vi "UHR-Fleezers Control (host) -Leonardo 04-2018 V5_cleanup.vi"() -> ()   [LabVIEW 2013]
uses:
  <vilib>/Utility/miscctls.llb/LVPoint32TypeDef.ctl
  <vilib>/Utility/miscctls.llb/LVMinMaxIncTypeDef.ctl
  <vilib>/Platform/TimedLoop/XDataNode/timing_clust.ctl
  <vilib>/Platform/TimedLoop/XDataNode/nitl_modes.ctl
  <vilib>/Platform/TimedLoop/XDataNode/wakeup.ctl
  <vilib>/userdefined/High Color/nirio_resource_hc.ctl
  <vilib>/Analysis/baseanly.llb/Mean (DBL).vi
  FPGA VIs Alex/Alex subVIs/Downsample1D.vi
  FPGA VIs Alex/Alex subVIs/Integrate1D.vi
  <vilib>/FPGAPlugInAG/PCIe-7852R/niLvFpga_Open_PCIe-7852R.vi
  <vilib>/FPGAPlugInAG/PCIe-7852R/niLvFpga_Reset_PCIe-7852R.vi
  <vilib>/FPGAPlugInAG/PCIe-7852R/niLvFpga_Run_PCIe-7852R.vi
  <vilib>/FPGAPlugInAG/PCIe-7852R/niLvFpga_Close_PCIe-7852R.vi
  <vilib>/Utility/error.llb/Error Cluster From Error Code.vi
  <vilib>/rvi/errors/niLvFpgaAdjustHostInterfaceError.vi
  <vilib>/rvi/interface/common/niFpgaWaitOnOcc.vi
  downsample 1D array - double.vi
  <vilib>/express/express analysis/Spectral/Block/exnSpectralBlock spectral measurements PSD poly.vi
  <vilib>/express/express analysis/Spectral/Block/exnSpectralBlock spectral measurements PSD WFM.vi
  <vilib>/Waveform/WDTOps.llb/WDT Append Waveforms DBL.vi
  <vilib>/gmath/statdist.llb/Exp Random.vi
  <vilib>/gmath/statdist.llb/Gamma Random.vi
  <vilib>/FPGAPlugInAG/PCIe-7852R/niLvFpga_Abort_PCIe-7852R.vi
  openfpgaref.8.6.ctl
  <vilib>/Platform/TimedLoop/XDataNode/XDataNode.xnode
  <vilib>/rvi/interface/nirviOpenFPGA/nirviOpenFPGA.xnode
  openfpgaref.initrf.ctl
  FPGA Bitfiles/UHR-FleezersInst_FPGATarget_intitializeRF201804.lvbitx
  <vilib>/rvi/interface/nirviMethod/nirviMethod.xnode
  <vilib>/rvi/interface/nirviCloseFPGA/nirviCloseFPGA.xnode
  FPGA Bitfiles/UHR-FleezersInst_FPGATarget_UHR-FleezersCont_IqK95Pvv9lYv5.3.lvbitx
  <vilib>/rvi/interface/nirviReadWriteControl/nirviReadWriteControl.xnode
  <vilib>/express/express analysis/Spectral/XNode/ExpressSpectralMeasurementsBlockNode.xnode
  <vilib>/Analysis/NI_AALBase.lvlib
  <vilib>/Platform/TimedLoop/XDataNode/XDNodeRunTimeDep.lvlib
  <vilib>/rvi/errors/niLvFpgaMergeErrorWithErrorCode.vi
  <vilib>/gmath/NI_Gmath.lvlib
  <vilib>/FPGAPlugInAG/PCIe-7852R/niLvFpga_ConfigureFifo_PCIe-7852R.vi
  NiFpgaLv.dll
panel:
  in  "Reinit Valve?":bool=TRUE
  out "Data Period (s)":dbl=1.4999999999999999e-05 caption="Trap Data Period (s)" format="%#_6p"
  out "ideal setpoint fpga":dbl
  out "ideal setpoint avgd":dbl
  out "Step duration":dbl
  in  "Number of steps":i32
  out "Step taken":dbl
  in  "Distribution":enum16{"uniform", "Exponential", "Gamma2"}(ring)
  in  "Mean dwell time (s)":dbl=0.001 min=0.001
  in  "Backtrack probability":dbl min=0.0 max=1.0
  in  "Simulate stepping":bool
  in  "Step size (nm)":dbl min=0.0
  out "Actual setpoint":fxp<+/-,16,1> format="%.16g"
  in  "Target Force (pN)":dbl=10.5
  in  "MCL Tracking":bool
  out "Current Trap Delta":dbl=20.03845214843774
  out "Tether Extension (nm, calculated)":dbl=1280.0838354247721 format="%0.2f"
  in  "Set SP to Current Frc":bool
  out "Trap X (AI1)":T1={"Trap 1"=0.030792236328125, "Trap 2"=-0.011322021484375}
  in  "Trap Pos FB SP":fxp<+/-,16,1>=0.231353759765625 caption="Setpoint"
  in  "Trap Pos. FB ON":bool
  out "Trap Positions":waveform(dbl)[](graph)
  out "Action (%)":dbl(knob)=-100.0 scale=-100.0..100.0
  in  "Trap Pos. FB Out Scale 2^n":u8=23 caption="Action Scale"
  out "Location path":path=path "C:/Users/Fleezers/Desktop/UHR-Fleezers Instrument - Charlie/Locations.txt"
  in  "Location Matrix":string[][](array[string])=[["N.D.\r\n", "N.D.\r\n", "N.D.\r\n"], ["N.D.\r\n", "N.D.\r\n", "N.D.\r\n"], ["N.D.\r\n", "N.D.\r\n", "N.D.\r\n"], ["N.D.\r\n", "N.D.\r\n", "N.D.\r\n"]]
  in  "Tab Action Shortcuts":T2(tab)=enum."Calibration"
  in  "Negate trap 2 force":bool
  in  "Use Full Offset?":bool=TRUE
  in  "Take Stepping Data":bool
  in  "Cap 1 Flow ON":bool=TRUE
  in  "Move Cap. 1 (DNA Top)":bool
  in  "Cal/Data Acq. Spot":bool
  in  "Cap 1 T ON":bool=TRUE
  in  "Cap 1 Samp Flow ON":bool=TRUE
  in  "Offset 2 Set":dbl=2.0
  in  "Offset 1 Set":dbl=1.0
  in  "Cal @ (MHz)":dbl=20.0
  in  "W/ Offset 1":bool=TRUE
  in  "Offset 1 Start (MHz)":dbl=13.0
  in  "W/ Offset 2":bool
  in  "Offset 2 Start (MHz)":dbl=16.0
  in  "Pause at Closest Delta (s)":dbl
  in  "Move to Delta 2 (MHz)":dbl=41.0
  in  "Attempt Limit":dbl=30.0 caption="Limit"
  out "Attempts":dbl=1.0
  in  "Wait Before Save (s)":u32=1
  in  "Fish for Tether":bool
  in  "Closest Delta (MHz)":dbl=13.0 step=0.25
  in  "Stop F (pN)":dbl=10.0
  in  "Then...":string(combo)="2"
  in  "Move to Delta 1 (MHz)":dbl=15.0
  in  "Tether Alarm?":bool=TRUE
  out "Tether":bool
  in  "Raster Set Upon Tether":u32=1
  in  "Save at end (5, 6)":bool
  in  "N Steps":dbl=20.0
  in  "Step Size (nm)":dbl=0.34
  in  "Save ave factor":dbl=1.0
  in  "APD to Watch":bool
  out "Duration (s)":dbl
  in  "Action":string(combo)="Yank"
  in  "Fl. Triggered...":bool
  in  "Fl. Delta Thresh. (kHz)":dbl=0.6
  out "Waiting":bool
  out "Fl. High":bool
  in  "Yank Delay (s)":dbl=3.5
  in  "Yank to Delta Array (MHz)":dbl[](array[numeric])=[16.3, 15.85, 14.85]
  in  "N Array El":u8=3 min=1 step=1
  in  "Random Choice":bool=TRUE
  in  "Force Yank":bool
  in  "Force Reset":bool
  in  "Toggle AFish":bool
  in  "Extend Min F":dbl=1.0
  in  "Extend Min TD":dbl=8.0
  in  "Extend dTD":dbl=5.0
  out "AF Time":u32
  in  "Wiggle time":dbl
  in  "Wiggle TD":dbl=1.0
  in  "Max TD":dbl=15.0
  in  "Min TD":dbl=8.0
  out "Fish Status":u16(ring) items=["Off", "Approach", "Wiggle", "Extend", "Tether Found"]
  in  "Approach dTD":dbl=-5.0 format="%#_13g"
  out "Messages":string="5:58 PM\tUHR-Fleezers ready.\r"
  in  "Stop All":bool=TRUE
  in  "Tab Control Display":T3(tab)
  in  "APD 2 Offset":dbl
  in  "APD 1 Offset":dbl
  out "Mean":dbl=1.039039384389187 caption="Mean (pN)" format="%#_3g"
  out "Force":waveform(dbl)[](graph)
  out "APD Chart":waveform(dbl)[](graph)
  in  "Calibration":u16(ring)=2 items=["None", "Position", "Force"]
  out "T1 X":dbl=-1.511158478291593 caption="T1 X (pN)" format="%0.2f"
  out "T2 X":dbl=0.5669202904867809 caption="T2 X (pN)" format="%0.2f"
  out "Bead Separation":waveform(dbl)(graph)={"t0"=timestamp(2751.0000000002074 s since 1904-01-01), "dt"=0.15, "Y"=[13.487296816964651, 13.48037403257866], "attributes"=variant("NI_ChannelName"=variant(string "T1 X"))}
  out "Difference":dbl=0.9442381878048121 caption="Difference (pN)" format="%.2g"
  in  "Offset (nm)":dbl
  in  "Rescale on Mean":bool
  in  "Bead Sep. Int. Time (s)":dbl=5.0 caption="Int. Time (s)"
  in  "Take Detection Laser\nImage":bool
  out "APD 2":T4(plugin-control) caption="APD 2 (Cy5)"
  in  "Flip Green Filter":bool
  in  "Set X Only":bool
  in  "Set Y Only":bool
  out "APD 1":T4(plugin-control) caption="APD 1 (Cy3)"
  out "Detection Laser Y":T4(plugin-control)
  out "Pointer Y (V)":dbl=4.0025870540482815 format="%_3g"
  out "Pointer X (V)":dbl=4.635613485356835 format="%_3g"
  in  "Set Confocal Spot (X-Y)":bool
  out "Detection Laser X":T4(plugin-control)
  out "All Signals":waveform(dbl)[](graph)=[{"t0"=timestamp(2751.0000000002074 s since 1904-01-01), "dt"=0.02, "Y"=[0.0, 0.0, 0.0, 0.0, 0.0, 0.0, 0.0, 0.0, 0.0, 0.0, 0.0, 0.0, 0.0, 0.0, 0.0], "attributes"=variant("NI_ChannelName"=variant(string "APD 1"))}, {"t0"=timestamp(2751.0000000002074 s since 1904-01-01), "dt"=0.02, "Y"=[0.0, 0.0, 0.0, 0.0, 0.0, 0.0, 0.0, 0.0, 0.0, 0.0, 0.0, 0.0, 0.0, 0.0, 0.0], "attributes"=variant("NI_ChannelName"=variant(string "APD 2"))}, {"t0"=timestamp(2751.0000000002074 s since 1904-01-01), "dt"=0.15, "Y"=[-0.020049210394969354, -0.02003592505550746], "attributes"=variant("NI_ChannelName"=variant(string "T1 Y"))}, {"t0"=timestamp(2751.0000000002074 s since 1904-01-01), "dt"=0.15, "Y"=[0.03074231675925172, 0.03074526419399293], "attributes"=variant("NI_ChannelName"=variant(string "T1 X"))}, {"t0"=timestamp(2751.0000000002074 s since 1904-01-01), "dt"=0.15, "Y"=[2.9160941496017294, 2.916128360850853], "attributes"=variant("NI_ChannelName"=variant(string "T1 Sum"))}, {"t0"=timestamp(2751.0000000002074 s since 1904-01-01), "dt"=0.15, "Y"=[-0.002644972968316131, -0.002638961391604115], "attributes"=variant("NI_ChannelName"=variant(string "T2 Y"))}, {"t0"=timestamp(2751.0000000002074 s since 1904-01-01), "dt"=0.15, "Y"=[-0.011335016186436862, -0.011341032214389745], "attributes"=variant("NI_ChannelName"=variant(string "T2 X"))}, {"t0"=timestamp(2751.0000000002074 s since 1904-01-01), "dt"=0.15, "Y"=[2.746599475081634, 2.746642933439132], "attributes"=variant("NI_ChannelName"=variant(string "T2 Sum"))}, {"t0"=timestamp(2751.0000000002074 s since 1904-01-01), "dt"=0.15, "Y"=[-0.526083166086966, -0.5261552546492463], "attributes"=variant("NI_ChannelName"=variant(string "T1 FB X"))}, {"t0"=timestamp(2751.0000000002074 s since 1904-01-01), "dt"=0.15, "Y"=[3.0920304879909737, 3.0920243537705665], "attributes"=variant("NI_ChannelName"=variant(string "T2 FB Sum"))}, {"t0"=timestamp(2751.0000000002074 s since 1904-01-01), "dt"=0.15, "Y"=[-0.7128125059590501, -0.7128388598091219], "attributes"=variant("NI_ChannelName"=variant(string "T2 FB X"))}, {"t0"=timestamp(2751.0000000002074 s since 1904-01-01), "dt"=0.15, "Y"=[2.9122738731040343, 2.91227808465834], "attributes"=variant("NI_ChannelName"=variant(string "T2 FB Sum"))}, {"t0"=timestamp(2751.0000000002074 s since 1904-01-01), "dt"=0.15, "Y"=[-0.0023344523453474137, -0.002339854121524665], "attributes"=variant("NI_ChannelName"=variant(string "PSD Y"))}, {"t0"=timestamp(2751.0000000002074 s since 1904-01-01), "dt"=0.15, "Y"=[-0.0026477858821374683, -0.002642139957884409], "attributes"=variant("NI_ChannelName"=variant(string "PSD X"))}, {"t0"=timestamp(2751.0000000002074 s since 1904-01-01), "dt"=0.15, "Y"=[0.014415417950986964, 0.014429639576402777], "attributes"=variant("NI_ChannelName"=variant(string "PSD Sum"))}]
  in  "Signals to Plot":i32(listbox)=9
  out "Trap Disp. Freq. (Hz)":dbl=6.666666666666667 caption="Freq. (Hz)" format="%#_6p"
  out "Display Period (s)":dbl=0.15 caption="Period (s)" format="%#_6p"
  in  "Trap Disp. Downsample":i32=10000 caption="Downsample" max=20000
  in  "APD Disp. Scale":dbl=0.1 caption="Scale (Divide,\nfor above plot only)"
  in  "APD Disp. dSamp":i32=2 caption="Integrate" min=1 max=30 step=1
  out "APD Display Freq. (Hz)":dbl=50.0 caption="Freq. (Hz)"
  out "APD Display Period (s)":dbl=0.02 caption="Period (s)"
  out "FFT 1":cluster{"f0":dbl, "df":dbl, "magnitude":dbl[]}[](graph)=[{"f0"=0.0, "df"=16.666666666666668, "magnitude"=[-331.1367572010275, -79.05506245821404, -86.61411242440559, -88.4728176091699, -90.3181253945935, -94.12566333707997, -92.52740723119955, -94.92192587982518, -99.60936585245742, -96.87568627870715, -94.02570383337763, -83.8058550151726, -97.57441397235512, -101.59968530846606, -101.523049255742, -103.35038532190343, -101.58594091014982, -102.96098031851216, -91.39759462745924, -103.75019963279499, -104.45030075054324, -103.04245334279298, -104.0720279134107, -106.06482372394834, -103.69131867828104, -104.40395035115309, -105.96420043276396, -107.6735556337804, -106.673030006608, -107.34889066208132, -108.05626565233933, -106.25659018850432, -105.29934513380842, -105.43096056709592, -108.3728498841465, -106.0555440144992, -105.78001282181421, -107.48741857324953, -108.67624970548897, -105.39976667156175, -105.91413119232612, -109.4222808198164, -107.0898971593174, -107.91164191890915, -108.26032038855709, -107.58332347164534, -108.23559688234297, -108.01271040303237, -107.66511723652701, -106.51901583170391, -109.27249501469946, -108.55647681594805, -107.93499259231463, -107.05068166453935, -109.13641475410455, -109.29679733781423, -108.19360835527803, -109.57747591546632, -109.58364591011674, -110.47061433372711, -109.8144340420426, -108.79067462293897, -107.54887553357234, -107.99559866705923, -108.85023923652685, -109.68733225238618, -108.51101278437793, -108.51620475114115, -108.22212402200637, -104.63726950302143, -110.2989919678048, -107.61796444414897, -108.68882962798736, -104.79193983043893, -103.59504263746938, -93.64633660288543, -101.9191640501395, -105.73717393151816, -108.92572458793902, -107.43962662800902, -107.79595323081325, -107.0923101993207, -108.17603277205289, -107.87074270713183, -109.20899066381877, -108.61832060412445, -109.10072003106593, -105.76480632823524, -108.60877649218978, -109.67541158970121, -110.2286232768028, -109.84952155309578, -109.33772024076384, -109.95251642394683, -110.14777282585466, -109.13825677905699, -110.05989365698167, -109.39359990189426, -110.56255614635295, -109.66477183197163, -108.9397158528824, -110.26529907650465, -109.20049464984628, -108.20183857013548, -109.09752250184418, -108.00440442238454, -108.35465963524055, -111.16774134451799, -110.34812550238405, -108.94506763426756, -108.72845542102493, -109.41512344014713, -112.44661664432377, -110.35437330889101, -111.32939440655925, -109.42989530434981, -110.98084669076195, -111.92160561143541, -108.57755551751093, -111.40042616180912, -110.15284955891853, -112.21455132279115, -111.40787773511747, -108.82949641635288, -110.13442122547907, -111.42229298204664, -112.06314940885191, -110.6015308813694, -109.51144097251623, -111.15989713761475, -110.25535755335385, -109.65868178057926, -110.51649885452997, -109.77194745285269, -108.4234206864394, -109.50892632093968, -109.46471287444389, -107.92241289271415, -109.72283805386196, -108.63426821579918, -110.37316681536255, -111.09713996884652, -110.32903619589223, -105.32012665515045, -107.36858557554393, -108.00382215905725, -110.06430686942338, -108.81666625979916, -110.01277074453823, -110.94194741225512, -109.65934609082873, -107.80979136006962, -112.81333866824724, -111.61474300955487, -109.83998277184975, -109.45953946904639, -109.79640584952526, -108.19172301667324, -109.28894656674316, -107.61471301278785, -108.83814006090513, -109.08866847726084, -108.20250571862371, -107.96222236861584, -107.03811197900873, -108.93533000393974, -107.74482548035408, -110.79811544577694, -111.1387476496877, -107.42970105883512, -109.18442281176472, -108.73546184641192, -108.71800246690864, -108.51945944378063, -108.06825856571285, -107.27210712368412, -108.12304695877637, -107.84933283677306, -109.73682373154998, -109.32284761503395, -109.31328817453769, -106.68762108642842, -109.79203616876461, -109.9020278896408, -110.27080024357275, -108.54152101558762, -111.00464391726017, -112.42244020766577, -110.82707315747889, -111.00344011890857, -109.90461839395674, -109.42877207451863, -109.73549298167016, -111.67494793393293, -108.85799077901427, -108.5348443278263, -109.803781083881, -108.30644755543659, -108.5079527456017, -111.2055351312823, -108.53089994340155, -108.01739789012176, -108.70360662855235, -107.95873456794631, -109.58297170693093, -108.9372401694271, -110.15921663527153, -109.22399119911955, -110.89883651739237, -108.92840112258382, -110.0545300523626, -109.05961065387005, -109.45831398589371, -108.61239387653227, -110.13001256174265, -108.80060224137931, -109.46327400696283, -108.0177965824709, -109.29727944627197, -110.3237255895986, -109.03258262543821, -110.97880178489321, -109.70034895077919, -111.16405638194153, -109.17324451464711, -109.65698250854277, -108.96750235822178, -112.00534231585624, -108.69274607723942, -108.98110446396657, -108.40723795464795, -111.44459094807324, -111.74799245277113, -111.1601960491512, -108.92048232753773, -110.30506377784799, -111.33145973979093, -110.91850998672503, -110.33684985776448, -108.90206518366908, -109.28458878227542, -108.98773986023751, -110.85813863075646, -109.00041591105906, -110.84543686681204, -109.84382395806176, -109.69722434763266, -108.50915601095721, -107.80829925826895, -110.59736107582401, -109.75377770317087, -109.3992084496136, -110.51151565846742, -112.49753959826434, -109.7299632589479, -109.54070743868353, -109.90314341132164, -111.05974202976806, -109.03766862152392, -109.46667095459878, -109.52800799036197, -111.3163121356807, -110.07817134522178, -108.69251657453547, -109.40472158898045, -109.71400709815576, -110.60534468715097, -109.46937396724682, -107.70342491418788, -109.86331122597839, -108.64971387994616, -110.90117371097081, -108.34928840565928, -110.04172889660904, -111.52979926554961, -110.34759300823305, -109.62712781837159, -109.24131154553284, -110.23196152450447, -108.68509612326807, -108.0246905483419, -106.61876139289784, -101.5519630114271, -80.57695480953835, -102.03744443354402, -107.1449217193017, -110.0695213407169, -106.61597783999268, -110.79221011808191, -109.58974545931426, -109.1149802216988, -109.20993813088597, -109.63768480465863, -110.10428394219181, -109.08445084271477, -108.83472375362581, -109.69508502050168, -108.05588796178941, -110.62586360101581, -109.95315261676905, -107.52208264977473, -108.80708007514875, -110.43484881098874, -110.45942171588936, -107.83804717866751, -109.98973910294193, -109.3496496054193, -108.425252911127, -110.94579264380809, -108.54181722177951, -108.67696070083541, -108.4150202151644, -109.24973583101504, -112.0454922608961, -111.29046597340738, -110.75018248960077, -109.38326363603683, -109.2033340336957, -109.45076170874889, -109.52878049853727, -109.32340869724774, -110.98123395128233, -110.75736340635505, -109.7218385823809, -107.97422606064993, -109.77313701758703, -110.95948744392717, -110.08996774172691, -108.51011830110778, -109.78063140243836, -110.65996628628228, -109.83684298615616, -110.33329049188029, -110.13755118968292, -110.3717925645783, -108.55302219178951, -106.86811628734195, -108.6302156589162, -108.75341391045045, -108.32589578384841, -108.70061474734084, -112.30742263527534, -109.16842570592085, -109.29767035534508, -108.87829025017463, -108.2255616391397, -108.4316108616088, -108.82995906929271, -110.40135575415563, -109.51623498946435, -109.79409808792403, -107.03832759632121, -108.36534528684132, -109.72010868372905, -107.90933028179892, -106.95643597294047, -111.29929166165778, -110.23001135794706, -108.98838015381585, -109.79115357104436, -108.18627479511115, -108.14988122174307, -109.12074063466532, -109.41904850488358, -111.40409873721113, -108.83156790193294, -108.77032248953847, -108.88363158686694, -108.47515048290681, -105.94172147874599, -109.38146940214403, -109.21277078848794, -108.11309390545507, -110.70840012427504, -109.5504457849329, -109.52330684534209, -110.06776026911132, -108.21949434182314, -111.21266686269992, -108.78581501170974, -108.43115799297222, -109.63260325780062, -109.84070220619535, -109.72041980780126, -110.29615941882527, -110.60316734262464, -108.79165446414692, -110.95840439895592, -109.64926233107009, -109.16526769544322, -108.65292362430982, -109.56113898129935, -109.85693046339026, -108.92316027325207, -109.79492493553914, -109.38157962945887, -110.24545136266825, -109.30031463492487, -109.0795429936869, -111.4091719525013, -108.63499083917162, -108.43863465339358, -109.23207864880891, -111.21947487191643, -109.24525201480154, -109.56842406077318, -109.46711940800672, -111.91389548262572, -108.15655736690546, -108.71882059966947, -111.26328503478568, -110.95027143873176, -108.4853106242357, -110.36902802777546, -109.9314203579182, -108.77686164101732, -108.71871020068312, -111.04829661168574, -109.95072655339462, -109.88221342875462, -109.53241732756136, -108.2625005404823, -108.00677030040697, -110.19659317581693, -108.93858924796267, -109.46817875483995, -110.78063992017232, -111.11066570318451, -110.78774336696706, -109.19199744617812, -108.54914256407436, -109.28414960420909, -110.64143585101183, -110.5855350821307, -109.47578632252726, -108.89705360836223, -109.89214013612292, -107.93271261027171, -109.32631601340563, -108.60274611341092, -109.40110159872573, -110.889237682208, -110.01391165813328, -109.99747108785071, -108.65542819213674, -110.37211847668736, -110.44656500845738, -110.8128133834973, -108.8909299260433, -110.19551227077532, -111.37647266643523, -110.83802189730321, -109.98519377913681, -110.52378970770522, -108.16970420057817, -110.70974729773344, -110.76836765494402, -110.26884275594577, -109.22041044268806, -109.87809744746195, -107.76823252107832, -109.12119474042969, -110.28066108731146, -108.55000033509207, -110.18152097767907, -110.73030521152278, -111.49470908029893, -110.2320929919509, -110.03370979233021, -109.79181668155233, -108.6673501209991, -109.86695766650877, -107.88926518046961, -110.95525003776572, -109.18130359755742, -110.42618009658618, -107.90341931158893, -111.44736855661769, -110.72634267386593, -109.29945988519303, -107.67889101961411, -108.81148059987765, -109.13375212757057, -109.8122873383549, -109.80176697684155, -109.96342275204768, -109.90406635707086, -108.75674342748256, -110.12362902701081, -109.82151095527837, -108.62543344241836, -110.09171852771195, -110.21434637862887, -109.97254504855631, -109.27043209093468, -111.35149588204125, -110.12399876776051, -111.65983675538546, -109.28788875768564, -110.86554069990251, -111.26990906470603, -108.60956517491746, -111.49613890850938, -111.79685722966795, -109.26269485364045, -110.38555615546439, -109.40641023162068, -110.966136593156, -108.78892524584494, -110.29340727375603, -111.44032043281035, -109.95212021173755, -109.79233511584334, -112.41184021118175, -109.73687851881148, -108.65493879781806, -110.76132988919045, -108.43230346094671, -110.32968175895853, -110.29890782023821, -108.77609076424456, -110.3298662333555, -109.47734504217333, -108.2677295732245, -109.21234363352882, -107.83278941978479, -108.85136784424789, -108.43241251530755, -109.76609391460555, -108.53204373005357, -110.9660641972934, -110.3152512161094, -110.72570499399905, -109.23877906286317, -111.72407743101837, -109.20311421918561, -108.06021800233717, -109.29288625761943, -108.78395253409145, -111.85250172876302, -108.78827588901797, -109.79775055719482, -109.12089297455859, -109.49896359356035, -110.34432647103819, -107.94700097960238, -109.30489238477631, -108.89170290869342, -108.82574563272509, -110.11024077194833, -107.37946433552314, -109.60167933458756, -107.80625057819019, -110.11489057210264, -107.35436859378505, -105.69819484613895, -109.11280625683739, -109.27770293057978, -107.7053735252589, -109.75022444894368, -109.3310543596577, -107.87683693707739, -108.19931495338068, -109.26462246191564, -106.71885779297867, -100.00018022217961, -92.54434511397295, -107.20472143807373, -107.39203415155283, -110.04461177268398, -108.48860496315312, -109.0057168110333, -108.37627790492552, -108.4108380728248, -109.65509454313073, -109.64243000632982, -97.04219069306761, -109.0928856629964, -107.9760697315632, -107.52611064047497, -108.87702814778996, -109.08437599027614, -110.70097118837974, -109.00969860961283, -110.38275386163214, -110.0699155421545, -106.91498895181175, -106.22178738309017, -109.36827866896039, -107.59953130968307, -109.19516217272808, -108.31502495393616, -109.384158926223, -107.11670654202719, -108.09436312738853, -110.14559230873704, -109.84997663447679, -107.83465335309926, -108.60947100624459, -108.9932479423645, -109.17174810371898, -108.79457339828916, -109.40909327982367, -109.6328723628302, -109.51081854476179, -107.63054408568418, -109.63728404010122, -108.51163794839918, -107.55002282725216, -108.97796212764939, -107.24648164623483, -112.21470452291085, -108.74294024554423, -109.62070777514892, -108.05768666239368, -109.8224946685739, -109.34575507446003, -108.53536952609525, -109.60789300457671, -107.56681538208278, -109.22777325016398, -108.79047910308894, -110.10332477250668, -108.00206387955672, -108.45604004720035, -109.00645795765472, -109.81039564269616, -108.92785144634745, -108.3978471520567, -107.94411095685999, -110.53486519304262, -108.8773780319227, -109.03345093296107, -107.30746693745031, -108.54277704832029, -108.77629108166091, -108.91111762599647, -107.74965195880401, -109.97375370738439, -109.76326492689246, -107.91717581777407, -109.0730556927617, -107.66804873204664, -110.40438871064791, -108.05794247751498, -108.80206615156494, -107.51329354700796, -108.83687012994949, -107.57713176895379, -107.94774159581414, -109.41894615439651, -107.10869425078764, -110.51480854078629, -108.92221367099775, -109.91358786461535, -110.1744263092835, -109.30795472883494, -107.91359710691006, -109.77888185049835, -109.52060975706438, -108.66686651982212, -108.71041801553639, -110.13619546359467, -108.87957097273856, -109.72150387215271, -109.00776068810654, -109.70251113927438, -110.75769213896399, -108.53234896741436, -109.69439526582246, -110.15412541604617, -108.25183374628219, -107.97402569656481, -110.34920156998648, -108.45106995186384, -108.82031145748209, -111.38690005057539, -107.01968459818563, -110.3044500039584, -110.8755481852125, -111.08915057663255, -107.94824988655199, -110.21669144934839, -109.90539774633154, -109.58985438756767, -110.12258796623348, -109.41689951612143, -109.31128210476795, -109.00258476567323, -109.11093063041056, -108.83347064311234, -108.32685287566952, -109.44770946560935, -108.40145063144861, -109.68448193892085, -108.76525439243828, -107.62837139034596, -107.39300298848994, -109.36993934990318, -109.2465218489418, -106.66307369796812, -110.15891092764934, -109.57151745419041, -108.92425698310808, -109.8036704717834, -108.79751146756549, -109.25926431818017, -108.46260574057584, -109.1967554647261, -110.63319560262356, -109.02343067385144, -111.22073171487528, -109.4731095097105, -109.69335000085164, -109.48782989577005, -107.95204227683271, -108.19468255763758, -111.36195112053247, -109.55696116543685, -110.3130767640534, -108.9621824253354, -109.99735074896789, -109.20198058456344, -108.12100614259485, -111.27227490807289, -110.09248554008288, -109.14395535060149, -110.80882692379708, -109.22632926901655, -108.64497210802793, -111.00030482190711, -111.1317849358033, -107.43140429257826, -107.9783302193555, -109.2639893652291, -108.97008485446163, -108.66556668859064, -108.12995785876932, -109.73001061107855, -108.09691302413727, -110.68391499215569, -112.78583642012705, -108.7093037763389, -110.67868795924797, -109.0190959349128, -108.36247198231372, -109.82829353258869, -108.24916379311045, -109.84154533905823, -108.55470160833775, -109.75438989348815, -108.82865632118325, -107.63622268162582, -111.00943492886312, -110.81824358463759, -109.46028423652966, -107.52479398900992, -108.99087806823736, -109.94494831750349, -110.26788355564504, -109.8954055022304, -106.9478122391182, -108.91705388158901, -107.76095584490312, -109.28456723055147, -109.7982307261767, -108.98552661346622, -109.98937979783426, -110.57907422426224, -108.68113463944836, -108.06257240208589, -110.0707224529617, -109.19515280354733, -109.35868842818849, -110.37311467065695, -109.0404734478992, -108.16686395270187, -108.61859220485148, -109.19986437876149, -108.19707189725302, -110.06564239663074, -108.87850403465154, -110.63824157544798, -107.36918104067212, -108.7008736325543, -110.9359398265406, -111.08529123080929, -108.44209934821818, -109.79529621208783, -108.38917887958179, -108.169117639508, -109.24332926356216, -110.50584058811704, -109.63592524002665, -109.32261039377495, -109.16720880524552, -109.3084314664462, -109.5812223978583, -107.70213196487856, -108.0557884982431, -110.67058020007828, -111.68459781023608, -109.66270627185824, -110.52536245663693, -109.70208409132103, -108.78645420809342, -109.23122088059863, -109.24601474121832, -111.25604763816514, -109.50225851581177, -107.32434217163818, -109.28548556764925, -107.59972621660836, -110.46928774723048, -109.25950101547609, -110.32016453935465, -107.78482761561703, -107.89462895091089, -107.51366154391481, -108.08036891159172, -109.53371809947035, -101.2452927166745, -109.32763325689056, -107.52166868423687, -109.89648659445174, -109.11350200980485, -109.81336712738089, -110.02799517445062, -108.02767143538516, -107.97850220501483, -109.50772934896838, -109.31069875721964, -108.49991657749598, -105.60880911233095, -109.79128597340213, -106.91084537903113, -107.84880087118997, -109.63628170511824, -109.03203967193224, -110.64186113413658, -110.98027990365594, -112.33841002907062, -111.01793075565425, -108.58025797022215, -110.4259296883756, -110.38643255981424, -108.93051671115133, -110.97544177116494, -108.63883100482677, -108.37581711765226, -108.90240163126536, -107.94688047875466, -109.9482937437732, -110.09097112364414, -110.09805032265376, -111.44307114024532, -109.15483789122554, -110.9713708217832, -107.8548737634672, -111.41418477109195, -109.45699779859628, -97.03595099331734, -109.16746744169623, -109.66209204485918, -112.57048704774604, -109.73989735035725, -108.16252575067017, -110.7546980664636, -108.91536673403449, -109.20509151422344, -111.0260632167785, -109.62924582406518, -110.45466277291722, -110.2973970018937, -109.67550222925419, -108.84481022020094, -107.23686414357573, -111.79004633370906, -109.85453094194085, -109.45617270081004, -110.73920606732504, -108.90879956851099, -109.67774425528265, -109.4745715721361, -110.18080454693559, -109.26079184315502, -109.41692499885505, -109.02240975088358, -107.80833423058168, -109.32657361431549, -107.87138278655101, -110.910364670719, -109.70067156846706, -108.55301754282077, -109.4243252157005, -109.77567725161107, -107.83737232063925, -110.36509412773016, -109.6371048811367, -109.49430894422814, -108.55509251499753, -108.03996302911446, -110.4385715838736, -110.08864436068788, -109.48922484379962, -109.90865554258562, -109.7491963238264, -110.04796094537969, -107.413043439116, -108.54229076126079, -108.2522516728666, -109.75464941327974, -110.26795832300996, -109.28073673851144, -108.62990200974927, -109.89408067552287, -109.09160284731726, -109.90740624925795, -109.92534708896517, -109.79578862362752, -109.97278346890566, -107.80679350393824, -112.81728446281548, -108.09689504419987, -109.89549991422173, -108.43930976031248, -109.95153099843282, -108.18277483720716, -111.89607792605433, -109.52567003805, -109.17125106979698, -109.64300739407085, -108.21045178846524, -109.64036472149706, -109.02324448538845, -109.039163008889, -110.41006510134076, -109.50289952116489, -110.4732620447796, -110.08777181504614, -110.15589511434341, -109.55705089158471, -109.2547682932589, -110.86823885471617, -109.96330502176939, -109.85995369810554, -110.63211290903473, -112.08007783432191, -110.24725218052279, -107.62861148917592, -110.08691795849435, -108.89793794632287, -111.07702220466341, -109.46946126482341, -109.19747345337464, -110.70018609416007, -109.66366205691908, -110.78032312133551, -108.05724200456513, -108.195661625627, -110.90724508408255, -110.08307674771669, -110.76863516643007, -110.46620425061583, -109.16986788877276, -109.61921294239114, -108.51159432329543, -109.96308336765689, -107.38178944242856, -111.95930944846394, -109.3329826827624, -109.59119636368249, -108.83148571828912, -110.46194288788257, -105.87694286145472, -107.985886302892, -109.2975019660806, -111.05138725716857, -109.60005889204612, -110.92871351729086, -110.73480546964537, -108.41587420326718, -109.84275465824477, -108.8249071047676, -107.65358887817105, -108.3254150042995, -111.47362100321767, -112.7287536850025, -108.8217125660507, -109.50232320231771, -110.29587061625348, -109.30644535112089, -107.69178032077258, -110.84522325672016, -109.3735891463141, -109.12506388923123, -109.65582307934665, -111.11427272192576, -112.19827973435466, -109.11306367925813, -108.19203577968261, -107.89831568266465, -108.85805249169313, -109.51100049661844, -111.71546684086955, -109.53880495724334, -107.07739286222231, -110.66836728754211, -111.5415170557177, -110.16051267940297, -110.6107546662698, -111.36389129556191, -107.77888179117923, -110.34160392509817, -109.61287125994414, -110.23791773883013, -111.00669159903549, -110.97165069538953, -109.43965413392434, -110.6813161690388, -110.31441293654314, -111.96129906273796, -108.15998218707462, -110.08095912053633, -109.41084567452768, -109.28774416263552, -110.80159950384204, -110.41956747809755, -108.85005186267244, -107.9069227847757, -108.84249369063123, -109.92569208845894, -109.34109797584448, -109.41334788055491, -108.76462023086997, -108.22069272136177, -107.0786679601274, -108.30206755098202, -108.57613406368954, -110.83330887636482, -111.93966942736989, -109.76373713473264, -108.25782074884941, -108.16490627215555, -109.93351470267982, -110.75525684428368, -108.22814762283093, -109.73442331991602, -107.53145627482685, -108.27195221226805, -110.33032779278457, -109.48951857415828, -108.12599093700939, -107.97627415508097, -108.81426859968796, -111.21764717894752, -109.80856212352333, -110.92658779118501, -109.71551885834796, -110.38682741010847, -108.87671328341361, -109.68368600774755, -108.35359806351899, -111.7519400010676, -109.89407081573103, -108.24301180922755, -110.00646944788126, -108.6685299083706, -107.52856885980722, -111.7622363038509, -111.0025144494897, -108.64719599357296, -110.62968467177518, -108.821509935539, -107.94915453463719, -111.53070432277694, -109.87282048586256, -110.71167589371663, -109.79225006081626, -109.96203471712074, -110.29921092232489, -110.10644439440416, -111.28815007382043, -111.19165661703703, -108.46024117100558, -110.22528296512183, -110.32184972386672, -110.05120383416072, -109.78792549362107, -109.00355659956696, -108.85989369286315, -113.00899556732638, -110.91756826567867, -111.25016866167897, -111.84225040552181, -110.54451635944174, -110.72722829912917, -109.60759702177283, -110.49362602516815, -108.74419542915284, -110.3379671069179, -109.66259088220754, -110.45956400953156, -109.13956157147233, -109.27130155486806, -110.83015602667983, -109.17970724944131, -109.09662765889193, -108.0447366108107, -108.9536269357457, -110.35663108940085, -108.73418835472056, -113.42965806805827, -111.81270536656905, -110.06155590173537, -108.76582224646269, -106.7488061675813, -108.5700320158723, -111.11038264410035, -110.41435767488723, -109.12763443489911, -109.30517580756394, -111.61251165371237, -109.8116632664339, -109.36845864976851, -109.00390009629231, -110.54359197165573, -109.52629258465976, -110.75932197632896, -109.50903215359567, -107.42652056246085, -107.81146496533543, -103.22224383145215, -108.53803076819163, -109.78623360072066, -109.66306634612869, -110.80245829141279, -111.87835085452016, -102.27372781471168, -111.27763038431458, -108.45838423437681, -108.79077917058028, -109.31951755762685, -110.05415097017186, -109.5535934823387, -111.62732254641111, -110.73478247119641, -109.9468722686683, -110.39698367573979, -109.30612942398305, -109.7578384694043, -109.34817295524313, -105.56944757301993, -110.1940418750125, -109.27076023513962, -111.03491935225027, -112.2980497521063, -110.65725497955563, -109.0567530102422, -110.31700596563523, -109.64508026365678, -109.6190471404421, -110.52566833759428, -109.68595899227789, -109.7431160985074, -110.4798230300751, -109.45506977604765, -110.69504157940786, -110.63067849573177, -108.06456949500138, -107.99354148885966, -108.11349194720599, -109.15944121207349, -110.61766925164031, -110.14145801314527, -110.67420842201165, -111.91532881806512, -112.15901550030345, -109.94774413630104, -109.2819568305201, -110.94623189179737, -110.17685430287735, -110.39082916961016, -109.53953238698966, -110.76940623620611, -109.89327922318515, -109.10275695043765, -110.21445972656734, -110.58968777252528, -110.57016757660259, -109.59208496373341, -109.07946946465374, -109.10762003745964, -110.36892993974607, -109.81864495218393, -112.12972189864566, -109.26185849434863, -111.56305819991357, -111.36019621828058, -110.3397604159226, -109.58675612753163, -110.58041217474447, -106.34739062044932, -108.6722699609389, -110.03906060709869, -109.16794717548382, -109.65012481802809, -109.35377624077988, -110.51889143862303, -110.03397458059777, -110.7981307056636, -110.56653507062292, -107.61367005067231, -109.99279736988825, -111.79875182878175, -108.60382315996031, -109.71381533228038, -108.60388131505613, -107.0933685540362, -107.86037690830757, -108.40980028847238, -108.83869602763895, -110.76921375395764, -109.96766364716046, -110.8256171465781, -110.13805084291067, -108.5349140035878, -110.57158437465219, -110.8920694413417, -108.71646695477324, -108.33274238445665, -108.96152108305608, -111.03750932994224, -109.48915027983756, -110.29725207211165, -110.79527247268442, -109.47969936716117, -109.79306701834035, -110.16840035577498, -110.29840230783668, -109.15306387075587, -110.72651274964761, -109.08881658764956, -110.8349724030761, -110.64653625576447, -111.40392562616867, -109.94581588927414, -108.85136340231294, -109.77228546607624, -111.48297395390018, -109.7334001251941, -109.30537415590783, -109.63937411233408, -109.69785848648013, -109.3523781030017, -112.04667421182404, -111.56311816195343, -108.18548447362308, -110.63388993686104, -111.39768634137992, -109.87157345395542, -108.6734208287271, -109.46213300216168, -111.75774769437145, -110.10245994173216, -109.52385139033495, -110.96513097775451, -111.8709319163154, -111.54948269614047, -110.29760900080463, -108.52168175904663, -111.09033925738258, -111.14752744054172, -108.83074523709202, -109.05704141259113, -111.74377805749482, -109.57200906899736, -108.84121318623825, -110.86657990204343, -109.54363603755047, -110.89448416316372, -109.58965570570145, -110.21012263847972, -110.4063470702923, -109.5021950342969, -110.33648801598177, -110.90551031296536, -109.69205870504638, -109.8648503154861, -110.28183391384131, -109.65970942950766, -108.43615680946908, -111.11790511866548, -110.89043476451553, -113.64898442872548, -113.08004494963895, -110.81525412051718, -113.91009875719509, -110.95802128672312, -110.40944585634135, -110.33464695414992, -109.98984645778987, -110.18795067005652, -110.62364351231234, -110.44029833291248, -109.01598585569788, -110.95430216511514, -109.77987141110621, -108.54452361812068, -111.41780266439777, -110.47172771858405, -109.06084635984516, -109.30794593246578, -108.8764083815745, -108.18222749506985, -110.31330487887435, -109.04176821738014, -108.8558386035048, -109.47888284507395, -110.01459604573937, -110.48596659065309, -112.6781342298378, -109.85522803775775, -109.0569534499285, -109.08991286548698, -110.89485727880403, -109.18715778948663, -111.50381433568144, -111.3545424730884, -110.07710926239977, -111.99977850157067, -109.47444853853723, -109.81605328527645, -110.74995213151195, -112.56834665925544, -108.52052472391404, -110.89121213995557, -112.02004142355113, -108.66413739656008, -111.10053848695652, -110.41241079991636, -111.80152991764473, -110.21746151515111, -110.63265128607344, -109.483042128511, -112.78639954059729, -109.47114195846122, -109.23309637902875, -108.97133643967169, -110.08909147812822, -111.01105271457081, -111.18602432128249, -110.04633990216801, -109.53453538673071, -108.81939452082017, -111.13486114285661, -111.65877073200598, -111.63763706753498, -112.14107810664572, -113.6231865196724, -109.31743865878806, -109.18551713085722, -108.74951309653638, -109.28206426212142, -112.36687029711229, -110.10933061193728, -111.29501093502684, -108.19021080564794, -109.34497312126749, -110.37228033937312, -108.63277512903049, -110.61033993911002, -111.2975761598062, -111.49780004751436, -109.91019436685814, -109.32789992989028, -111.4482538110117, -110.1538439123475, -110.66347034043578, -110.05055133068794, -108.53002033538341, -111.7522199783972, -113.49108651193104, -108.03793940563418, -110.07108694011555, -110.83958739865201, -109.62805629409038, -112.69637731014087, -109.57996950503268, -110.104850643722, -108.83376203949506, -108.69400304840181, -110.59434352922563, -110.69121011800921, -110.18694553784364, -111.90598571547098, -110.30230802494223, -109.66810649416752, -112.6017099000434, -111.00296745333219, -110.64462650261785, -111.4775358707403, -111.98753241268494, -112.26574909791167, -112.04796822399412, -110.65853064447325, -109.6623218025264, -109.40559579075378, -110.42174451813142, -109.18991987957241, -111.02050178263048, -112.77950487440032, -110.42443751566815, -111.35440372400903, -108.5263524245987, -105.07498063939795, -107.15444425741984, -110.4508720018025, -110.25163264819463, -111.1383261104107, -109.91171620173931, -110.52200560606038, -110.5299174299573, -109.34628087255733, -110.26101817411786, -109.65071853372183, -109.66953335961068, -110.83590602054682, -110.980546313788, -109.4110066989163, -111.47223607390256, -110.00281523859483, -109.4088722967626, -109.00401922839337, -109.59655302543185, -109.7359970854586, -111.46016206343049, -110.23478747568004, -109.29441275295858, -109.82941912510167, -110.43088525283673, -108.21649744751299, -108.70220592702613, -105.2334473604296, -110.60620657984927, -107.97533820921146, -110.7664079806058, -110.56406610911355, -111.76465470250328, -108.84172809688911, -111.03661078143631, -109.85351980370237, -110.70091167176791, -109.52380717508088, -108.4356492672842, -112.25498760397127, -110.69648730540193, -110.36748838594507, -109.99090797924349, -111.2678642544111, -110.42541694325627, -111.4575545259775, -109.3211175669008, -112.7465573314208, -109.56208667784249, -111.59733497772172, -109.42295730962105, -108.55804089331346, -108.71397903286748, -110.09188290952392, -108.90810063278326, -110.31333217069538, -109.69794714542728, -109.06210020835357, -112.42465112160288, -111.74630553904855, -109.99304310093493, -108.93867687355595, -113.1669287525049, -109.09193568851137, -109.27500368450697, -108.99643325722404, -110.53962759110647, -111.2052088429852, -110.05855563908841, -110.30763723153481, -110.03411001268613, -109.6161415052669, -110.6304714466923, -110.17116005754627, -109.0753171640551, -110.92564270851628, -109.60831770517053, -110.25913363817017, -107.76644895378317, -109.2619309023068, -107.64198246311884, -107.37056168314048, -107.31978563121643, -107.68171928702894, -104.57515288104209, -104.75187637758803, -105.27246893266054, -106.96524396060869, -105.93920355631757, -103.66449995825586, -104.08476660009461, -104.53081578265315, -103.0148493379086, -106.74751670818362, -104.92309629919443, -103.98320340724693, -104.81633219413234, -105.77996356028235, -107.12559309216644, -107.28196039053535, -108.84583578337953, -109.4494696919565, -109.15525441177898, -109.7634811359225, -110.79433338587495, -108.44440079452527, -108.79597700117748, -109.98590735173822, -110.72144284267539, -109.30550753718086, -109.70072152916897, -109.65801130162137, -109.65949265997646, -109.82238573025273, -110.30669821947491, -109.83394128869384, -108.90433312205332, -110.664046708231, -110.39926453734134, -110.37725911098757, -112.12508639032839, -110.26795666332589, -108.98741993218054, -107.76168841100478, -109.82334992872889, -110.83516363498563, -112.60649745671253, -111.1960726449926, -111.03919163866381, -112.05129034965563, -108.83187987662883, -109.57240688505179, -109.32857861150738, -109.54934849013647, -108.29359879300195, -111.5179112931669, -109.52702486426027, -109.95429980789645, -110.7011078611564, -109.43204524997455, -105.56031249677113, -107.70609254346495, -108.78303653454363, -108.11457060956113, -110.44215460317537, -110.78267897406572, -110.33119812901934, -109.34449539666907, -108.82636558484161, -107.1834151347969, -108.83808254322192, -108.2542825327446, -108.80298057862501, -107.59922121598055, -108.9131916496929, -109.51519107961856, -107.7704986323755, -108.79678029009878, -111.13791068210752, -110.402746275919, -111.31702623823912, -108.49812727557243, -110.63723264798182, -109.32890666586829, -110.29721723278237, -111.66560929315017, -111.04227698307153, -111.36927505376269, -112.5203298417673, -109.93967930487354, -110.14533835678606, -110.3868348991775, -110.85413569165249, -108.44519725537315, -107.93391978795047, -109.82778679299085, -109.79311153223738, -109.25261055399044, -111.47738679135526, -111.11775495397512, -108.65898844492045, -110.26505495390529, -111.02017977446526, -110.34817965403467, -107.55161094495372, -110.21667403085983, -112.43970497917284, -110.70535338255132, -110.79438078890512, -109.81809822502822, -108.99167960596515, -106.5556893069368, -97.51736665041192, -105.29926513345109, -108.72453297392224, -108.23203912463346, -109.50324111400698, -110.9939986929772, -108.05367524487318, -108.37339392211176, -109.8553291283933, -110.46179639493138, -112.48795697163695, -111.88145079973545, -110.8678969738583, -110.62677605624849, -111.83824818603244, -109.76798658735359, -109.6654742351465, -112.58543522753767, -110.3406716250781, -109.55013159400883, -108.00481229232405, -109.90793236599207, -111.28597960985334, -110.54144527494444, -110.14704702870655, -111.2652554338908, -110.97520848958668, -108.63647576273343, -110.52472680617548, -113.16137826273847, -109.62457037485827, -109.53869420402964, -110.71399284283449, -108.55435337782664, -108.09492728294455, -112.2373886856363, -110.3693019226993, -111.65116752865308, -111.3223986412311, -109.67734725401074, -111.36420709226297, -109.14293108556625, -110.5982939020188, -110.29596476096043, -112.69847120697035, -108.39052787054206, -109.06205229490357, -110.00045399262885, -110.71775009467346, -110.69530760167493, -112.54144940754935, -109.55755373438097, -107.88943697845929, -109.98578587243783, -110.14202980613851, -110.80051915904802, -109.11327182471621, -109.50637030500913, -109.77023677605327, -109.98552825925917, -110.40235854896, -109.37603004890141, -111.36989177909379, -110.8399811877331, -109.30394670937987, -112.2769814990538, -109.10893172594731, -109.17733972841754, -108.35968166480572, -112.64492569586005, -110.13779257328873, -110.64439690778532, -108.45446935516622, -108.97325006911116, -110.54637968933774, -110.66412364132371, -111.38627695224784, -109.8942998516069, -110.36392017322382, -109.92355133054227, -109.61886697310419, -109.71969465343778, -109.85627196259388, -112.1407808286419, -111.1013489416651, -110.70428953307596, -109.3454280179969, -110.22984684615578, -109.53826801613613, -107.83673208330934, -108.72742563398342, -109.5745872123195, -108.83031823548816, -110.89059911076627, -109.87842545384129, -109.21980161063786, -109.07140273870678, -109.04628915564135, -108.79255665097845, -105.20875397856382, -110.0838008881032, -109.68293832806683, -111.24644641302518, -110.01257579497496, -110.99281477454484, -108.99296184719546, -110.96495665514604, -110.70404386182749, -108.25078498739035, -100.77667501455139, -107.61479263900088, -110.06600976399395, -110.02035637581871, -111.45524052052504, -109.975541184397, -111.07333860975358, -108.4808974233161, -109.59513524582242, -110.74711589861774, -109.50005300854993, -105.23071652566294, -111.81094849223531, -109.0168079712372, -111.89029991620679, -109.90672274216391, -109.30959446424889, -108.23718655264584, -110.10868108588909, -109.21139771899594, -110.33333323577992, -110.25792318324204, -110.67825932924109, -112.33148517950511, -108.9724848367048, -110.78371843797613, -111.40913868573313, -110.2930522718577, -111.9538408094371, -108.63639312641844, -112.4462941079034, -110.40266356498321, -108.66617580940074, -109.44306834729083, -111.08962916641603, -110.52132608161017, -110.53757698855654, -111.5587344449704, -109.77722315102946, -110.40060629757771, -109.45395807961631, -108.77558572395142, -109.0151938598724, -109.80739619986889, -108.9332873172888, -112.49933978358132, -111.28667321897437, -110.40629082858706, -109.9829216820938, -108.85102919990373, -110.84179127037925, -110.27309817549309, -109.88857884367955, -112.24517967927224, -110.23377125710859, -111.26951227953063, -110.09782138347559, -109.77508406986834, -110.55359722398646, -110.09534729906368, -109.96333904888587, -110.29372855476366, -111.36651812163072, -109.97141184588116, -110.16701683369045, -112.8562627359291, -110.66651146857079, -108.78873821095968, -108.59208174618087, -110.31784275318834, -109.43177042415276, -112.80272887161644, -111.79874205007107, -111.08216899537892, -110.73699224045636, -111.04738767291953, -110.43395896705012, -111.62106163510778, -111.32599933330843, -110.29360981749807, -109.66562228449096, -109.21316193790335, -110.06363162177448, -110.54480468587292, -109.31791670875509, -112.65386492377107, -109.91857609999171, -110.57233605624137, -110.7597333064856, -111.49767138733276, -109.36548654843229, -112.34145274183716, -110.52831153822652, -111.55802243871352, -111.81399803046556, -110.17680125962372, -111.23811621944807, -110.48042049674514, -112.43786993562033, -109.56507357271987, -110.67030752598993, -110.86377249100713, -109.06001892813467, -111.37023727930494, -109.52881096984436, -112.95107295160436, -110.49467818026214, -109.29804210589607, -109.89270706931751, -109.46354468058833, -112.10350702955014, -111.06083529077077, -110.49996587015904, -111.1617248913634, -108.84725633199014, -111.42852695852422, -110.01433866707184, -109.11616968390972, -110.76961079765468, -111.80403513904453, -109.84442686379181, -109.65447921666167, -111.3378640555306, -110.8882647652338, -112.58014202075226, -109.67128881545659, -111.73429980763389, -110.82258070774773, -110.71895931098041, -112.5117489008152, -109.16182299471309, -109.71651258790612, -109.7770618808562, -111.94294809571427, -111.1629115541574, -109.57489224865171, -109.8402445779754, -111.17931450307283, -110.09045865447595, -109.23658206733491, -112.54929616847242, -110.5150381158864, -111.32296447909377, -111.64472156295191, -111.65832771066007, -111.03359562742956, -110.85303206770837, -110.80655337650862, -109.3712696310075, -110.57313454785879, -111.18525355670417, -111.67423695430561, -112.00829831274282, -111.08915434609605, -110.3298290221436, -108.68552957386795, -112.11377370993225, -110.80288297661977, -110.33640536217185, -109.5907971201988, -107.9195263775506, -108.50223113159429, -111.91191347156142, -110.29585599512956, -109.50902788911351, -110.76819145749467, -108.86899533416589, -112.09963049260891, -110.13374376572433, -110.15881393584463, -110.87392107947531, -109.18658540731009, -109.72734703956934, -110.18732487568724, -108.76554115185057, -109.94122289815374, -110.39583285609643, -111.09540935727229, -110.6618176357367, -111.6281345666718, -109.69686483639367, -110.31633402076315, -110.61246951748903, -111.73300235294965, -111.34221378834899, -109.46708370903485, -110.70412671997354, -110.7007891485379, -110.31685483435038, -111.03016917417074, -110.94517365625376, -109.46580797053619, -111.20935248224806, -109.20661126636224, -109.50147037097533, -110.14241781654353, -109.8510950344643, -111.3794198224028, -111.28966889207122, -110.43347441663424, -109.86759980279523, -111.92101892013198, -109.31594011390644, -112.92253433794441, -110.74000829597605, -110.3690783911604, -111.9386136764295, -111.04196305034188, -110.41800427558245, -110.94287511448232, -111.66035388807579, -107.53723747644062, -110.68014818358719, -111.86628806511304, -110.12097497430523, -109.69880468221378, -111.4312783987915, -109.18240866486639, -111.45649839248873, -110.1242345454651, -113.75911576151633, -112.71747598882953, -110.9614554157337, -110.92294419716129, -110.87229098694876, -111.09943759113875, -109.48107247947176, -108.62783006742795, -110.8108025857779, -111.63342408317932, -112.0221522906341, -109.96411229549527, -111.29821085030613, -110.04566676239914, -108.41674583097112, -107.50256474992416, -108.68086611003493, -110.3738906060137, -108.86763212826641, -109.81681043446049, -111.04539822346567, -111.73290882980949, -109.75238769150758, -110.55268275367449, -110.48423701377924, -112.1116140908134, -109.53952175199518, -108.538611608547, -111.3788321484912, -110.36378736224961, -110.37712171023523, -109.82150687920334, -109.17046632238393, -105.1169578108227, -110.84067642540583, -112.91626789016587, -111.32030958133453, -108.93375913686056, -112.44450956563915, -111.1596840012794, -110.17380444915341, -109.634859036508, -110.68819277718731, -110.0648098825346, -108.87385575091399, -111.99676414571755, -111.32585405719519, -110.59892045991457, -110.32589048340424, -111.1172696292077, -109.79946399891651, -110.10030723919304, -110.71841081343656, -112.23013150012054, -108.94400401141407, -109.71044551701596, -111.77560214164039, -109.68779520039777, -110.96119601299907, -113.66477058855787, -110.17794649102234, -110.30159876509862, -110.11953836266514]}, ...(2 in all)]
  out "FFT 2":cluster{"f0":dbl, "df":dbl, "magnitude":dbl[]}[](graph)=[{"f0"=0.0, "df"=16.666666666666668, "magnitude"=[-324.19011195451765, -78.1272953812706, -85.85545438627958, -89.30587144190069, -92.90590394398903, -93.63083388385274, -91.8644929119412, -95.26924857401164, -97.0710469181336, -98.01148078956652, -99.33043660296804, -95.58776817681839, -99.9570097527269, -101.45494093095093, -101.51838334751548, -101.00386616525799, -103.01963069818913, -103.20223925731209, -103.53783076500916, -103.48065647812659, -103.97797518531912, -104.58942778240602, -104.46991277190502, -104.59813972158683, -104.56685024229951, -104.69893799348945, -105.05669000016238, -106.17061117835001, -106.43303821862656, -107.39468286383597, -106.2899368267905, -105.7863846168199, -105.17170638885071, -104.53818172761852, -106.70340956723133, -106.55444321137247, -106.67654843051936, -107.79888413750199, -107.86424326005849, -106.09722609215336, -107.71648639013972, -107.79500725395155, -106.17330953637067, -105.43663624517525, -108.04970689199158, -109.92106271611999, -106.2505251183406, -110.60221373795562, -107.11377887451098, -108.4126937286195, -108.37794745021417, -113.22457316369011, -106.38281814065472, -107.55385617652075, -108.93026538982782, -106.19334142366085, -108.90462602264525, -107.63084712174981, -109.12192537022624, -107.90627042480016, -109.44472079190832, -108.91731458372392, -105.74102972706788, -105.74407510394178, -107.5989477192235, -106.2838630137392, -107.46190542725505, -107.38881299750702, -109.08024783239452, -104.97871836903269, -106.65424712290651, -107.04966019632134, -106.16202578092883, -102.98374199247179, -99.1568704142098, -87.07383781389657, -96.41471411313154, -102.65176579899618, -107.65674867775193, -102.85397890306213, -107.58658613411464, -104.79044898833125, -106.65282019869865, -108.65027966345534, -109.46169054950127, -108.69969979291741, -110.4048706652988, -108.81020193837274, -109.42808902484134, -108.85398463561398, -108.3849716744813, -109.1844457168716, -109.32787859535676, -111.01992124870878, -106.64843449415699, -108.9926343573667, -111.59837822080355, -110.57121677672183, -111.17280164669164, -110.68901970586144, -111.69013245592781, -109.90200577018311, -109.3554172126163, -110.7515368822992, -109.2863324212524, -109.66209701262974, -108.50795548698007, -110.58126481096504, -112.36093896766921, -109.78612141282203, -108.85120530917233, -109.91424431080952, -109.84698632196245, -110.93960894966105, -109.77214706089354, -110.30762971422381, -108.77791302937449, -110.79522659679036, -108.47242514643455, -111.20629758187835, -109.05996769621125, -111.13574821570619, -107.79388178889101, -111.5768481279296, -110.52058839597171, -111.58729762739313, -108.99000864386126, -111.6585121505227, -110.50715371958135, -108.87151956974363, -110.30486244367107, -108.32392040018144, -108.1769507919999, -110.43198471512189, -109.81454097966842, -110.26717009815644, -110.82924135076777, -110.34103661156989, -110.0692667126265, -109.34555682020833, -109.1694484721415, -109.9940980324044, -110.81940616215803, -108.21162003366862, -107.97087538330561, -107.55312461506225, -110.60339321606872, -110.09004629292225, -109.05860430198882, -113.1412749514818, -109.81628200948371, -108.62343219429849, -109.48172424209761, -110.85978755785311, -109.47778611557064, -108.81728552967951, -107.47864241666747, -107.61735128422292, -109.62511618983821, -110.32417726356636, -108.24287897478176, -108.60460879530194, -110.2181558494026, -107.95550802888957, -110.80234484950323, -111.09955733353904, -109.43923052503506, -108.98949130235951, -110.05778199870154, -110.36224432927585, -108.13523430027999, -110.681114579241, -110.49106131529867, -108.73493328004297, -110.07663907252234, -109.9968931372618, -112.10715231091008, -108.80994125105168, -111.63774865669372, -111.54355694032755, -111.64024217585788, -109.34986300492378, -108.88053713185408, -111.14370830146245, -111.17327416167232, -110.36311492990576, -109.99414559884396, -112.96912007380595, -111.43191437097785, -111.71327312809349, -108.77202323682606, -110.25970374932486, -112.59574277180732, -109.77247894866957, -110.09219852365874, -111.7197662726775, -109.85454092697009, -110.06789440397942, -110.38055758638309, -111.04251386932805, -111.54279434240568, -109.74385329575985, -110.98924544863415, -111.17898077762852, -110.98364252730245, -110.75024385843372, -109.24766708578407, -109.67753987004863, -110.6537235844391, -111.84436313010086, -109.12654337292446, -109.65519521121124, -111.1845162935778, -110.5009101465602, -110.22980642268818, -110.88540043278346, -110.29249073109453, -108.80459864528464, -107.49372141121728, -108.50353962704821, -110.00730069533373, -112.012876492648, -109.01283702976382, -109.07442203290057, -108.2961442983685, -111.60962842680907, -108.84312815413224, -108.6276642979969, -108.75132871638827, -109.30004903844721, -107.20359872252604, -109.12175943862074, -110.43914247337625, -109.55954680842791, -110.37116786618797, -108.55907813251434, -110.19249995041955, -106.95269845697632, -111.07027929458712, -110.1073996792702, -110.61729280468039, -109.6419175310234, -109.47995019876329, -109.66602827275211, -110.01953864498805, -108.45989120418268, -109.79778555296474, -109.94663827736616, -109.52410616839379, -110.58014441463794, -110.09182359045897, -111.0487262011397, -110.49609187214915, -110.6114701312941, -111.17752423063314, -109.74965389041003, -108.58973724447526, -108.84292130035902, -108.90689510645983, -110.69840140049361, -111.30494362640982, -111.00224390075273, -110.50848328538423, -111.59232911931113, -109.30826761863756, -108.44510893127558, -109.63744704504391, -108.95037574307332, -111.36486409910674, -112.74508631930381, -111.03952454593811, -110.57133212903979, -110.59969855145111, -108.25570461975128, -110.44617635200193, -110.32190307214704, -110.95204704643322, -112.0595421753479, -110.45342552693265, -112.50183987758867, -110.08217804938009, -108.90353583389084, -107.02032313792242, -88.3334978919524, -107.92027625495886, -109.83148570028482, -110.30427997450572, -110.92855407802753, -109.67404674397338, -111.03606345823586, -110.58277018943096, -109.77692362669393, -109.39170901729935, -110.20711662408928, -109.41601946806779, -110.34213214925832, -111.2283900972803, -111.51682597931386, -110.47069117801351, -110.93808974285523, -111.11277478000933, -112.50698886748012, -112.12918507523611, -110.46316790252011, -109.9387334819968, -109.78723249688426, -107.13037722044297, -108.16132376075751, -109.07255491017162, -108.85068428558272, -110.28038153100799, -107.77611023481016, -110.69754506886444, -110.09495581837979, -109.21214884561816, -112.62718526248648, -109.22048725312992, -109.17793923163308, -110.87372121410577, -109.71902632604333, -112.61041177225496, -109.6374750969677, -110.74738952366951, -108.93404661877067, -109.84938675700889, -112.25316361679832, -110.30788094875312, -109.26929069321925, -111.20853536783942, -110.05212566057608, -111.72448131932816, -111.55474439772887, -111.81988954424324, -108.44452452934028, -109.21897824914645, -109.55634869894358, -111.36318572800242, -110.05777399011298, -109.64458567712875, -108.73315084760529, -108.93332091319675, -108.4816455312154, -108.80120578498936, -108.1804470361839, -109.7177707524778, -109.31977709844544, -109.33603116022124, -111.46120546572519, -111.7480378245176, -109.17907150677627, -110.47970652472505, -109.73718750984082, -109.7935026884937, -110.40458408612054, -110.91781389491092, -108.39352075861481, -108.27512197925346, -109.59155075404814, -110.40183121737397, -109.25423373270381, -108.37769008625712, -107.91335995938509, -109.5576520703013, -107.27392145737491, -110.98592762117059, -108.41809950647861, -111.48163889400448, -109.70961684769624, -109.22952568656495, -109.76504719131209, -108.86928627177666, -107.97855299877004, -109.8412204399902, -109.6690048999326, -112.28329030175193, -111.54977099314607, -109.55689540119126, -107.93716711232997, -109.84247640855929, -111.5098351445789, -109.14317615215809, -110.28319116384824, -110.57901069942578, -107.2890252845352, -109.66754569546274, -110.15708115946433, -108.83782190109405, -111.60783857760667, -111.46884385151185, -109.21985333366634, -109.63605494317056, -110.87999187262697, -112.26992029775087, -111.05491095860552, -109.22795442529183, -108.99135781712076, -110.46475190704264, -109.35746113713218, -109.29125989270668, -107.40922407684049, -109.24391685563656, -110.41554602144217, -110.68952735085914, -110.62457364102458, -110.39856310555466, -108.84256124354566, -110.01614601335088, -109.8071306678428, -110.2804500736802, -108.76205061238203, -110.3962440297242, -108.98253716257014, -109.32990745926702, -111.17276766165281, -110.41113652364085, -110.36616199963426, -112.09767002991742, -108.43599666470733, -110.91876588140981, -109.05329272502944, -107.07198690769708, -108.72934463903034, -108.6666471996132, -108.97529973794413, -109.68895260146817, -109.2658844652487, -109.75690097249196, -109.38585024123027, -110.17593039468063, -107.87223111061134, -108.15261097418302, -110.09277437980633, -110.8665497655964, -108.43061614348413, -110.3052458526819, -109.22446919161898, -110.51909692711594, -110.06620699121913, -109.53439413051383, -110.31952463872884, -111.4732125902982, -110.41443606663168, -109.9579358088152, -109.930778061577, -108.5473214465574, -109.34719220288939, -109.16964653934396, -110.04824158176345, -109.42616539603762, -108.3556027482992, -110.62331917617789, -111.3652147859356, -110.12362012120938, -110.13175448595814, -111.20110099151856, -111.50643914621541, -108.11659117128028, -111.06037600347967, -109.03822892917451, -108.25678204604324, -110.82608024151122, -109.15887945314851, -109.88255674562845, -111.18322672526185, -110.95836040044516, -107.91535345885436, -110.66285812468733, -109.61906549925033, -109.58059721670746, -109.65198009505977, -109.65950565672951, -108.95264505276342, -109.23343669003113, -110.74308548011575, -106.39170014998685, -109.61471203101753, -108.24258770956924, -109.84609566640096, -107.83834185503922, -108.93052854090027, -107.55568820082641, -109.758551082242, -110.65892780872205, -111.99907420485852, -110.71043004141137, -110.62257237494617, -109.15610413532767, -106.87403836327807, -108.19175324576331, -110.27819583792918, -110.23918003777561, -108.29703377268754, -110.07182881114713, -109.60256111108491, -111.00394752430006, -110.30750337485472, -108.78309624082331, -109.24103013025798, -108.76979253891403, -109.91618737478264, -108.83915940855513, -110.92536150834754, -109.72250903746432, -108.96533939688658, -111.08949280651164, -109.20335070860871, -109.37826578362439, -109.77953166722301, -110.1867310744785, -110.07114559821346, -110.7003631567182, -107.86455899696074, -108.94113264174617, -109.35999427135138, -109.33627364788704, -108.96588828808375, -109.08716536982254, -108.73575375369026, -109.47770132070654, -109.83726171472907, -110.73516506891792, -110.56827134787686, -107.65667508354096, -109.30200115708924, -109.28406803847896, -110.55374624323233, -111.2017766725333, -108.50851279608973, -109.79494403619485, -109.08320018013063, -110.21850624918747, -108.4652936555984, -108.74837610538873, -108.81326140648238, -108.83830180036702, -108.785270477003, -110.01845876259073, -108.76030368637825, -108.57879884880157, -110.6610608456059, -108.74669367794318, -111.55956030460833, -110.22906685783455, -110.48411613865359, -109.48060880085136, -112.77556331479562, -108.2676071206087, -108.8571136162698, -108.56944905160177, -109.16406757131058, -111.42259299295839, -108.25216316582294, -110.48487127684025, -109.69532331373831, -108.13992755196784, -109.2987762526628, -109.82536192480795, -111.28650061088359, -109.12820736404241, -109.37960655471406, -108.96014976926716, -107.97535047619023, -112.31953123574708, -109.06198330523004, -107.52722515967098, -107.31555373665437, -99.89671790804692, -107.44442600896275, -110.6549218761941, -108.02265794322076, -109.63582761762919, -110.00574746987859, -109.51565124961209, -109.3550083591902, -110.4541529175301, -107.85799722437162, -105.1197113090786, -110.25038075579738, -110.39710812865657, -109.3618876098789, -107.6131301952152, -109.21529527621463, -108.7995754403799, -108.48347353145697, -106.45678488065816, -109.60427918561142, -110.81194387812535, -109.52215044127382, -109.88751598659705, -109.30205143590227, -110.74984456751768, -109.03952092986351, -110.69170786328897, -110.39236248162467, -108.65456161733339, -107.60439764386904, -109.97367926606955, -110.2754359970249, -108.81546418006434, -106.99691398176165, -108.42047325825182, -107.24499915944605, -109.28116135603187, -108.70650358781573, -108.05516916105047, -107.20893100196241, -112.07029265690055, -109.38099990478445, -111.53461820465232, -108.11312509555277, -108.76714028655223, -109.89565008459624, -107.71879172001115, -108.08434857420214, -108.79142773619792, -107.25153085963885, -110.05595039449301, -109.31604222314259, -109.94405791565286, -109.04715370361387, -108.89278831045846, -108.84682466376424, -110.0067927716526, -107.63768959294084, -108.98109382020348, -111.4720219575084, -110.76023788797733, -108.78599647633777, -106.59726674064618, -108.66715709719243, -107.99134359630926, -110.11396713841884, -107.21091759882775, -108.08576824949941, -108.80217666857972, -111.72949572713338, -107.33126296136014, -107.33731660097102, -108.04470462977443, -109.42963925921418, -111.03517778720736, -109.55293581015796, -107.99948151285162, -106.59480934999681, -107.63777243313498, -108.96490626068824, -108.8948210299064, -108.30870516747477, -109.13612869658097, -109.59971429402015, -110.2571461001396, -108.7655464686992, -109.81144209568883, -109.80796806645141, -109.20948481699544, -108.68653880881129, -109.26329796696166, -109.22428132233863, -110.12571678351438, -109.14615461144786, -107.08261621308327, -109.11338327144382, -107.75421565039201, -107.45291780756361, -109.00477000647248, -107.41031480478154, -109.98948062864928, -107.45953654921264, -106.37522884807879, -107.7786128523167, -108.03610987358499, -108.05926797128022, -108.59400205554164, -109.89620453365603, -109.03811240487515, -109.96909236705363, -109.28212981785472, -109.6772152101994, -108.26493868190678, -110.55558039199732, -106.6252818398841, -110.19075011176416, -109.56520012524705, -109.8023423576176, -111.2697570480663, -108.26752571816566, -112.00337375484828, -109.85709226796116, -109.36922081321148, -108.8424844298318, -111.2512302139209, -110.61775974680471, -110.22501328999012, -107.76874906708105, -110.71023653476604, -109.4025656165291, -107.66667684986125, -107.59759854092948, -107.94763263251238, -107.3888591871119, -108.62692803125044, -109.18012867988286, -107.78662871481455, -108.5072814073944, -109.50348958982907, -109.95177634938378, -107.78756251182895, -108.03865042797304, -110.1814993556385, -109.34937567548833, -109.52162025123161, -109.50819015441117, -108.20953105254624, -110.52154040214435, -109.3324404469266, -109.2696617050831, -109.54675609195674, -108.5940367000989, -109.40184828664549, -108.2518305610941, -108.55972691669434, -109.03647225394408, -108.48166656251695, -107.42023429066523, -109.42453054302521, -110.09532345960083, -108.78315822119662, -109.97508586102265, -108.22687406536997, -109.17110028890058, -110.15390449992647, -107.88577458651508, -108.28851074361447, -108.52030295163331, -110.03496861709483, -109.40014319167584, -107.73048113044877, -108.17571683963915, -110.34839852994926, -108.55894048192191, -108.74107339998285, -111.17734138993401, -110.22946440841412, -109.45511941802884, -108.0657300641843, -109.33797363184166, -106.95974095511333, -107.93068343723691, -109.78867669512647, -107.2087297624043, -109.542665021243, -110.05035859052961, -110.30235238883523, -109.20586170783808, -109.2796396673401, -109.14260673746566, -108.22019460542734, -109.99011886871159, -109.89103038547285, -110.36964772493243, -108.62340319923602, -109.06779821699769, -109.21830861066148, -107.7402395759509, -107.7178850938205, -113.45665085929117, -109.24039191621704, -109.30387033426037, -107.61849760982835, -109.41430582703529, -109.11482836392241, -111.89328423764577, -111.84653367963301, -109.00674896486915, -109.84488648739638, -109.41914760797953, -108.53442910169935, -109.66883322968232, -107.68762956301386, -109.82583101109167, -107.83405397804887, -108.78052031141966, -107.37842078941692, -105.40843158543845, -108.81430898189338, -109.57374640194516, -109.41111270322058, -108.82621700188898, -110.2552502368822, -110.23903890097205, -110.52171662278697, -108.21249857906324, -109.97268479379733, -108.20088823960992, -108.85682002802234, -110.11642849164285, -109.94087886999255, -111.63180946270296, -108.20899499456195, -106.73341567332112, -109.90003508676807, -110.14688274481229, -109.62259307329889, -107.57811196819495, -106.88584597822792, -109.16132624528932, -109.78677836397806, -108.59319344451784, -108.55877448618652, -109.46883711353044, -108.47309455543844, -108.09487065732198, -109.82219079158135, -109.63780237877428, -109.28348848877269, -107.62893405379826, -109.46986737961593, -108.03089712610223, -110.3931917410696, -106.06970126043262, -109.41866550703786, -105.31710372440419, -109.20218082282653, -108.28467118008108, -108.80026326744611, -107.40729224715713, -111.07322915141532, -107.1057186510818, -107.98286374205958, -108.51298722989311, -108.69632670891366, -107.96509231988331, -108.15882223414738, -106.85862416470376, -109.70705792539056, -108.64519930633055, -106.78708421443504, -109.43552377900174, -109.4474526498122, -109.10135248755788, -111.43316642580763, -109.33457343739448, -110.23547887071898, -108.95690647379442, -109.21159903769149, -108.12969562680841, -110.82751409340537, -108.55724349027832, -109.8796329603075, -108.50369978374582, -107.43145467247209, -108.60003323209516, -108.77155705999647, -109.33806063660796, -108.37500858898439, -109.65641721611547, -109.81905873737344, -108.03483220769625, -110.48028107566635, -108.60527372219985, -109.28768201151478, -99.8804125587218, -108.8913334544964, -108.23534920737794, -111.07646463287153, -108.59029790589766, -110.3405916586831, -107.66387718565608, -108.73793152614131, -110.61440166477816, -108.76211382544581, -110.23236978486065, -109.10669297094852, -109.15247609779597, -109.00539004923506, -110.14424353412238, -110.55445060661157, -109.48721312920799, -108.17040942305823, -108.77592227268228, -108.77130256578067, -107.82494496098512, -109.57266989523707, -108.75767497229612, -108.13688624150026, -107.8280716764963, -105.676279602552, -107.6370316684844, -109.73508547021689, -109.25365178573009, -108.86767843317584, -109.70969944273735, -108.91917504090888, -109.97734866522867, -112.17308993943783, -110.28356299479682, -110.7927103729386, -110.30837645846702, -107.56364161860179, -109.50188349731121, -109.36065627483853, -109.75389877587511, -109.81713476007774, -108.14524057525358, -109.43832376796216, -110.89342891210596, -108.15657882822792, -106.84106061627887, -107.83091759905821, -108.61794662682962, -109.57142366843581, -109.85402645528154, -110.12877022469837, -109.19414429724044, -110.56168468006764, -108.74720588273881, -107.90448559921305, -108.54421401507743, -105.06700039841249, -109.17937358052484, -108.94317576365822, -107.79410219455083, -109.24955437598658, -108.23334395173994, -108.98759227946937, -107.05986359444529, -107.20956512998849, -109.00295831471958, -109.43119556916457, -108.93348410522628, -108.99932477701081, -106.6448790859128, -109.06877251308666, -107.67053918439544, -109.15052780608639, -110.16878033319385, -106.55101141640301, -108.02811045752685, -111.52173447126572, -110.16854119242062, -110.93164036911654, -111.25979320890855, -108.82629030379024, -108.52004501839738, -107.09697056562636, -108.94233383169858, -107.37962568194772, -109.1239201710643, -108.93949898577122, -110.62573772949195, -110.09592372075662, -107.56136391005947, -110.45600430869621, -108.79481000016084, -109.41462449554598, -109.30248158488335, -108.70735295493108, -109.9174743694956, -109.94232543385962, -110.71725446170196, -110.0346196158573, -110.34814317845934, -110.6651078322521, -107.55409880424479, -108.71734776861287, -109.50902203986271, -110.40207542979611, -108.7847687630861, -111.10599488129682, -109.30824728923263, -108.20134064331717, -110.55959112431609, -107.77099734327174, -110.23862843385446, -108.48520797666865, -108.54205896654946, -107.79288769037599, -109.84022250170581, -108.02758364115576, -109.35132492327935, -108.87009749667932, -109.86905123364855, -109.19826752168308, -106.835240323691, -109.37910022114056, -110.80633973102931, -109.12703823829597, -111.07432699570984, -111.8064506085314, -110.09349947650527, -108.66467295777367, -108.75119108236053, -112.63983351316729, -110.90940743670113, -110.27973159222081, -109.57141664526549, -108.61645363771719, -109.31742355616147, -109.5839599160637, -110.01188998365383, -110.01923429741011, -108.94779759137936, -108.26169431000017, -109.24553201026085, -109.95709526422822, -110.68677343596859, -108.7678734483002, -110.47090469179284, -110.31604700116512, -110.10256600741997, -109.76634647265719, -110.8830805828562, -109.94609564072982, -109.20662382740542, -108.12492970530919, -110.5274435478767, -108.02351960398035, -110.6264936805739, -107.14559226383577, -109.13821777857531, -111.05324489472586, -110.15190797512811, -107.96366234783144, -110.03950681967147, -109.17476300510336, -110.41251816187909, -111.39219865477246, -111.32530426869943, -109.97369363558423, -108.98666403063845, -109.62049358645565, -109.58130494498671, -111.72738873188874, -110.39825891106616, -108.57430325757545, -111.28625510212446, -108.77421250595326, -109.75025415031793, -109.51948456745635, -108.82129398637998, -109.81362137198361, -107.86292494316123, -107.49318292857053, -109.66948564589373, -109.54288390056654, -107.99912445612077, -110.3497559614379, -108.00549349666127, -110.01361420523357, -108.4977916421456, -109.67078387286976, -109.85678367732866, -112.01237658746248, -108.4855625950998, -110.84880875737286, -110.9178674382154, -110.44187536727453, -108.75076921971127, -110.04946286646651, -109.99780941000827, -110.14242932305507, -109.56343773672316, -109.6278993388131, -108.77419573790174, -109.10543670530926, -109.7801848627463, -110.30733124104881, -113.13440550301436, -109.32709134514755, -109.74136656933283, -110.01525283266193, -109.43924662938396, -110.25325289253, -107.75460576671303, -110.60057027395933, -110.71458404922404, -110.15788509050662, -110.69167485018224, -110.96006652476157, -111.01156633983031, -111.6058448010008, -109.51364005052672, -109.76058205940885, -108.43421621088261, -109.47973949170208, -109.25533250208288, -109.47422603921065, -111.36411644613841, -107.27566171102698, -110.45098686173688, -109.93589296291184, -109.03803734663714, -110.53118128434016, -110.2408872254969, -110.0532234862915, -109.94185495614619, -110.2662004220774, -109.51094016962288, -108.5210104215432, -108.13691752270934, -110.18460088390265, -108.32609309150783, -109.89652230508281, -109.80923900768477, -109.01917388968883, -110.01248300968739, -109.43415605440147, -108.09823485138017, -107.40637725320931, -109.40632232658412, -111.97981999127656, -111.16609811629485, -111.64500793960192, -110.99793748693381, -109.55531276386903, -110.2535662621666, -108.17429802469516, -109.09425673355422, -110.23187110421917, -110.55358397926925, -109.93461124753053, -109.55604345832225, -109.44569510408274, -109.72185151080762, -109.52963702944834, -109.2303630328152, -109.74819502244243, -109.3932530349457, -109.17096788339686, -110.46153727064616, -113.1073731246639, -109.43753070459397, -108.13332547768168, -109.42294574929969, -108.45798401969856, -110.29453435046327, -112.66249403705643, -108.78314667434937, -105.9634478773668, -109.14327524669528, -108.50645190860273, -100.81571594994128, -104.4482859840643, -110.68926237051092, -109.12362553230196, -109.45234390564677, -107.91461416156068, -110.67788819353727, -110.05744935668449, -111.78333392154664, -106.83628914455993, -110.11115457346548, -109.13434608275826, -110.80006861194663, -110.35323502651462, -112.29149906501372, -109.01656376530778, -109.30871662948859, -109.79736315392456, -109.17848983603582, -108.09752397056482, -111.6039030763455, -109.27008844877828, -110.84475733314184, -109.72393917557073, -111.31060762894991, -110.78858793807466, -107.12841545099752, -109.54510865218204, -105.2805426080281, -106.28514149354733, -109.50656759582803, -110.14700878401054, -110.49737016725709, -109.19811547071924, -109.92527399676051, -110.7961615015146, -109.7447227818197, -109.49432012009893, -108.714081576733, -110.09766801550917, -109.08448507943001, -110.36154838733857, -109.86328656267403, -109.21144237434696, -112.4145136888034, -108.57567151011159, -109.66748589540896, -109.72985837578446, -109.29989238126763, -109.85868902806475, -111.01778182304162, -111.23625326328558, -110.01270868104203, -109.27067928081415, -109.71171312410247, -109.28697459293629, -110.67868067201007, -110.91353786857455, -111.21479955051575, -109.11315965407708, -109.40418681804496, -107.80511819596003, -107.37201025889816, -111.81969609169838, -109.89875624306032, -110.29328043898657, -109.74853280072202, -111.39527865400605, -109.47746221101964, -111.75141177452517, -109.31325306583483, -109.30117448911659, -109.3997781364162, -109.45356931295724, -109.60585285774386, -111.33951689512735, -107.74187210470228, -109.62706021606415, -108.72139655505221, -109.79552836110567, -110.64354037499807, -110.96138240913136, -110.02215059889615, -110.92978442698893, -110.0620778287114, -110.85019647293322, -111.77397403227091, -109.81257196800128, -109.15643451383403, -110.72777566469594, -108.7463769025616, -109.80959395914073, -111.24500986151126, -110.48863498350322, -110.30863780110901, -109.79331354195703, -110.34087081762074, -109.45183222569266, -109.6440990067103, -111.15034876658994, -112.14912485578341, -111.8886180186196, -110.57054820211916, -111.07556239924551, -110.5872832735073, -110.28912501038172, -108.91501133754849, -111.44575118962761, -109.90799859177967, -109.74421995550023, -108.70941446115883, -110.28822893097275, -109.70039554000401, -110.33701797570251, -110.79445894683306, -109.57694314608153, -108.816904416038, -109.66517126767175, -109.39501469321644, -110.85775022889956, -109.3689402795614, -112.09107318723095, -110.67985626248422, -110.32971146814747, -112.08166943494875, -109.93955548712543, -109.31722953035252, -110.2062913031861, -108.22565380081006, -110.680898028151, -111.95386604441454, -110.83354130587097, -108.5873626748948, -111.97536144124408, -109.23944159551515, -111.57859477689586, -110.80135186615524, -110.4800953731021, -110.14040729648133, -109.25873050390551, -108.87000960474569, -110.97091597211167, -110.15787270199012, -111.62434537618091, -108.5421625277294, -110.42258666403919, -110.96896115868603, -108.98253068925274, -109.54245055160168, -110.28051096122468, -109.48060498658319, -109.77618362117276, -111.64513838754992, -111.13945484239875, -110.18094280356001, -110.43757222770748, -110.81588360154201, -110.11656805555333, -108.47936291282355, -109.16476249859961, -109.3549985917136, -110.77753190334253, -111.46065694661178, -110.40387985996301, -109.95673803226478, -111.58660981285446, -108.59894875229345, -109.37333363882607, -110.26849699991793, -109.30500469266264, -109.23789020998296, -110.82000706486865, -109.25927538839868, -111.03285659417519, -111.08899832832414, -110.69361682858042, -109.45187168573815, -109.9614018482838, -109.70209527974106, -112.11903952100165, -109.59713611623246, -110.70292028698111, -110.12743849746808, -110.63315585514292, -108.60450276298175, -109.32832664986026, -109.99753023477764, -109.46644696130294, -109.1781290160558, -111.58830180575129, -111.67229040267557, -111.3750024136205, -108.33616679452298, -109.99797067800029, -110.50892429124391, -108.66074740829372, -111.17094662568759, -109.87538933985836, -109.152526628291, -110.44623159817101, -110.21603106403009, -110.64376935639365, -109.36897426842583, -108.67303022227141, -109.89327693080823, -111.50442955563923, -111.37532237834381, -109.38132821290205, -109.73509680539144, -110.53918379735906, -111.22869870340647, -109.39977573957616, -110.3674665334106, -110.5366125953241, -109.99025356764304, -109.97300035646616, -109.87631077033762, -109.64608829594286, -113.02486102973394, -108.26250283140733, -109.62234918138763, -111.18766216512655, -110.33666026406992, -110.5808115327039, -108.2971671321189, -110.10964334161903, -110.61254021379767, -109.89852549557533, -110.16562049054073, -109.41433790018287, -111.2453823439446, -110.45554802599901, -113.11454453784393, -110.7333866145056, -110.00858191882439, -108.54745315874294, -110.08430415376903, -111.9006972727596, -110.3031506154679, -110.26331790366497, -109.36797925566673, -109.04860552478912, -111.83514212681175, -111.38960737633833, -109.01429665187288, -110.96404839103826, -108.95488871107163, -109.09652004914592, -111.884304581971, -110.57566691021339, -111.95113404442795, -110.13677174050159, -108.10078686353354, -107.69442565416006, -112.42676605669463, -109.12681161784135, -109.23120766087519, -110.57649395555585, -110.22143082743162, -108.40065951773644, -109.46923168308618, -111.39095086729745, -110.46375658526013, -111.45145283328486, -112.22610823637353, -110.61090190564383, -112.22250292674809, -111.7379343196361, -110.18530386733481, -108.93867365671692, -111.89304844956082, -109.06146134986984, -110.98405731832798, -109.76366821333497, -108.08326795663608, -109.95041147835065, -112.94140614324155, -111.79814935135965, -108.07337559063119, -109.13733403265212, -111.74906646037496, -111.12228668433455, -110.02899450462209, -110.22237716929811, -109.0224776891049, -110.18135850497721, -113.32516073881047, -111.3576490243877, -110.60510094465171, -109.6935518470342, -110.36313473154901, -111.95933240129618, -109.49625308071019, -109.18827910216122, -110.54311407822692, -108.4811035913567, -112.81280225723607, -108.86530665787413, -110.85796435061886, -110.40059714639627, -108.19250716343407, -108.96956521802292, -108.61281798886506, -109.78061525370413, -111.58885511891798, -109.06279169160345, -111.43043988466789, -111.63169336321079, -109.54702536206447, -109.62860636296405, -109.47865811135546, -108.02265793654806, -109.97461304995515, -110.72549884050886, -111.57309413919933, -110.03317891949746, -110.39570411598524, -110.27606115470397, -110.63294457306095, -110.71821689302902, -110.38076268941819, -111.51223508887897, -110.40703572670697, -112.24933273737743, -109.74954300082398, -108.46020292937696, -111.05315219575881, -110.38635148390118, -109.58268303790976, -112.34211536832117, -108.45894118755307, -108.96463982695337, -110.56040438523046, -110.67803313671729, -111.07349872375121, -110.42184162876096, -111.82081126435692, -108.85923651136297, -112.57723799596502, -113.65690874668172, -112.62314325834605, -110.70357529341362, -110.959925221544, -111.26336183001875, -108.1350700630152, -107.94545932312926, -111.17610778209841, -110.20386728310686, -108.55646511121591, -109.8400922569145, -111.73466587035968, -110.47272877573613, -108.33011124048193, -107.93042857580332, -108.60928277989103, -109.25240966798974, -108.96403833602028, -106.94222615757475, -109.37086694261907, -106.72743097285155, -109.03160193412796, -107.3549903889451, -106.8543848510082, -107.83503929060929, -106.30745467433752, -108.36915807168845, -107.13065938379303, -107.84769200880969, -106.08004345082777, -108.15244601930225, -108.37254117816573, -106.57863034819223, -108.1283698227614, -108.19776505569902, -107.58283412238643, -108.17365133196301, -108.6794309781181, -107.91552140588759, -111.60122989270022, -107.04360635941174, -111.55535949001795, -109.39870426166594, -109.55937904851662, -111.81389508925734, -109.88957041098786, -110.84764586896561, -110.59130246272693, -111.15944135223884, -110.19496154041607, -111.51861903129362, -110.74798816525838, -111.37312965175558, -110.10842817220238, -110.73198099204856, -111.36708667993291, -110.30840247819665, -110.11744489669044, -110.55237850846444, -108.2073528237766, -112.70750856801911, -110.99917956040802, -109.84949484779976, -111.3403161887679, -110.08924435263565, -110.17749213365616, -112.10849123224503, -110.94270741299202, -109.29350963424746, -110.33477486966507, -112.19620157705627, -111.45484078395934, -111.86858843505124, -110.22491147345858, -108.96177661263177, -108.67862820579893, -107.55155410582937, -108.27984439169573, -108.72682528077233, -110.64231212183269, -109.32873093119183, -112.98564364754564, -110.78933114228725, -108.50921025910479, -107.91087245586935, -112.57350030929283, -111.75871577457525, -108.42095298945462, -112.31266064114303, -110.1295657579673, -109.67444664474456, -110.33749884929306, -109.16098218724147, -109.63554874360221, -109.15892392675141, -111.90580809179818, -108.81196712336858, -111.42223552606656, -109.90571484965518, -109.99739812086352, -111.64103850263211, -111.31463957090885, -110.61247447444549, -110.20960333715526, -110.1707327818923, -109.70412636554525, -110.97278093107532, -110.24386747740314, -109.81378546061525, -110.83784085086458, -109.77357954318757, -111.22663832948885, -111.14563050139252, -110.87152231402447, -110.34246044319893, -109.97174570657546, -110.23599592972218, -111.08206161770731, -110.0073315341242, -111.11748366902188, -112.04005964728601, -109.81290191679287, -109.68543639040858, -112.01143296194752, -110.13641850530031, -108.19348942447623, -109.7534468948808, -109.36697824644176, -97.56454580435337, -104.97829040517887, -108.1539132982256, -110.048991273122, -107.46172505860011, -110.49269280640675, -109.94209901400029, -109.38576869679022, -111.43699124347364, -110.89973083498887, -111.2994445418276, -109.25144782032437, -113.25676258473536, -110.82078737428088, -109.97779571182073, -113.36294799183014, -111.38584551238931, -112.17267897274873, -108.56430946159155, -112.06841286528645, -110.36822473102735, -109.54758527532016, -110.48190506674653, -110.03535695860182, -109.3951469796576, -112.41910682256774, -111.38124138857238, -109.37850389100952, -111.65544568836181, -111.55876881606889, -109.3029209617236, -109.20030046194076, -108.82610577621037, -110.53329453526098, -109.96090595542142, -109.67834229432077, -110.62303603007352, -109.8388817181171, -109.22430039793213, -108.92749786663613, -110.05794249283548, -109.58534943218437, -110.50493887507297, -109.96373022997366, -111.0645036323456, -111.28501675364454, -109.77386932343008, -108.8952247140968, -110.09242801628717, -112.90943444063141, -110.72299296247249, -109.39094335967056, -110.95165384057718, -109.59809519359453, -110.4978602309597, -109.67109981692639, -111.2489619905986, -110.0937750887109, -109.76771021128954, -108.32976315018955, -111.3058145792439, -111.09464974601362, -110.99797900696136, -109.174315000222, -109.630351559617, -110.26289147175856, -110.22688407202517, -109.96748050100612, -112.13247633583758, -110.59994952890855, -110.93023020153811, -109.22457750926695, -110.26162558926984, -110.09713110375579, -111.73858994918328, -109.78183160058515, -109.7603471824367, -110.96016892586911, -111.23309626937036, -109.83093663960678, -114.05354944347246, -111.58202863059464, -110.42281828744524, -110.9521484732059, -112.5120328206343, -111.614891937737, -109.84428787405484, -111.61119567831453, -110.43095563229411, -111.71833448430398, -110.01132196809407, -109.37558169247951, -109.14091380022785, -110.42663661754088, -110.3598013572826, -109.78207135281417, -109.94058843992468, -109.88210328447205, -108.6217811850147, -107.17834387173707, -110.6447226986756, -111.10704778101115, -111.24396771977769, -110.47849395539598, -110.75150631628034, -109.67662689396347, -109.23145032835053, -108.83780193265358, -109.43468321661163, -102.22521103859944, -106.90009867479111, -108.91580608784525, -109.58671397003187, -110.56692028436989, -108.75103142680105, -111.00795573084157, -110.75039085328763, -109.48222099288613, -111.8621134816908, -110.26507966786443, -108.885924716389, -109.30841399453053, -112.3188631425597, -111.05677697153163, -108.8268571902449, -109.63028152237679, -114.82339015806369, -107.03435216376964, -111.34847692589166, -109.61354114874855, -112.32687758049907, -109.59816404231358, -111.64248480241805, -111.84075757907273, -110.44017657636552, -110.15181635726277, -111.93813663582833, -109.11826378836209, -109.99779889778326, -109.927119030584, -109.4389650887841, -111.52448814187727, -111.38736268499642, -110.51920914917922, -108.64230614681055, -108.90307263595304, -110.57246891832371, -109.65575340646116, -109.80359672370373, -108.83368585528197, -111.09385004343437, -108.83430005497769, -112.37784208819113, -109.50005381621696, -109.67421750136593, -111.39664088797532, -109.70867599669316, -109.52498993629875, -111.12341349673187, -110.0484037026941, -109.55138667646308, -111.06614422098669, -109.4785941493091, -110.25724082617013, -110.93950616855716, -110.53487953881397, -111.45722057988401, -110.32393446412904, -110.34361936710438, -108.6610336097813, -109.53631603696368, -108.06930707969195, -107.68056561368934, -108.73860971027449, -108.87111384617579, -108.40433837098611, -110.55999576884835, -106.83832061167207, -108.28786975902513, -109.18482905697472, -107.81071696594883, -107.91047268802457, -108.79613111673706, -111.05361322310213, -109.97897453479862, -109.12920563729425, -111.20538391490288, -109.26286135293664, -111.31400407177502, -109.92167984752287, -110.70854322826071, -108.59406515713611, -109.69371333227458, -109.36664873267313, -110.35521729513704, -110.40667924006368, -112.0181844636846, -111.01529188207431, -110.59246505728431, -109.95068312717868, -110.75807466894047, -109.58596443762707, -111.12127793384956, -109.59041634463125, -111.56255571372793, -110.43405578864342, -108.39660324329928, -111.1420710307505, -113.64788483868595, -111.67645688353934, -111.36878760365944, -109.68523694561108, -110.11608766310304, -109.25670490330123, -110.73546181099229, -111.77855039399805, -107.9662794718261, -109.67483334602832, -109.891258579519, -110.24757768183042, -109.50202895993814, -110.07763831916637, -109.96891925839451, -110.97268925927641, -109.31698133827767, -112.27933593506792, -110.36206721075725, -109.47379463718867, -110.27836850941338, -110.63738280998388, -111.3611682777485, -110.72689155959884, -111.55480904927032, -111.16689658479412, -110.35555645743601, -111.56609319131051, -110.88279459952174, -114.73607246523177, -109.95813757295693, -107.64639932425493, -111.26486783320321, -112.03946356928121, -111.8915972448334, -110.35245920812773, -110.83155104803564, -110.67437747473863, -110.9959682920065, -110.7815352345103, -111.13722283763049, -112.54797265493127, -110.06894780898469, -111.65186554925783, -111.83545188116254, -110.65894756123697, -108.48458025065264, -112.43760714427981, -114.1368408201927, -110.40065777895025, -110.1066998945526, -108.60654239598591, -110.5716060205154, -110.74257357180736, -111.1136089342442, -111.53539811075092, -113.2559601458872, -109.2003227548348, -110.42285840441025, -111.4086884998834, -111.61503050693868, -110.8194303494779, -108.9701587059964, -112.58521089509063, -110.10873915265242, -112.43440038319561, -110.03468788439882, -111.57896603236308, -110.21939233582523, -109.03614470500777, -110.11738923539659, -109.55359574898291, -110.416473622654, -109.4626868574157, -111.17164025076731, -110.3579689035081, -109.04338716157822, -112.36157114517567, -109.32125615922843, -112.71105693789394, -110.11019129547768, -108.96439402555632, -111.107663418839, -111.48306369859839, -110.9317530461794, -107.98628540532181, -111.1636972328743, -110.47837837583148, -109.04649309175733, -110.27110334963734, -111.35803630614352, -110.77259078859605, -111.46352820533895, -111.16789261049541, -109.2376344776325, -111.6795794983659, -111.74292205167644, -109.40835022991612, -111.02163652600731, -108.79482078001607, -110.6718658416566, -111.08747067599332, -112.15383726791498, -109.47049126158717, -109.061574046483, -111.23993049318979, -111.02521156588335, -109.46012868444186, -110.13918914826291, -112.08180381836377, -110.61929875223015, -111.4424805369965, -111.43420275069585, -109.71347556238717, -110.24726273025648, -109.7860268673935, -109.94126895018422, -111.41948668868926, -108.90555991781676, -110.81242861886172, -109.65007052722677, -112.12672329335953, -110.01123170946096, -111.13980448279096, -113.92013682657084, -108.6000853867411, -110.66793592761913, -110.61237681642844, -110.00839105230496, -109.38083187034974, -109.46119372195675, -110.3708067287448, -108.55518656223285, -113.33935987443276, -111.92184778392033, -111.80820718236087, -107.36852757311246, -109.51077803361602, -110.066791721019, -108.756710558672, -107.91391289865918, -110.72851430959301, -111.39074956442978, -112.928843679455, -109.87348280521556, -112.21371750380071, -110.82495902297394, -109.94006136010094, -110.58757785050143, -110.2790091349881, -111.43884888223081, -108.09540986530712, -109.63783244641691, -110.19577975613292, -110.01690033746098, -112.75938920157155, -109.27158857362184, -111.19519821680541, -110.14381902425255, -110.45955291199236, -111.55660330002316, -110.75604254261134, -111.02122553784838, -111.6490091060193, -110.93362819419399, -110.49033159684308, -110.70789549836027, -110.41991882034145, -110.0264093421208, -109.18432746063652, -110.15292268755287, -112.40733942236504, -111.32869665965416, -110.95418667871114, -111.14291568823575, -111.75555369152653, -112.98146297069803, -109.73870744292117, -111.33806139459435, -110.18838799491355, -112.60408243005732, -110.26112648646833, -110.58257045107274, -109.75155437454112]}, ...(2 in all)]
  in  "FFT 1 Choice 1":u16(ring) items=["T1 Y", "T1 X", "T1 Sum", "T2 Y", "T2 X", "T2 Sum", "T1 FB X", "T1 FB Sum", "T2 FB X", "T2 FB Sum", "PSD Y", "PSD X", "PSD Y Sum", "none"]
  in  "FFT 2 Choice 1":u16(ring)=3 items=["T1 Y", "T1 X", "T1 Sum", "T2 Y", "T2 X", "T2 Sum", "T1 FB X", "T1 FB Sum", "T2 FB X", "T2 FB Sum", "PSD Y", "PSD X", "PSD Y Sum", "none"]
  in  "FFT 1 Choice 2":u16(ring)=1 items=["T1 Y", "T1 X", "T1 Sum", "T2 Y", "T2 X", "T2 Sum", "T1 FB X", "T1 FB Sum", "T2 FB X", "T2 FB Sum", "PSD Y", "PSD X", "PSD Y Sum", "none"]
  in  "FFT 2 Choice 2":u16(ring)=4 items=["T1 Y", "T1 X", "T1 Sum", "T2 Y", "T2 X", "T2 Sum", "T1 FB X", "T1 FB Sum", "T2 FB X", "T2 FB Sum", "PSD Y", "PSD X", "PSD Y Sum", "none"]
  in  "Reset FFT":bool
  in  "# Spectra to Ave.":dbl=25.0
  out "Ave. Time (s)":dbl=1.5
  out "1 Channel":waveform(dbl)(graph)={"t0"=timestamp(0 s since 1904-01-01), "dt"=1.4999999999999999e-05, "Y"=array[20000 elements], "attributes"=variant("NI_ChannelName"=variant(string "T1 Y"))}
  out "Slow mean":dbl=-0.021350993491001932 format="%0.2f"
  in  "Slow mean N ave.":dbl=1.0 min=1.0 step=1.0
  out "Mean Intensity":dbl=-0.021350993491001957
  out "Sigma":dbl=0.006231607115497778
  out "Sigma/Mean":dbl=-0.2918649719098079
  in  "Subtract mean":bool
  in  "High Res. Display":u16(ring) items=["T1 Y", "T1 X", "T1 Sum", "T2 Y", "T2 X", "T2 Sum", "T1 FB X", "T1 FB Sum", "T2 FB X", "T2 FB Sum", "PSD Y", "PSD X", "PSD Y Sum"]
  in  "Tab Green FB":T5(tab)=enum."Trap Control (RF)"
  in  "Scale factor":dbl=0.5
  in  "Scale intensities":bool
  out "Feedback overload":bool
  in  "T2 for asymmetric\n(MHz)":dbl=85.0
  in  "Middle freq for \nsymmetric (MHz)":dbl=78.0
  in  "Symmetric manual \ntrap motion":bool
  out "Stage Moving":bool
  in  "Read Cal":bool
  in  "Confocal Linescan":bool
  in  "Speed (nm/s)":dbl=100.0
  in  "Furthest Withdraw (MHz)":dbl=15.0
  in  "Confocal Image":bool
  in  "Round T1 X":bool caption="Round"
  in  "T1 offset_x (mV)":dbl=44.132512662199076 format="%#_2g"
  in  "T1 kappa_x (pN/nm)":dbl=0.1608167093260824 min=0.0 step=0.001 format="%#_2g"
  out "Time (s)":dbl=40.5
  out "Total Time (s)":dbl=60.0
  in  "Start Saving":bool
  in  "Cal sets to save":u32=50 min=1 step=1
  in  "Comment":string="testing confocal setup"
  out "Calibrating Trap...":bool
  in  "Trap 2 (ON/OFF)":bool=TRUE
  in  "Trap 1 (ON/OFF)":bool=TRUE
  in  "Save Calibration":bool
  in  "N sets to save":u32=200 caption="N Sets"
  in  "Save N Sets":bool
  out "Save file name":path=path "I:/Data/160525/160525_043.dat"
  in  "Save ave N":i32=500 caption="Averaging Factor"
  out "Saving...":bool
  in  "Stop Saving":bool
  out "Progress":u16(slide) scale=0.0..100.0
  out "Manipulating Trap":bool
  out "Buffer Status":dbl(slide) scale=0.0..1.0
  out "Overflow (data lost)":bool
  in  "Reset":bool
  out "Data Rate (Hz)":dbl=66666.66666666667 caption="Trap Data Rate (Hz)" format="%#_3p"
  out "Save Data Rate (Hz)":dbl=133.33333333333334 caption="Rate (Hz)" format="%#_3p"
  out "Save Data Period (s)":dbl=0.0075 caption="Period (s)" format="%#_6p"
  in  "T1 alpha_x (nm/V)":dbl=701.8425766517444 step=10.0 format="%#_3g"
  in  "T2 alpha_x (nm/V)":dbl=806.869454518421 step=10.0 format="%#_3g"
  in  "T2 kappa_x (pN/nm)":dbl=0.13871102209446912 min=0.0 step=0.001 format="%#_2g"
  in  "T2 offset_x (mV)":dbl=-16.403354316809207 format="%#_2g"
  in  "BD 1 Frq 2 (MHz)":dbl=90.0 caption="T2 X (MHz)" min=60.0 max=90.0 step=1.0 format="%#_6p"
  in  "Round T2 X":bool caption="Round"
  in  "MCL Y":dbl(slide)=4.669617603076266 caption="Confocal Y (V)" min=0.0 max=10.0 step=0.01 scale=0.0..10.0 scale format="%_1f"
  in  "MCL X":dbl(slide)=3.742542191839351 caption="Confocal X (V)" min=0.0 max=10.0 step=0.01 scale=0.0..10.0 scale format="%_1f"
  in  "Trap Raster Scan":bool
  out "Raster Scanning...":bool
  in  "Trap Delta (MHz)":dbl=20.0 step=1.0 format="%05.2g"
  in  "Trap Intensity\nSetpoints (V)":cluster{"Set 1":dbl, "Set 2":dbl}={"Set 1"=5.0, "Set 2"=5.0}
  in  "Index":dbl=43.0 caption="Save File Index" min=1.0 step=1.0
  in  "BD 1 Frq 1 (MHz)":dbl=70.0 caption="T1 X (MHz)" min=60.0 max=90.0 step=1.0 format="%#_6p"
  in  "Goto Top (F6)":bool
  in  "Save":bool
  in  "Capture":bool
  in  "?":cluster{"x":string, "y":string, "z":string}={"x"="N.D.\r\n", "y"="N.D.\r\n", "z"="N.D.\r\n"}
  in  "Capture Locations":i32(listbox)=2
  out "X Pos":string="-0.85624\r\n"
  out "Y Pos":string="0.27735\r\n"
  out "Z Pos Pos":string="0.05734\r\n"
  out "X Motion":string="1\r\n"
  out "Y Motion":string="1\r\n"
  out "Z motion":string="1\r\n"
  in  "Goto Bottom (F7)":bool
  in  "Goto Exp (F8)":bool
  in  "Main:":bool caption="Inject Pump 3"
  in  "Inject Top:":bool caption="Inject Pump 1"
  in  "Shunt:":bool
  in  "Inject Bottom":bool
  in  "Scan Range (nm)":dbl=1683.3000000000002
  in  "Symmetric Raster/Feedback?":bool
  in  "VISA Clear":bool
  in  "Green Laser ON/Interlacing":bool
  in  "Current When FB OFF (%)":dbl=10.0 min=0.0 max=100.0 step=1.0
  in  "Green laser mode":enum32{"Laser ON", "Laser OFF", "Interlace"}(radio)
  in  "Ch 1 Inject Rate (ul/h)":dbl=50.0
  in  "Pump write delay (ms)":dbl=300.0
  in  "All Pump Parameters":T6={"Pump 1"={"Diameter (mm)"=4.61, "Units"=4.0, "Volume"=100.0, "Rate"=50.0}, "Pump 2"={"Diameter (mm)"=4.61, "Units"=3.0, "Volume"=0.0, "Rate"=0.0}, "Pump 3"={"Diameter (mm)"=4.61, "Units"=4.0, "Volume"=100.0, "Rate"=250.0}}
  in  "Ch 2 Inject Volume (uL)":dbl=100.0
  in  "Pump pause delay (ms)":u32
  in  "Ch 3 Inject Volume (uL)":dbl=100.0
  in  "Ch 3 Inject Rate (ul/h)":dbl=250.0
  in  "Flush Center Ch Volume (uL)":dbl=15.0
  in  "Flush Center Ch Rate (ul/m)":dbl=100.0
  in  "Inject Valve B":bool caption="Inject Pump 2\n(Flush Center)"
  in  "Total Volume\nFlushed (uL)":dbl
  in  "Tab IR Control":T7(tab)=enum."Feedback on Trap Position"
  in  "RF phase reset before cycles":bool
  in  "Phase increment trap 2":fxp<+/-,64,32>
  in  "Phase increment trap 1":fxp<+/-,64,32>
  in  "Phase offset method":u8=3
  in  "Next trap write delay (ticks)":u16
  out "FPGA error out":errorcluster
  out "Total Counts (ticks)":u32=600
  in  "Trap ON/OFF X or Y Amp?":bool=TRUE
  in  "Oscillate Set 2":bool
  in  "Trap 1 ON":bool=TRUE
  in  "Number Interlace Sets":u8=3 min=1 max=3
  in  "DIO count 3 (ticks)":u32=200
  in  "DIO count 2 (ticks)":u32=200
  in  "DIO count 1 (ticks)":u32=200
  in  "BD 2 Amp 3 (%)":dbl min=0.0 max=75.0 step=1.0
  in  "BD 2 Amp 2 (%)":dbl min=0.0 max=75.0 step=1.0
  in  "BD 2 Amp 1 (%)":dbl min=0.0 max=75.0 step=1.0
  in  "BD 1 Amp 3 (%)":dbl min=0.0 max=75.0 step=1.0
  in  "BD 1 Amp 2 (%)":dbl=42.0 min=0.0 max=75.0 step=1.0
  in  "BD 1 Amp 1 (%)":dbl=40.0 min=0.0 max=75.0 step=1.0
  in  "BD 2 Frq 3 (MHz)":dbl=26.0 min=60.0 max=90.0 step=1.0 format="%#_6p"
  in  "BD 1 Frq 3 (MHz)":dbl=70.0 min=60.0 max=90.0 step=1.0 format="%#_6p"
  in  "BD 2 Frq 2 (MHz)":dbl=26.0 min=60.0 max=90.0 step=1.0 format="%#_6p"
  in  "BD 2 Frq 1 (MHz)":dbl=26.0 min=60.0 max=90.0 step=1.0 format="%#_6p"
  in  "Not-Interlacing Set":enum32{"Set 1", "Set 2", "Set 3"}(radio)
  in  "Interlace":bool=TRUE
  in  "Trap 2 ON":bool=TRUE
  in  "Trap 3 ON":bool
  in  "Scan axis 2":bool=TRUE
  in  "Osc. freq. (Hz)":dbl=0.25
  in  "Osc. amp. (MHz)":dbl=2.0 format="%1_3g"
  out "Coords":T8
  in  "Manipulation Scaling":cluster{"Horizontal":dbl, "Vertical":dbl}={"Horizontal"=0.075, "Vertical"=0.01}
  in  "Freq or Amp switch first":bool=TRUE
  in  "Swap F1 and F2":bool
  in  "Freq switch delay":u16=9
  in  "Amp switch delay":u16=4
  in  "Period":i64=2
  in  "Raster to target force?":bool
  in  "Raster target force (pN)":dbl=10.0
  in  "MCL Step Increment (V_int)":dbl=3.0
  out "Time to Finish All (min)":dbl=0.666 format="%#_2p"
  in  "Scan Speed (nm/s)":dbl=100.0
  in  "Step Size (nm)":dbl=1.0
  in  "MCL/AOM Scale Tweak":dbl=1.0
  in  "MCL Step Position Ratio":dbl=0.5
  in  "Move MCL Also?":bool
  out "Final sep (nm)":dbl=1590.0
  out "Initial sep (nm)":dbl=360.0
  out "Save index":dbl=43.0
  out "Final delta (MHz)":dbl=30.0
  out "Initial delta (MHz)":dbl=20.0
  out "Final freq. (MHz)":dbl=60.0
  out "Initial freq. (MHz)":dbl=70.0
  in  "Saved AOD Raster Scan Parameter Sets":T9(array[cluster])=[{"Scan Range AOD (nm) 2"=500.0, "Step Size AOD (nm) 2"=1.0, "Scan Speed AOD (nm/s) 2"=100.0, "Number of scans (AOD) 2"=1, "Label"="offset curve"}, {"Scan Range AOD (nm) 2"=1000.0, "Step Size AOD (nm) 2"=1.0, "Scan Speed AOD (nm/s) 2"=100.0, "Number of scans (AOD) 2"=1, "Label"="hp raster check"}, {"Scan Range AOD (nm) 2"=6.8, "Step Size AOD (nm) 2"=0.34, "Scan Speed AOD (nm/s) 2"=0.34, "Number of scans (AOD) 2"=1, "Label"="3.4 kbp - 1 bp steps"}]
  in  "Load parameters":bool
  out "Scan Range (MHz)":dbl=-10.0
  in  "Restart DMA? (AOD)":bool=TRUE caption="Restart DMA?"
  out "Incr. int (AOD)":i64=-5670036101
  out "Time/Scan (s) (AOD)":dbl=19.98 format="%#_2p"
  out "Data points/scans":dbl=2664000.0
  out "Data points/scan (f/b)":dbl=2664000.0
  in  "Save scans":bool=TRUE
  out "AOD Scan I":u64=2 caption="Scan I"
  in  "Continuous AOD Scanning":bool caption="Continuous Scanning"
  in  "Abort AOD Scan":bool caption="Abort Scan"
  in  "Scan BD":bool=TRUE
  out "Cycles/step (AOD)":u64=666 format="%.3p"
  in  "Number of F/B Scans (AOD)":u16=1 min=1
  out "Scan steps (AOD)":u64=2000
  out "Scan Increment (MHz)":dbl=-0.0050025012506253125
  out "AOD Scanning":bool caption="Scanning"
  in  "Start AOD Scan":bool caption="Start Scan"
  out "N sets should be saved":dbl=133.2
  out "Progress 2":u16(slide) caption="Progress" scale=0.0..100.0
  in  "Abort save 2":bool caption="Abort save"
  in  "Trap 1 Bead Size (nm)":dbl=1000.0
  in  "Trap 2 Bead Size (nm)":dbl=1000.0
  out "MCL Count":dbl=782931.6080202644
  out "Trap 2 amplitude":ext
  out "Trap 1 amplitude":ext
  in  "PID gains":T10={"proportional gain (Kc)"=0, "integral gain (Kc*Ts/Ti)"=5, "derivative gain (Kc*Td/Ts)"=0}
  in  "All FB On/Off":bool
  in  "AI2 to Setpoint":cluster{"Set 1":bool, "Set 2":bool}
  out "AI2 (V)":cluster{"Set 1":dbl, "Set 2":dbl}={"Set 1"=3.087557603686636, "Set 2"=2.914212469862972}
  in  "Reset Feedback":cluster{"Set 1":bool, "Set 2":bool}
  in  "Feedback On/Off":cluster{"Set 1":bool, "Set 2":bool}={"Set 1"=TRUE, "Set 2"=TRUE}
  in  "Semi Passive ON":bool
  in  "DNA stiffness (pN / nm)":dbl=0.1
  in  "Semi Passive mode":enum16{"None", "Use Feedback", "Sharp Jump"}(ring)
  in  "Jump Force (pN)":dbl
  in  "Auto read offset\ncorrection":bool=TRUE
  in  "Negate Diff?":bool
  in  "Diff. FB.":bool=TRUE
  in  "Dynamic Force FB":bool=TRUE
  in  "Reset Trap Pos. FB":bool
  in  "Tab Control 8":enum32{"Main Setting", "Details"}(tab)
  in  "Real time offset \ncorrection for setpoint":bool=TRUE
  in  "Setpoint correction\noffset file":path
  in  "Negate offset difference":bool
  out "B factor":dbl=0.9916156324677038
  in  "Trap Pos FB Int Count":u16=100
  in  "Trap Pos. FB Gains":T11={"proportional gain (Kc)"=20.0, "integral gain (Kc*Ts/Ti)"=3.0, "derivative gain (Kc*Td/Ts)"=0.0} {"proportional gain (Kc)" format="%.11g"; "integral gain (Kc*Ts/Ti)" format="%.11g"; "derivative gain (Kc*Td/Ts)" format="%.11g"}
  out "Offset file step size":dbl=0.1
  in  "Read setpoint correction\nfile":bool
  in  "Trap Pos. FB Offset Factor":i64
  in  "Trap Pos FB Negate Action":bool=TRUE
  in  "Trap Pos. FB Mult Factor":i64=8388608
  in  "Trap Pos. AI1 X Pre-scale":u16
  in  "Trap Pos. FB Range":T12={"output high"=0.999969482421875, "output low"=-1.0}
  out "Trap Pos FB Int Signal":fxp<+/-,24,9>=42.09515380859375 format="%.18g"
  out "Trap Pos FB Int-Norm Signal":fxp<+/-,16,1>=0.042083740234375 format="%.16g"
  in  "Set SP Using...":bool
  in  "Trap Pos FB Monitor\nT1 or T2":bool
  out "Trap X AI1 (DMA)":T13={"Set 1"=0.030731201171875, "Set 2"=-0.0113525390625}
  in  "N El. to Ave.":i32=10000
  out "Trap Pos FB Action":i64=-32767
  out "Mean T1 Position (nm)":dbl=-4.784226348419907e-12 caption="Mean T1 (nm)" format="%0.2f"
  out "Trap 1 Position RMS (A)":dbl caption="RMS (Ang)"
  in  "Offset Values":T14={"Trap 1X offset"=array[500 elements], "Trap 2X offset"=array[500 elements]}
  in  "Setpoint offset\nCorrection values":dbl[](array[numeric])=[0.024496601698410773, 0.024671186719617436, 0.024845771740824106, 0.025020356762030765, 0.02519494178323743, 0.025369526804444095, 0.025544111825650764, 0.025718696846857424, 0.025893281868064093, 0.026067866889270756, 0.026242451910477423, 0.026417036931684082, 0.02659162195289075, 0.026766206974097418, 0.02694079199530408, 0.027115377016510744, 0.027289962037717407, 0.027464547058924076, 0.02763913208013074, 0.027813717101337402, 0.027988302122544065, 0.02816288714375073, 0.028337472164957394, 0.02851205718616406, 0.028686642207370723, 0.028861227228577393, 0.02903581224978405, 0.029210397270990722, 0.029384982292197385, 0.02955956731340405, 0.02973415233461071, 0.029908737355817377, 0.030083322377024047, 0.03025790739823071, 0.030432492419437372, 0.030607077440644035, 0.0307816624618507, 0.030956247483057368, 0.03113083250426403, 0.0313054175254707, 0.03148000254667736, 0.03165458756788402, 0.03182917258909068, 0.03200375761029735, 0.032178342631504014, 0.03235292765271068, 0.03252751267391735, 0.03270209769512401, 0.03287668271633068, 0.033051267737537346, 0.033225852758744005, 0.03340043777995067, 0.03357502280115733, 0.033749607822364, 0.033924192843570664, 0.03409877786477733, 0.034273362885983996, 0.034447947907190656, 0.03462253292839732, 0.03479711794960398, 0.03497170297081065, 0.035146287992017314, 0.03532087301322398, 0.035495458034430646, 0.035670043055637306, 0.03584462807684397, 0.036019213098050645, 0.036193798119257305, 0.03636838314046397, 0.03654296816167063, 0.0367175531828773, 0.03689213820408396, 0.03706672322529063, 0.037241308246497296, 0.037415893267703955, 0.03759047828891062, 0.03776506331011729, 0.03793964833132395, 0.03811423335253061, 0.03828881837373728, 0.038463403394943946, 0.038637988416150605, 0.03881257343735727, 0.03898715845856393, 0.0391617434797706, 0.03933632850097726, 0.03951091352218393, 0.039685498543390596, 0.03986008356459726, 0.04003466858580393, 0.040209253607010595, 0.040383838628217254, 0.04055842364942392, 0.04073300867063058, 0.040907593691837246, 0.04108217871304391, 0.04125676373425058, 0.041431348755457245, 0.0416059337766639, 0.041780518797870564, 0.04195510381907723, 0.042129688840283896, 0.04230427386149057, 0.04247885888269723, 0.042653443903903895, 0.04282802892511056, 0.04300261394631722, 0.04317719896752389, 0.043351783988730554, 0.04352636900993721, 0.04370095403114388, 0.043875539052350546, 0.04405012407355721, 0.04422470909476388, 0.04439929411597054, 0.044573879137177204, 0.04474846415838387, 0.044923049179590537, 0.045097634200797196, 0.04527221922200386, 0.04544680424321053, 0.045621389264417195, 0.04579597428562386, 0.04597055930683052, 0.04614514432803718, 0.046319729349243846, 0.04649431437045051, 0.04666889939165718, 0.046843484412863845, 0.04701806943407051, 0.04719256456184452, 0.04736536676840916, 0.04753446267808822, 0.047696991448649737, 0.04784953848765512, 0.04799284096907562, 0.048127712917801824, 0.048257934523222495, 0.04838705366421733, 0.04851995197559876, 0.04865949840047511, 0.04880178465045004, 0.0489357994772595, 0.04905304538798107, 0.0491519464532862, 0.049234486275402736, 0.04930263064515607, 0.04935733149089569, 0.04939552771001872, 0.04941451823245213, 0.04941830757306315, 0.049410747020732684, 0.049392795273013504, 0.049367258833286985, 0.049339629147657244, 0.049311849604908836, 0.04928407006216041, 0.049256290519411994, 0.04922851097666357, 0.04920073143391515, 0.04917295189116673, 0.04914517234841831, 0.049117392805669895, 0.049089613262921473, 0.04906183372017306, 0.04903405417742463, 0.04900627463467622, 0.0489784950919278, 0.048950715549179374, 0.04892293600643097, 0.04889515646368254, 0.048867376920934125, 0.0488395973781857, 0.04881181783543728, 0.04878403829268886, 0.04875625874994044, 0.048728479207192026, 0.0487006996644436, 0.04867292012169519, 0.04864514057894676, 0.04861736103619835, 0.048589581493449926, 0.048561801950701505, 0.04853402240795309, 0.04850624286520466, 0.04847846332245625, 0.04845068377970783, 0.04842290423695941, 0.048395124694210985, 0.04836734515146257, 0.04833956560871415, 0.04831178606596573, 0.048284006523217314, 0.048256226980468886, 0.04822844743772048, 0.04820066789497206, 0.048172888352223636, 0.048145108809475215, 0.048117329266726794, 0.04808954972397837, 0.04806177018122996, 0.048033990638481544, 0.048006211095733116, 0.0479784315529847, 0.04795065201023628, 0.04792287246748786, 0.04789509292473944, 0.04786731338199102, 0.0478395338392426, 0.04781175429649418, 0.04778397475374576, 0.047756195210997346, 0.047728415668248925, 0.047700636125500503, 0.04767285658275208, 0.04764507704000366, 0.04761729749725524, 0.047589517954506826, 0.047561738411758404, 0.04753395886900998, 0.04750617932626157, 0.04747839978351315, 0.047450620240764727, 0.047422840698016305, 0.047395061155267884, 0.04736728161251948, 0.047339502069771056, 0.047311722527022634, 0.04728394298427421, 0.04725616344152579, 0.04722838389877737, 0.047200604356028956, 0.047172824813280535, 0.047145045270532114, 0.0471172657277837, 0.04708948618503528, 0.04706170664228686, 0.047033927099538436, 0.047006147556790015, 0.0469783680140416, 0.04695058847129318, 0.04692280892854476, 0.046895029385796344, 0.04686724984304792, 0.0468394703002995, 0.04681169075755108, 0.04678391121480266, 0.04675613167205424, 0.046728352129305824, 0.0467005725865574, 0.04667279304380899, 0.04664501350106057, 0.046617233958312146, 0.046589454415563725, 0.046561674872815303, 0.04653389533006689, 0.046506115787318475, 0.046478336244570054, 0.04645055670182163, 0.04642277715907321, 0.04639499761632479, 0.04636721807357637, 0.046339438530827955, 0.04631165898807953, 0.04628387944533112, 0.0462560999025827, 0.04622832035983428, 0.046200540817085856, 0.046172761274337434, 0.04614498173158901, 0.04611720218884059, 0.04608942264609218, 0.046061643103343757, 0.04603386356059534, 0.04600608401784692, 0.0459783044750985, 0.04595052493235008, 0.04592274538960166, 0.045894965846853236, 0.045867186304104815, 0.0458394067613564, 0.045811627218607986, 0.045783847675859565, 0.045756068133111144, 0.04572828859036272, 0.0457005090476143, 0.04567272950486588, 0.04564494996211747, 0.04561717041936905, 0.04558939087662063, 0.04556161133387221, 0.04553383179112379, 0.04550605224837537, 0.045478272705626946, 0.045450493162878525, 0.04542271362013011, 0.045394934077381696, 0.045367154534633275, 0.045339374991884854, 0.04531159544913643, 0.04528381590638801, 0.04525603636363959, 0.04522825682089117, 0.045200477278142755, 0.045172697735394333, 0.04514491819264592, 0.0451171386498975, 0.04508935910714908, 0.045061579564400656, 0.045033800021652234, 0.04500602047890381, 0.04497824093615539, 0.044950461393406985, 0.04492268185065856, 0.04489490230791014, 0.04486712276516172, 0.0448393432224133, 0.04481156367966488, 0.044783784136916464, 0.04475600459416805, 0.04472822505141963, 0.04470044550867121, 0.044672665965922786, 0.044644886423174365, 0.044617106880425944, 0.04458932733767752, 0.04456154779492911, 0.044533768252180694, 0.04450598870943227, 0.04447820916668385, 0.04445042962393543, 0.04442265008118701, 0.04439487053843859, 0.04436709099569017, 0.04433931145294175, 0.04431153191019333, 0.04428375236744492, 0.044255972824696496, 0.044228193281948075, 0.044200413739199654, 0.04417263419645123, 0.04414485465370281, 0.0441170751109544, 0.04408929556820598, 0.04406151602545756, 0.04403373648270914, 0.04400595693996072, 0.0439781773972123, 0.043950397854463884, 0.04392261831171546, 0.04389483876896704, 0.04386705922621863, 0.043839279683470206, 0.043811500140721785, 0.04378372059797336, 0.04375594105522494, 0.04372816151247652, 0.04370038196972811, 0.04367260242697968, 0.043644822884231264, 0.04361704334148285, 0.04358926379873443, 0.04356148425598601, 0.043533704713237587, 0.043505925170489165, 0.04347814562774075, 0.04345036608499233, 0.043422586542243916, 0.043394806999495494, 0.04336702745674707, 0.04333924791399865, 0.04331146837125023, 0.043283688828501816, 0.0432559092857534, 0.04322812974300498, 0.04320035020025656, 0.04317257065750814, 0.04314479111475972, 0.043117011572011296, 0.04308923202926288, 0.04306145248651446, 0.04303367294376604, 0.043005893401017625, 0.0429781138582692, 0.04295033431552078, 0.04292255477277236, 0.04289477523002394, 0.04286699568727552, 0.0428392161445271, 0.042811436601778684, 0.04278365705903027, 0.04275587751628185, 0.04272809797353343, 0.042700318430785006, 0.042672538888036585, 0.042644759345288163, 0.04261697980253975, 0.04258920025979133, 0.04256142071704291, 0.04253364117429449, 0.04250586163154607, 0.04247808208879765, 0.04245030254604923, 0.04242252300330081, 0.042394743460552387, 0.04236696391780398, 0.04233918437505556, 0.04231140483230714, 0.042283625289558716, 0.042255845746810294, 0.04222806620406188, 0.04220028666131346, 0.04217250711856504, 0.042144727575816616, 0.0421169480330682, 0.04208916849031978, 0.04206138894757136, 0.04203360940482294, 0.04200582986207452, 0.0419780503193261, 0.041950270776577675, 0.04192249123382926, 0.041894711691080846, 0.041866932148332425, 0.041839152605584004, 0.04181137306283558, 0.04178359352008716, 0.04175581397733874, 0.04172803443459032, 0.0417002548918419, 0.04167247534909349, 0.04164469580634507, 0.04161691626359665, 0.04158913672084823, 0.041561357178099806, 0.0415335776353514, 0.04150579809260298, 0.041478018549854556, 0.041450239007106135, 0.041422459464357714, 0.04139467992160929, 0.04136690037886087, 0.04133912083611246, 0.04131134129336403, 0.04128356175061562, 0.04125578220786719, 0.04122800266511878, 0.04120022312237036, 0.04117244357962194, 0.041144664036873516, 0.041116884494125094, 0.04108910495137668, 0.04106132540862826, 0.04103354586587984, 0.041005766323131417, 0.040977986780383, 0.04095020723763458, 0.04092242769488616, 0.04089464815213774, 0.04086686860938932, 0.0408390890666409, 0.04081130952389249, 0.04078352998114407, 0.040755750438395646, 0.040727970895647225, 0.040700191352898804, 0.04067241181015039, 0.040644632267401976, 0.04061685272465355, 0.04058907318190513, 0.04056129363915671, 0.04053351409640829, 0.04050573455365987, 0.04047795501091145, 0.040450175468163034, 0.04042239592541461, 0.0403946163826662, 0.04036683683991778, 0.04033905729716935, 0.040311277754420935, 0.040283498211672514, 0.0402557186689241, 0.04022793912617567, 0.04020015958342725, 0.040172380040678836, 0.04014460049793042, 0.040116820955182, 0.04008904141243358, 0.04006126186968516, 0.04003348232693674, 0.04000570278418832, 0.03997792324143991, 0.03995014369869149, 0.039922364155943066, 0.039894584613194645, 0.03986680507044622, 0.0398390255276978, 0.03981124598494939, 0.03978346644220096, 0.039755686899452546]
  in  "Tab APD Timing":enum32{"Timing", "MCL Scan", "Analog Out"}(tab)=enum."MCL Scan"
  out "APD 2 Gate Late Counter":u32
  out "APD 2 Gate Relative Phase":i16
  in  "Phase Adj. (APD 2 Gate)":i16=20
  in  "Initial Phase Adjustment (APD 2 Gate)":i16=45
  out "APD 1 Gate Late Counter":u32
  in  "- phase (APD 1 Gate)":bool
  in  "+ phase (APD 1 Gate)":bool
  out "APD 1 Gate Relative Phase":i16
  in  "Phase Adj. (APD 1 Gate)":i16=20
  in  "Initial Phase Adjustment (APD 1 Gate)":i16=50
  in  "Save APD":bool=TRUE
  out "APD FIFO Elements Remaining":u32
  in  "- phase (APD Acq)":bool
  in  "+ phase (APD Acq)":bool
  out "APD Acq Late Counter":u32
  out "APD Acq Relative Phase":i16
  in  "Phase Adj. (APD Acq)":i16=20
  in  "Initial Phase Adjustment (APD Acq)":i16
  in  "Invert APD Gate":bool caption="Invert Gate"
  in  "APD Gate OFF Count":u32=450 caption="Gate OFF Count"
  in  "APD Gate ON Count":u32=150 caption="Gate ON Count"
  in  "APD Gate":enum32{"ON", "OFF", "Interlace"}(radio)=enum."Interlace"
  in  "APD Integration Time (s)":dbl=0.01 caption="Integration Time (s)"
  out "APD Acq Rate (Hz)":dbl=100.0 caption="Rate (Hz)"
  out "APD Samples/FIFO Acq.":dbl=30.0
  out "APD Elements/DMA read":u32=60
  out "APD Int. Count":u32=400000 format="%.0p"
  in  "+ phase (APD 2 Gate)":bool
  in  "- phase (APD 2 Gate)":bool
  in  "APD FIFO Depth (requires restart)":u32=300000 format="%.0p"
  in  "Abort MCL Scan":bool
  out "MCL Scan I":u64=2
  out "MCL Scanning":bool
  in  "Start MCL Scan":bool
  out "wait to reset values":bool
  in  "Tab MCL Scan Settings":enum32{"Scan Settings", "MCL FPGA Loop Timing"}(tab)
  out "Total Time (s)":dbl=48.0
  in  "Scan lines (y)":u64=20
  in  "Fast Scan Dir":bool=TRUE
  in  "2D or 1D Scan":bool=TRUE
  out "Initial X":dbl=1.6310662274449115
  out "Initial Y":dbl=2.5691326639606933
  out "Time/f+b scan (s) (MCL)":dbl=2.4 caption="Time/scan (s)"
  in  "Number of scans (MCL)":u64=1 caption="Scans"
  in  "Scan steps (x)":u64=40
  in  "N APD Samp/step":i32=3
  in  "Scan Range (V)\n(of steps)":dbl=3.5
  in  "Restart DMA? (MCL)":bool=TRUE caption="Restart DMA?"
  in  "Continuous MCL Scanning":bool caption="Cont. Scanning"
  in  "Center Scan":bool=TRUE
  in  "Save Data (MCL)":bool=TRUE caption="Save Data"
  out "Actual Incr. int (MCL)":i16=462 caption="Incr. int"
  out "Desired incr (int)":dbl=462.098717948718
  out "Desired Scan Incr (V)":dbl=0.14102564102564102
  out "N sets should be saved (MCL)":dbl=160.0 caption="N sets should be saved"
  out "Data points/scans (MCL)":dbl=4800.0 caption="Data points/scans"
  out "Data points/scan (f+b)":dbl=240.0 caption="points/scan (f+b)"
  out "Cycles/step (MCL)":u64=2000 caption="Cycles/step" format="%.0p"
  out "Actual MCL Inc (V)":dbl=0.14099551377910702
  in  "Phase adjust (MCL)":i16 caption="Phase adjust"
  out "Relative Phase (MCL)":i16 caption="Relative Phase"
  in  "Initial Phase Adj. (MCL)":i16 caption="Initial Phase Adj."
  in  "Update Count (MCL)":u32=600
  in  "+ phase (MCL)":bool
  in  "- phase (MCL)":bool
  out "MCL Late Counter":u32
  in  "APD 1 AO Mult.":i16=1 min=1
  in  "APD 2 AO Mult.":i16=1 min=1
  in  "Tab Control 7":enum32{"Green FB Signals", "Slow MCL Scan"}(tab)
  out "Green FB Plot":dbl(graph)=-10.00030518509476
  out "MCL Scan 2":cluster{"Begin (V)":dbl, dbl, dbl[]}(graph)
  out "MCL Scan":cluster{"Begin (V)":dbl, dbl, dbl[]}(graph)
  in  "GI Frequency, ON count":u32=150 min=1 step=1
  in  "Invert GI":bool
  out "GI Late Counter":u32
  in  "Phase adj. (GI)":i16=5
  out "GI relative phase":i16
  in  "+ phase (GI)":bool
  in  "Initial Phase Adjustment (GI)":i16=4
  in  "GI Frequency, OFF count":u32=450 min=1 step=1
  in  "- phase (GI)":bool
  out "Green FB Signals (V)":cluster{"Y":dbl, "X":dbl, "Sum":dbl}={"Y"=-0.999969482421875, "X"=1.0, "Sum"=-10.00030518509476}
  out "Relative phase (Green FB)":i16
  in  "+ phase (Green FB)":bool
  in  "- phase (Green FB)":bool
  in  "Green FB Count":u32=600
  in  "Phase adj. (Green FB)":i16=10
  in  "Initial Phase Adjustment (Green FB)":i16=50
  in  "Green FB On/Off":bool
  in  "Green int current ON count adj":u32=150
  in  "Green FB Gains":T10={"proportional gain (Kc)"=10, "integral gain (Kc*Ts/Ti)"=5, "derivative gain (Kc*Td/Ts)"=0}
  in  "Green FB Setpoint (mV)":dbl=100.0
  in  "- phase (GI) 2":bool
  in  "Initial Phase Adjustment (GI) 2":i16=-100
  in  "+ phase (GI) 2":bool
  out "GI relative phase 2":i16
  in  "Phase adj. (GI) 2":i16=20
  out "GI Late Counter 2":u32
  in  "Trap Position FIFO Depth":u32=300000 format="%.0p"
  in  "# Samples/trap":u32=20000 format="%.0p"
  out "Trap AI Elements/DMA read":u32=320000 format="%.0p"
  out "Ave. Rate (Hz)":dbl=200000.0 format="%#_6p"
  out "Trap AI FIFO El. Rem.":u32 format="%.0p"
  in  "Phase adj. (AI1)":i16
  out "Relative phase (AI1)":i16
  in  "+ phase (AI1)":bool
  in  "- phase (AI1)":bool
  out "Late Counter (AI1)":u32
  in  "Initial Phase Adjustment (AI1)":i16=185
  out "AI rate (Hz)":dbl=200000.0 format="%#_6p"
  in  "AI Count (ticks)":u32=200
  out "# Samples/channel":u32=40000 format="%.0p"
  in  "Trap AI FIFO Depth":u32=340000 format="%.0p"
  in  "Detector Type":string(combo)="UCB Fleezers 052511"
  in  "N Acq Sets (Traps + Fl.)":i16=3
  in  "Sets to FIFO (Traps)":T15={"Set 1"=TRUE, "Set 2"=TRUE, "Set 3"=FALSE}
  in  "FPGA Ave.":dbl=1.0 min=1.0 step=1.0
  out "Ave. Period (s)":dbl=5e-06 format="%#_6p"
  out "DMA Update Period (s)":dbl=0.3
  out "FPGA Averaging":bool
  out "Trap Sets":u32=2
  out "Counts/DMA":dbl=12000000.0 format="%#_6p"
  out "Trap Pos FIFO El Remaining":u32=171
  out "Trap Pos Elements/DMA read":u32=120000 format="%.0p"
  out "Trap AI FIFO Timeout":u16
  out "Trap Pos FIFO Timeout":u16
  out "Waveform Chart":i32(graph)=320000
  in  "AOM X Cal (nm/MHz)":dbl=160.0
  in  "MCL X Cal (nm/V)":dbl=1174.0
  out "X RF Amplitude Limits (%)":T16={"Minimum"=0.0, "Maximum"=75.0, "Increment"=1.0}
  out "X RF Frequency Limits (MHz)":T16={"Minimum"=60.0, "Maximum"=90.0, "Increment"=1.0}
  out "Y RF Frequency Limits (MHz)":T16={"Minimum"=60.0, "Maximum"=90.0, "Increment"=1.0}
  out "Y RF Amplitude Limits (%)":T16={"Minimum"=0.0, "Maximum"=75.0, "Increment"=1.0}
  in  "Manip. X?":bool=TRUE
  in  "Manip. Y?":bool
  in  "Force Manip Abort":bool
  out "Read cal error":errorcluster
  in  "DAQ Delay (ms)":u32=1000
  in  "Start Scan":bool
  in  "Scan axis":bool
  in  "Osc. amp. (V)":dbl=5.0
  in  "Osc. center (V)":dbl=5.0
  in  "Osc. freq. (Hz) 2":dbl=1.0
  in  "MCL Mode":u16(ring) items=["Manual Positioning", "Sinusoidal Wave", "Linear Scan"]
  in  "Begin (V)":dbl
  in  "End (V)":dbl=10.0
  in  "N Points":dbl=20.0
  in  "Delay to Interlace (s)":dbl
  in  "Delayed Interlace Start":bool
  in  "Read Lateness and Rel Phase":bool
  out "Vec Mean of T1 T2":dbl[](array[numeric])=[1.039290883164312, 1.038787885614062]
  in  "Cal read wait (s)":u32=5
  out "Time tether formed":timestamp=timestamp(3371146929.513132 s since 1904-01-01)
  in  "Chemyx Syringe Pump Serial Port":refnum<visa-resource-name>="ASRL3::INSTR"
  in  "Limit Min (MHz)":dbl=10.0 caption="Min (MHz)"
  in  "Limit Max (MHz)":dbl=16.0 caption="Max (MHz)"
  in  "Limits Enable":bool=TRUE caption="Enable"
  out "AI labels":string[](array[string])=["T1 Y", "T1 X", "T1 Sum", "T2 Y", "T2 X", "T2 Sum", "T1 FB X", "T2 FB Sum", "T2 FB X", "T2 FB Sum", "PSD Y", "PSD X", "PSD Sum"]
  in  "Save TPos":bool=TRUE
  in  "ESP Port":refnum<visa-resource-name>="COM4"
  in  "Axis 3":string="0.00500\r\n"
  in  "Axis 2":string="0.00500\r\n"
  in  "Axis 1":string="0.00500\r\n"
  in  "Axis 3":string="0.20000\r\n"
  in  "Axis 2":string="0.20000\r\n"
  in  "Axis 1":string="0.20000\r\n"
  in  "Activate Joystick":bool
  in  "ESP ZL-Limit":string="-0.09900"
  in  "ESP ZR-Limit":string="0.09900"
  in  "error in":errorcluster
  out "error out":errorcluster
  out "Current MCL (V)":dbl=5.657514378627918
  in  "Tracking factor":dbl=-0.45
  out "Zero T1 position":dbl=70.0
  out "Zero MCL x position":dbl=5.6547922360429315
  out "Error Events":errorcluster
  # "Hidden Controls"
  # "TO BE MOVEDDDD"
  # "After"
  # "During"
  # "Trap On?"
  # "BD Flow ON?"
  # "Samp Flow ON?"
  # "1"
  # "2"
  # "Trap Display:"
  # "APD Display:"
  # "originally 10k"
  # "Data Saving"
  # "Trap Manipulation"
  # "DAQ"
  # "Central frequency 80 MHz"
  # "INS"
  # "DEL"
  # "Bead Calibration"
  # "Current Location"
  # "Select the chamber to go to"
  # "Harvard Pump\n(sample channel for flow exp)"
  # "Chemyx Pump 2"
  # "Units: \n1 = ml/m\n2 = ml/h\n3 = ul/m\n4 = ul/h"
  # "Rate param is ul/h\nVolume param is ul"
  # "Trap interlacing RF phase control\n\n0 = no phase control\n1 = offset increments each trap cycle by values below\n2 = offset increment increases by increment factor each cycle\n3 = random phase (no parameters set)"
  # "Oscillate Set 2 freq. (debugging)"
  # "BD 1"
  # "BD 2"
  # "X"
  # "Y"
  # "AOD Raster Scan"
  # "Approx. trap separations"
  # "X"
  # "Y"
  # "DON'T TURN ON\nUNTIL YOU CLOSE\nTHE LOOP"
  # "FPGA\nreading"
  # "DMA\ntransfer"
  # "APD Gates"
  # "APD 2"
  # "APD 1"
  # "X"
  # "2D"
  # "Y"
  # "1D"
  # "Green FB Measurement"
  # "Green Laser Interlacing"
  # "Digital Gate"
  # "Current Analog Control"
  # "was 87"
  # "originally 600k"
  # "Total AI Rates (NOT rates/trap)"
  # "originally 20k"
  # "(Samples/trap x Trap Sets)"
  # "(Samples/channel x\n8 if averaging (8 channels)\n4 if no averaging)"
  # "Trap 1"
  # "Trap 2"
  # "Flour./Trap 3"
  # "MCL Position Debugging"
  # "Temporary Control Storage\n(these used to be somewhere else, still want to keep them)"
  # "Y"
  # "X"
  # "Trap Position Difference Limits"
  # "Joystick Control"
  # "Setting Limit for the z-axis"
  # "Errors detected in determing Current Location"
  # "High Jog Velocity"
  # "Low Jog Velocity"
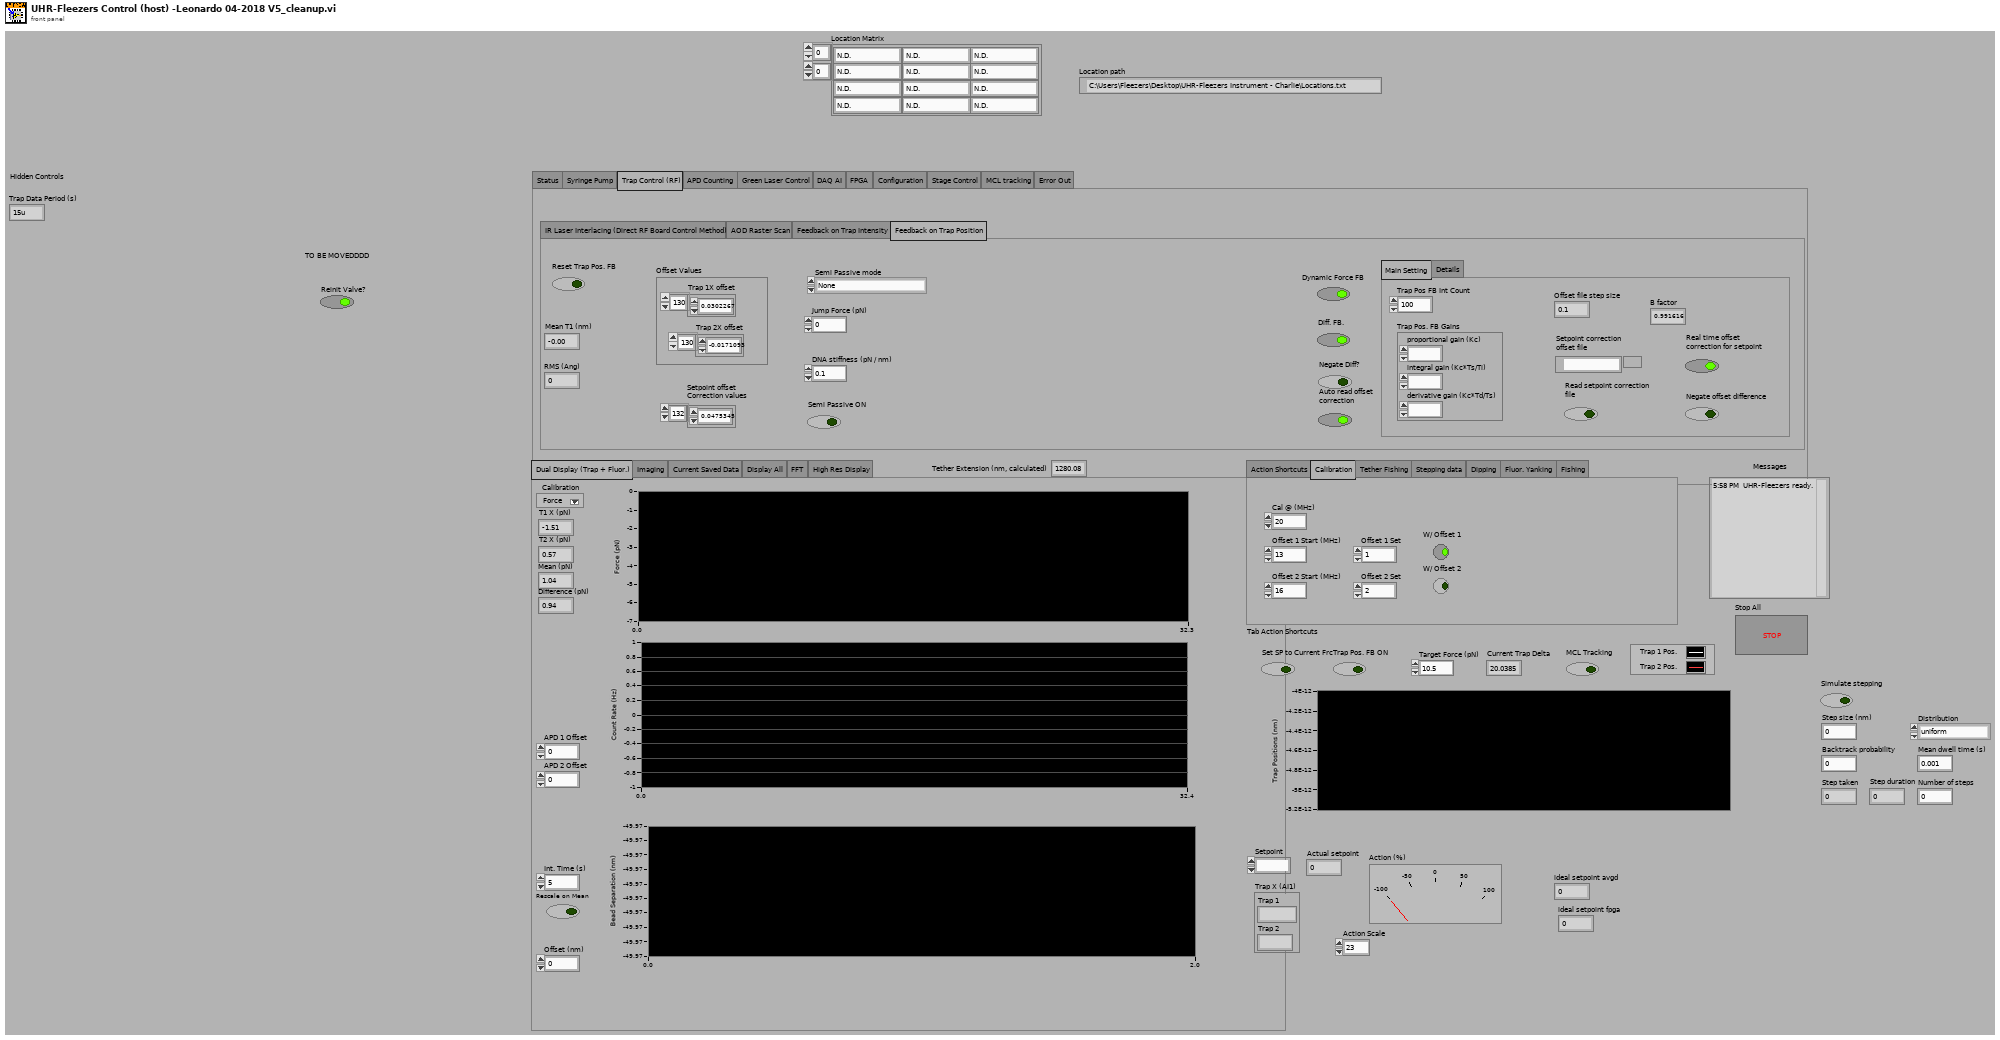
[diagram p1: front panel]
types:
  T1 = cluster{"Trap 1":fxp<+/-,16,1>, "Trap 2":fxp<+/-,16,1>}
  T2 = enum32{"Action Shortcuts", "Calibration", "Tether Fishing", "Stepping data", "Dipping", "Fluor. Yanking", "Fishing"}
  T3 = enum32{"Dual Display (Trap + Fluor.)", "Imaging", "Current Saved Data", "Display All", "FFT", "High Res Display"}
  T4 = typedef "IMAQ Image.ctl" = refnum<image>
  T5 = enum32{"Status", "Syringe Pump", "Trap Control (RF)", "APD Counting", "Green Laser Control", "DAQ AI", "FPGA", "Configuration", "Stage Control", "MCL tracking", "Error Out"}
  T6 = cluster{"Pump 1":cluster{"Diameter (mm)":dbl, "Units":dbl, "Volume":dbl, "Rate":dbl}, "Pump 2":cluster{"Diameter (mm)":dbl, "Units":dbl, "Volume":dbl, "Rate":dbl}, "Pump 3":cluster{"Diameter (mm)":dbl, "Units":dbl, "Volume":dbl, "Rate":dbl}}
  T7 = enum32{"IR Laser Interlacing (Direct RF Board Control Method)", "AOD Raster Scan", "Feedback on Trap Intensity", "Feedback on Trap Position"}
  T8 = typedef "LVPoint32TypeDef.ctl" = cluster{"Horizontal":i32, "Vertical":i32}
  T9 = cluster{"Scan Range AOD (nm) 2":dbl, "Step Size AOD (nm) 2":dbl, "Scan Speed AOD (nm/s) 2":dbl, "Number of scans (AOD) 2":u16, "Label":string}[]
  T10 = cluster{"proportional gain (Kc)":i16, "integral gain (Kc*Ts/Ti)":i16, "derivative gain (Kc*Td/Ts)":i16}
  T11 = cluster{"proportional gain (Kc)":fxp<+/-,16,8>, "integral gain (Kc*Ts/Ti)":fxp<+/-,16,8>, "derivative gain (Kc*Td/Ts)":fxp<+/-,16,8>}
  T12 = cluster{"output high":fxp<+/-,16,1>, "output low":fxp<+/-,16,1>}
  T13 = cluster{"Set 1":fxp<+/-,16,1>, "Set 2":fxp<+/-,16,1>}
  T14 = cluster{"Trap 1X offset":dbl[], "Trap 2X offset":dbl[]}
  T15 = cluster{"Set 1":bool, "Set 2":bool, "Set 3":bool}
  T16 = typedef "LVMinMaxIncTypeDef.ctl" = cluster{"Minimum":dbl, "Maximum":dbl, "Increment":dbl}
  T17 = typedef "Image Type" = u32
  T18 = typedef "nirio_resource_hc.ctl" = tag
  T19 = typedef "openfpgaref.initrf.ctl" = refnum<k20>
  T20 = typedef "openfpgaref.8.6.ctl" = refnum<k20>
  T21 = enum16{"CONNECT", "INITIALIZE VALVES", "DISCONNECT", "MOVE VALVE"}
  T22 = cluster{"New Image":T4, "New Image":T4, "New Image":T4, "New Image":T4}
  T23 = cluster{"Location Matrix[0]":string, "Location Matrix[1]":string, "Location Matrix[2]":string}
  T24 = typedef "XDNodeRunTimeDep.lvlib/timing_clust.ctl" = cluster{"Expected End [f-1]":u64, "Actual End [f-1]":u64, "Finished Late? [f-1]":bool, "Expected End [i-1]":u64, "Actual End [i-1]":u64, "Finished Late? [i-1]":bool, "Expected Start [i]":u64, "Actual Start [i]":u64, "Expected Start [f]":u64, "Actual Start [f]":u64, "Source Name":string, "Structure Name":string, "Period":i64, "Deadline":i64, "Offset":i64, "Start":i64, "Priority":i32, "Timeout":i32, "Mode":T25, "Wakeup Reason":T26, "Error":errorcluster, "Source Type":string, "Secondary Source Type":string, "Global End Time":u64, "Global Start Time":u64, "Frame Duration":u64, "Iteration Duration":u64, "Assigned CPU":i32, "I/O Scan Engine Mode":u32}
  T25 = typedef "XDNodeRunTimeDep.lvlib/nitl_modes.ctl" = enum32{"No Change", "Process missed periods, maintain original phase", "Discard missed periods, maintain original phase", "Process missed periods, ignore original phase", "Discard missed periods, ignore original phase"}
  T26 = typedef "XDNodeRunTimeDep.lvlib/wakeup.ctl" = enum32{"Normal", "Aborted", "Asynchronous wakeup", "Timing source error", "Timed loop error", "Timeout"}
  T27 = enum16{"open", "replace", "create", "open or create", "replace or create", "replace or create with confirmation"}
  T28 = enum16{"big-endian, network order", "native, host order", "little-endian"}
  T29 = cluster{"Scan Range AOD (nm) 2":dbl, "Step Size AOD (nm) 2":dbl, "Scan Speed AOD (nm/s) 2":dbl, "Number of scans (AOD) 2":u16, "Label":string}
  T30 = cluster{"[0]":dbl, "[1]":dbl, "[2]":dbl, "[3]":dbl, "[4]":dbl, "[5]":dbl}
  T31 = cluster{"Diameter (mm)":dbl, "Units":dbl, "Volume":dbl, "Rate":dbl}
  T32 = cluster{"Left":i32, "Top":i32, "Width":u32, "Height":u32}
  T33 = cluster{cluster{"Left":i32, "Top":i32, "Width":u32, "Height":u32}}[]
  T34 = cluster{"averaging mode":u16, "weighting mode":u16, "number of averages":u32}
  T35 = cluster{"dB On (F)":bool, "unwrap phase (F)":bool, "convert to degree (F)":bool}
  T36 = cluster{"f0":dbl, "df":dbl, "magnitude":dbl[]}[][]
  T37 = cluster{"Label.Text":string, "Label.Text":string, "Label.Text":string, "Label.Text":string, "Label.Text":string}
  T38 = cluster{"Green FB Ch 0":i16, "Green FB Ch 1":i16, "Green FB Ch 2":i16}
  T39 = cluster{"Green FB Ch 0":dbl, "Green FB Ch 1":dbl, "Green FB Ch 2":dbl}
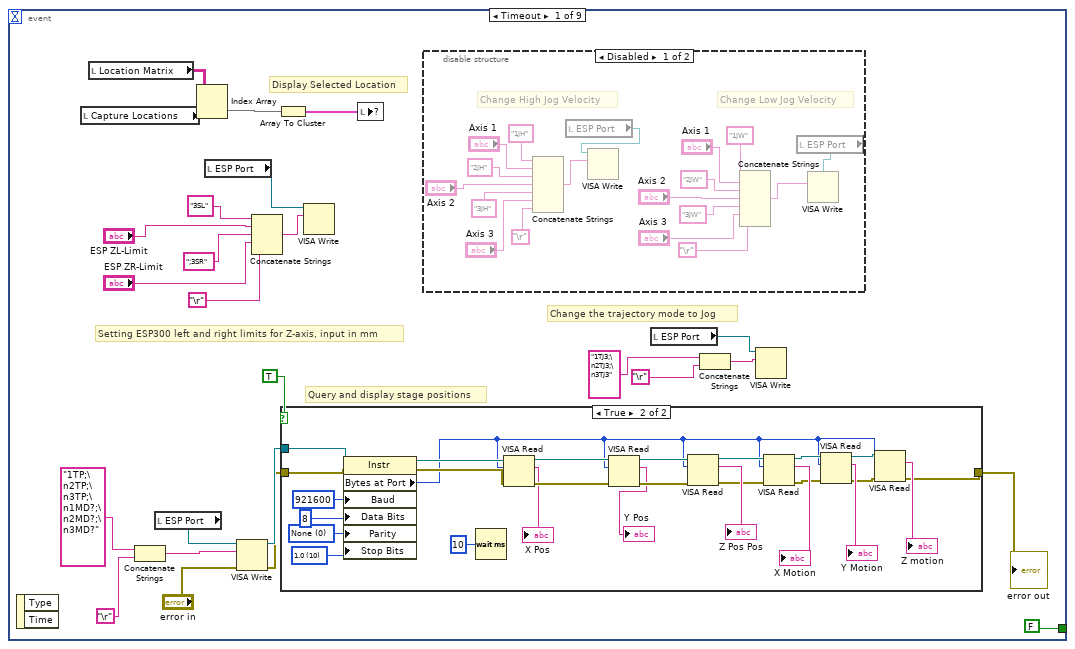
[diagram p2: hidden frame]
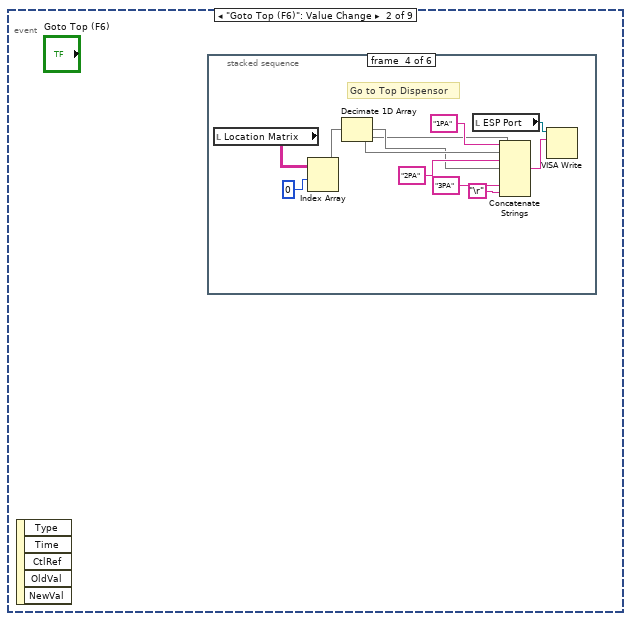
[diagram p5: hidden frame]
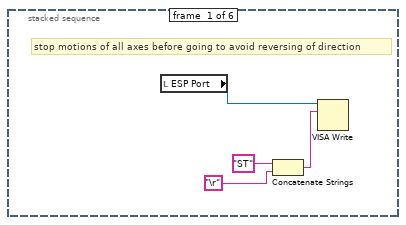
[diagram p6: hidden frame]
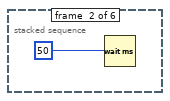
[diagram p7: hidden frame]
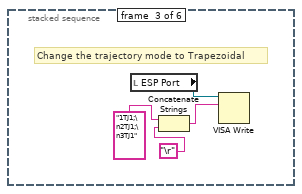
[diagram p8: hidden frame]
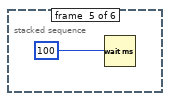
[diagram p9: hidden frame]
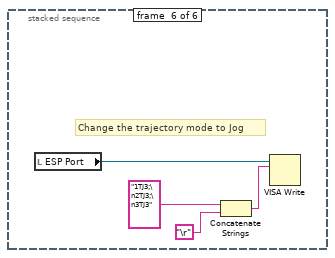
[diagram p10: hidden frame]
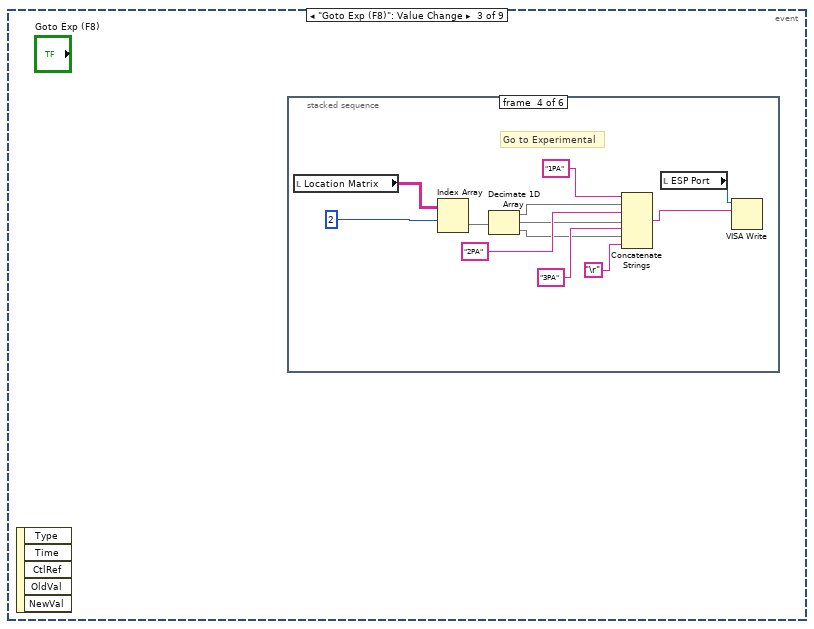
[diagram p11: hidden frame]
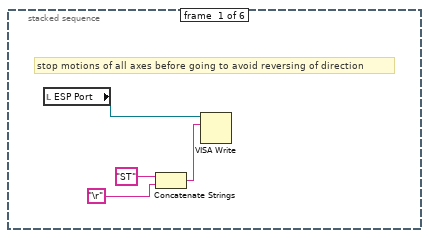
[diagram p12: hidden frame]
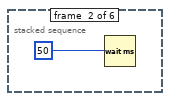
[diagram p13: hidden frame]
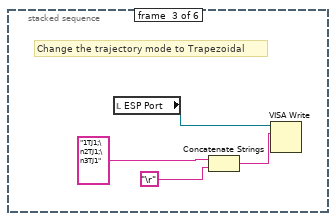
[diagram p14: hidden frame]
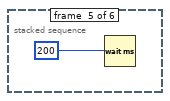
[diagram p15: hidden frame]
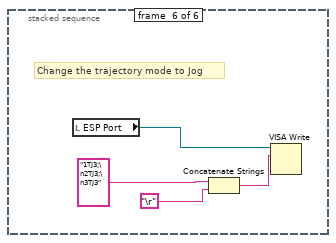
[diagram p16: hidden frame]
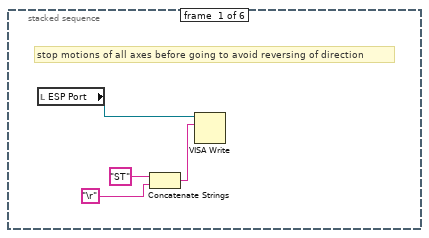
[diagram p17: hidden frame]
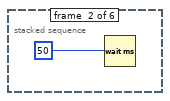
[diagram p18: hidden frame]
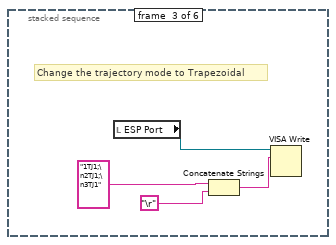
[diagram p19: hidden frame]
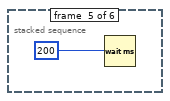
[diagram p20: hidden frame]
diagram:
  w5 = u16 0 items=["Off", "Approach", "Wiggle", "Extend", "Tether Found"] ("Fish Status")
  w77 = T17 2 items=["Grayscale (U8)", "Grayscale (I16)", "Grayscale (SGL)", "Complex (CSG)", "RGB (U32)", "HSL (U32)", "RGB (U64)", "Grayscale (U16)"] ("Image Type")
  w200 = 10.0 ("y")
  w199 = 32767.0 ("y")
  w215 = 6.0  # clock mult.
  w216 = 49152000.0  # TCXO frequ.
  # "Orphaned Controls"
  n1 = flat-sequence "FPGA bitfile init" {
    tunnel: [w248] -> w25
    tunnel: w25 -> [w263]
    tunnel: [w257] -> w146
    tunnel: [w256] -> w129
    frame #0 {
      w248 = T18 "RIO0" ("resource name")
      n2 = xnode "Open FPGA VI Reference"("resource name"=w248) -> ("FPGA VI Reference Out"=w255:T19)  [unwired: 1 in, 1 out]
      n3 = xnode "Invoke Method"("FPGA VI Reference In"=w255) -> ("FPGA VI Reference Out"=w254:T19, "error out"=w253:errorcluster)  [unwired: 1 in]
      n4 = xnode "Invoke Method"("FPGA VI Reference In"=w254, "error in"=w253) -> ("FPGA VI Reference Out"=w251:T19, "error out"=w252:errorcluster)  [unwired: 1 in]
      n5 = call "Initialize RF boards - with FPGA init only vi v1.vi"("error in"=w252, "FPGA Interface"=w251) -> ("error out"=w249:errorcluster, "FPGA Interface 2"=w250:T19)
      n6 = xnode "Close FPGA VI Reference"("FPGA VI Reference In"=w250, "error in"=w249) -> ()  [unwired: 1 out]
    }
    frame #1 {
      w258 = TRUE
      n7 = xnode "Open FPGA VI Reference"("resource name"=w263) -> ("FPGA VI Reference Out"=w262:T20, "error out"=w261:errorcluster)  [unwired: 1 in]
      n8 = xnode "Invoke Method"("FPGA VI Reference In"=w262, "error in"=w261) -> ("FPGA VI Reference Out"=w260:T20, "error out"=w259:errorcluster)
      n9 = xnode "Read/Write Control"("FPGA VI Reference In"=w260, "error in"=w259, "PMODE"=w258, "RD"=w258) -> ("FPGA VI Reference Out"=w256:T20, "error out"=w257:errorcluster)
      "FPGA error out" <- w257
    }
  }
  n10 = Build Array("DIO count 1 (ticks)", "DIO count 2 (ticks)", "DIO count 3 (ticks)") -> (w121:u32[])
  n11 = Multiply(x="APD Integration Time (s)", y=40000000.0) -> (x*y=w137:dbl)
  n12 = Reciprocal(x="APD Integration Time (s)") -> (1/x=w134:dbl)
  n13 = local write "APD Acq Rate (Hz)"(w134) -> ()
  n14 = local read "MCL Y"() -> (w194:dbl)
  n15 = local read "MCL X"() -> (w193:dbl)
  n16 = local read "Dynamic Force FB"() -> (w27:bool)
  n17 = local read "Negate Diff?"() -> (w26:bool)
  n18 = To Unsigned Long Integer(number=w137) -> (unsigned 32bit integer=w136:u32)
  "APD Int. Count" <- w136
  n19 = local read "Diff. FB."() -> (w28:bool)
  n20 = local read "Scan Increment (MHz)"() -> (w211:dbl)
  n21 = local read "Continuous MCL Scanning"() -> (w181:bool)
  n22 = local read "Fast Scan Dir"() -> (w180:bool)
  n23 = local read "Trap Intensity\nSetpoints (V)"() -> (w226:cluster{"Set 1":dbl, "Set 2":dbl})
  n24 = local read "Number of scans (MCL)"() -> (w182:u64)
  n25 = Multiply(x=w194, y=w199) -> (x*y=w196:dbl)
  n26 = Multiply(x=w193, y=w199) -> (x*y=w198:dbl)
  n27 = Divide(x=w196, y=w200) -> (x/y=w195:dbl)
  n28 = Divide(x=w198, y=w200) -> (x/y=w197:dbl)
  n29 = flat-sequence "Set RF Freq/Amp Limits" {
    tunnel: w129 -> [w268]
    tunnel: [w268] -> w128
    tunnel: [w265] -> w29
    tunnel: [w267] -> w127
    tunnel: [w264] -> w125
    tunnel: [w266] -> w126
    frame #0 {
      w266 = T16 {"Minimum"=60.0, "Maximum"=90.0, "Increment"=1.0} ("Min Max Inc")
      w264 = T16 {"Minimum"=0.0, "Maximum"=75.0, "Increment"=1.0} ("Data Entry Limits")
      w265 = T16 {"Minimum"=60.0, "Maximum"=90.0, "Increment"=1.0} ("Min Max Inc")
      w267 = T16 {"Minimum"=0.0, "Maximum"=75.0, "Increment"=1.0} ("Data Entry Limits")
      n30 = property on="BD 1 Frq 1 (MHz)" class="DigNum (strict)"("Data Range"=w265) -> ()  [unwired: 2 in, 2 out]
      n31 = property on="BD 1 Frq 2 (MHz)" class="DigNum (strict)"("Data Range"=w265) -> ()  [unwired: 2 in, 2 out]
      n32 = property on="BD 1 Frq 3 (MHz)" class="DigNum (strict)"("Data Range"=w265) -> ()  [unwired: 2 in, 2 out]
      n33 = property on="BD 2 Frq 1 (MHz)" class="DigNum (strict)"("Data Range"=w266) -> ()  [unwired: 2 in, 2 out]
      n34 = property on="BD 2 Frq 2 (MHz)" class="DigNum (strict)"("Data Range"=w266) -> ()  [unwired: 2 in, 2 out]
      n35 = property on="BD 2 Frq 3 (MHz)" class="DigNum (strict)"("Data Range"=w266) -> ()  [unwired: 2 in, 2 out]
      n36 = property on="BD 1 Amp 1 (%)" class="DigNum (strict)"("Data Range"=w267) -> ()  [unwired: 2 in, 2 out]
      n37 = property on="BD 1 Amp 2 (%)" class="DigNum (strict)"("Data Range"=w267) -> ()  [unwired: 2 in, 2 out]
      n38 = property on="BD 1 Amp 3 (%)" class="DigNum (strict)"("Data Range"=w267) -> ()  [unwired: 2 in, 2 out]
      n39 = property on="BD 2 Amp 1 (%)" class="DigNum (strict)"("Data Range"=w264) -> ()  [unwired: 2 in, 2 out]
      n40 = property on="BD 2 Amp 2 (%)" class="DigNum (strict)"("Data Range"=w264) -> ()  [unwired: 2 in, 2 out]
      n41 = property on="BD 2 Amp 3 (%)" class="DigNum (strict)"("Data Range"=w264) -> ()  [unwired: 2 in, 2 out]
      "X RF Frequency Limits (MHz)" <- w265
      "X RF Amplitude Limits (%)" <- w267
      "Y RF Amplitude Limits (%)" <- w264
      "Y RF Frequency Limits (MHz)" <- w266
    }
  }
  n42 = To Word Integer(number=w195) -> (16bit integer=w192:i16)
  n43 = To Word Integer(number=w197) -> (16bit integer=w191:i16)
  n44 = Not(x=w180) -> (.not. x?=w176:bool)
  n45 = local read "Cycles/step (MCL)"() -> (w183:u64)
  n46 = Multiply(x=w211, y=1000.0) -> (x*y=w218:dbl)
  n47 = local write "Trap Pos FIFO Timeout"(u16 0 ("Trap Pos FIFO Timeout")) -> ()
  n48 = local read "Scan steps (x)"() -> (w184:u64)
  n49 = local read "Desired Scan Incr (V)"() -> (w186:dbl)
  n50 = Scale By Power Of 2(n=48, x=w218) -> (x*2^n=w219:dbl)
  n51 = local read "Sets to FIFO (Traps)"() -> (w24:T15)
  n52 = Multiply(x=w216, y=w215) -> (x*y=w214:dbl)
  n53 = Divide(x=w219, y=w214) -> (x/y=w213:dbl)
  n54 = local read "Number Interlace Sets"() -> (w114:u8)
  n55 = Split 1D Array(array=w121, index=w114) -> (first subarray=w123:u32[])  [unwired: 1 out]
  n56 = Add Array Elements(numeric array=w123) -> (sum=w122:u32)
  n57 = property on="AI Count (ticks)" class="DigNum (strict)"("Val(Sgnl)"="AI Count (ticks)") -> ()  [unwired: 2 in, 2 out]
  n58 = local read "# Samples/channel"() -> (w203:u32)
  n59 = local read "Number of F/B Scans (AOD)"() -> (w204:u16)
  n60 = To Quad Integer(1:w213) -> (0:w210:i64)
  n61 = local read "Not-Interlacing Set"() -> (w113:enum32{"Set 1", "Set 2", "Set 3"})
  n62 = To Unsigned Byte Integer(number=w113) -> (unsigned 8bit integer=w119:u8)
  n63 = Index Array(array=w121, index=w119) -> (element=w120:u32)
  n64 = local read "Feedback On/Off"() -> (w229:cluster{"Set 1":bool, "Set 2":bool})
  n65 = Divide(x=40000000.0, y="AI Count (ticks)") -> (x/y=w173:dbl)
  n66 = Multiply(x=w186, y=32767.0) -> (x*y=w188:dbl)
  n67 = local read "Scan steps (AOD)"() -> (w209:u64)
  n68 = local read "All FB On/Off"() -> (w230:bool)
  n69 = local read "Cycles/step (AOD)"() -> (w208:u64)
  n70 = local write "AI rate (Hz)"(w173) -> ()
  n71 = Divide(x=w188, y=10.0) -> (x/y=w187:dbl)
  n72 = Multiply(x=w209, y=w208) -> (x*y=w207:u64)
  n73 = Multiply(x=3276.7, y=w226) -> (x*y=w225:cluster{"Set 1":dbl, "Set 2":dbl})
  n74 = To Word Integer(number=w187) -> (16bit integer=w185:i16)
  n75 = Multiply(x=w207, y=u64 2) -> (x*y=w205:u64)
  n76 = Divide(x=w173, y="FPGA Ave.") -> (x/y=w174:dbl)
  n77 = To Word Integer(number=w225) -> (16bit integer=w224:cluster{"Set 1":i16, "Set 2":i16})
  n78 = Multiply(x=w205, y=w204) -> (x*y=w202:u64)
  n79 = local write "Ave. Rate (Hz)"(w174) -> ()
  n80 = Divide(x=w202, y=w203) -> (x/y=w201:dbl)
  n81 = Unbundle By Name(w24) -> ("Set 1"=w23:bool, "Set 2"=w22:bool, "Set 3"=w21:bool)
  n82 = Unbundle By Name(w224) -> ("Set 1"=w223:i16, "Set 2"=w222:i16)
  n83 = local read "2D or 1D Scan"() -> (w131:bool)
  n84 = local write "Data points/scans"(w202) -> ()
  n85 = local read "Scan BD"() -> (w220:bool)
  n86 = And(x=w229, y=w230) -> (x .and. y?=w228:cluster{"Set 1":bool, "Set 2":bool})
  n87 = local write "Data points/scan (f/b)"(w205) -> ()
  n88 = Reciprocal(x=w174) -> (1/x=w175:dbl)
  n89 = local read "N Acq Sets (Traps + Fl.)"() -> (w166:i16)
  n90 = local write "N sets should be saved"(w201) -> ()
  n91 = Unbundle By Name(w228) -> ("Set 1"=w232:bool, "Set 2"=w231:bool)
  n92 = local read "Interlace"() -> (w115:bool)
  n93 = Select(t=w122, s=w115, f=w120) -> (s? t:f=w112:u32)
  n94 = local write "Update Count (MCL)"(w112) -> ()
  n95 = local write "Total Counts (ticks)"(w112) -> ()
  n96 = local write "Ave. Period (s)"(w175) -> ()
  n97 = property on="2D or 1D Scan" class="Bool (strict)"("Val(Sgnl)"=w131) -> ()  [unwired: 2 in, 2 out]
  n98 = xnode "Read/Write Control"("FPGA VI Reference In"=w128, "error in"=w146, "ai count"="AI Count (ticks)", "Interlace ON/OFF"=w115, "Number Interlace Cycles"=w114, "Set 1"=w23, "Set 2"=w22, "Set 3"=w21, "FB On/Off Set 1"=w232, "FB On/Off Set 2"=w231, "Interlace Off Parameters"=w113, "FB Setpoint Set 1"=w223, "FB Setpoint Set 2"=w222, "FB Gains"="PID gains", "FB output range"=cluster{"output high":i16, "output low":i16} {"output high"=3000, "output low"=0} ("FB output range 1"), "Cycles per step"=w208, "Scan BD"=w220, "Number of scans"=w204, "Scan steps"=w209, "Scan freq.  increment"=w210, "AO1 (Y)"=w192, "AO2 (X)"=w191, "Scan freq.  increment (MCL)"=w185, "Scan steps (MCL)"=w184, "Cycles per step (MCL)"=w183, "Number of scans (MCL)"=w182, "MCL count"=w112, "Cont. Scan (MCL)"=w181, "MCL Scan Axis"=w176, "1D or 2D Scan?"=w131, "N of AI1 Int Acq Sets"=w166, "BD 1 Delay (ticks)"="Freq switch delay", "Amp switch delay"="Amp switch delay", "Swap F1 and F2"="Swap F1 and F2", "APD Acq Rate Count"=w136, "APD to FIFO"=FALSE, "APD Gate Operating Mode"="APD Gate", "APD Gate ON Count"="APD Gate ON Count", "APD Gate OFF Count"="APD Gate OFF Count", "Invert APD Gate"="Invert APD Gate", "DIO count 1 (ticks)"="DIO count 1 (ticks)", "DIO count 2 (ticks)"="DIO count 2 (ticks)", "DIO count 3 (ticks)"="DIO count 3 (ticks)", "APD 1 AO scale factor"="APD 1 AO Mult.", "APD 2 AO scale factor"="APD 2 AO Mult.", "Diff FB Measurement?"=w28, "Dynamic Force FB (Ronen)"=w27, "Negate Diff?"=w26, "Next trap write delay (ticks)"="Next trap write delay (ticks)", "Phase offset method"="Phase offset method", "Phase Trap 1"="Phase increment trap 1", "RF phase reset before cycles"="RF phase reset before cycles", "Phase Trap 2"="Phase increment trap 2") -> ("FPGA VI Reference Out"=w107:T20, "error out"=w109:errorcluster)  [unwired: 1 in]
  n99 = local read "Green Laser ON/Interlacing"() -> (w110:bool)
  n100 = local read "Green laser mode"() -> (w111:enum32{"Laser ON", "Laser OFF", "Interlace"})
  n101 = local read "GI Frequency, OFF count"() -> (w103:u32)
  n102 = local read "GI Frequency, ON count"() -> (w102:u32)
  n103 = Multiply(x="Current When FB OFF (%)", y=655.35) -> (x*y=w94:dbl)
  n104 = local read "Green FB Count"() -> (w101:u32)
  n105 = Multiply(x="Green FB Setpoint (mV)", y=3.2767) -> (x*y=w91:dbl)
  n106 = To Unsigned Word Integer(number=w94) -> (unsigned 16bit integer=w92:u16)
  n107 = local read "Invert GI"() -> (w105:bool)
  n108 = To Word Integer(number=w91) -> (16bit integer=w89:i16)
  n109 = case shown="True" w110 {
    tunnel: w111 -> [_ w270]
    tunnel: [enum32{"Laser ON", "Laser OFF", "Interlace"}."Laser OFF" ("Green laser mode") w270] -> w104
    frame False {
    }
    frame True {
    }
  }
  n110 = local read "Trap Pos. AI1 X Pre-scale"() -> (w61:u16)
  n111 = local read "Trap Pos FB Monitor\nT1 or T2"() -> (w68:bool)
  n112 = local read "Trap Pos FB Int Count"() -> (w58:u16)
  n113 = local read "Trap Pos FB Negate Action"() -> (w67:bool)
  n114 = local read "Trap Pos. FB Offset Factor"() -> (w66:i64)
  n115 = local read "Trap Pos. FB Mult Factor"() -> (w65:i64)
  n116 = local read "Trap Pos. FB Gains"() -> (w63:T11)
  n117 = local read "Trap Pos. FB Range"() -> (w64:T12)
  n118 = xnode "Read/Write Control"("FPGA VI Reference In"=w107, "error in"=w109, "Green interlace ON count 2"=w102, "Green interlace OFF count 2"=w103, "Invert GI 2"=w105, "Operating Mode 2"=w104, "Green FB Gains"="Green FB Gains", "Green FB Setpoint"=w89, "Green FB On/Off"="Green FB On/Off", "Current Out"=w92, "Green int current ON count adj"="Green int current ON count adj", "Green FB Count"=w101, "Operating Mode"=w104, "Green interlace OFF count"=w103, "Green interlace ON count"=w102, "Invert GI"=w105, "Trap Pos FB Monitor T1 or T2"=w68, "Trap Pos FB Negate Action"=w67, "Trap Pos. FB Offset Factor"=w66, "Trap Pos. FB Mult Factor"=w65, "Trap pos. FB Range"=w64, "Trap Pos. FB Gains"=w63, "Force feedback"=FALSE, "AI1 X Scale"=w61, "Trap Pos to FIFO"=TRUE, "Trap Pos FB Int Count"=w58) -> ("FPGA VI Reference Out"=w106:T20, "error out"=w108:errorcluster)
  n119 = xnode "Invoke Method"("FPGA VI Reference In"=w106, "error in"=w108, "Requested Depth"="Trap AI FIFO Depth") -> ("FPGA VI Reference Out"=w71:T20, "error out"=w70:errorcluster)  [unwired: 1 out]
  n120 = xnode "Invoke Method"("FPGA VI Reference In"=w71, "error in"=w70, "Requested Depth"="Trap Position FIFO Depth") -> ("FPGA VI Reference Out"=w11:T20, "error out"=w9:errorcluster)  [unwired: 1 out]
  n121 = xnode "Invoke Method"("FPGA VI Reference In"=w11, "error in"=w9, "Requested Depth"="APD FIFO Depth (requires restart)") -> ("FPGA VI Reference Out"=w10:T20, "error out"=w8:errorcluster)  [unwired: 1 out]
  n122 = xnode "Invoke Method"("FPGA VI Reference In"=w10, "error in"=w8) -> ("FPGA VI Reference Out"=w43:T20, "error out"=w42:errorcluster)  [unwired: 1 in]
  n123 = flat-sequence "Initial FPGA Loop Relative Phase Adjustment" {
    tunnel: w42 -> [w272]
    tunnel: w43 -> [w273]
    tunnel: [w273] -> w47
    tunnel: [w272] -> w46
    tunnel: [w285] -> w152
    tunnel: [w282] -> w150
    tunnel: w47 -> [w284]
    tunnel: w46 -> [w283]
    tunnel: w152 -> [w287]
    tunnel: [w288] -> w151
    tunnel: w150 -> [w288]
    tunnel: [w287] -> w149
    tunnel: w151 -> [w291]
    tunnel: w149 -> [w290]
    tunnel: [w293] -> w148
    tunnel: [w292] -> w147
    tunnel: [w295] -> w41
    tunnel: [w296] -> w44
    tunnel: w148 -> [w296]
    tunnel: w147 -> [w295]
    frame #0 {
      n124 = Wait (ms)(milliseconds to wait=u32 1000) -> ()  [unwired: 1 out]
    }
    frame #1 {
      n125 = xnode "Read/Write Control"("FPGA VI Reference In"=w284, "error in"=w283, "Phase count adjustment"="Initial Phase Adjustment (AI1)", "Phase count adjustment (GI)"="Initial Phase Adjustment (GI)", "Phase count adjustment (MCL)"="Initial Phase Adj. (MCL)", "Phase Count Adjustment (APD Acq)"="Initial Phase Adjustment (APD Acq)", "Phase count adjustment (APD 1 Gate)"="Initial Phase Adjustment (APD 1 Gate)", "Phase count adjustment (APD 2 Gate)"="Initial Phase Adjustment (APD 2 Gate)", "Phase count adjustment (Green FB)"="Initial Phase Adjustment (Green FB)", "Phase count adjustment (GI) 2"="Initial Phase Adjustment (GI) 2") -> ("FPGA VI Reference Out"=w282:T20, "error out"=w285:errorcluster)
    }
    frame #2 {
      n126 = Wait (ms)(milliseconds to wait=u32 1000) -> ()  [unwired: 1 out]
    }
    frame #3 {
      w289 = TRUE
      n127 = xnode "Read/Write Control"("FPGA VI Reference In"=w291, "error in"=w290, "+ phase"=w289, "+ phase (GI)"=w289, "+ phase (MCL)"=w289, "+ phase (APD Acq)"=w289, "+ phase (APD 1 Gate)"=w289, "+ phase (APD 2 Gate)"=w289, "+ phase (Green FB)"=w289, "+ phase (GI) 2"=w289) -> ("FPGA VI Reference Out"=w292:T20, "error out"=w293:errorcluster)
    }
    frame #4 {
      n128 = Wait (ms)(milliseconds to wait=u32 1000) -> ()  [unwired: 1 out]
    }
  }
  n129 = local read "Phase adj. (AI1)"() -> (w179:i16)
  n130 = local read "Phase adj. (GI)"() -> (w178:i16)
  n131 = local read "Phase adjust (MCL)"() -> (w177:i16)
  n132 = local read "Phase adj. (Green FB)"() -> (w124:i16)
  n133 = local read "Phase adj. (GI) 2"() -> (w95:i16)
  n134 = xnode "Read/Write Control"("FPGA VI Reference In"=w41, "error in"=w44, "Phase count adjustment"=w179, "Phase count adjustment (GI)"=w178, "Phase count adjustment (MCL)"=w177, "Phase Count Adjustment (APD Acq)"="Phase Adj. (APD Acq)", "Phase count adjustment (APD 1 Gate)"="Phase Adj. (APD 1 Gate)", "Phase count adjustment (APD 2 Gate)"="Phase Adj. (APD 2 Gate)", "Phase count adjustment (Green FB)"=w124, "Phase count adjustment (GI) 2"=w95) -> ("FPGA VI Reference Out"=w19:T20, "error out"=w18:errorcluster)
  n135 = Unbundle By Name(w29) -> ("Minimum"=w4:dbl, "Maximum"=w2:dbl)
  n136 = call "MHz2uint64.vi"("inMHz"=w4) -> ("outu64"=w3:u64)  [unwired: 4 in]
  n137 = call "MHz2uint64.vi"("inMHz"=w2) -> ("outu64"=w1:u64)  [unwired: 4 in]
  n138 = xnode "Read/Write Control"("FPGA VI Reference In"=w19, "FB Min frequency"=w3, "FB Max Frequency"=w1) -> ()  [unwired: 1 in, 2 out]
  n139 = call "set RF board frequency - interlace.vi"("Board 2 Frequency Limits"=w126, "Board 1 Frequency Limits"=w29, "error in"=w18, "FPGA VI Reference In"=w19, "Board 2 Frequency 3 (MHz)"="BD 2 Frq 3 (MHz)", "Board 1 Frequency 3 (MHz)"="BD 1 Frq 3 (MHz)", "Board 2 Frequency 2 (MHz)"="BD 2 Frq 2 (MHz)", "Board 2 Frequency 1 (MHz)"="BD 2 Frq 1 (MHz)", "Board 1 Frequency 2 (MHz)"="BD 1 Frq 2 (MHz)", "Board 1 Frequency 1  (MHz)"="BD 1 Frq 1 (MHz)") -> ("error out"=w243:errorcluster, "FPGA VI Reference Out"=w244:T20)
  n140 = Subtract(x="BD 1 Frq 1 (MHz)", y="BD 1 Frq 2 (MHz)") -> (x-y=w165:dbl)
  n141 = Subtract(x="BD 2 Frq 1 (MHz)", y="BD 2 Frq 2 (MHz)") -> (x-y=w164:dbl)
  n142 = Square(x=w164) -> (x^2=w162:dbl)
  n143 = Square(x=w165) -> (x^2=w163:dbl)
  n144 = Add(x=w163, y=w162) -> (x+y=w161:dbl)
  n145 = Square Root(x=w161) -> (sqrt(x)=w160:dbl)
  n146 = call "set RF board amplitude - interlace.vi"("Board 2 Amplitude Limits"=w125, "Board 1 Amplitude Limits"=w127, "error in"=w243, "FPGA VI Reference In"=w244, "Board 2 Amplitude 3 (%)"="BD 2 Amp 3 (%)", "Board 1 Amplitude 3 (%)"="BD 1 Amp 3 (%)", "Board 2 Amplitude 2 (%)"="BD 2 Amp 2 (%)", "Board 2 Amplitude 1 (%)"="BD 2 Amp 1 (%)", "Board 1 Amplitude 2 (%)"="BD 1 Amp 2 (%)", "Board 1 Amplitude 1 (%)"="BD 1 Amp 1 (%)") -> ("error out"=w39:errorcluster, "FPGA VI Reference Out"=w40:T20)
  n147 = local write "Trap Delta (MHz)"(w160) -> ()
  n148 = flat-sequence {
    tunnel: w40 -> [w298]
    tunnel: w39 -> [w297]
    tunnel: [w298] -> w236
    tunnel: [w297] -> w235
    tunnel: [w306] -> w234
    tunnel: w236 -> [w306]
    tunnel: [w305] -> w233
    tunnel: w235 -> [w305]
    tunnel: w234 -> [w309]
    tunnel: w233 -> [w308]
    tunnel: [w309] -> w35
    tunnel: [w308] -> w34
    tunnel: [w316] -> w55
    tunnel: [w319] -> w45
    tunnel: w35 -> [w319]
    tunnel: w34 -> [w315]
    frame #0 {
      n149 = local read "Trap 1 (ON/OFF)"() -> (w299:bool)
      n150 = local write "Stop All"(FALSE ("Stop All")) -> ()
      n151 = local write "Saving..."(FALSE ("Saving Data")) -> ()
      n152 = local write "Index"(1.0 ("Index")) -> ()
      n153 = property on="Trap 1 ON" class="Bool (strict)"("Value"=w299) -> ()  [unwired: 2 in, 2 out]
      "Manipulating Trap" <- FALSE ("Manipulating Trap")
    }
    frame #1 {
      n154 = local read "Trap 2 (ON/OFF)"() -> (w304:bool)
      n155 = Wait (ms)(milliseconds to wait=u32 50) -> ()  [unwired: 1 out]
      n156 = property on="Trap 2 ON" class="Bool (strict)"("Val(Sgnl)"=w304) -> ()  [unwired: 2 in, 2 out]
    }
    frame #2 {
      n157 = local read "Scan Range (nm)"() -> (w310:dbl)
      n158 = call "Update messages.vi"("Message to add"="UHR-Fleezers ready.", "Old message string"="") -> ("New message string"=w313:string)
      n159 = property on="Scan Range (nm)" class="DigNum (strict)"("Val(Sgnl)"=w310) -> ()  [unwired: 2 in, 2 out]
      n160 = local write "Messages"(w313) -> ()
    }
    frame #3 {
      n161 = call "hamilton_controller.vi"("error in"=w315, "action"=T21."CONNECT") -> ("error out"=w317:errorcluster)  [unwired: 9 in]
      n162 = case shown="True" "Reinit Valve?" {
        tunnel: w317 -> [w320 w323]
        tunnel: [w320 w322] -> w316
        frame False {
        }
        frame True {
          n163 = local write "Reinit Valve?"(FALSE ("Reinit Valve?")) -> ()
          n164 = call "hamilton_controller.vi"("error in"=w323, "action"=T21."INITIALIZE VALVES") -> ("error out"=w322:errorcluster)  [unwired: 9 in]
        }
      }
    }
  }
  n165 = call "IMAQ Create"("Image Name"="APD 1 Image", "Image Type"=w77) -> ("New Image"=w76:T4)  [unwired: 3 in, 1 out]
  n166 = call "IMAQ Create"("Image Name"="APD 2 Image", "Image Type"=w77) -> ("New Image"=w75:T4)  [unwired: 3 in, 1 out]
  n167 = call "IMAQ Create"("Image Name"="Det. X Image", "Image Type"=w77) -> ("New Image"=w74:T4)  [unwired: 3 in, 1 out]
  n168 = call "IMAQ Create"("Image Name"="Det. Y Image", "Image Type"=w77) -> ("New Image"=w73:T4)  [unwired: 3 in, 1 out]
  n169 = Bundle("New Image"=w76, "New Image"=w75, "New Image"=w74, "New Image"=w73) -> (w72:T22)  [unwired: 1 in]
  n170 = Current VI's Path() -> (path=w30:path)
  n171 = Strip Path(path=w30) -> (stripped path=w31:path)  [unwired: 1 out]
  n172 = Build Path(base path=w31, name or relative path="Locations.txt") -> (appended path=→"Location path":path)
  n173 = while "Stage Control" {
    stop <- w325 stop-if-true
    n174 = event shown="[3] \"Goto Bottom (F7)\": Value Change" {
      selector: _ -> [_ _ _ _ _ _ _ _ _]
      dyn-events: _ -> [_ _ _ _ _ _ _ _ _]
      timeout: 10 -> [_ _ _ _ _ _ _ _ _]
      tunnel: [FALSE _ _ _ _ _ _ _ TRUE] -> w325
      event Timeout {
        # "Change the trajectory mode to Jog"
        # "Query and display stage positions"
        # "Setting ESP300 left and right limits for Z-axis, input in mm"
        # "Display Selected Location"
        n175 = event-data() -> ()  [unwired: 1 in, 2 out]
        n176 = local read "Capture Locations"() -> (w350:i32)
        n177 = local read "Location Matrix"() -> (w351:string[][])
        n178 = Concatenate Strings("1TP;\n2TP;\n3TP;\n1MD?;\n2MD?;\n3MD?" ("Substring"), "\r") -> (w334:string)
        n179 = local read "ESP Port"() -> (w337:refnum<visa-resource-name>)
        n180 = Index Array(array=w351, index (row)=w350) -> (element=w349:string[])  [unwired: 1 in]
        n181 = local read "ESP Port"() -> (w346:refnum<visa-resource-name>)
        n182 = VISA Write(VISA resource name=w337, write buffer=w334, error in (no error)="error in") -> (VISA resource name out=w335:refnum<visa-resource-name>, error out=w333:errorcluster)  [unwired: 1 out]
        n183 = Concatenate Strings("3SL" ("Substring"), "ESP ZL-Limit", ";3SR", "ESP ZR-Limit", "\r") -> (w345:string)
        n184 = Array To Cluster(array=w349) -> (cluster=w348:T23)
        n185 = case shown="True" TRUE ("Case Constant\n(See Context Help)") {
          tunnel: w335 -> [_ w389]
          tunnel: w333 -> [w370 w388]
          tunnel: [w370 w372] -> w339
          frame False {
          }
          frame True {
            w382 = u16 10 items=["1.0"=10, "1.5"=15, "2.0"=20] ("Serial Settings:Stop Bits")
            w383 = u16 0 items=["None", "Odd", "Even", "Mark", "Space"] ("Serial Settings:Parity")
            n186 = property class="Instr"(reference=w389, error in=w388, "Baud"=u32 921600 ("Serial Settings:Baud Rate"), "Data Bits"=u16 8 ("Serial Settings:Data Bits"), "Parity"=w383, "Stop Bits"=w382) -> (reference out=w387:refnum<visa-resource-name>, error out=w386:errorcluster, "Bytes at Port"=w371:u32)
            n187 = Wait (ms)(milliseconds to wait=u32 10) -> ()  [unwired: 1 out]
            n188 = VISA Read(VISA resource name=w387, byte count=w371, error in (no error)=w386) -> (VISA resource name out=w395:refnum<visa-resource-name>, read buffer=→"X Pos":string, error out=w396:errorcluster)  [unwired: 1 out]
            n189 = VISA Read(VISA resource name=w395, byte count=w371, error in (no error)=w396) -> (VISA resource name out=w393:refnum<visa-resource-name>, read buffer=→"Y Pos":string, error out=w394:errorcluster)  [unwired: 1 out]
            n190 = VISA Read(VISA resource name=w393, byte count=w371, error in (no error)=w394) -> (VISA resource name out=w381:refnum<visa-resource-name>, read buffer=→"Z Pos Pos":string, error out=w380:errorcluster)  [unwired: 1 out]
            n191 = VISA Read(VISA resource name=w381, byte count=w371, error in (no error)=w380) -> (VISA resource name out=w377:refnum<visa-resource-name>, read buffer=→"X Motion":string, error out=w378:errorcluster)  [unwired: 1 out]
            n192 = VISA Read(VISA resource name=w377, byte count=w371, error in (no error)=w378) -> (VISA resource name out=w376:refnum<visa-resource-name>, read buffer=→"Y Motion":string, error out=w374:errorcluster)  [unwired: 1 out]
            n193 = VISA Read(VISA resource name=w376, byte count=w371, error in (no error)=w374) -> (read buffer=→"Z motion":string, error out=w372:errorcluster)  [unwired: 2 out]
          }
        }
        "error out" <- w339
        n194 = VISA Write(VISA resource name=w346, write buffer=w345) -> ()  [unwired: 1 in, 3 out]
        n195 = local write item#428(w348) -> ()
        n196 = disable-structure shown="Disabled" {
          frame Disabled {
            # "Change Low Jog Velocity"
            # "Change High Jog Velocity"
            n197 = Concatenate Strings("1JH" ("Substring"), "Axis 1", "2JH" ("Substring"), "Axis 2", "3JH" ("Substring"), "Axis 3", "\r") -> (w369:string)
            n198 = local read "ESP Port"() -> (w368:refnum<visa-resource-name>)
            n199 = VISA Write(VISA resource name=w368, write buffer=w369) -> ()  [unwired: 1 in, 3 out]
            n200 = Concatenate Strings("1JW" ("Substring"), "Axis 1", "2JW" ("Substring"), "Axis 2", "3JW" ("Substring"), "Axis 3", "\r") -> (w360:string)
            n201 = local read "ESP Port"() -> (w359:refnum<visa-resource-name>)
            n202 = VISA Write(VISA resource name=w359, write buffer=w360) -> ()  [unwired: 1 in, 3 out]
          }
          frame Enabled {
          }
        }
        n203 = local read "ESP Port"() -> (w327:refnum<visa-resource-name>)
        n204 = Concatenate Strings("1TJ3;\n2TJ3;\n3TJ3" ("Substring"), "\r") -> (w328:string)
        n205 = VISA Write(VISA resource name=w327, write buffer=w328) -> ()  [unwired: 1 in, 3 out]
      }
      event "Goto Top (F6)": Value Change {
        n206 = event-data() -> ()  [unwired: 1 in, 5 out]
        n207 = stacked-sequence {
          frame #0 {
            # "stop motions of all axes before going to avoid reversing of direction"
            n208 = local read "ESP Port"() -> (w401:refnum<visa-resource-name>)
            n209 = Concatenate Strings("ST" ("Substring"), "\r") -> (w398:string)
            n210 = VISA Write(VISA resource name=w401, write buffer=w398) -> ()  [unwired: 1 in, 3 out]
          }
          frame #1 {
            n211 = Wait (ms)(milliseconds to wait=u32 50) -> ()  [unwired: 1 out]
          }
          frame #2 {
            # "Change the trajectory mode to Trapezoidal"
            n212 = local read "ESP Port"() -> (w406:refnum<visa-resource-name>)
            n213 = Concatenate Strings("1TJ1;\n2TJ1;\n3TJ1" ("Substring"), "\r") -> (w403:string)
            n214 = VISA Write(VISA resource name=w406, write buffer=w403) -> ()  [unwired: 1 in, 3 out]
          }
          frame #3 {
            # "Go to Top Dispensor"
            n215 = local read "Location Matrix"() -> (w418:string[][])
            n216 = Index Array(array=w418, index (row)=0) -> (element=w414:string[])  [unwired: 1 in]
            n217 = Decimate 1D Array(w414) -> (w412:string[], w410:string[], w408:string[])
            n218 = local read "ESP Port"() -> (w415:refnum<visa-resource-name>)
            n219 = Concatenate Strings("1PA" ("Substring"), w412, "2PA" ("Substring"), w410, "3PA" ("Substring"), w408, "\r") -> (w416:string)
            n220 = VISA Write(VISA resource name=w415, write buffer=w416) -> ()  [unwired: 1 in, 3 out]
          }
          frame #4 {
            n221 = Wait (ms)(milliseconds to wait=u32 100) -> ()  [unwired: 1 out]
          }
          frame #5 {
            # "Change the trajectory mode to Jog"
            n222 = local read "ESP Port"() -> (w423:refnum<visa-resource-name>)
            n223 = Concatenate Strings("1TJ3;\n2TJ3;\n3TJ3" ("Substring"), "\r") -> (w420:string)
            n224 = VISA Write(VISA resource name=w423, write buffer=w420) -> ()  [unwired: 1 in, 3 out]
          }
        }
      }
      event "Goto Exp (F8)": Value Change {
        n225 = event-data() -> ()  [unwired: 1 in, 5 out]
        n226 = stacked-sequence {
          frame #0 {
            # "stop motions of all axes before going to avoid reversing of direction"
            n227 = local read "ESP Port"() -> (w427:refnum<visa-resource-name>)
            n228 = Concatenate Strings("ST" ("Substring"), "\r") -> (w424:string)
            n229 = VISA Write(VISA resource name=w427, write buffer=w424) -> ()  [unwired: 1 in, 3 out]
          }
          frame #1 {
            n230 = Wait (ms)(milliseconds to wait=u32 50) -> ()  [unwired: 1 out]
          }
          frame #2 {
            # "Change the trajectory mode to Trapezoidal"
            n231 = local read "ESP Port"() -> (w432:refnum<visa-resource-name>)
            n232 = Concatenate Strings("1TJ1;\n2TJ1;\n3TJ1" ("Substring"), "\r") -> (w429:string)
            n233 = VISA Write(VISA resource name=w432, write buffer=w429) -> ()  [unwired: 1 in, 3 out]
          }
          frame #3 {
            # "Go to Experimental"
            n234 = local read "Location Matrix"() -> (w444:string[][])
            n235 = Index Array(array=w444, index (row)=2) -> (element=w440:string[])  [unwired: 1 in]
            n236 = Decimate 1D Array(w440) -> (w438:string[], w436:string[], w434:string[])
            n237 = Concatenate Strings("1PA" ("Substring"), w438, "2PA" ("Substring"), w436, "3PA" ("Substring"), w434, "\r") -> (w442:string)
            n238 = local read "ESP Port"() -> (w441:refnum<visa-resource-name>)
            n239 = VISA Write(VISA resource name=w441, write buffer=w442) -> ()  [unwired: 1 in, 3 out]
          }
          frame #4 {
            n240 = Wait (ms)(milliseconds to wait=u32 200) -> ()  [unwired: 1 out]
          }
          frame #5 {
            # "Change the trajectory mode to Jog"
            n241 = local read "ESP Port"() -> (w446:refnum<visa-resource-name>)
            n242 = Concatenate Strings("1TJ3;\n2TJ3;\n3TJ3" ("Substring"), "\r") -> (w449:string)
            n243 = VISA Write(VISA resource name=w446, write buffer=w449) -> ()  [unwired: 1 in, 3 out]
          }
        }
      }
      event "Goto Bottom (F7)": Value Change {
        n244 = event-data() -> ()  [unwired: 1 in, 5 out]
        n245 = stacked-sequence {
          frame #0 {
            # "stop motions of all axes before going to avoid reversing of direction"
            n246 = local read "ESP Port"() -> (w453:refnum<visa-resource-name>)
            n247 = Concatenate Strings("ST" ("Substring"), "\r") -> (w450:string)
            n248 = VISA Write(VISA resource name=w453, write buffer=w450) -> ()  [unwired: 1 in, 3 out]
          }
          frame #1 {
            n249 = Wait (ms)(milliseconds to wait=u32 50) -> ()  [unwired: 1 out]
          }
          frame #2 {
            # "Change the trajectory mode to Trapezoidal"
            n250 = local read "ESP Port"() -> (w458:refnum<visa-resource-name>)
            n251 = Concatenate Strings("1TJ1;\n2TJ1;\n3TJ1" ("Substring"), "\r") -> (w455:string)
            n252 = VISA Write(VISA resource name=w458, write buffer=w455) -> ()  [unwired: 1 in, 3 out]
          }
          frame #3 {
            # "Go to Bottom Dispensor"
            n253 = local read "Location Matrix"() -> (w470:string[][])
            n254 = Index Array(array=w470, index (row)=1) -> (element=w466:string[])  [unwired: 1 in]
            n255 = Decimate 1D Array(w466) -> (w464:string[], w462:string[], w460:string[])
            n256 = Concatenate Strings("1PA" ("Substring"), w464, "2PA" ("Substring"), w462, "3PA" ("Substring"), w460, "\r") -> (w468:string)
            n257 = local read "ESP Port"() -> (w467:refnum<visa-resource-name>)
            n258 = VISA Write(VISA resource name=w467, write buffer=w468) -> ()  [unwired: 1 in, 3 out]
          }
          frame #4 {
            n259 = Wait (ms)(milliseconds to wait=u32 200) -> ()  [unwired: 1 out]
          }
          frame #5 {
            # "Change the trajectory mode to Jog"
            n260 = local read "ESP Port"() -> (w472:refnum<visa-resource-name>)
            n261 = Concatenate Strings("1TJ3;\n2TJ3;\n3TJ3" ("Substring"), "\r") -> (w475:string)
            n262 = VISA Write(VISA resource name=w472, write buffer=w475) -> ()  [unwired: 1 in, 3 out]
          }
        }
      }
      event "Capture": Value Change {
        n263 = event-data() -> ()  [unwired: 1 in, 5 out]
        n264 = local read "Capture Locations"() -> (w476:i32)
        n265 = local read "Z Pos Pos"() -> (w477:string)
        n266 = local read "X Pos"() -> (w479:string)
        n267 = local read "Y Pos"() -> (w478:string)
        n268 = case shown="3" w476 {
          selector: w476 -> [w483 w490 w497 w504]
          tunnel: w479 -> [w486 w493 w500 w507]
          tunnel: w478 -> [w485 w492 w499 w506]
          tunnel: w477 -> [w484 w491 w498 w505]
          frame 0, Default {
            # "Capture Top Dispensor Location"
            n269 = local read "Location Matrix"() -> (w482:string[][])
            n270 = Build Array(w486, w485, w484) -> (w481:string[])
            n271 = Replace Array Subset(array=w482, new element=w481, index (row)=w483) -> (w480:string[][])  [unwired: 1 in]
            n272 = local write "Location Matrix"(w480) -> ()
          }
          frame 1 {
            # "Capture Bottom Dispensor Location"
            n273 = local read "Location Matrix"() -> (w489:string[][])
            n274 = Build Array(w493, w492, w491) -> (w488:string[])
            n275 = Replace Array Subset(array=w489, new element=w488, index (row)=w490) -> (w487:string[][])  [unwired: 1 in]
            n276 = local write "Location Matrix"(w487) -> ()
          }
          frame 2 {
            # "Capture Experimental Region Location"
            n277 = local read "Location Matrix"() -> (w496:string[][])
            n278 = Build Array(w500, w499, w498) -> (w495:string[])
            n279 = Replace Array Subset(array=w496, new element=w495, index (row)=w497) -> (w494:string[][])  [unwired: 1 in]
            n280 = local write "Location Matrix"(w494) -> ()
          }
          frame 3 {
            # "Capture Other Location"
            n281 = local read "Location Matrix"() -> (w503:string[][])
            n282 = Build Array(w507, w506, w505) -> (w502:string[])
            n283 = Replace Array Subset(array=w503, new element=w502, index (row)=w504) -> (w501:string[][])  [unwired: 1 in]
            n284 = local write "Location Matrix"(w501) -> ()
          }
        }
      }
      event "Save": Value Change {
        # "reshape Location Matrix to 1-D array to write"
        n285 = event-data() -> ()  [unwired: 1 in, 5 out]
        n286 = local read "Location Matrix"() -> (w511:string[][])
        n287 = local read "Location path"() -> (w508:path)
        n288 = Reshape Array(w511, 12) -> (w509:string[])
        n289 = Write to Text File(file (use dialog)=w508, text=w509) -> ()  [unwired: 2 in, 3 out]
      }
      event "VISA Clear": Value Change {
        n290 = event-data() -> ()  [unwired: 1 in, 5 out]
        n291 = local read "ESP Port"() -> (w512:refnum<visa-resource-name>)
        n292 = VISA Clear(VISA resource name=w512) -> ()  [unwired: 1 in, 2 out]
      }
      event "Activate Joystick": Value Change {
        # "Change the trajectory mode to Jog"
        n293 = event-data() -> ()  [unwired: 1 in, 5 out]
        n294 = disable-structure shown="Disabled" {
          frame Disabled {
            n295 = case shown="True" "Activate Joystick" {
              frame False {
              }
              frame True {
                # "Change the trajectory mode to Jog"
                n296 = local read "ESP Port"() -> (w521:refnum<visa-resource-name>)
                n297 = Concatenate Strings("1TJ3;\n2TJ3;\n3TJ3" ("Substring"), "\r") -> (w518:string)
                n298 = VISA Write(VISA resource name=w521, write buffer=w518) -> ()  [unwired: 1 in, 3 out]
              }
            }
          }
          frame Enabled {
          }
        }
        n299 = local read "ESP Port"() -> (w513:refnum<visa-resource-name>)
        n300 = Concatenate Strings("1TJ3;\n2TJ3;\n3TJ3" ("Substring"), "\r") -> (w516:string)
        n301 = VISA Write(VISA resource name=w513, write buffer=w516) -> ()  [unwired: 1 in, 3 out]
      }
      event "Stop All": Mouse Down {
        n302 = event-data() -> ()  [unwired: 1 in, 5 out]
      }
    }
  }
  n303 = disable-structure shown="Enabled" {
    disable-tunnel: [w524 _] -> w50
    disable-tunnel: w45 -> [w523 _]
    frame Enabled {
      n304 = node-c288() -> (w526:T24)  [unwired: 4 out]
      n305 = timed-loop "Rough control of MCL mirror stage (debugging)" {
        tunnel: w523 -> [w529]
        tunnel: [w528] -> w524
        timing: w526 -> [_]
        timing-out: [_] -> w525
        stop <- w528 stop-if-true
        n306 = node-c288() -> ()  [unwired: 2 out]
        n307 = case shown="2" "MCL Mode" {
          tunnel: w529 -> [_ w532 w571]
          frame 0, Default {
            # "manual positioning"
          }
          frame 1 {
            # "sinusoidal wave"
            n308 = node-c288() -> (w534:T24)  [unwired: 4 out]
            n309 = timed-loop "Oscillate MCL mirror" {
              timing: w534 -> [_]
              timing-out: [_] -> w533
              tunnel: w532 -> [w565]
              i -> [w564]
              stop <- w539 stop-if-true
              n310 = node-c288() -> (w563:i64)  [unwired: 1 out]
              n311 = call "V2int16.vi"("InV"="MCL X") -> ("Out i16"=w535:i16)  [unwired: 4 in]
              n312 = call "V2int16.vi"("InV"="MCL Y") -> ("Out i16"=w537:i16)  [unwired: 4 in]
              n313 = Divide(x=w563, y=i64 1000) -> (x/y=w546:dbl)
              n314 = Multiply(x=w546, y=w564) -> (x*y=w557:dbl)
              n315 = Multiply(x="Osc. freq. (Hz) 2", y=6.283185307179586) -> (x*y=w558:dbl)
              n316 = Multiply(x=w558, y=w557) -> (x*y=w556:dbl)
              n317 = Sine(x=w556) -> (sin(x)=w555:dbl)
              n318 = Multiply(x=w555, y="Osc. amp. (V)") -> (x*y=w553:dbl)
              n319 = Add(x=w553, y="Osc. center (V)") -> (x+y=w551:dbl)
              n320 = Divide(x=w551, y=10.0) -> (x/y=w549:dbl)
              n321 = Multiply(x=w549, y=32767.0) -> (x*y=w544:dbl)
              n322 = Select(t=w544, s="Scan axis", f=w537) -> (s? t:f=w562:dbl)
              n323 = Select(t=w535, s="Scan axis", f=w544) -> (s? t:f=w561:dbl)
              n324 = local read "MCL Mode"() -> (w543:u16)
              n325 = Not Equal?(x=w543, y=u16 1) -> (x != y?=w540:bool)
              n326 = local read "Stop All"() -> (w541:bool)
              n327 = xnode "Read/Write Control"("FPGA VI Reference In"=w565, "AO1 (Y)"=w562, "AO2 (X)"=w561) -> ()  [unwired: 1 in, 2 out]
              n328 = Compound Arithmetic op=OR(w541, w540) -> (w539:bool)
              n329 = node-c288() -> ()  [unwired: 2 out]
            }
            n330 = node-c288(w533) -> ()  [unwired: 1 out]
          }
          frame 2 {
            # "linear scan"
            n331 = case shown="True" "Start Scan" {
              tunnel: w571 -> [_ w583]
              frame False {
              }
              frame True {
                n332 = Subtract(x="End (V)", y="Begin (V)") -> (x-y=w579:dbl)
                n333 = Decrement(x="N Points") -> (x-1=w578:dbl)
                n334 = Divide(x=w579, y=w578) -> (x/y=w576:dbl)
                n335 = for {
                  N: "N Points" -> [_]
                  tunnel: "Begin (V)" -> [w596]
                  tunnel: w583 -> [w588]
                  tunnel: [w587] -> w582 mode=indexing
                  tunnel: w576 -> [w586]
                  tunnel: [w584] -> w575 mode=indexing
                  i -> [w595]
                  n336 = Multiply(x=w586, y=w595) -> (x*y=w594:dbl)
                  n337 = Add(x=w596, y=w594) -> (x+y=w591:dbl)
                  n338 = local read "MCL Y"() -> (w593:dbl)
                  n339 = local read "MCL X"() -> (w592:dbl)
                  n340 = local read "Scan axis"() -> (w585:bool)
                  n341 = Select(t=w591, s=w585, f=w593) -> (s? t:f=w590:dbl)
                  n342 = Select(t=w592, s=w585, f=w591) -> (s? t:f=w589:dbl)
                  n343 = flat-sequence {
                    tunnel: w590 -> [w600]
                    tunnel: w589 -> [w599]
                    tunnel: w588 -> [w597]
                    tunnel: [w610] -> w587
                    tunnel: [w609] -> w584
                    frame #0 {
                      w603 = 10.0 ("y")
                      w598 = 32767.0 ("y")
                      n344 = Multiply(x=w600, y=w598) -> (x*y=w606:dbl)
                      n345 = Multiply(x=w599, y=w598) -> (x*y=w604:dbl)
                      n346 = Divide(x=w606, y=w603) -> (x/y=w607:dbl)
                      n347 = Divide(x=w604, y=w603) -> (x/y=w605:dbl)
                      n348 = To Word Integer(number=w607) -> (16bit integer=w601:i16)
                      n349 = To Word Integer(number=w605) -> (16bit integer=w602:i16)
                      n350 = xnode "Read/Write Control"("FPGA VI Reference In"=w597, "AO1 (Y)"=w601, "AO2 (X)"=w602) -> ()  [unwired: 1 in, 2 out]
                    }
                    frame #1 {
                      n351 = Wait (ms)(milliseconds to wait="DAQ Delay (ms)") -> ()  [unwired: 1 out]
                    }
                    frame #2 {
                      n352 = local read "Slow mean"() -> (w610:dbl)
                      n353 = local read "Sigma"() -> (w609:dbl)
                    }
                  }
                }
                n354 = Bundle("Begin (V)"="Begin (V)", w576, w582) -> (→"MCL Scan":cluster{"Begin (V)":dbl, dbl, dbl[]})  [unwired: 1 out]
                n355 = Bundle("Begin (V)"="Begin (V)", w576, w575) -> (→"MCL Scan 2":cluster{"Begin (V)":dbl, dbl, dbl[]})  [unwired: 1 out]
              }
            }
          }
        }
        n356 = local read "Stop All"() -> (w528:bool)
        n357 = node-c288() -> ()  [unwired: 2 out]
      }
      n358 = node-c288(w525) -> ()  [unwired: 1 out]
    }
    frame Disabled {
    }
  }
  n359 = node-c288(2 ("Processor")) -> (w38:T24)  [unwired: 3 in]
  n360 = timed-loop "Control parameters (event loop)" {
    tunnel: w45 -> [w616]
    shift-right: [w615] -> _
    shift-left: errorcluster {"status"=FALSE, "code"=0, "source"=""} ("error out") -> [w614]
    tunnel: [w613] -> w52
    timing: w38 -> [_]
    timing-out: [_] -> w37
    stop <- w613 stop-if-true
    n361 = node-c288() -> ()  [unwired: 1 in, 1 out]
    n362 = event shown="[40] \"Index\": Value Change" {
      selector: _ -> [_ _ _ _ _ _ _ _ _ _ _ _ _ _ _ _ _ _ _ _ _ _ _ _ _ _ _ _ _ _ _ _ _ _ _ _ _ _ _ _ _ _ _ _ _ _ _ _ _ _ _ _ _ _ _ _ _ _ _ _]
      dyn-events: _ -> [_ _ _ _ _ _ _ _ _ _ _ _ _ _ _ _ _ _ _ _ _ _ _ _ _ _ _ _ _ _ _ _ _ _ _ _ _ _ _ _ _ _ _ _ _ _ _ _ _ _ _ _ _ _ _ _ _ _ _ _]
      timeout: _ -> [_ _ _ _ _ _ _ _ _ _ _ _ _ _ _ _ _ _ _ _ _ _ _ _ _ _ _ _ _ _ _ _ _ _ _ _ _ _ _ _ _ _ _ _ _ _ _ _ _ _ _ _ _ _ _ _ _ _ _ _]
      tunnel: w616 -> [w657 _ _ w680 _ w698 w704 _ _ _ _ w781 _ _ w825 w831 w835 w840 w876 w894 w901 w919 w930 w941 w952 w963 w974 w992 w998 w1092 _ w1104 w1142 _ w1212 w1217 w1221 w1232 w1237 w1261 _ w1269 _ _ _ _ _ w1405 w1420 w1435 w1461 w1464 w1487 w1547 _ w1564 w1567 _ _ _]
      tunnel: [w656 _ _ w670 _ _ w703 _ _ w746 _ w761 _ _ w824 w827 w834 w837 w875 w892 w900 w913 w924 w935 w946 w957 w968 w990 w997 w1090 _ w1102 w1140 _ _ w1215 w1219 w1222 w1235 w1259 _ w1267 _ _ _ _ _ w1403 _ _ _ _ _ _ _ _ _ _ _ _] -> w615
      tunnel: w614 -> [w655 _ _ w679 _ _ w702 _ _ w746 _ w780 _ _ w823 w826 w833 w836 w874 w893 w899 w918 w929 w940 w951 w962 w973 w991 w996 w1091 _ w1103 w1141 _ _ w1216 w1220 w1231 w1236 w1260 _ w1268 _ _ _ _ _ w1404 w1419 w1434 w1460 w1463 w1488 w1546 _ w1563 _ _ _ _]
      tunnel: [_ _ _ _ _ _ _ _ _ w745 _ _ _ _ _ _ _ _ _ _ _ _ _ _ _ _ _ _ _ _ _ _ _ _ _ _ _ _ _ _ _ _ _ _ _ _ _ _ _ _ _ _ _ _ _ _ _ _ _ _] -> w613
      tunnel: [_ _ _ _ _ _ _ "Round T1 X" _ _ _ _ _ _ _ _ _ _ _ _ _ _ _ _ _ _ _ _ _ _ _ _ _ _ _ _ _ _ _ _ _ _ _ _ _ _ _ _ _ _ _ _ _ _ _ _ _ _ _ _] -> _
      tunnel: [_ _ _ _ _ _ _ _ _ _ _ _ _ _ _ _ _ _ _ _ _ _ _ _ _ _ _ _ _ _ _ _ _ _ _ _ _ _ _ _ _ _ _ _ _ _ _ _ _ _ _ _ _ "Set SP to Current Frc" _ _ _ _ _ _] -> _
      tunnel: [_ _ _ _ _ _ _ _ "Round T2 X" _ "Delayed Interlace Start" _ _ _ _ _ _ _ _ _ _ _ _ _ _ _ _ _ _ _ _ _ _ _ _ _ _ _ _ _ _ _ _ _ _ _ _ _ _ _ _ _ _ _ _ _ _ _ _ _] -> _
      event "AI Count (ticks)", "Sets to FIFO (Traps)", "Save ave N", "FPGA Ave.", "# Samples/channel", "N sets to save": Value Change {
        # "So that if 'Save ave N' is updated, the AOD scanning code updates too."
        n363 = event-data() -> ()  [unwired: 6 out]
        n364 = local read "AI Count (ticks)"() -> (w638:u32)
        n365 = Unbundle By Name("Sets to FIFO (Traps)") -> ("Set 1"=w621:bool, "Set 2"=w620:bool, "Set 3"=w619:bool)
        n366 = Boolean To (0,1)(Boolean="Sets to FIFO (Traps)") -> (0, 1=w647:cluster{"Set 1":i16, "Set 2":i16, "Set 3":i16})
        n367 = xnode "Read/Write Control"("FPGA VI Reference In"=w657, "error in"=w655, "ai count"=w638, "Set 1"=w621, "Set 2"=w620, "Set 3"=w619, "N of AI1 Int Acq Sets"="N Acq Sets (Traps + Fl.)") -> ("error out"=w656:errorcluster)  [unwired: 1 out]
        n368 = Cluster To Array(cluster=w647) -> (array=w646:i16[])
        n369 = To Unsigned Long Integer(number=w646) -> (unsigned 32bit integer=w627:u32[])
        n370 = local read "Scan steps (AOD)"() -> (w648:u64)
        n371 = Multiply(x=w638, y="N Acq Sets (Traps + Fl.)") -> (x*y=w636:u32)
        n372 = Divide(x=40000000.0, y=w638) -> (x/y=w630:dbl)
        "AI rate (Hz)" <- w630
        "Ave. Rate (Hz)" <- w630
        n373 = Add Array Elements(numeric array=w627) -> (sum=w639:u32)
        "Trap Sets" <- w639
        n374 = Reciprocal(x=w630) -> (1/x=→"Ave. Period (s)":dbl)
        n375 = property on="Scan steps (AOD)" class="DigNum (strict)"("Val(Sgnl)"=w648) -> ()  [unwired: 2 in, 2 out]
        n376 = Divide(x=w630, y="N Acq Sets (Traps + Fl.)") -> (x/y=w652:dbl)
        "Data Rate (Hz)" <- w652
        n377 = Reciprocal(x=w652) -> (1/x=→"Data Period (s)":dbl)
        n378 = local read "Save ave N"() -> (w651:i32)
        n379 = Divide(x=w652, y=w651) -> (x/y=w650:dbl)
        "Save Data Rate (Hz)" <- w650
        n380 = Reciprocal(x=w650) -> (1/x=→"Save Data Period (s)":dbl)
        n381 = Multiply(x=w636, y="# Samples/trap") -> (x*y=w634:u32)
        "Counts/DMA" <- w634
        n382 = property on="Trap Disp. Downsample" class="DigNum (strict)"("Maximum"="# Samples/trap") -> ()  [unwired: 2 in, 2 out]
        n383 = Multiply(x=w639, y="# Samples/trap") -> (x*y=w628:u32)
        "# Samples/channel" <- w628
        n384 = Multiply(x=w628, y=u32 8) -> (x*y=→"Trap AI Elements/DMA read":u32)
        n385 = local read "APD Int. Count"() -> (w635:u32)
        n386 = Multiply(x=w628, y=u32 3) -> (x*y=→"Trap Pos Elements/DMA read":u32)
        n387 = Divide(x=w634, y=w635) -> (x/y=w625:dbl)
        "APD Samples/FIFO Acq." <- w625
        n388 = Divide(x=w634, y=40000000.0) -> (x/y=w632:dbl)
        "DMA Update Period (s)" <- w632
        n389 = Multiply(x=2.0, y=w625) -> (x*y=→"APD Elements/DMA read":dbl)
        n390 = property on="APD Disp. dSamp" class="DigNum (strict)"("Maximum"=w625) -> ()  [unwired: 2 in, 2 out]
        n391 = local read "N sets to save"() -> (w644:u32)
        n392 = Multiply(x=w632, y=w644) -> (x*y=→"Total Time (s)":dbl)
        "FPGA Averaging" <- FALSE ("FPGA Averaging")
      }
      event "Rescale on Mean": Value Change {
        n393 = event-data() -> ()  [unwired: 7 out]
        n394 = And(x=FALSE, y="Rescale on Mean") -> (x .and. y?=w659:bool)
        n395 = local write "Rescale on Mean"(w659) -> ()
      }
      event "Detector Type": Value Change {
        n396 = event-data() -> ()  [unwired: 7 out]
        n397 = local read "AI labels"() -> (w661:string[])
        n398 = property on="High Res. Display" class="Ring (strict)"("Strings []"=w661) -> ()  [unwired: 2 in, 2 out]
        n399 = Build Array (concatenate)(w661, "none") -> (w662:string[])
        n400 = property on="FFT 1 Choice 1" class="Ring (strict)"("Strings []"=w662) -> ()  [unwired: 2 in, 2 out]
        n401 = property on="FFT 1 Choice 2" class="Ring (strict)"("Strings []"=w662) -> ()  [unwired: 2 in, 2 out]
        n402 = property on="FFT 2 Choice 1" class="Ring (strict)"("Strings []"=w662) -> ()  [unwired: 2 in, 2 out]
        n403 = property on="FFT 2 Choice 2" class="Ring (strict)"("Strings []"=w662) -> ()  [unwired: 2 in, 2 out]
        n404 = Bundle("APD 1", "APD 2") -> (w665:cluster{string, string})  [unwired: 1 out]
        n405 = Cluster To Array(cluster=w665) -> (array=w663:string[])
        n406 = Build Array (concatenate)(w663, w662) -> (w667:string[])
        n407 = Array Size(array=w667) -> (size(s)=w668:i32)
        n408 = property on="Signals to Plot" class="LstBox (strict)"("Item Names"=w667) -> ()  [unwired: 2 in, 2 out]
        n409 = property on="Signals to Plot" class="LstBox (strict)"("Number of Rows"=w668) -> ()  [unwired: 2 in, 2 out]
        n410 = property on="All Signals" class="WFChart (strict)"("LegNumRows"=w668) -> ()  [unwired: 2 in, 2 out]
      }
      event "Phase adj. (AI1)", "+ phase (AI1)", "- phase (AI1)": Value Change {
        n411 = event-data() -> ()  [unwired: 7 out]
        n412 = Negate(x="Phase adj. (AI1)") -> (-x=w677:i16)
        n413 = Select(t=w677, s="- phase (AI1)", f="Phase adj. (AI1)") -> (s? t:f=w676:i16)
        n414 = xnode "Read/Write Control"("FPGA VI Reference In"=w680, "error in"=w679, "Phase count adjustment"=w676) -> ("FPGA VI Reference Out"=w675:T20, "error out"=w674:errorcluster)
        n415 = Or(x="- phase (AI1)", y="+ phase (AI1)") -> (x .or. y?=w671:bool)
        n416 = xnode "Read/Write Control"("FPGA VI Reference In"=w675, "error in"=w674, "+ phase"=w671) -> ("error out"=w670:errorcluster)  [unwired: 1 out]
      }
      event "Signals to Plot": Double Click {
        w683 = u32 9868950 ("Color Box")
        n417 = event-data() -> ("Row"=w685:i32)  [unwired: 9 out]
        n418 = property on="All Signals" class="WFChart (strict)"("Active Plot"=w685) -> (error out=w696:errorcluster)  [unwired: 2 in, 1 out]
        n419 = property on="All Signals" class="WFChart (strict)" props=["Plot", "Visible?", "Plot", "Plot Color"](error in=w696) -> (error out=w695:errorcluster, "Plot.Visible?"=w694:bool)  [unwired: 1 in, 2 out]
        n420 = Select(t=FALSE ("Plot.Visible"), s=w694, f=TRUE ("Plot.Visible")) -> (s? t:f=w689:bool)
        n421 = property on="All Signals" class="WFChart (strict)"(error in=w695, "Plot.Visible?"=w689) -> (error out=w691:errorcluster)  [unwired: 1 in, 1 out]
        n422 = property on="All Signals" class="WFChart (strict)"(error in=w691) -> (error out=w686:errorcluster, "Plot.Plot Color"=w690:u32)  [unwired: 1 in, 1 out]
        n423 = property on="Signals to Plot" class="LstBox (strict)"(error in=w686, "Active Row"=w685) -> (error out=w684:errorcluster)  [unwired: 1 in, 1 out]
        n424 = Select(t=w690, s=w689, f=u32 0) -> (s? t:f=w687:u32)
        n425 = property on="Signals to Plot" class="LstBox (strict)"(error in=w684, "CellFontColor"=w687, "SelColor"=w683, "CellBG"=w683, "CellFontSize"=u32 20 ("Active Row:Cell Font:Size"), "CellFontBold"=TRUE ("Active Row:Cell Font:Bold")) -> ()  [unwired: 1 in, 2 out]
      }
      event "Dynamic Force FB": Value Change {
        n426 = event-data() -> ()  [unwired: 7 out]
        n427 = xnode "Read/Write Control"("FPGA VI Reference In"=w698, "Dynamic Force FB (Ronen)"="Dynamic Force FB") -> ()  [unwired: 1 in, 2 out]
      }
      event "BD 1 Frq 1 (MHz)", "BD 1 Frq 2 (MHz)", "BD 1 Frq 3 (MHz)", "BD 2 Frq 1 (MHz)", "BD 2 Frq 2 (MHz)", "BD 2 Frq 3 (MHz)", "Trap Delta (MHz)": Value Change {
        # "anytime one of the frequencies is changed, write it to the RF board UNLESS Set 2 is being oscillated. The oscillation\nscript writes the frequencies to the RF board."
        n428 = event-data() -> ("CtlRef"=w701:refnum<vi>)  [unwired: 6 out]
        n429 = control-ref of="Trap Delta (MHz)"() -> (w700:refnum<vi>)
        n430 = Equal?(x=w700, y=w701) -> (x = y?=w699:bool)
        n431 = case shown="False" "Oscillate Set 2" {
          tunnel: w704 -> [w725 _]
          tunnel: [w724 w737] -> w703
          tunnel: w702 -> [w723 w737]
          tunnel: w699 -> [w710 _]
          frame False {
            n432 = case shown="True" "Symmetric manual \ntrap motion" {
              tunnel: ["T2 for asymmetric\n(MHz)" w736] -> w711
              tunnel: "Trap Delta (MHz)" -> [w730 w735]
              tunnel: [w729 w732] -> w707
              frame False {
                n433 = Subtract(x="T2 for asymmetric\n(MHz)", y=w730) -> (x-y=w729:dbl)
              }
              frame True {
                n434 = Divide(x=w735, y=2) -> (x/y=w733:dbl)
                n435 = Subtract(x="Middle freq for \nsymmetric (MHz)", y=w733) -> (x-y=w732:dbl)
                n436 = Add(x="Middle freq for \nsymmetric (MHz)", y=w733) -> (x+y=w736:dbl)
              }
            }
            n437 = local read "BD 1 Frq 2 (MHz)"() -> (w712:dbl)
            n438 = local write "BD 1 Frq 1 (MHz)"(w707) -> ()
            n439 = Select(t=w711, s=w710, f=w712) -> (s? t:f=w709:dbl)
            n440 = local read "Y RF Frequency Limits (MHz)"() -> (w713:T16)
            n441 = local read "X RF Frequency Limits (MHz)"() -> (w714:T16)
            n442 = local read "BD 1 Frq 3 (MHz)"() -> (w726:dbl)
            n443 = local write "BD 1 Frq 2 (MHz)"(w709) -> ()
            n444 = local read "BD 2 Frq 1 (MHz)"() -> (w717:dbl)
            n445 = local read "BD 2 Frq 2 (MHz)"() -> (w716:dbl)
            n446 = local read "BD 2 Frq 3 (MHz)"() -> (w727:dbl)
            n447 = call "set RF board frequency - interlace.vi"("Board 2 Frequency Limits"=w713, "Board 1 Frequency Limits"=w714, "error in"=w723, "FPGA VI Reference In"=w725, "Board 2 Frequency 3 (MHz)"=w727, "Board 1 Frequency 3 (MHz)"=w726, "Board 2 Frequency 2 (MHz)"=w716, "Board 2 Frequency 1 (MHz)"=w717, "Board 1 Frequency 2 (MHz)"=w709, "Board 1 Frequency 1  (MHz)"=w707) -> ("error out"=w724:errorcluster)  [unwired: 1 out]
            n448 = Subtract(x=w717, y=w716) -> (x-y=w721:dbl)
            n449 = Subtract(x=w709, y=w707) -> (x-y=w722:dbl)
            n450 = Square(x=w721) -> (x^2=w719:dbl)
            n451 = Square(x=w722) -> (x^2=w720:dbl)
            n452 = Add(x=w720, y=w719) -> (x+y=w718:dbl)
            n453 = Square Root(x=w718) -> (sqrt(x)=w715:dbl)
            n454 = local write "Trap Delta (MHz)"(w715) -> ()
            n455 = property on="Initial delta (MHz)" class="DigNum (strict)"("Val(Sgnl)"=w715) -> ()  [unwired: 2 in, 2 out]
          }
          frame True {
          }
        }
      }
      event "Round T1 X": Value Change {
        n456 = event-data() -> ()  [unwired: 7 out]
        n457 = local read "BD 1 Frq 1 (MHz)"() -> (w740:dbl)
        n458 = Round To Nearest(number=w740) -> (nearest integer value=w739:dbl)
        n459 = property on="BD 1 Frq 1 (MHz)" class="DigNum (strict)"("Val(Sgnl)"=w739) -> ()  [unwired: 2 in, 2 out]
      }
      event "Round T2 X": Value Change {
        n460 = event-data() -> ()  [unwired: 7 out]
        n461 = local read "BD 1 Frq 2 (MHz)"() -> (w742:dbl)
        n462 = Round To Nearest(number=w742) -> (nearest integer value=w741:dbl)
        n463 = property on="BD 1 Frq 2 (MHz)" class="DigNum (strict)"("Val(Sgnl)"=w741) -> ()  [unwired: 2 in, 2 out]
      }
      event "Stop All": Value Change {
        n464 = event-data() -> ()  [unwired: 7 out]
        n465 = call "hamilton_controller.vi"("action"=T21."DISCONNECT") -> ()  [unwired: 10 in, 1 out]
        n466 = local read "Stop All"() -> (w745:bool)
      }
      event "Delayed Interlace Start": Value Change {
        n467 = event-data() -> ()  [unwired: 7 out]
        n468 = flat-sequence {
          frame #0 {
            n469 = Multiply(x="Delay to Interlace (s)", y=1000.0) -> (x*y=w748:dbl)
            n470 = Wait (ms)(milliseconds to wait=w748) -> ()  [unwired: 1 out]
          }
          frame #1 {
            n471 = property on="Green laser mode" class="RadioBtnsControl (strict)"("Val(Sgnl)"=enum32{"Laser ON", "Laser OFF", "Interlace"}."Interlace" ("Value (Signaling)")) -> ()  [unwired: 2 in, 2 out]
          }
        }
      }
      event "BD 1 Amp 1 (%)", "BD 1 Amp 2 (%)", "BD 1 Amp 3 (%)", "BD 2 Amp 1 (%)", "BD 2 Amp 2 (%)", "BD 2 Amp 3 (%)", "Trap 1 ON", "Trap 2 ON", "Trap 3 ON", "Feedback On/Off", "All FB On/Off": Value Change {
        w772 = i16 1 ("f")
        n472 = event-data() -> ()  [unwired: 7 out]
        n473 = local write "Trap 1 (ON/OFF)"("Trap 1 ON") -> ()
        n474 = local write "Trap 2 (ON/OFF)"("Trap 2 ON") -> ()
        n475 = Boolean To (0,1)(Boolean="Trap 3 ON") -> (0, 1=w773:i16)
        n476 = Boolean To (0,1)(Boolean="Trap 1 ON") -> (0, 1=w774:i16)
        n477 = Boolean To (0,1)(Boolean="Trap 2 ON") -> (0, 1=w775:i16)
        n478 = Select(t=w775, s="Trap ON/OFF X or Y Amp?", f=w772) -> (s? t:f=w770:i16)
        n479 = Select(t=w774, s="Trap ON/OFF X or Y Amp?", f=w772) -> (s? t:f=w771:i16)
        n480 = Select(t=w773, s="Trap ON/OFF X or Y Amp?", f=w772) -> (s? t:f=w769:i16)
        n481 = Select(t=w772, s="Trap ON/OFF X or Y Amp?", f=w775) -> (s? t:f=w767:i16)
        n482 = Select(t=w772, s="Trap ON/OFF X or Y Amp?", f=w774) -> (s? t:f=w768:i16)
        n483 = Select(t=w772, s="Trap ON/OFF X or Y Amp?", f=w773) -> (s? t:f=w766:i16)
        n484 = And(x="All FB On/Off", y="Feedback On/Off") -> (x .and. y?=w764:cluster{"Set 1":bool, "Set 2":bool})
        n485 = Unbundle By Name(w764) -> ("Set 1"=w760:bool, "Set 2"=w757:bool)
        n486 = local read "BD 1 Amp 1 (%)"() -> (w784:dbl)
        n487 = local read "BD 1 Amp 2 (%)"() -> (w783:dbl)
        n488 = local read "BD 1 Amp 3 (%)"() -> (w782:dbl)
        n489 = local read "Y RF Amplitude Limits (%)"() -> (w753:T16)
        n490 = local read "X RF Amplitude Limits (%)"() -> (w754:T16)
        n491 = local read "BD 2 Amp 1 (%)"() -> (w785:dbl)
        n492 = local read "BD 2 Amp 2 (%)"() -> (w786:dbl)
        n493 = local read "BD 2 Amp 3 (%)"() -> (w787:dbl)
        n494 = And(x="Trap 2 ON", y=w757) -> (x .and. y?=w755:bool)
        n495 = And(x="Trap 1 ON", y=w760) -> (x .and. y?=w758:bool)
        n496 = Multiply(x=w771, y=w784) -> (x*y=w779:dbl)
        n497 = Multiply(x=w783, y=w770) -> (x*y=w777:dbl)
        n498 = Multiply(x=w782, y=w769) -> (x*y=w778:dbl)
        n499 = Multiply(x=w785, y=w768) -> (x*y=w788:dbl)
        n500 = Multiply(x=w786, y=w767) -> (x*y=w789:dbl)
        n501 = Multiply(x=w787, y=w766) -> (x*y=w790:dbl)
        n502 = call "set RF board amplitude - interlace.vi"("Board 2 Amplitude Limits"=w753, "Board 1 Amplitude Limits"=w754, "error in"=w780, "FPGA VI Reference In"=w781, "Board 2 Amplitude 3 (%)"=w790, "Board 1 Amplitude 3 (%)"=w778, "Board 2 Amplitude 2 (%)"=w789, "Board 2 Amplitude 1 (%)"=w788, "Board 1 Amplitude 2 (%)"=w777, "Board 1 Amplitude 1 (%)"=w779) -> ("error out"=w762:errorcluster, "FPGA VI Reference Out"=w763:T20)
        n503 = xnode "Read/Write Control"("FPGA VI Reference In"=w763, "error in"=w762, "FB On/Off Set 1"=w758, "FB On/Off Set 2"=w755) -> ("error out"=w761:errorcluster)  [unwired: 1 out]
        n504 = case shown="True" "All FB On/Off" {
          frame False {
          }
          frame True {
            n505 = local write "Feedback overload"(FALSE) -> ()
          }
        }
      }
      event "Load parameters": Value Change {
        n506 = event-data() -> ()  [unwired: 7 out]
        n507 = property on="Saved AOD Raster Scan Parameter Sets" class="Arr (strict)"() -> ("Index Values"=w802:u32[])  [unwired: 2 in, 2 out]
        n508 = Index Array(array=w802, index=0) -> (element=w799:u32)
        n509 = local write "Load parameters"(FALSE ("Load parameters")) -> ()
        n510 = Index Array(array="Saved AOD Raster Scan Parameter Sets", index=w799) -> (element=w798:T29)
        n511 = Unbundle By Name(w798) -> ("Scan Range AOD (nm) 2"=w797:dbl, "Step Size AOD (nm) 2"=w796:dbl, "Scan Speed AOD (nm/s) 2"=w795:dbl, "Number of scans (AOD) 2"=w794:u16)
        n512 = flat-sequence {
          tunnel: w797 -> [w805]
          tunnel: w796 -> [w804]
          tunnel: w795 -> [w803]
          tunnel: w794 -> [w806]
          frame #0 {
            n513 = local write "Scan Speed (nm/s)"(w803) -> ()
            n514 = local write "Scan Range (nm)"(w805) -> ()
            n515 = local write "Step Size (nm)"(w804) -> ()
          }
          frame #1 {
            n516 = property on="Number of F/B Scans (AOD)" class="DigNum (strict)"("Val(Sgnl)"=w806) -> ()  [unwired: 2 in, 2 out]
          }
        }
      }
      event "Trap 1 (ON/OFF)", "Trap 2 (ON/OFF)": Value Change {
        n517 = event-data() -> ()  [unwired: 7 out]
        n518 = property on="Trap 2 ON" class="Bool (strict)"("Val(Sgnl)"="Trap 2 (ON/OFF)") -> ()  [unwired: 2 in, 2 out]
        n519 = property on="Trap 1 ON" class="Bool (strict)"("Val(Sgnl)"="Trap 1 (ON/OFF)") -> ()  [unwired: 2 in, 2 out]
      }
      event "DIO count 1 (ticks)", "DIO count 2 (ticks)", "DIO count 3 (ticks)", "Interlace", "Number Interlace Sets", "Not-Interlacing Set": Value Change {
        n520 = event-data() -> ()  [unwired: 7 out]
        n521 = local read "DIO count 3 (ticks)"() -> (w819:u32)
        n522 = local read "DIO count 1 (ticks)"() -> (w821:u32)
        n523 = local read "DIO count 2 (ticks)"() -> (w820:u32)
        n524 = To Unsigned Byte Integer(number="Not-Interlacing Set") -> (unsigned 8bit integer=w810:u8)
        n525 = Add(x=w810, y=u8 1) -> (x+y=w814:u8)
        n526 = xnode "Read/Write Control"("FPGA VI Reference In"=w825, "error in"=w823, "DIO count 1 (ticks)"=w821, "DIO count 2 (ticks)"=w820, "DIO count 3 (ticks)"=w819, "Interlace ON/OFF"="Interlace", "Number Interlace Cycles"="Number Interlace Sets", "Interlace Off Parameters"=w814) -> ("error out"=w824:errorcluster)  [unwired: 1 out]
        n527 = Build Array(w821, w820, w819) -> (w812:u32[])
        n528 = Split 1D Array(array=w812, index="Number Interlace Sets") -> (first subarray=w822:u32[])  [unwired: 1 out]
        n529 = Index Array(array=w812, index=w810) -> (element=w811:u32)
        n530 = Add Array Elements(numeric array=w822) -> (sum=w816:u32)
        n531 = Select(t=w816, s="Interlace", f=w811) -> (s? t:f=→"Total Counts (ticks)":u32)
      }
      event "Reset Feedback": Value Change {
        n532 = event-data() -> ()  [unwired: 7 out]
        n533 = Unbundle By Name("Reset Feedback") -> ("Set 1"=w829:bool, "Set 2"=w828:bool)
        n534 = xnode "Read/Write Control"("FPGA VI Reference In"=w831, "error in"=w826, "FB Reset Set 1"=w829, "FB Reset Set 2"=w828) -> ("error out"=w827:errorcluster)  [unwired: 1 out]
      }
      event "PID gains": Value Change {
        n535 = event-data() -> ()  [unwired: 7 out]
        n536 = local read "PID gains"() -> (w832:T10)
        n537 = xnode "Read/Write Control"("FPGA VI Reference In"=w835, "error in"=w833, "FB Gains"=w832) -> ("error out"=w834:errorcluster)  [unwired: 1 out]
      }
      event "AI2 to Setpoint", "Trap Intensity\nSetpoints (V)": Value Change {
        n538 = event-data() -> ()  [unwired: 7 out]
        n539 = xnode "Read/Write Control"("FPGA VI Reference In"=w840, "error in"=w836) -> ("FPGA VI Reference Out"=w839:T20, "error out"=w838:errorcluster, "AI2 Y Sum Set 1"=w847:i16, "AI2 Y Sum Set 2"=w846:i16)
        n540 = Cluster To Array(cluster="AI2 to Setpoint") -> (array=w850:bool[])
        n541 = local read "AI2 (V)"() -> (w848:cluster{"Set 1":dbl, "Set 2":dbl})
        n542 = Or Array Elements(Boolean array=w850) -> (logical OR=w851:bool)
        n543 = Bundle By Name(cluster=w848, "Set 1"=w847, "Set 2"=w846) -> (w845:cluster{"Set 1":dbl, "Set 2":dbl})
        n544 = Divide(x=w845, y=3276.7) -> (x/y=w844:cluster{"Set 1":dbl, "Set 2":dbl})
        "AI2 (V)" <- w844
        n545 = case shown="True" w851 {
          tunnel: [w854 w871] -> w843
          tunnel: "AI2 to Setpoint" -> [_ w867]
          tunnel: "Trap Intensity\nSetpoints (V)" -> [w855 w870]
          tunnel: w844 -> [_ w864]
          frame False {
            n546 = Multiply(x=3276.7, y=w855) -> (x*y=w856:cluster{"Set 1":dbl, "Set 2":dbl})
            n547 = To Word Integer(number=w856) -> (16bit integer=w854:cluster{"Set 1":i16, "Set 2":i16})
          }
          frame True {
            n548 = Unbundle By Name(w864) -> ("Set 1"=w863:dbl, "Set 2"=w862:dbl)
            n549 = Unbundle By Name(w870) -> ("Set 1"=w869:dbl, "Set 2"=w868:dbl)
            n550 = Unbundle By Name(w867) -> ("Set 1"=w866:bool, "Set 2"=w865:bool)
            n551 = Select(t=w863, s=w866, f=w869) -> (s? t:f=w861:dbl)
            n552 = Select(t=w862, s=w865, f=w868) -> (s? t:f=w860:dbl)
            n553 = Bundle By Name(cluster=w870, "Set 1"=w861, "Set 2"=w860) -> (w858:cluster{"Set 1":dbl, "Set 2":dbl})
            n554 = local write "Trap Intensity\nSetpoints (V)"(w858) -> ()
            n555 = Multiply(x=3276.7, y=w858) -> (x*y=w859:cluster{"Set 1":dbl, "Set 2":dbl})
            n556 = To Word Integer(number=w859) -> (16bit integer=w871:cluster{"Set 1":i16, "Set 2":i16})
          }
        }
        n557 = Unbundle By Name(w843) -> ("Set 1"=w842:i16, "Set 2"=w841:i16)
        n558 = xnode "Read/Write Control"("FPGA VI Reference In"=w839, "error in"=w838, "FB Setpoint Set 1"=w842, "FB Setpoint Set 2"=w841) -> ("error out"=w837:errorcluster)  [unwired: 1 out]
      }
      event "Invert GI": Value Change {
        n559 = event-data() -> ()  [unwired: 7 out]
        n560 = xnode "Read/Write Control"("FPGA VI Reference In"=w876, "error in"=w874, "Invert GI"="Invert GI", "Invert GI 2"="Invert GI") -> ("error out"=w875:errorcluster)  [unwired: 1 out]
      }
      event "Green FB Setpoint (mV)", "Green FB Gains", "Green FB On/Off", "Current When FB OFF (%)", "Green int current ON count adj": Value Change {
        n561 = event-data() -> ()  [unwired: 7 out]
        n562 = local read "Green FB Setpoint (mV)"() -> (w883:dbl)
        n563 = local read "Current When FB OFF (%)"() -> (w886:dbl)
        n564 = Multiply(x=w883, y=3.2767) -> (x*y=w882:dbl)
        n565 = Multiply(x=w886, y=655.35) -> (x*y=w887:dbl)
        n566 = To Unsigned Word Integer(number=w887) -> (unsigned 16bit integer=w885:u16)
        n567 = local read "Green int current ON count adj"() -> (w890:u32)
        n568 = local read "Green FB Gains"() -> (w889:T10)
        n569 = local read "Green Laser ON/Interlacing"() -> (w880:bool)
        n570 = local read "Green laser mode"() -> (w879:enum32{"Laser ON", "Laser OFF", "Interlace"})
        n571 = local read "Green FB On/Off"() -> (w891:bool)
        n572 = Equal?(x=w879, y=enum32{"Laser ON", "Laser OFF", "Interlace"}."Interlace") -> (x = y?=w877:bool)
        n573 = Compound Arithmetic op=AND(w877, w891, w880) -> (w881:bool)
        n574 = xnode "Read/Write Control"("FPGA VI Reference In"=w894, "error in"=w893, "Green FB Setpoint"=w882, "Green FB On/Off"=w881, "Current Out"=w885, "Green int current ON count adj"=w890, "Green FB Gains"=w889) -> ("error out"=w892:errorcluster)  [unwired: 1 out]
      }
      event "Green laser mode", "Green Laser ON/Interlacing": Value Change {
        n575 = event-data() -> ()  [unwired: 7 out]
        n576 = case shown="True" "Green Laser ON/Interlacing" {
          tunnel: "Green laser mode" -> [_ w908]
          tunnel: [enum32{"Laser ON", "Laser OFF", "Interlace"}."Laser OFF" ("Green laser mode") w908] -> w896
          tunnel: [FALSE w904] -> w895
          frame False {
          }
          frame True {
            n577 = local read "Green FB On/Off"() -> (w905:bool)
            n578 = Equal?(x=w908, y=enum32{"Laser ON", "Laser OFF", "Interlace"}."Interlace") -> (x = y?=w906:bool)
            n579 = And(x=w906, y=w905) -> (x .and. y?=w904:bool)
          }
        }
        n580 = xnode "Read/Write Control"("FPGA VI Reference In"=w901, "error in"=w899, "Operating Mode"=w896, "Operating Mode 2"=w896, "Green FB On/Off"=w895) -> ("error out"=w900:errorcluster)  [unwired: 1 out]
      }
      event "- phase (APD 1 Gate)", "+ phase (APD 1 Gate)": Value Change {
        n581 = event-data() -> ()  [unwired: 7 out]
        n582 = local read "Phase Adj. (APD 1 Gate)"() -> (w909:i16)
        n583 = Negate(x=w909) -> (-x=w917:i16)
        n584 = Select(t=w917, s="- phase (APD 1 Gate)", f=w909) -> (s? t:f=w916:i16)
        n585 = Or(x="- phase (APD 1 Gate)", y="+ phase (APD 1 Gate)") -> (x .or. y?=w912:bool)
        n586 = xnode "Read/Write Control"("FPGA VI Reference In"=w919, "error in"=w918, "Phase count adjustment (APD 1 Gate)"=w916) -> ("FPGA VI Reference Out"=w914:T20, "error out"=w915:errorcluster)
        n587 = xnode "Read/Write Control"("FPGA VI Reference In"=w914, "error in"=w915, "+ phase (APD 1 Gate)"=w912) -> ("error out"=w913:errorcluster)  [unwired: 1 out]
      }
      event "+ phase (APD 2 Gate)", "- phase (APD 2 Gate)": Value Change {
        n588 = event-data() -> ()  [unwired: 7 out]
        n589 = local read "Phase Adj. (APD 2 Gate)"() -> (w920:i16)
        n590 = Negate(x=w920) -> (-x=w928:i16)
        n591 = Select(t=w928, s="- phase (APD 2 Gate)", f=w920) -> (s? t:f=w927:i16)
        n592 = Or(x="- phase (APD 2 Gate)", y="+ phase (APD 2 Gate)") -> (x .or. y?=w923:bool)
        n593 = xnode "Read/Write Control"("FPGA VI Reference In"=w930, "error in"=w929, "Phase count adjustment (APD 2 Gate)"=w927) -> ("FPGA VI Reference Out"=w925:T20, "error out"=w926:errorcluster)
        n594 = xnode "Read/Write Control"("FPGA VI Reference In"=w925, "error in"=w926, "+ phase (APD 2 Gate)"=w923) -> ("error out"=w924:errorcluster)  [unwired: 1 out]
      }
      event "Phase Adj. (APD Acq)", "+ phase (APD Acq)", "- phase (APD Acq)": Value Change {
        n595 = event-data() -> ()  [unwired: 7 out]
        n596 = local read "Phase Adj. (APD Acq)"() -> (w933:i16)
        n597 = Negate(x=w933) -> (-x=w939:i16)
        n598 = Select(t=w939, s="+ phase (APD Acq)", f=w933) -> (s? t:f=w938:i16)
        n599 = Or(x="+ phase (APD Acq)", y="- phase (APD Acq)") -> (x .or. y?=w934:bool)
        n600 = xnode "Read/Write Control"("FPGA VI Reference In"=w941, "error in"=w940, "Phase Count Adjustment (APD Acq)"=w938) -> ("FPGA VI Reference Out"=w936:T20, "error out"=w937:errorcluster)
        n601 = xnode "Read/Write Control"("FPGA VI Reference In"=w936, "error in"=w937, "+ phase (APD Acq)"=w934) -> ("error out"=w935:errorcluster)  [unwired: 1 out]
      }
      event "Phase adj. (GI)", "+ phase (GI)", "- phase (GI)": Value Change {
        n602 = event-data() -> ()  [unwired: 7 out]
        n603 = Negate(x="Phase adj. (GI)") -> (-x=w950:i16)
        n604 = Select(t=w950, s="+ phase (GI)", f="Phase adj. (GI)") -> (s? t:f=w949:i16)
        n605 = Or(x="+ phase (GI)", y="- phase (GI)") -> (x .or. y?=w945:bool)
        n606 = xnode "Read/Write Control"("FPGA VI Reference In"=w952, "error in"=w951, "Phase count adjustment (GI)"=w949) -> ("FPGA VI Reference Out"=w947:T20, "error out"=w948:errorcluster)
        n607 = xnode "Read/Write Control"("FPGA VI Reference In"=w947, "error in"=w948, "+ phase (GI)"=w945) -> ("error out"=w946:errorcluster)  [unwired: 1 out]
      }
      event "Phase adj. (GI) 2", "+ phase (GI) 2", "- phase (GI) 2": Value Change {
        n608 = event-data() -> ()  [unwired: 7 out]
        n609 = Negate(x="Phase adj. (GI) 2") -> (-x=w961:i16)
        n610 = Select(t=w961, s="+ phase (GI) 2", f="Phase adj. (GI) 2") -> (s? t:f=w960:i16)
        n611 = Or(x="+ phase (GI) 2", y="- phase (GI) 2") -> (x .or. y?=w956:bool)
        n612 = xnode "Read/Write Control"("FPGA VI Reference In"=w963, "error in"=w962, "Phase count adjustment (GI) 2"=w960) -> ("FPGA VI Reference Out"=w958:T20, "error out"=w959:errorcluster)
        n613 = xnode "Read/Write Control"("FPGA VI Reference In"=w958, "error in"=w959, "+ phase (GI) 2"=w956) -> ("error out"=w957:errorcluster)  [unwired: 1 out]
      }
      event "Phase adj. (Green FB)", "- phase (Green FB)", "+ phase (Green FB)": Value Change {
        n614 = event-data() -> ()  [unwired: 7 out]
        n615 = Negate(x="Phase adj. (Green FB)") -> (-x=w972:i16)
        n616 = Select(t=w972, s="+ phase (Green FB)", f="Phase adj. (Green FB)") -> (s? t:f=w971:i16)
        n617 = Or(x="+ phase (Green FB)", y="- phase (Green FB)") -> (x .or. y?=w967:bool)
        n618 = xnode "Read/Write Control"("FPGA VI Reference In"=w974, "error in"=w973, "Phase count adjustment (Green FB)"=w971) -> ("FPGA VI Reference Out"=w969:T20, "error out"=w970:errorcluster)
        n619 = xnode "Read/Write Control"("FPGA VI Reference In"=w969, "error in"=w970, "+ phase (Green FB)"=w967) -> ("error out"=w968:errorcluster)  [unwired: 1 out]
      }
      event "Invert APD Gate", "APD Gate ON Count", "APD Gate OFF Count", "APD Gate", "APD Integration Time (s)", "APD 1 AO Mult.", "APD 2 AO Mult.": Value Change {
        n620 = event-data() -> ()  [unwired: 7 out]
        n621 = local read "APD Integration Time (s)"() -> (w975:dbl)
        n622 = local read "APD Gate ON Count"() -> (w988:u32)
        n623 = local read "APD Gate OFF Count"() -> (w987:u32)
        n624 = local read "Invert APD Gate"() -> (w989:bool)
        n625 = local read "APD Gate"() -> (w986:enum32{"ON", "OFF", "Interlace"})
        n626 = Multiply(x=w975, y=40000000.0) -> (x*y=w984:dbl)
        n627 = Reciprocal(x=w975) -> (1/x=→"APD Acq Rate (Hz)":dbl)
        n628 = To Unsigned Long Integer(number=w984) -> (unsigned 32bit integer=w983:u32)
        n629 = local read "DMA Update Period (s)"() -> (w976:dbl)
        n630 = Divide(x=w976, y=w975) -> (x/y=w979:dbl)
        n631 = local read "APD 1 AO Mult."() -> (w981:i16)
        n632 = local read "APD 2 AO Mult."() -> (w980:i16)
        n633 = Multiply(x=2.0, y=w979) -> (x*y=w978:dbl)
        n634 = local write "APD Samples/FIFO Acq."(w979) -> ()
        n635 = local write "APD Elements/DMA read"(w978) -> ()
        n636 = xnode "Read/Write Control"("FPGA VI Reference In"=w992, "error in"=w991, "Invert APD Gate"=w989, "APD Gate ON Count"=w988, "APD Gate OFF Count"=w987, "APD Acq Rate Count"=w983, "APD Gate Operating Mode"=w986, "APD 1 AO scale factor"=w981, "APD 2 AO scale factor"=w980) -> ("error out"=w990:errorcluster)  [unwired: 1 out]
      }
      event "GI Frequency, ON count", "Green FB Count", "GI Frequency, OFF count": Value Change {
        n637 = event-data() -> ()  [unwired: 7 out]
        n638 = xnode "Read/Write Control"("FPGA VI Reference In"=w998, "error in"=w996, "Green interlace ON count"="GI Frequency, ON count", "Green interlace OFF count"="GI Frequency, OFF count", "Green interlace ON count 2"="GI Frequency, ON count", "Green interlace OFF count 2"="GI Frequency, OFF count", "Green FB Count"="Green FB Count") -> ("error out"=w997:errorcluster)  [unwired: 1 out]
      }
      event "Number of F/B Scans (AOD)", "Scan Speed (nm/s)", "Scan BD", "Initial delta (MHz)", "Step Size (nm)", "Scan Range (nm)": Value Change {
        w1060 = 123.0  # AOM cal (nm/MHz)
        n639 = event-data() -> ()  [unwired: 7 out]
        n640 = local read "AOM X Cal (nm/MHz)"() -> (w1035:dbl)
        n641 = local read "X RF Frequency Limits (MHz)"() -> (w1047:T16)
        n642 = local read "Y RF Frequency Limits (MHz)"() -> (w1044:T16)
        n643 = local read "BD 1 Frq 1 (MHz)"() -> (w1043:dbl)
        n644 = local read "BD 2 Frq 1 (MHz)"() -> (w1049:dbl)
        n645 = Negate(x="Scan Range (nm)") -> (-x=w1013:dbl)
        n646 = Divide(x=w1013, y=w1035) -> (x/y=w1017:dbl)
        n647 = Select(t=w1047, s="Scan BD", f=w1044) -> (s? t:f=w1046:T16)
        n648 = Select(t=w1043, s="Scan BD", f=w1049) -> (s? t:f=w1048:dbl)
        n649 = Unbundle By Name(w1046) -> ("Maximum"=w1055:dbl, "Minimum"=w1054:dbl)
        n650 = Add(x=w1017, y=w1048) -> (x+y=w1052:dbl)
        n651 = Divide(x=w1013, y="Step Size (nm)") -> (x/y=w1032:dbl)
        n652 = Divide(x="Step Size (nm)", y=w1035) -> (x/y=w1041:dbl)
        n653 = Absolute Value(x=w1032) -> (abs(x)=w1016:dbl)
        n654 = Sign(1:w1013) -> (0:w1014:dbl)
        n655 = In Range and Coerce(upper limit=w1055, x=w1052, lower limit=w1054) -> (coerced(x)=w1051:dbl, In Range?=w1053:bool)
        n656 = To Unsigned Quad Integer(1:w1016) -> (0:w1031:u64)
        "Scan steps (AOD)" <- w1031
        n657 = call "IR AOM freq to word.vi"("Frequency In (MHz)"=w1041) -> ("Frequency Word Out (double)"=w1038:dbl)
        n658 = Multiply(x=w1014, y=w1038) -> (x*y=w1015:dbl)
        n659 = Subtract(x=w1052, y=w1051) -> (x-y=w1050:dbl)
        n660 = To Quad Integer(1:w1015) -> (0:w1037:i64)
        "Incr. int (AOD)" <- w1037
        n661 = Subtract(x=w1017, y=w1050) -> (x-y=w1036:dbl)
        "Scan Range (MHz)" <- w1036
        n662 = Select(t=w1017, s=w1053, f=w1036) -> (s? t:f=w1056:dbl)
        n663 = Multiply(x=w1036, y=w1035) -> (x*y=w1034:dbl)
        n664 = Decrement(x=w1031) -> (x-1=w1084:u64)
        n665 = Negate(x=w1034) -> (-x=w1030:dbl)
        n666 = local write "Scan Range (nm)"(w1030) -> ()
        n667 = Divide(x=w1056, y=w1084) -> (x/y=w1040:dbl)
        "Scan Increment (MHz)" <- w1040
        n668 = call "IR AOM freq to word.vi"("Frequency In (MHz)"=w1040) -> ("Frequency Word Out (double)"=w1039:dbl)
        n669 = Divide(x="Step Size (nm)", y="Scan Speed (nm/s)") -> (x/y=w1027:dbl)
        n670 = To Quad Integer(1:w1039) -> ()  [unwired: 1 out]
        n671 = local read "Number Interlace Sets"() -> (w1011:u8)
        n672 = local read "AI Count (ticks)"() -> (w1012:u32)
        n673 = local read "Total Counts (ticks)"() -> (w1010:u32)
        n674 = local read "# Samples/trap"() -> (w1042:u32)
        n675 = Multiply(x=w1012, y=w1011) -> (x*y=w1009:u32)
        n676 = Divide(x=w1010, y=w1009) -> (x/y=w1008:dbl)
        n677 = Select(t=w1043, s="Scan BD", f=w1049) -> (s? t:f=w1081:dbl)
        "Initial freq. (MHz)" <- w1081
        n678 = Add(x=w1056, y=w1081) -> (x+y=→"Final freq. (MHz)":dbl)
        n679 = Divide(x=w1010, y=40000000.0) -> (x/y=w1026:dbl)
        n680 = Divide(x=w1027, y=w1026) -> (x/y=w1025:dbl)
        n681 = To Unsigned Quad Integer(1:w1025) -> (0:w1000:u64)
        n682 = Quotient & Remainder(x=w1000, y=u64 2) -> (x-y*floor(x/y)=w1004:u64)  [unwired: 1 out]
        n683 = Equal?(x=w1004, y=u64 0) -> (x = y?=w1002:bool)
        n684 = Decrement(x=w1000) -> (x-1=w1001:u64)
        n685 = Select(t=w1000, s=w1002, f=w1001) -> (s? t:f=w999:u64)
        "Cycles/step (AOD)" <- w999
        n686 = xnode "Read/Write Control"("FPGA VI Reference In"=w1092, "error in"=w1091, "Scan steps"=w1031, "Number of scans"="Number of F/B Scans (AOD)", "Cycles per step"=w999, "Scan freq.  increment"=w1037, "Scan BD"="Scan BD") -> ("error out"=w1090:errorcluster)  [unwired: 1 out]
        n687 = Multiply(x=w1031, y=w999) -> (x*y=w1085:u64)
        n688 = Multiply(x=w1085, y=u64 2) -> (x*y=w1007:u64)
        n689 = Multiply(x=w1008, y=w1007) -> (x*y=w1006:dbl)
        "Data points/scan (f/b)" <- w1006
        n690 = Multiply(x=w1006, y="Number of F/B Scans (AOD)") -> (x*y=w1088:dbl)
        "Data points/scans" <- w1088
        n691 = Divide(x=w1088, y=w1042) -> (x/y=→"N sets should be saved":dbl)
        n692 = Multiply(x=w1085, y=w1026) -> (x*y=w1024:dbl)
        "Time/Scan (s) (AOD)" <- w1024
        n693 = Select(t=w1056, s="Scan BD", f=0.0) -> (s? t:f=w1082:dbl)
        n694 = Select(t=0.0, s="Scan BD", f=w1056) -> (s? t:f=w1078:dbl)
        n695 = local read "BD 2 Frq 2 (MHz)"() -> (w1074:dbl)
        n696 = local read "BD 1 Frq 2 (MHz)"() -> (w1077:dbl)
        n697 = Add(x=w1078, y=w1049) -> (x+y=w1075:dbl)
        n698 = Add(x=w1043, y=w1082) -> (x+y=w1076:dbl)
        n699 = Multiply(x=w1024, y=2.0) -> (x*y=w1023:dbl)
        n700 = Multiply(x=w1023, y="Number of F/B Scans (AOD)") -> (x*y=w1020:dbl)
        n701 = Divide(x=w1020, y=60.0) -> (x/y=→"Time to Finish All (min)":dbl)
        n702 = Add(x="Trap 2 Bead Size (nm)", y="Trap 1 Bead Size (nm)") -> (x+y=w1064:dbl)
        n703 = local read "Initial delta (MHz)"() -> (w1061:dbl)
        n704 = Divide(x=w1064, y=2.0) -> (x/y=w1058:dbl)
        n705 = Subtract(x=w1075, y=w1074) -> (x-y=w1072:dbl)
        n706 = Subtract(x=w1076, y=w1077) -> (x-y=w1073:dbl)
        n707 = Square(x=w1072) -> (x^2=w1071:dbl)
        n708 = Square(x=w1073) -> (x^2=w1070:dbl)
        n709 = Add(x=w1070, y=w1071) -> (x+y=w1069:dbl)
        n710 = Square Root(x=w1069) -> (sqrt(x)=w1068:dbl)
        "Final delta (MHz)" <- w1068
        n711 = Multiply(x=w1060, y=w1068) -> (x*y=w1067:dbl)
        n712 = Multiply(x=w1061, y=w1060) -> (x*y=w1059:dbl)
        n713 = Subtract(x=w1059, y=w1058) -> (x-y=→"Initial sep (nm)":dbl)
        n714 = Subtract(x=w1067, y=w1058) -> (x-y=→"Final sep (nm)":dbl)
      }
      event "Raster Scanning...": Value Change {
        n715 = event-data() -> ("NewVal"=w1093:bool)  [unwired: 6 out]
        n716 = case shown="True" w1093 {
          frame False {
          }
          frame True {
            n717 = property on="BD 1 Frq 1 (MHz)" class="DigNum (strict)"("Val(Sgnl)"=65.0 ("Value (Signaling)")) -> ()  [unwired: 2 in, 2 out]
          }
        }
      }
      event "Phase increment trap 1", "Swap F1 and F2", "Freq switch delay", "Amp switch delay", "Phase increment trap 2", "RF phase reset before cycles", "Phase offset method": Value Change {
        n718 = event-data() -> ()  [unwired: 7 out]
        n719 = local read "Amp switch delay"() -> (w1099:u16)
        n720 = local read "Phase increment trap 1"() -> (w1098:fxp<+/-,64,32>)
        n721 = local read "Freq switch delay"() -> (w1101:u16)
        n722 = local read "Phase increment trap 2"() -> (w1097:fxp<+/-,64,32>)
        n723 = local read "RF phase reset before cycles"() -> (w1096:bool)
        n724 = local read "Swap F1 and F2"() -> (w1100:bool)
        n725 = local read "Phase offset method"() -> (w1095:u8)
        n726 = xnode "Read/Write Control"("FPGA VI Reference In"=w1104, "error in"=w1103, "BD 1 Delay (ticks)"=w1101, "Swap F1 and F2"=w1100, "Amp switch delay"=w1099, "Phase Trap 1"=w1098, "Phase Trap 2"=w1097, "RF phase reset before cycles"=w1096, "Phase offset method"=w1095) -> ("error out"=w1102:errorcluster)  [unwired: 1 out]
      }
      event "Scan steps (x)", "Number of scans (MCL)", "Scan Range (V)\n(of steps)", "2D or 1D Scan", "N APD Samp/step", "Fast Scan Dir", "Continuous MCL Scanning", "Scan lines (y)": Value Change {
        w1106 = 32767.0 ("y")
        n727 = event-data() -> ()  [unwired: 7 out]
        n728 = Select(t="Scan lines (y)", s="2D or 1D Scan", f="Number of scans (MCL)") -> (s? t:f=w1111:u64)
        n729 = Decrement(x="Scan steps (x)") -> (x-1=w1127:u64)
        n730 = Divide(x="Scan Range (V)\n(of steps)", y=w1127) -> (x/y=w1126:dbl)
        "Desired Scan Incr (V)" <- w1126
        n731 = local read "APD Integration Time (s)"() -> (w1119:dbl)
        n732 = Multiply(x=w1126, y=w1106) -> (x*y=w1135:dbl)
        n733 = Divide(x=w1135, y=10.0) -> (x/y=w1125:dbl)
        "Desired incr (int)" <- w1125
        n734 = local read "Update Count (MCL)"() -> (w1131:u32)
        n735 = Round Toward -Infinity(1:w1125) -> (0:w1134:dbl)
        n736 = To Word Integer(number=w1134) -> (16bit integer=w1109:i16)
        "Actual Incr. int (MCL)" <- w1109
        n737 = Multiply(x=w1119, y=40000000.0) -> (x*y=w1132:dbl)
        n738 = Divide(x=w1132, y=w1131) -> (x/y=w1130:dbl)
        n739 = Multiply(x=i16 10, y=w1109) -> (x*y=w1107:i16)
        n740 = Multiply(x="N APD Samp/step", y=w1130) -> (x*y=w1129:dbl)
        "Cycles/step (MCL)" <- w1129
        n741 = Divide(x=w1107, y=w1106) -> (x/y=→"Actual MCL Inc (V)":dbl)
        n742 = Multiply(x="N APD Samp/step", y="Scan steps (x)") -> (x*y=w1121:u64)
        n743 = local read "APD Samples/FIFO Acq."() -> (w1118:dbl)
        n744 = Multiply(x=w1121, y=u64 2) -> (x*y=w1120:u64)
        "Data points/scan (f+b)" <- w1120
        n745 = Multiply(x=w1120, y=w1111) -> (x*y=w1138:u64)
        "Data points/scans (MCL)" <- w1138
        n746 = Multiply(x=w1119, y=w1120) -> (x*y=w1112:dbl)
        "Time/f+b scan (s) (MCL)" <- w1112
        n747 = Divide(x=w1138, y=w1118) -> (x/y=→"N sets should be saved (MCL)":dbl)
        n748 = Multiply(x=w1112, y=w1111) -> (x*y=→"Total Time (s)":dbl)
        n749 = Not(x="Fast Scan Dir") -> (.not. x?=w1116:bool)
        n750 = xnode "Read/Write Control"("FPGA VI Reference In"=w1142, "error in"=w1141, "Scan steps (MCL)"="Scan steps (x)", "Number of scans (MCL)"=w1111, "Cycles per step (MCL)"=w1129, "Scan freq.  increment (MCL)"=w1109, "1D or 2D Scan?"="2D or 1D Scan", "MCL Scan Axis"=w1116, "Cont. Scan (MCL)"="Continuous MCL Scanning") -> ("error out"=w1140:errorcluster)  [unwired: 1 out]
      }
      event "Read Cal": Value Change {
        w1179 = 1000.0 ("y")
        w1167 = T28."big-endian, network order" ("byte order (0:big-endian, network order)")
        w1168 = -1 ("count (1)")
        n751 = event-data() -> ()  [unwired: 7 out]
        n752 = local read "Save file name"() -> (w1197:path)
        n753 = local write "Read Cal"(FALSE ("Read Cal")) -> ()
        n754 = Strip Path(path=w1197) -> (stripped path=w1196:path)  [unwired: 1 out]
        n755 = Path To String(path=w1196) -> (string=w1177:string)
        n756 = Concatenate Strings(w1177, "\\current.off" ("string")) -> (w1175:string)
        n757 = Concatenate Strings(w1177, "\\current.cal" ("string")) -> (w1194:string)
        n758 = local read "Scale intensities"() -> (w1147:bool)
        n759 = String To Path(string=w1194) -> (path=w1193:path)
        n760 = String To Path(string=w1175) -> (path=w1174:path)
        n761 = Open/Create/Replace File(file path (use dialog)=w1193, operation (0:open)=T27."open", access (0:read/write)=enum16{"read/write", "read-only", "write-only"}."read-only") -> (refnum out=w1200:refnum<file>, error out=w1189:errorcluster)  [unwired: 1 in, 3 out]
        n762 = Deny Access(4:w1189, 7:w1200) -> (0:w1188:errorcluster, 3:w1192:refnum<file>)  [unwired: 1 out]
        n763 = Open/Create/Replace File(file path (use dialog)=w1174, operation (0:open)=T27."open", access (0:read/write)=enum16{"read/write", "read-only", "write-only"}."read-only") -> (refnum out=w1171:refnum<file>)  [unwired: 1 in, 4 out]
        n764 = Deny Access(7:w1171) -> (3:w1169:refnum<file>)  [unwired: 1 in, 2 out]
        n765 = Read from Binary File(5:0.0, 8:w1188, 9:w1167, 10:w1168, 11:w1192) -> (0:w1187:errorcluster, 2:w1185:dbl[], 3:w1190:refnum<file>)  [unwired: 2 out]
        n766 = Array To Cluster(array=w1185) -> (cluster=w1184:T30)
        n767 = Unbundle(w1184) -> ("[0]"=w1158:dbl, "[1]"=w1157:dbl, "[2]"=w1144:dbl, "[3]"=w1146:dbl, "[4]"=w1183:dbl, "[5]"=w1182:dbl)
        n768 = case "Cal is OK if you load a cal with scale intensities on - Alex 081418" shown="True" w1147 {
          tunnel: w1146 -> [w1202 w1205]
          tunnel: [w1202 w1204] -> w1145
          tunnel: w1144 -> [w1201 w1207]
          tunnel: [w1201 w1206] -> w1143
          frame False {
          }
          frame True {
            n769 = local read "Scale factor"() -> (w1203:dbl)
            n770 = Multiply(x=w1205, y=w1203) -> (x*y=w1204:dbl)
            n771 = Multiply(x=w1207, y=w1203) -> (x*y=w1206:dbl)
          }
        }
        n772 = Close File(refnum=w1190, error in=w1187) -> (error out=→"Read cal error":errorcluster)  [unwired: 1 out]
        n773 = Multiply(x=w1182, y=w1179) -> (x*y=w1180:dbl)
        n774 = local write "T2 kappa_x (pN/nm)"(w1145) -> ()
        n775 = local write "T1 kappa_x (pN/nm)"(w1143) -> ()
        n776 = local write "T1 alpha_x (nm/V)"(w1158) -> ()
        n777 = local write "T2 alpha_x (nm/V)"(w1157) -> ()
        n778 = Read from Binary File(5:0.0, 9:w1167, 10:w1168, 11:w1169) -> (2:w1163:dbl[], 3:w1166:refnum<file>)  [unwired: 1 in, 3 out]
        n779 = Multiply(x=w1183, y=w1179) -> (x*y=w1181:dbl)
        n780 = local write "T1 offset_x (mV)"(w1181) -> ()
        n781 = local write "T2 offset_x (mV)"(w1180) -> ()
        n782 = Close File(refnum=w1166) -> ()  [unwired: 1 in, 2 out]
        n783 = Array Subset(array=w1163, index=3) -> (w1161:dbl[])  [unwired: 1 in]
        n784 = Index Array(array=w1163, index=0) -> (element=→"Offset file step size":dbl)
        n785 = Multiply(x=w1158, y=w1144) -> (x*y=w1155:dbl)
        n786 = Multiply(x=w1157, y=w1146) -> (x*y=w1156:dbl)
        n787 = Divide(x=w1156, y=w1155) -> (x/y=w1149:dbl)
        n788 = Decimate 1D Array(w1161) -> (w1153:dbl[], w1154:dbl[])  [unwired: 1 out]
        n789 = disable-structure "Removed B factor to improve position FB -Alex 081418 2of3" shown="Enabled" {
          disable-tunnel: w1149 -> [w1208 _]
          disable-tunnel: [w1208 1.0] -> w1148
          frame Disabled {
          }
          frame Enabled {
          }
        }
        n790 = Bundle By Name(cluster="Offset Values", "Trap 1X offset"=w1153, "Trap 2X offset"=w1154) -> (w1159:T14)
        n791 = Multiply(x=w1154, y=w1148) -> (x*y=w1152:dbl[])
        n792 = Subtract(x=w1153, y=w1152) -> (x-y=w1151:dbl[])
        n793 = local write "Offset Values"(w1159) -> ()
        n794 = case shown="True" "Auto read offset\ncorrection" {
          tunnel: w1151 -> [_ w1210]
          frame False {
          }
          frame True {
            n795 = property on="Setpoint offset\nCorrection values" class="Arr (strict)"("Val(Sgnl)"=w1210) -> ()  [unwired: 2 in, 2 out]
          }
        }
        n796 = property on="B factor" class="DigNum (strict)"("Val(Sgnl)"=w1148) -> ()  [unwired: 2 in, 2 out]
      }
      event "Symmetric Raster/Feedback?": Value Change {
        n797 = event-data() -> ()  [unwired: 7 out]
        n798 = xnode "Read/Write Control"("FPGA VI Reference In"=w1212, "Symmetric FB/Raster"="Symmetric Raster/Feedback?") -> ()  [unwired: 1 in, 2 out]
      }
      event "Abort MCL Scan": Value Change {
        n799 = event-data() -> ()  [unwired: 7 out]
        n800 = local write "MCL Scanning"(FALSE ("MCL Scanning")) -> ()
        n801 = xnode "Read/Write Control"("FPGA VI Reference In"=w1217, "error in"=w1216, "Abort scan (MCL)"="Abort MCL Scan") -> ("error out"=w1215:errorcluster)  [unwired: 1 out]
      }
      event "Update Count (MCL)": Value Change {
        n802 = event-data() -> ()  [unwired: 7 out]
        n803 = xnode "Read/Write Control"("FPGA VI Reference In"=w1221, "error in"=w1220, "MCL count"="Update Count (MCL)") -> ("error out"=w1219:errorcluster)  [unwired: 1 out]
      }
      event "Phase adjust (MCL)", "+ phase (MCL)", "- phase (MCL)": Value Change {
        n804 = event-data() -> ()  [unwired: 7 out]
        n805 = Negate(x="Phase adjust (MCL)") -> (-x=w1230:i16)
        n806 = Select(t=w1230, s="- phase (MCL)", f="Phase adjust (MCL)") -> (s? t:f=w1228:i16)
        n807 = Or(x="- phase (MCL)", y="+ phase (MCL)") -> (x .or. y?=w1223:bool)
        n808 = xnode "Read/Write Control"("FPGA VI Reference In"=w1232, "error in"=w1231, "Phase count adjustment (MCL)"=w1228) -> ("FPGA VI Reference Out"=w1224:T20, "error out"=w1225:errorcluster)
        n809 = xnode "Read/Write Control"("FPGA VI Reference In"=w1224, "error in"=w1225, "+ phase (MCL)"=w1223) -> ("error out"=w1222:errorcluster)  [unwired: 1 out]
      }
      event "Abort AOD Scan": Value Change {
        n810 = event-data() -> ()  [unwired: 7 out]
        n811 = flat-sequence {
          tunnel: w1237 -> [w1244]
          tunnel: w1236 -> [w1243]
          tunnel: [w1242] -> w1234
          tunnel: [w1238] -> w1233
          tunnel: [w1257] -> w1235
          tunnel: w1234 -> [w1257]
          tunnel: w1233 -> [w1256]
          frame #0 {
            n812 = local read "Save scans"() -> (w1240:bool)
            n813 = xnode "Read/Write Control"("FPGA VI Reference In"=w1244, "error in"=w1243, "Abort scan"="Abort AOD Scan") -> ("FPGA VI Reference Out"=w1238:T20, "error out"=w1242:errorcluster)
            n814 = case shown="True" w1240 {
              frame False {
              }
              frame True {
                n815 = local write "Stop Saving"(TRUE) -> ()
              }
            }
            n816 = local write "Raster Scanning..."(FALSE) -> ()
          }
          frame #1 {
            n817 = xnode "Read/Write Control"("FPGA VI Reference In"=w1256) -> ("BD1 Frequency Out 1"=w1247:u64)  [unwired: 1 in, 2 out]
            n818 = To Double Precision Float(number=w1247) -> (double precision float=w1253:dbl)
            n819 = Multiply(x=49125000.0, y=6.0) -> (x*y=w1252:dbl)
            n820 = Multiply(x=w1253, y=w1252) -> (x*y=w1250:dbl)
            n821 = Scale By Power Of 2(n=-48, x=w1250) -> (x*2^n=w1249:dbl)
            n822 = Divide(x=w1249, y=1000000.0) -> (x/y=w1246:dbl)
            n823 = property on="BD 1 Frq 1 (MHz)" class="DigNum (strict)"("Val(Sgnl)"=w1246) -> ()  [unwired: 2 in, 2 out]
          }
        }
      }
      event "Continuous AOD Scanning": Value Change {
        n824 = event-data() -> ()  [unwired: 7 out]
        n825 = xnode "Read/Write Control"("FPGA VI Reference In"=w1261, "error in"=w1260, "Cont. Scan"="Continuous AOD Scanning") -> ("error out"=w1259:errorcluster)  [unwired: 1 out]
      }
      event "Index": Value Change {
        n826 = event-data() -> ()  [unwired: 7 out]
        n827 = call "Create new save file.vi"("Insert"="", "Ext"=".dat" ("string"), "Index In"="Index") -> ("Path Out"=→"Save file name":path, "Index Out"=w1262:dbl)
        "Save index" <- w1262
        n828 = local write "Index"(w1262) -> ()
      }
      event "MCL Y", "MCL X": Value Change {
        w1277 = 10.0 ("y")
        w1276 = 32767.0 ("y")
        n829 = event-data() -> ()  [unwired: 7 out]
        n830 = local read "MCL X"() -> (w1275:dbl)
        n831 = local read "MCL Y"() -> (w1272:dbl)
        n832 = Multiply(x=w1272, y=w1276) -> (x*y=w1271:dbl)
        n833 = Multiply(x=w1275, y=w1276) -> (x*y=w1274:dbl)
        n834 = Divide(x=w1271, y=w1277) -> (x/y=w1270:dbl)
        n835 = Divide(x=w1274, y=w1277) -> (x/y=w1273:dbl)
        n836 = To Word Integer(number=w1270) -> (16bit integer=w1278:i16)
        n837 = To Word Integer(number=w1273) -> (16bit integer=w1279:i16)
        n838 = xnode "Read/Write Control"("FPGA VI Reference In"=w1269, "error in"=w1268, "AO1 (Y)"=w1278, "AO2 (X)"=w1279) -> ("error out"=w1267:errorcluster)  [unwired: 1 out]
      }
      event "Inject Top:": Value Change {
        n839 = event-data() -> ()  [unwired: 7 out]
        n840 = disable-structure shown="Disabled" {
          disable-tunnel: "Inject Top:" -> [w1281 w1321]
          frame Disabled {
            n841 = local read "Chemyx Syringe Pump Serial Port"() -> (w1282:refnum<visa-resource-name>)
            n842 = local read "Pump write delay (ms)"() -> (w1283:dbl)
            n843 = case shown="True" w1281 {
              tunnel: w1283 -> [w1289 w1303]
              tunnel: w1282 -> [w1286 w1302]
              frame False {
                n844 = flat-sequence {
                  tunnel: w1286 -> [w1290]
                  tunnel: [w1290] -> w1287
                  tunnel: w1289 -> [_]
                  tunnel: [w1293] -> w1288
                  tunnel: w1287 -> [w1293]
                  tunnel: w1288 -> [w1294]
                  tunnel: [w1294] -> w1284
                  tunnel: [w1296] -> w1285
                  tunnel: w1284 -> [w1296]
                  tunnel: w1285 -> [w1298]
                  frame #0 {
                    n845 = call "Write to pump.vi"("string"="enter pump1", "VISA resource name"=w1290) -> ()  [unwired: 1 out]
                  }
                  frame #1 {
                    n846 = Wait (ms)(milliseconds to wait="Pump pause delay (ms)") -> ()  [unwired: 1 out]
                  }
                  frame #2 {
                    n847 = call "Write to pump.vi"("string"="stop", "VISA resource name"=w1294) -> ()  [unwired: 1 out]
                  }
                  frame #3 {
                    n848 = Wait (ms)(milliseconds to wait=u32 500) -> ()  [unwired: 1 out]
                  }
                  frame #4 {
                    n849 = call "Write to pump.vi"("string"="stop", "VISA resource name"=w1298) -> ()  [unwired: 1 out]
                  }
                }
              }
              frame True {
                n850 = flat-sequence {
                  tunnel: w1302 -> [w1312]
                  tunnel: w1303 -> [w1307]
                  tunnel: w1303 -> [w1314]
                  tunnel: w1302 -> [w1315]
                  tunnel: [w1315] -> w1300
                  tunnel: [w1317] -> w1301
                  tunnel: w1300 -> [w1317]
                  tunnel: w1301 -> [w1319]
                  frame #0 {
                    n851 = local read "All Pump Parameters"() -> (w1306:T6)
                    n852 = Unbundle By Name(w1306) -> ("Pump 1"=w1313:T31)
                    n853 = call "Set pump parameters.vi"("Pump write delay (ms)"=w1307, "Volume (uL)"="Ch 2 Inject Volume (uL)", "Rate (uL/h)"="Ch 1 Inject Rate (ul/h)", "Units"=4.0, "Pump #"=1.0, "Pump Parameters In"=w1313, "VISA resource name"=w1312) -> ("Pump Parameters Out"=w1305:T31)  [unwired: 3 in]
                    n854 = Bundle By Name(cluster=w1306, "Pump 1"=w1305) -> (w1304:T6)
                    n855 = local write "All Pump Parameters"(w1304) -> ()
                  }
                  frame #1 {
                    n856 = Wait (ms)(milliseconds to wait=w1314) -> ()  [unwired: 1 out]
                  }
                  frame #2 {
                    n857 = call "Write to pump.vi"("string"="start", "VISA resource name"=w1315) -> ()  [unwired: 1 out]
                  }
                  frame #3 {
                    n858 = Wait (ms)(milliseconds to wait=u32 500) -> ()  [unwired: 1 out]
                  }
                  frame #4 {
                    n859 = call "Write to pump.vi"("string"="start", "VISA resource name"=w1319) -> ()  [unwired: 1 out]
                  }
                }
              }
            }
          }
          frame Enabled {
            n860 = call "hamilton_controller.vi"("Open?"=w1321, "valve"=enum16{"A", "B", "C", "D", "ALL"}."B", "action"=T21."MOVE VALVE") -> ()  [unwired: 8 in, 1 out]
          }
        }
      }
      event "Main:": Value Change {
        n861 = event-data() -> ()  [unwired: 7 out]
        n862 = disable-structure shown="Enabled" {
          disable-tunnel: "Main:" -> [_ w1365]
          frame Disabled {
            n863 = local read "Pump write delay (ms)"() -> (w1326:dbl)
            n864 = case shown="False" w1327 {
              tunnel: w1326 -> [w1333 w1347]
              tunnel: "Chemyx Syringe Pump Serial Port" -> [w1330 w1346]
              frame False {
                n865 = flat-sequence {
                  tunnel: w1330 -> [w1334]
                  tunnel: [w1334] -> w1331
                  tunnel: w1333 -> [_]
                  tunnel: [w1337] -> w1332
                  tunnel: w1331 -> [w1337]
                  tunnel: w1332 -> [w1338]
                  tunnel: [w1338] -> w1328
                  tunnel: [w1340] -> w1329
                  tunnel: w1328 -> [w1340]
                  tunnel: w1329 -> [w1342]
                  frame #0 {
                    n866 = call "Write to pump.vi"("string"="enter pump3", "VISA resource name"=w1334) -> ()  [unwired: 1 out]
                  }
                  frame #1 {
                    n867 = local read "Pump pause delay (ms)"() -> (w1336:u32)
                    n868 = Wait (ms)(milliseconds to wait=w1336) -> ()  [unwired: 1 out]
                  }
                  frame #2 {
                    n869 = call "Write to pump.vi"("string"="stop", "VISA resource name"=w1338) -> ()  [unwired: 1 out]
                  }
                  frame #3 {
                    n870 = Wait (ms)(milliseconds to wait=u32 0) -> ()  [unwired: 1 out]
                  }
                  frame #4 {
                    n871 = call "Write to pump.vi"("string"="stop", "VISA resource name"=w1342) -> ()  [unwired: 1 out]
                  }
                }
              }
              frame True {
                n872 = flat-sequence {
                  tunnel: w1346 -> [w1356]
                  tunnel: w1347 -> [w1351]
                  tunnel: w1347 -> [w1358]
                  tunnel: w1346 -> [w1359]
                  tunnel: [w1359] -> w1344
                  tunnel: [w1362] -> w1345
                  tunnel: w1344 -> [w1362]
                  tunnel: w1345 -> [w1363]
                  frame #0 {
                    n873 = local read "All Pump Parameters"() -> (w1350:T6)
                    n874 = Unbundle By Name(w1350) -> ("Pump 3"=w1357:T31)
                    n875 = call "Set pump parameters.vi"("Pump write delay (ms)"=w1351, "Volume (uL)"="Ch 3 Inject Volume (uL)", "Rate (uL/h)"="Ch 3 Inject Rate (ul/h)", "Units"=4.0, "Pump #"=3.0, "Pump Parameters In"=w1357, "VISA resource name"=w1356) -> ("Pump Parameters Out"=w1349:T31)  [unwired: 3 in]
                    n876 = Bundle By Name(cluster=w1350, "Pump 3"=w1349) -> (w1348:T6)
                    n877 = local write "All Pump Parameters"(w1348) -> ()
                  }
                  frame #1 {
                    n878 = Wait (ms)(milliseconds to wait=w1358) -> ()  [unwired: 1 out]
                  }
                  frame #2 {
                    n879 = call "Write to pump.vi"("string"="start", "VISA resource name"=w1359) -> ()  [unwired: 1 out]
                  }
                  frame #3 {
                    n880 = Wait (ms)(milliseconds to wait=u32 500) -> ()  [unwired: 1 out]
                  }
                  frame #4 {
                    n881 = call "Write to pump.vi"("string"="start", "VISA resource name"=w1363) -> ()  [unwired: 1 out]
                  }
                }
              }
            }
          }
          frame Enabled {
            n882 = call "hamilton_controller.vi"("Open?"=w1365, "valve"=enum16{"A", "B", "C", "D", "ALL"}."A", "action"=T21."MOVE VALVE") -> ()  [unwired: 8 in, 1 out]
          }
        }
      }
      event "Inject Valve B": Value Change {
        n883 = event-data() -> ()  [unwired: 7 out]
        n884 = disable-structure shown="Enabled" {
          disable-tunnel: "Inject Valve B" -> [w1369 w1389]
          frame Disabled {
            n885 = local read "Pump write delay (ms)"() -> (w1371:dbl)
            n886 = flat-sequence {
              tunnel: w1370 -> [w1384]
              tunnel: w1371 -> [w1380]
              tunnel: w1369 -> [_]
              tunnel: w1371 -> [w1386]
              tunnel: w1370 -> [w1387]
              frame #0 {
                n887 = local read "All Pump Parameters"() -> (w1379:T6)
                n888 = Multiply(x=60.0, y="Flush Center Ch Rate (ul/m)") -> (x*y=w1376:dbl)
                n889 = Unbundle By Name(w1379) -> ("Pump 2"=w1385:T31)
                n890 = call "Set pump parameters.vi"("Pump write delay (ms)"=w1380, "Volume (uL)"="Flush Center Ch Volume (uL)", "Rate (uL/h)"=w1376, "Units"=3.0, "Pump #"=2.0, "Pump Parameters In"=w1385, "VISA resource name"=w1384) -> ("Pump Parameters Out"=w1378:T31)  [unwired: 3 in]
                n891 = Bundle By Name(cluster=w1379, "Pump 2"=w1378) -> (w1377:T6)
                n892 = local write "All Pump Parameters"(w1377) -> ()
                n893 = Add(x="Flush Center Ch Volume (uL)", y="Total Volume\nFlushed (uL)") -> (x+y=w1373:dbl)
                n894 = local write "Total Volume\nFlushed (uL)"(w1373) -> ()
              }
              frame #1 {
                n895 = Wait (ms)(milliseconds to wait=w1386) -> ()  [unwired: 1 out]
              }
              frame #2 {
                n896 = call "Write to pump.vi"("string"="start", "VISA resource name"=w1387) -> ()  [unwired: 1 out]
              }
            }
            n897 = local read "Chemyx Syringe Pump Serial Port"() -> (w1370:refnum<visa-resource-name>)
          }
          frame Enabled {
            n898 = call "hamilton_controller.vi"("Open?"=w1389, "valve"=enum16{"A", "B", "C", "D", "ALL"}."B", "action"=T21."MOVE VALVE") -> ()  [unwired: 8 in, 1 out]
          }
        }
      }
      event "Inject Bottom": Value Change {
        n899 = event-data() -> ()  [unwired: 7 out]
        n900 = call "hamilton_controller.vi"("Open?"="Inject Bottom", "valve"=enum16{"A", "B", "C", "D", "ALL"}."C", "action"=T21."MOVE VALVE") -> ()  [unwired: 8 in, 1 out]
      }
      event "Shunt:": Value Change {
        n901 = event-data() -> ()  [unwired: 7 out]
        n902 = call "hamilton_controller.vi"("Open?"="Shunt:", "valve"=enum16{"A", "B", "C", "D", "ALL"}."D", "action"=T21."MOVE VALVE") -> ()  [unwired: 8 in, 1 out]
      }
      event "Flip Green Filter": Value Change {
        n903 = event-data() -> ()  [unwired: 7 out]
        n904 = local write "Flip Green Filter"("Flip Green Filter") -> ()
        n905 = flat-sequence {
          tunnel: w1405 -> [w1410]
          tunnel: w1404 -> [w1409]
          tunnel: [w1407] -> w1402
          tunnel: [w1406] -> w1401
          tunnel: [w1412] -> w1400
          tunnel: w1402 -> [w1412]
          tunnel: [w1411] -> w1399
          tunnel: w1401 -> [w1411]
          tunnel: w1400 -> [w1416]
          tunnel: w1399 -> [w1415]
          tunnel: [w1414] -> w1403
          frame #0 {
            n906 = xnode "Read/Write Control"("FPGA VI Reference In"=w1410, "error in"=w1409, "Green Filter Flipper"=TRUE) -> ("FPGA VI Reference Out"=w1407:T20, "error out"=w1406:errorcluster)
          }
          frame #1 {
            n907 = Wait (ms)(milliseconds to wait=u32 100) -> ()  [unwired: 1 out]
          }
          frame #2 {
            n908 = xnode "Read/Write Control"("FPGA VI Reference In"=w1416, "error in"=w1415, "Green Filter Flipper"=FALSE) -> ("error out"=w1414:errorcluster)  [unwired: 1 out]
          }
        }
      }
      event "Reset Trap Pos. FB": Value Change {
        n909 = event-data() -> ()  [unwired: 7 out]
        n910 = xnode "Read/Write Control"("FPGA VI Reference In"=w1420, "error in"=w1419, "Trap Pos. FB Reset"="Reset Trap Pos. FB") -> ()  [unwired: 2 out]
      }
      event "Trap Pos. FB ON": Value Change {
        n911 = event-data() -> ()  [unwired: 7 out]
        n912 = xnode "Read/Write Control"("FPGA VI Reference In"=w1435, "error in"=w1434) -> ("FPGA VI Reference Out"=w1432:T20, "BD1 Frequency Out 1"=w1429:u64)  [unwired: 1 out]
        n913 = To Double Precision Float(number=w1429) -> (double precision float=w1428:dbl)
        n914 = Multiply(x=49125000.0, y=6.0) -> (x*y=w1427:dbl)
        n915 = Multiply(x=w1428, y=w1427) -> (x*y=w1425:dbl)
        n916 = Scale By Power Of 2(n=-48, x=w1425) -> (x*2^n=w1424:dbl)
        n917 = Divide(x=w1424, y=1000000.0) -> (x/y=w1421:dbl)
        n918 = flat-sequence {
          tunnel: [w1438] -> w1433
          tunnel: w1432 -> [w1439]
          tunnel: w1429 -> [w1437]
          tunnel: "Trap Pos. FB ON" -> [w1436]
          tunnel: "Trap Pos. FB ON" -> [w1445]
          tunnel: w1433 -> [w1444]
          tunnel: "Trap Pos. FB ON" -> [w1447]
          tunnel: w1421 -> [w1446]
          frame #0 {
            n919 = case shown="False" w1436 {
              tunnel: w1439 -> [w1442 w1443]
              tunnel: [w1441 w1443] -> w1438
              tunnel: w1437 -> [w1440 _]
              frame False {
                n920 = xnode "Read/Write Control"("FPGA VI Reference In"=w1442, "BD 1 Frequency 1"=w1440) -> ("FPGA VI Reference Out"=w1441:T20)  [unwired: 1 in, 1 out]
              }
              frame True {
              }
            }
          }
          frame #1 {
            n921 = xnode "Read/Write Control"("FPGA VI Reference In"=w1444, "Force feedback"=w1445) -> ()  [unwired: 1 in, 2 out]
          }
          frame #2 {
            n922 = case shown="False" w1447 {
              tunnel: w1446 -> [w1450 _]
              frame False {
                n923 = local read "T2 for asymmetric\n(MHz)"() -> (w1448:dbl)
                n924 = Subtract(x=w1448, y=w1450) -> (x-y=w1449:dbl)
                n925 = property on="Trap Delta (MHz)" class="DigNum (strict)"("Val(Sgnl)"=w1449) -> ()  [unwired: 2 in, 2 out]
              }
              frame True {
              }
            }
          }
        }
      }
      event "Diff. FB.", "Trap Pos. FB Gains", "Trap Pos. FB Mult Factor", "Trap Pos. FB Offset Factor", "Trap Pos FB Negate Action", "Trap Pos FB Monitor\nT1 or T2", "Negate Diff?": Value Change {
        n926 = event-data() -> ()  [unwired: 7 out]
        n927 = xnode "Read/Write Control"("FPGA VI Reference In"=w1461, "error in"=w1460, "Trap pos. FB Range"="Trap Pos. FB Range", "Trap Pos. FB Gains"="Trap Pos. FB Gains", "Trap Pos. FB Mult Factor"="Trap Pos. FB Mult Factor", "Trap Pos. FB Offset Factor"="Trap Pos. FB Offset Factor", "Trap Pos FB Negate Action"="Trap Pos FB Negate Action", "Trap Pos FB Monitor T1 or T2"="Trap Pos FB Monitor\nT1 or T2", "AI1 X Scale"="Trap Pos. AI1 X Pre-scale", "Negate Diff?"="Negate Diff?", "Diff FB Measurement?"="Diff. FB.") -> ()  [unwired: 2 out]
      }
      event "Trap Pos FB SP": Value Change {
        n928 = event-data() -> ()  [unwired: 7 out]
        n929 = xnode "Read/Write Control"("FPGA VI Reference In"=w1464, "error in"=w1463, "Trap Pos. FB SP"="Trap Pos FB SP") -> ()  [unwired: 2 out]
        n930 = disable-structure shown="Disabled" {
          frame Disabled {
            n931 = local read "Trap X AI1 (DMA)"() -> (w1485:T13)
            n932 = local read "Trap X (AI1)"() -> (w1486:T1)
            n933 = local read "Setpoint offset\nCorrection values"() -> (w1479:dbl[])
            n934 = local read "Trap Delta (MHz)"() -> (w1483:dbl)
            n935 = local read "B factor"() -> (w1470:dbl)
            n936 = Unbundle(w1486) -> ("Trap 1"=w1484:fxp<+/-,16,1>, "Trap 2"=w1473:fxp<+/-,16,1>)
            n937 = Unbundle(w1485) -> ("Set 1"=w1469:fxp<+/-,16,1>, "Set 2"=w1468:fxp<+/-,16,1>)
            n938 = Negate(x=w1473) -> (-x=w1466:fxp<+/-,17,2>)
            n939 = Negate(x=w1484) -> (-x=w1467:fxp<+/-,17,2>)
            n940 = Divide(x=w1483, y=0.1) -> (x/y=w1481:dbl)
            n941 = Multiply(x=w1468, y=w1470) -> (x*y=w1471:dbl)
            n942 = Subtract(x=w1469, y=w1471) -> (x-y=w1476:dbl)
            n943 = To Long Integer(number=w1481) -> (32bit integer=w1480:i32)
            n944 = Index Array(array=w1479, index=w1480) -> (element=w1475:dbl)
            n945 = Multiply(x=w1470, y=w1466) -> (x*y=w1472:dbl)
            n946 = Subtract(x=w1467, y=w1472) -> (x-y=w1478:dbl)
            n947 = Add(x=w1478, y=w1475) -> (x+y=→"ideal setpoint fpga":dbl)
            n948 = Add(x=w1476, y=w1475) -> (x+y=→"ideal setpoint avgd":dbl)
          }
          frame Enabled {
          }
        }
        n949 = disable-structure shown="Enabled" {
          frame Enabled {
          }
          frame Disabled {
            n950 = local write "B factor"(1.0 ("B factor")) -> ()
          }
        }
      }
      event "Simulate stepping": Value Change {
        n951 = event-data() -> ()  [unwired: 7 out]
        n952 = flat-sequence {
          tunnel: w1488 -> [w1491]
          tunnel: [w1490] -> _
          tunnel: w1487 -> [w1489]
          frame #0 {
            n953 = while {
              tunnel: w1491 -> [w1519]
              tunnel: [w1518] -> w1490 mode=indexing
              tunnel: w1489 -> [w1517]
              i -> [w1503]
              stop <- w1500 stop-if-true
              w1493 = 1000.0
              n954 = Divide(x="Backtrack probability", y=100) -> (x/y=w1527:dbl)
              n955 = Random Number (0-1)() -> (number: 0 to 1=w1528:dbl)
              n956 = Greater?(x=w1528, y=w1527) -> (0:w1526:bool)
              n957 = Select(t=1, s=w1526, f=-1) -> (s? t:f=w1523:i32)
              n958 = local read "BD 1 Frq 2 (MHz)"() -> (w1498:dbl)
              n959 = Multiply(x=w1523, y="Step size (nm)") -> (x*y=w1521:dbl)
              "Step taken" <- w1521
              n960 = Divide(x=w1521, y=168.33) -> (x/y=w1496:dbl)
              n961 = local read "X RF Frequency Limits (MHz)"() -> (w1516:T16)
              n962 = local read "BD 1 Frq 1 (MHz)"() -> (w1497:dbl)
              n963 = local read "Y RF Frequency Limits (MHz)"() -> (w1515:T16)
              n964 = Subtract(x=w1497, y=w1496) -> (x-y=w1495:dbl)
              n965 = local write "BD 1 Frq 1 (MHz)"(w1495) -> ()
              n966 = local read "BD 2 Frq 1 (MHz)"() -> (w1513:dbl)
              n967 = local read "BD 2 Frq 2 (MHz)"() -> (w1514:dbl)
              n968 = call "set RF board frequency - interlace.vi"("Board 2 Frequency Limits"=w1515, "Board 1 Frequency Limits"=w1516, "error in"=w1519, "FPGA VI Reference In"=w1517, "Board 2 Frequency 2 (MHz)"=w1514, "Board 2 Frequency 1 (MHz)"=w1513, "Board 1 Frequency 2 (MHz)"=w1498, "Board 1 Frequency 1  (MHz)"=w1495) -> ("error out"=w1518:errorcluster)  [unwired: 2 in, 1 out]
              n969 = Subtract(x=w1498, y=w1495) -> (x-y=w1512:dbl)
              n970 = Subtract(x=w1514, y=w1513) -> (x-y=w1511:dbl)
              n971 = Square(x=w1511) -> (x^2=w1509:dbl)
              n972 = Square(x=w1512) -> (x^2=w1510:dbl)
              n973 = Add(x=w1510, y=w1509) -> (x+y=w1508:dbl)
              n974 = Square Root(x=w1508) -> (sqrt(x)=w1499:dbl)
              n975 = local write "Trap Delta (MHz)"(w1499) -> ()
              n976 = property on="Initial delta (MHz)" class="DigNum (strict)"("Val(Sgnl)"=w1499) -> ()  [unwired: 2 in, 2 out]
              n977 = Multiply(x="Mean dwell time (s)", y=w1493) -> (x*y=w1505:dbl)
              n978 = case shown="\"Gamma2\"" "Distribution" {
                tunnel: w1505 -> [w1532 w1536 w1539]
                tunnel: [w1532 w1533 w1540] -> w1494
                frame "uniform", Default {
                }
                frame "Exponential" {
                  n979 = call-poly <vilib>:"Continuous Random.vi"("b"=w1536, "samples"=1) -> ("exp random data"=w1534:dbl[])  [unwired: 8 in, 1 out]
                  n980 = Index Array(array=w1534) -> (element=w1533:dbl)  [unwired: 1 in]
                }
                frame "Gamma2" {
                  w1537 = 2.0
                  # "Note: the shape and scale\nparameters of the gamma\nare inverted because LabView..."
                  n981 = Divide(x=w1539, y=w1537) -> (x/y=w1538:dbl)
                  n982 = call-poly <vilib>:"Continuous Random.vi"("c"=w1538, "b"=w1537, "samples"=1) -> ("gamma random numbers"=w1541:dbl[])  [unwired: 7 in, 1 out]
                  n983 = Index Array(array=w1541) -> (element=w1540:dbl)  [unwired: 1 in]
                }
              }
              n984 = Divide(x=w1494, y=w1493) -> (x/y=→"Step duration":dbl)
              n985 = To Unsigned Long Integer(number=w1494) -> (unsigned 32bit integer=w1506:u32)
              n986 = Add(x=w1503, y=1) -> (x+y=w1502:i32)
              n987 = Wait (ms)(milliseconds to wait=w1506) -> ()  [unwired: 1 out]
              n988 = Equal?(x=w1502, y="Number of steps") -> (x = y?=w1500:bool)
            }
          }
          frame #1 {
            n989 = local write "Simulate stepping"(FALSE) -> ()
          }
        }
      }
      event "Set SP to Current Frc": Value Change {
        n990 = event-data() -> ()  [unwired: 7 out]
        n991 = local read "Trap Pos FB Monitor\nT1 or T2"() -> (w1551:bool)
        n992 = local read "Trap X AI1 (DMA)"() -> (w1554:T13)
        n993 = local read "Trap X (AI1)"() -> (w1557:T1)
        n994 = Unbundle By Name(w1557) -> ("Trap 1"=w1556:fxp<+/-,16,1>, "Trap 2"=w1555:fxp<+/-,16,1>)
        n995 = Unbundle By Name(w1554) -> ("Set 1"=w1553:fxp<+/-,16,1>, "Set 2"=w1552:fxp<+/-,16,1>)
        n996 = Select(t=w1556, s=w1551, f=w1555) -> (s? t:f=w1550:fxp<+/-,16,1>)
        n997 = Select(t=w1553, s=w1551, f=w1552) -> (s? t:f=w1549:fxp<+/-,16,1>)
        n998 = Not(x="Set SP Using...") -> (.not. x?=w1544:bool)
        n999 = Select(t=w1550, s=w1544, f=w1549) -> (s? t:f=w1545:fxp<+/-,16,1>)
        n1000 = xnode "Read/Write Control"("FPGA VI Reference In"=w1547, "error in"=w1546, "Trap Pos. FB SP"=w1545) -> ()  [unwired: 2 out]
        n1001 = local write "Trap Pos FB SP"(w1545) -> ()
      }
      event "Trap Pos. FB Out Scale 2^n": Value Change {
        n1002 = event-data() -> ()  [unwired: 7 out]
        n1003 = Scale By Power Of 2(n="Trap Pos. FB Out Scale 2^n", x=ext 1.0) -> (x*2^n=w1559:ext)
        n1004 = property on="Trap Pos. FB Mult Factor" class="DigNum (strict)"("Val(Sgnl)"=w1559) -> ()  [unwired: 2 in, 2 out]
      }
      event "Trap Pos FB Int Count": Value Change {
        n1005 = event-data() -> ()  [unwired: 7 out]
        n1006 = xnode "Read/Write Control"("FPGA VI Reference In"=w1564, "error in"=w1563, "Trap Pos FB Int Count"="Trap Pos FB Int Count") -> ()  [unwired: 2 out]
      }
      event "Target Force (pN)", "Setpoint offset\nCorrection values", "Raster target force (pN)": Value Change {
        w1573 = 2.0
        n1007 = event-data() -> ()  [unwired: 7 out]
        n1008 = disable-structure "Removed B Factor to improve position feedback - Alex 081418 1of3" shown="Enabled" {
          disable-tunnel: [w1603 fxp<+/-,32,16> 1.0 ("B factor")] -> w1565
          frame Disabled {
            n1009 = local read "B factor"() -> (w1604:dbl)
            n1010 = To Fixed-Point(number=w1604) -> (fixed-point=w1603:fxp<+/-,16,16>)  [unwired: 1 in]
          }
          frame Enabled {
          }
        }
        n1011 = xnode "Read/Write Control"("FPGA VI Reference In"=w1567, "B factor"=w1565) -> ("BD1 Frequency Out 1"=w1594:u64)  [unwired: 1 in, 2 out]
        n1012 = local read "BD 1 Frq 2 (MHz)"() -> (w1593:dbl)
        n1013 = local read "Target Force (pN)"() -> (w1579:dbl)
        n1014 = To Double Precision Float(number=w1594) -> (double precision float=w1600:dbl)
        n1015 = Multiply(x=49125000.0, y=6.0) -> (x*y=w1599:dbl)
        n1016 = Multiply(x=w1600, y=w1599) -> (x*y=w1597:dbl)
        n1017 = Scale By Power Of 2(n=-48, x=w1597) -> (x*2^n=w1596:dbl)
        n1018 = Divide(x=w1596, y=1000000.0) -> (x/y=w1592:dbl)
        n1019 = Subtract(x=w1593, y=w1592) -> (x-y=w1591:dbl)
        n1020 = local read "T1 kappa_x (pN/nm)"() -> (w1580:dbl)
        n1021 = local read "T1 alpha_x (nm/V)"() -> (w1581:dbl)
        n1022 = local read "Negate offset difference"() -> (w1582:bool)
        n1023 = local read "Offset file step size"() -> (w1590:dbl)
        n1024 = Multiply(x="Raster target force (pN)", y=w1573) -> (x*y=w1572:dbl)
        n1025 = Multiply(x=w1579, y=w1573) -> (x*y=w1578:dbl)
        n1026 = local read "Setpoint offset\nCorrection values"() -> (w1587:dbl[])
        n1027 = Divide(x=w1591, y=w1590) -> (x/y=w1589:dbl)
        n1028 = Select(t=-1, s=w1582, f=1) -> (s? t:f=w1583:i32)
        n1029 = To Long Integer(number=w1589) -> (32bit integer=w1588:i32)
        n1030 = Multiply(x=w1581, y=w1580) -> (x*y=w1571:dbl)
        n1031 = Divide(x=w1578, y=w1571) -> (x/y=w1577:dbl)
        n1032 = Index Array(array=w1587, index=w1588) -> (element=w1586:dbl)
        n1033 = Divide(x=w1572, y=w1571) -> (x/y=w1570:dbl)
        n1034 = Multiply(x=w1583, y=w1586) -> (x*y=w1569:dbl)
        n1035 = Add(x=w1577, y=w1569) -> (x+y=w1576:dbl)
        n1036 = Add(x=w1570, y=w1569) -> (x+y=w1568:dbl)
        n1037 = To Fixed-Point(number=w1568) -> (fixed-point=w1566:fxp<+/-,16,1>)  [unwired: 1 in]
        n1038 = To Fixed-Point(number=w1576) -> (fixed-point=w1575:fxp<+/-,16,1>)  [unwired: 1 in]
        n1039 = property on="Trap Pos FB SP" class="DigNum (strict)"("Val(Sgnl)"=w1575) -> ()  [unwired: 2 in, 2 out]
        n1040 = xnode "Read/Write Control"("FPGA VI Reference In"=w1567, "Raster setpoint"=w1566) -> ()  [unwired: 1 in, 2 out]
      }
      event "Read setpoint correction\nfile": Value Change {
        n1041 = event-data() -> ()  [unwired: 7 out]
        n1042 = local write "Read setpoint correction\nfile"(FALSE) -> ()
        n1043 = Open/Create/Replace File(file path (use dialog)="Setpoint correction\noffset file", operation (0:open)=T27."open", access (0:read/write)=enum16{"read/write", "read-only", "write-only"}."read-only") -> (refnum out=w1631:refnum<file>)  [unwired: 1 in, 4 out]
        n1044 = Deny Access(7:w1631) -> (3:w1629:refnum<file>)  [unwired: 1 in, 2 out]
        n1045 = Read from Binary File(5:0.0, 9:T28."big-endian, network order" ("byte order (0:big-endian, network order)"), 10:-1 ("count (1)"), 11:w1629) -> (2:w1622:dbl[], 3:w1628:refnum<file>)  [unwired: 1 in, 3 out]
        n1046 = Close File(refnum=w1628) -> ()  [unwired: 1 in, 2 out]
        n1047 = Index Array(array=w1622, index=0) -> (element=w1618:dbl)
        n1048 = local write "Offset file step size"(w1618) -> ()
        n1049 = Array Subset(array=w1622, index=3) -> (w1621:dbl[])  [unwired: 1 in]
        n1050 = local read "T1 kappa_x (pN/nm)"() -> (w1616:dbl)
        n1051 = local read "T1 alpha_x (nm/V)"() -> (w1617:dbl)
        n1052 = local read "T2 alpha_x (nm/V)"() -> (w1615:dbl)
        n1053 = local read "T2 kappa_x (pN/nm)"() -> (w1614:dbl)
        n1054 = Decimate 1D Array(w1621) -> (w1610:dbl[], w1611:dbl[])  [unwired: 1 out]
        n1055 = local read "Offset Values"() -> (w1620:T14)
        n1056 = Multiply(x=w1617, y=w1616) -> (x*y=w1612:dbl)
        n1057 = Multiply(x=w1615, y=w1614) -> (x*y=w1613:dbl)
        n1058 = Bundle By Name(cluster=w1620, "Trap 1X offset"=w1610, "Trap 2X offset"=w1611) -> (w1619:T14)
        n1059 = Divide(x=w1613, y=w1612) -> (x/y=w1607:dbl)
        n1060 = disable-structure "Removed B Factor to better position FB - Alex 081418 3of3" shown="Enabled" {
          disable-tunnel: w1607 -> [w1635 _]
          disable-tunnel: [w1635 1.0] -> w1606
          frame Disabled {
          }
          frame Enabled {
          }
        }
        n1061 = Multiply(x=w1611, y=w1606) -> (x*y=w1609:dbl[])
        n1062 = local write "Offset Values"(w1619) -> ()
        n1063 = Subtract(x=w1610, y=w1609) -> (x-y=w1608:dbl[])
        n1064 = property on="B factor" class="DigNum (strict)"("Val(Sgnl)"=w1606) -> ()  [unwired: 2 in, 2 out]
        n1065 = property on="Setpoint offset\nCorrection values" class="Arr (strict)"("Val(Sgnl)"=w1608) -> ()  [unwired: 2 in, 2 out]
      }
      event "MCL Tracking": Value Change {
        n1066 = event-data() -> ()  [unwired: 7 out]
        n1067 = case shown="True" "MCL Tracking" {
          frame False {
            n1068 = local read "Current MCL (V)"() -> (w1638:dbl)
            n1069 = local write "MCL X"(w1638) -> ()
          }
          frame True {
            n1070 = local read "BD 1 Frq 1 (MHz)"() -> (→"Zero T1 position":dbl)
            n1071 = local read "MCL X"() -> (→"Zero MCL x position":dbl)
          }
        }
      }
      event "Scale intensities": Value Change {
        n1072 = event-data() -> ()  [unwired: 7 out]
        n1073 = local read "Trap Intensity\nSetpoints (V)"() -> (w1644:cluster{"Set 1":dbl, "Set 2":dbl})
        n1074 = local read "T1 kappa_x (pN/nm)"() -> (w1650:dbl)
        n1075 = local read "T2 kappa_x (pN/nm)"() -> (w1649:dbl)
        n1076 = Unbundle By Name(w1644) -> ("Set 1"=w1646:dbl, "Set 2"=w1645:dbl)
        n1077 = case shown="False" "Scale intensities" {
          tunnel: "Scale factor" -> [w1653 w1662]
          tunnel: w1650 -> [w1661 w1670]
          tunnel: w1649 -> [w1660 w1669]
          tunnel: [w1658 w1668] -> w1648
          tunnel: [w1659 w1667] -> w1647
          tunnel: w1646 -> [w1657 w1666]
          tunnel: w1645 -> [w1656 w1665]
          tunnel: [w1655 w1664] -> w1643
          tunnel: [w1654 w1663] -> w1642
          frame False {
            n1078 = Divide(x=w1657, y=w1653) -> (x/y=w1655:dbl)
            n1079 = Divide(x=w1656, y=w1653) -> (x/y=w1654:dbl)
            n1080 = Divide(x=w1661, y=w1653) -> (x/y=w1658:dbl)
            n1081 = Divide(x=w1660, y=w1653) -> (x/y=w1659:dbl)
          }
          frame True {
            n1082 = Multiply(x=w1666, y=w1662) -> (x*y=w1664:dbl)
            n1083 = Multiply(x=w1665, y=w1662) -> (x*y=w1663:dbl)
            n1084 = Multiply(x=w1670, y=w1662) -> (x*y=w1668:dbl)
            n1085 = Multiply(x=w1662, y=w1669) -> (x*y=w1667:dbl)
          }
        }
        n1086 = Bundle By Name(cluster=w1644, "Set 1"=w1643, "Set 2"=w1642) -> (w1641:cluster{"Set 1":dbl, "Set 2":dbl})
        n1087 = local write "T1 kappa_x (pN/nm)"(w1648) -> ()
        n1088 = local write "T2 kappa_x (pN/nm)"(w1647) -> ()
        n1089 = property on="Trap Intensity\nSetpoints (V)" class="Clust (strict)"("Val(Sgnl)"=w1641) -> ()  [unwired: 2 in, 2 out]
      }
    }
    "Error Events" <- w615
    n1090 = node-c288() -> ()  [unwired: 1 in, 1 out]
  }
  n1091 = node-c288() -> (w81:T24)  [unwired: 4 in]
  n1092 = timed-loop "Run Scripts, including: stage motion" {
    timing: w81 -> [_]
    timing-out: [_] -> w80
    tunnel: w45 -> [_]
    stop <- w1672 stop-if-true
    n1093 = node-c288() -> ()  [unwired: 1 in, 1 out]
    n1094 = event shown="[4] \"Step Size (nm)\": Value Change" {
      selector: _ -> [_ _ _ _ _ _ _]
      dyn-events: _ -> [_ _ _ _ _ _ _]
      timeout: 50 -> [_ _ _ _ _ _ _]
      tunnel: ["Move Cap. 1 (DNA Top)" _ "Cal/Data Acq. Spot" "Take Stepping Data" _ "Take Detection Laser\nImage" _] -> _
      tunnel: [_ _ _ _ _ _ w1849] -> w1672
      event "Move Cap. 1 (DNA Top)": Value Change {
        n1095 = event-data() -> ()  [unwired: 1 in, 5 out]
        n1096 = local write "Move Cap. 1 (DNA Top)"(FALSE ("Move Cap. 1 (DNA Right)")) -> ()
        n1097 = flat-sequence {
          tunnel: "Cap 1 Samp Flow ON" -> [w1678]
          frame #0 {
            n1098 = local write "Stage Moving"(FALSE ("Stage Moving")) -> ()
            n1099 = case "stop flow" shown="True" w1678 {
              frame False {
              }
              frame True {
                n1100 = call "hamilton_controller.vi"("Open?"=FALSE, "valve"=enum16{"A", "B", "C", "D", "ALL"}."C", "action"=T21."MOVE VALVE") -> ()  [unwired: 8 in, 1 out]
              }
            }
            n1101 = case shown="True" TRUE {
              tunnel: "Cap 1 T ON" -> [w1687 w1688]
              frame False {
                n1102 = property on="Trap 1 (ON/OFF)" class="Bool (strict)"("Val(Sgnl)"=w1687) -> ()  [unwired: 2 in, 2 out]
              }
              frame True {
                n1103 = property on="Trap 2 (ON/OFF)" class="Bool (strict)"("Val(Sgnl)"=w1688) -> ()  [unwired: 2 in, 2 out]
              }
            }
            n1104 = call <vilib>:"Beep.vi"() -> ()  [unwired: 3 in, 9 out]
            n1105 = case shown="True" "Cap 1 Flow ON" {
              frame False {
              }
              frame True {
                n1106 = property on="Main:" class="Bool (strict)"("Val(Sgnl)"=TRUE ("Value (Signaling)")) -> ()  [unwired: 2 in, 2 out]
              }
            }
          }
        }
      }
      event Timeout {
        n1107 = event-data() -> ()  [unwired: 1 in, 2 out]
      }
      event "Cal/Data Acq. Spot": Value Change {
        # "wait for calibration file\nto be written"
        # "signal save cal true\nthis tells the data \nacquisition loop to\nstart sending the data\nto a calibration file"
        # "separate traps to\nthe desired trap delta"
        # "move stage to data acquisition spot"
        # "CHANGE FISH FOR TETHER BACK\nTO TRUE VALUE HERE."
        n1108 = event-data() -> ()  [unwired: 1 in, 5 out]
        n1109 = flat-sequence {
          tunnel: ["Cal @ (MHz)"] -> w1689
          tunnel: w1689 -> [w1701]
          tunnel: w1689 -> [w1722]
          frame #0 {
            n1110 = property on="Trap Delta (MHz)" class="DigNum (strict)"("Val(Sgnl)"="Cal @ (MHz)") -> ()  [unwired: 2 in, 2 out]
            n1111 = call <vilib>:"Beep.vi"() -> ()  [unwired: 3 in, 9 out]
          }
          frame #1 {
            n1112 = local read "Scale intensities"() -> (w1693:bool)
            n1113 = case shown="True" w1693 {
              frame False {
              }
              frame True {
                n1114 = property on="Scale intensities" class="Bool (strict)"("Val(Sgnl)"=FALSE ("Value (Signaling)")) -> ()  [unwired: 2 in, 2 out]
              }
            }
          }
          frame #2 {
            n1115 = Wait (ms)(milliseconds to wait=u32 500) -> ()  [unwired: 1 out]
          }
          frame #3 {
            n1116 = property on="Save Calibration" class="Bool (strict)"("Val(Sgnl)"=TRUE ("Value (Signaling)")) -> ()  [unwired: 2 in, 2 out]
          }
          frame #4 {
            n1117 = Wait (ms)(milliseconds to wait=u32 4000) -> ()  [unwired: 1 out]
          }
          frame #5 {
            n1118 = while {
              stop <- w1698 stop-if-true
              n1119 = local read "Saving..."() -> (w1699:bool)
              n1120 = Wait (ms)(milliseconds to wait=u32 100) -> ()  [unwired: 1 out]
              n1121 = Not(x=w1699) -> (.not. x?=w1698:bool)
            }
          }
          frame #6 {
            n1122 = case shown="True" "W/ Offset 1" {
              tunnel: w1701 -> [_ w1703]
              frame False {
              }
              frame True {
                n1123 = stacked-sequence {
                  tunnel: w1703 -> [_ _ _ _ _ _ _ w1720]
                  frame #0 {
                    n1124 = Replace Array Subset(array=u32[] [0] ("Index Values"), new element="Offset 1 Set", index=0) -> (w1704:u32[])
                    n1125 = property on="Saved AOD Raster Scan Parameter Sets" class="Arr (strict)"("Index Values"=w1704) -> ()  [unwired: 2 in, 2 out]
                    n1126 = property on="Trap Delta (MHz)" class="DigNum (strict)"("Val(Sgnl)"="Offset 1 Start (MHz)") -> ()  [unwired: 2 in, 2 out]
                  }
                  frame #1 {
                    n1127 = Wait (ms)(milliseconds to wait=u32 200) -> ()  [unwired: 1 out]
                  }
                  frame #2 {
                    n1128 = property on="Load parameters" class="Bool (strict)"("Val(Sgnl)"=TRUE ("Value (Signaling)")) -> ()  [unwired: 2 in, 2 out]
                  }
                  frame #3 {
                    n1129 = Wait (ms)(milliseconds to wait=u32 200) -> ()  [unwired: 1 out]
                  }
                  frame #4 {
                    n1130 = property on="Trap Raster Scan" class="Bool (strict)"("Val(Sgnl)"=TRUE ("Value (Signaling)")) -> ()  [unwired: 2 in, 2 out]
                  }
                  frame #5 {
                    n1131 = Wait (ms)(milliseconds to wait=u32 2000) -> ()  [unwired: 1 out]
                  }
                  frame #6 {
                    n1132 = while {
                      stop <- w1717 stop-if-true
                      n1133 = local read "Raster Scanning..."() -> (w1719:bool)
                      n1134 = local read "Saving..."() -> (w1715:bool)
                      n1135 = Wait (ms)(milliseconds to wait=u32 100) -> ()  [unwired: 1 out]
                      n1136 = Not(x=w1715) -> (.not. x?=w1714:bool)
                      n1137 = Not(x=w1719) -> (.not. x?=w1716:bool)
                      n1138 = And(x=w1716, y=w1714) -> (x .and. y?=w1717:bool)
                    }
                  }
                  frame #7 {
                    n1139 = property on="Trap Delta (MHz)" class="DigNum (strict)"("Val(Sgnl)"=w1720) -> ()  [unwired: 2 in, 2 out]
                  }
                }
              }
            }
          }
          frame #7 {
            n1140 = local read "Save ave N"() -> (w1721:i32)
            n1141 = case shown="True" "W/ Offset 2" {
              tunnel: w1722 -> [_ w1728]
              tunnel: w1721 -> [_ w1727]
              frame False {
                n1142 = Multiply(x="Cal read wait (s)", y=u32 1000 ("milliseconds to wait")) -> (x*y=w1725:u32)
                n1143 = Wait (ms)(milliseconds to wait=w1725) -> ()  [unwired: 1 out]
              }
              frame True {
                n1144 = stacked-sequence {
                  tunnel: w1728 -> [_ _ _ _ _ _ _ _ _ w1749 _ _]
                  tunnel: w1727 -> [_ _ _ _ _ _ _ _ _ w1747 _ _]
                  frame #0 {
                    n1145 = property on="Save ave N" class="DigNum (strict)"("Val(Sgnl)"=1.0 ("Value (Signaling)")) -> ()  [unwired: 2 in, 2 out]
                  }
                  frame #1 {
                    n1146 = Wait (ms)(milliseconds to wait=u32 500) -> ()  [unwired: 1 out]
                  }
                  frame #2 {
                    n1147 = property on="Trap Delta (MHz)" class="DigNum (strict)"("Val(Sgnl)"="Offset 2 Start (MHz)") -> ()  [unwired: 2 in, 2 out]
                    n1148 = Replace Array Subset(array=u32[] [0] ("Index Values"), new element="Offset 2 Set", index=0) -> (w1733:u32[])
                    n1149 = property on="Saved AOD Raster Scan Parameter Sets" class="Arr (strict)"("Index Values"=w1733) -> ()  [unwired: 2 in, 2 out]
                  }
                  frame #3 {
                    n1150 = Wait (ms)(milliseconds to wait=u32 500) -> ()  [unwired: 1 out]
                  }
                  frame #4 {
                    n1151 = property on="Load parameters" class="Bool (strict)"("Val(Sgnl)"=TRUE ("Value (Signaling)")) -> ()  [unwired: 2 in, 2 out]
                  }
                  frame #5 {
                    n1152 = Wait (ms)(milliseconds to wait=u32 500) -> ()  [unwired: 1 out]
                  }
                  frame #6 {
                    n1153 = property on="Trap Raster Scan" class="Bool (strict)"("Val(Sgnl)"=TRUE ("Value (Signaling)")) -> ()  [unwired: 2 in, 2 out]
                  }
                  frame #7 {
                    n1154 = Wait (ms)(milliseconds to wait=u32 2000) -> ()  [unwired: 1 out]
                  }
                  frame #8 {
                    n1155 = while {
                      stop <- w1742 stop-if-true
                      n1156 = local read "Raster Scanning..."() -> (w1745:bool)
                      n1157 = local read "Saving..."() -> (w1743:bool)
                      n1158 = Wait (ms)(milliseconds to wait=u32 100) -> ()  [unwired: 1 out]
                      n1159 = Not(x=w1743) -> (.not. x?=w1741:bool)
                      n1160 = Not(x=w1745) -> (.not. x?=w1744:bool)
                      n1161 = And(x=w1744, y=w1741) -> (x .and. y?=w1742:bool)
                    }
                  }
                  frame #9 {
                    n1162 = property on="Trap Delta (MHz)" class="DigNum (strict)"("Val(Sgnl)"=w1749) -> ()  [unwired: 2 in, 2 out]
                    n1163 = property on="Saved AOD Raster Scan Parameter Sets" class="Arr (strict)"("Index Values"=u32[] [0]) -> ()  [unwired: 2 in, 2 out]
                    n1164 = property on="Save ave N" class="DigNum (strict)"("Val(Sgnl)"=w1747) -> ()  [unwired: 2 in, 2 out]
                  }
                  frame #10 {
                    n1165 = Wait (ms)(milliseconds to wait=u32 500) -> ()  [unwired: 1 out]
                  }
                  frame #11 {
                    n1166 = property on="Load parameters" class="Bool (strict)"("Val(Sgnl)"=TRUE ("Value (Signaling)")) -> ()  [unwired: 2 in, 2 out]
                  }
                }
              }
            }
          }
          frame #8 {
            n1167 = property on="Read Cal" class="Bool (strict)"("Val(Sgnl)"=TRUE ("Value (Signaling)")) -> ()  [unwired: 2 in, 2 out]
          }
          frame #9 {
            n1168 = Wait (ms)(milliseconds to wait=u32 500) -> ()  [unwired: 1 out]
          }
          frame #10 {
            n1169 = property on="Fish for Tether" class="Bool (strict)"("Val(Sgnl)"=FALSE ("Value (Signaling)")) -> ()  [unwired: 2 in, 2 out]
          }
        }
        n1170 = local write "Cal/Data Acq. Spot"(FALSE ("Cal/Data Acq. Spot")) -> ()
      }
      event "Take Stepping Data": Value Change {
        n1171 = event-data() -> ()  [unwired: 1 in, 5 out]
        n1172 = local read "Save ave N"() -> (w1763:i32)
        n1173 = flat-sequence {
          tunnel: w1763 -> [w1765]
          tunnel: [w1765] -> w1758
          tunnel: [w1767] -> w1759
          tunnel: w1758 -> [w1767]
          tunnel: [w1769] -> w1760
          tunnel: w1759 -> [w1769]
          tunnel: [w1772] -> w1761
          tunnel: w1760 -> [w1772]
          tunnel: [w1774] -> w1762
          tunnel: w1761 -> [w1774]
          tunnel: [w1776] -> w1756
          tunnel: w1762 -> [w1776]
          tunnel: w1756 -> [w1779]
          tunnel: [w1779] -> w1755
          tunnel: w1755 -> [w1780]
          tunnel: [w1780] -> w1757
          tunnel: w1757 -> [w1786]
          frame #0 {
            n1174 = property on="Save ave N" class="DigNum (strict)"("Val(Sgnl)"="Save ave factor") -> ()  [unwired: 2 in, 2 out]
          }
          frame #1 {
            n1175 = Wait (ms)(milliseconds to wait=u32 100) -> ()  [unwired: 1 out]
          }
          frame #2 {
            n1176 = local read "Offset 2 Start (MHz)"() -> (w1771:dbl)
            n1177 = property on="Saved AOD Raster Scan Parameter Sets" class="Arr (strict)"("Index Values"=u32[] [2]) -> ()  [unwired: 2 in, 2 out]
            n1178 = property on="Trap Delta (MHz)" class="DigNum (strict)"("Val(Sgnl)"=w1771) -> ()  [unwired: 2 in, 2 out]
          }
          frame #3 {
            n1179 = property on="Load parameters" class="Bool (strict)"("Val(Sgnl)"=TRUE ("Value (Signaling)")) -> ()  [unwired: 2 in, 2 out]
          }
          frame #4 {
            n1180 = Wait (ms)(milliseconds to wait=u32 100) -> ()  [unwired: 1 out]
          }
          frame #5 {
            n1181 = property on="Trap Raster Scan" class="Bool (strict)"("Val(Sgnl)"=TRUE ("Value (Signaling)")) -> ()  [unwired: 2 in, 2 out]
          }
          frame #6 {
            n1182 = Wait (ms)(milliseconds to wait=u32 1000) -> ()  [unwired: 1 out]
          }
          frame #7 {
            n1183 = while {
              stop <- w1783 stop-if-true
              n1184 = local read "Raster Scanning..."() -> (w1785:bool)
              n1185 = local read "Saving..."() -> (w1784:bool)
              n1186 = Not(x=w1784) -> (.not. x?=w1781:bool)
              n1187 = Not(x=w1785) -> (.not. x?=w1782:bool)
              n1188 = And(x=w1782, y=w1781) -> (x .and. y?=w1783:bool)
            }
          }
          frame #8 {
            n1189 = property on="Save ave N" class="DigNum (strict)"("Val(Sgnl)"=w1786) -> ()  [unwired: 2 in, 2 out]
          }
        }
      }
      event "Step Size (nm)": Value Change {
        n1190 = event-data() -> ()  [unwired: 1 in, 5 out]
        n1191 = flat-sequence {
          frame #0 {
            n1192 = property on="Saved AOD Raster Scan Parameter Sets" class="Arr (strict)"("Index Values"=u32[] [1]) -> ()  [unwired: 2 in, 2 out]
          }
          frame #1 {
            n1193 = Multiply(x="N Steps", y="Step Size (nm)") -> (x*y=w1788:dbl)
            n1194 = property on="Scan Speed AOD (nm/s) 2" class="DigNum (strict)"("Value"="Step Size (nm)") -> ()  [unwired: 2 in, 2 out]
            n1195 = property on="Step Size AOD (nm) 2" class="DigNum (strict)"("Value"="Step Size (nm)") -> ()  [unwired: 2 in, 2 out]
            n1196 = property on="Scan Range AOD (nm) 2" class="DigNum (strict)"("Value"=w1788) -> ()  [unwired: 2 in, 2 out]
          }
        }
      }
      event "Take Detection Laser\nImage": Value Change {
        n1197 = event-data() -> ()  [unwired: 1 in, 5 out]
        n1198 = flat-sequence {
          tunnel: [w1816] -> w1806
          tunnel: [w1815] -> w1799
          tunnel: [w1814] -> w1791
          tunnel: [w1819] -> w1807
          tunnel: w1806 -> [w1819]
          tunnel: [w1818] -> w1800
          tunnel: w1799 -> [w1818]
          tunnel: [w1817] -> w1792
          tunnel: w1791 -> [w1817]
          tunnel: [w1823] -> w1808
          tunnel: w1807 -> [w1823]
          tunnel: [w1822] -> w1801
          tunnel: w1800 -> [w1822]
          tunnel: [w1821] -> w1793
          tunnel: w1792 -> [w1821]
          tunnel: [w1829] -> w1809
          tunnel: w1808 -> [w1829]
          tunnel: [w1828] -> w1802
          tunnel: w1801 -> [w1828]
          tunnel: [w1827] -> w1794
          tunnel: w1793 -> [w1827]
          tunnel: [w1833] -> w1810
          tunnel: w1809 -> [w1833]
          tunnel: [w1832] -> w1803
          tunnel: w1802 -> [w1832]
          tunnel: [w1831] -> w1795
          tunnel: w1794 -> [w1831]
          tunnel: [w1837] -> w1811
          tunnel: w1810 -> [w1837]
          tunnel: [w1836] -> w1804
          tunnel: w1803 -> [w1836]
          tunnel: [w1835] -> w1796
          tunnel: w1795 -> [w1835]
          tunnel: [w1841] -> w1812
          tunnel: w1811 -> [w1841]
          tunnel: [w1840] -> w1805
          tunnel: w1804 -> [w1840]
          tunnel: [w1839] -> w1797
          tunnel: w1796 -> [w1839]
          tunnel: w1812 -> [w1847]
          tunnel: w1805 -> [w1846]
          tunnel: [w1844] -> w1798
          tunnel: w1797 -> [w1844]
          tunnel: w1798 -> [w1848]
          frame #0 {
            n1199 = local read "Green Laser ON/Interlacing"() -> (w1816:bool)
            n1200 = local read "Green laser mode"() -> (w1815:enum32{"Laser ON", "Laser OFF", "Interlace"})
            n1201 = local read "Green FB On/Off"() -> (w1814:bool)
          }
          frame #1 {
            n1202 = property on="Green FB On/Off" class="Bool (strict)"("Val(Sgnl)"=FALSE ("Value (Signaling)")) -> ()  [unwired: 2 in, 2 out]
          }
          frame #2 {
            n1203 = property on="Green Laser ON/Interlacing" class="Bool (strict)"("Val(Sgnl)"=TRUE ("Value (Signaling)")) -> ()  [unwired: 2 in, 2 out]
            n1204 = property on="Flip Green Filter" class="Bool (strict)"("Val(Sgnl)"=TRUE ("Value (Signaling)")) -> ()  [unwired: 2 in, 2 out]
            n1205 = property on="Green laser mode" class="RadioBtnsControl (strict)"("Val(Sgnl)"=enum32{"Laser ON", "Laser OFF", "Interlace"}."Laser ON" ("Value (Signaling)")) -> ()  [unwired: 2 in, 2 out]
          }
          frame #3 {
            n1206 = Wait (ms)(milliseconds to wait=u32 500) -> ()  [unwired: 1 out]
          }
          frame #4 {
            n1207 = property on="Confocal Image" class="Bool (strict)"("Val(Sgnl)"=TRUE ("Value (Signaling)")) -> ()  [unwired: 2 in, 2 out]
          }
          frame #5 {
            n1208 = Wait (ms)(milliseconds to wait=u32 2000) -> ()  [unwired: 1 out]
          }
          frame #6 {
            n1209 = while {
              stop <- w1842 stop-if-true
              n1210 = local read "Saving..."() -> (w1843:bool)
              n1211 = Not(x=w1843) -> (.not. x?=w1842:bool)
            }
          }
          frame #7 {
            n1212 = property on="Flip Green Filter" class="Bool (strict)"("Val(Sgnl)"=TRUE ("Value (Signaling)")) -> ()  [unwired: 2 in, 2 out]
            n1213 = property on="Green Laser ON/Interlacing" class="Bool (strict)"("Val(Sgnl)"=w1847) -> ()  [unwired: 2 in, 2 out]
            n1214 = property on="Green laser mode" class="RadioBtnsControl (strict)"("Val(Sgnl)"=w1846) -> ()  [unwired: 2 in, 2 out]
          }
          frame #8 {
            n1215 = property on="Green FB On/Off" class="Bool (strict)"("Val(Sgnl)"=w1848) -> ()  [unwired: 2 in, 2 out]
          }
        }
      }
      event "Stop All": Value Change {
        n1216 = event-data() -> ()  [unwired: 1 in, 5 out]
        n1217 = local read "Stop All"() -> (w1849:bool)
      }
    }
    n1218 = node-c288() -> ()  [unwired: 1 in, 1 out]
  }
  n1219 = node-c288() -> (w88:T24)  [unwired: 4 out]
  n1220 = timed-loop "Mouse control: trap position (AOM deflection), set confocal spot from image" {
    tunnel: [w1851] -> w49
    tunnel: w45 -> [w1850]
    timing: w88 -> [_]
    timing-out: [_] -> w87
    stop <- w1851 stop-if-true
    n1221 = node-c288() -> ()  [unwired: 2 out]
    n1222 = event shown="[0] \"Pane\": Mouse Down" {
      selector: _ -> [_ _]
      dyn-events: _ -> [_ _]
      timeout: _ -> [_ _]
      tunnel: w1850 -> [w1854 _]
      event Mouse Down {
        n1223 = event-data() -> ("Time"=w1856:u32, "Coords"=w1855:T8, "Button"=w1857:u16)  [unwired: 6 out]
        n1224 = case shown="1" w1857 {
          tunnel: w1856 -> [_ _ w1960]
          tunnel: w1855 -> [_ w1894 w1958]
          tunnel: w1854 -> [_ _ w1956]
          frame 0, Default {
          }
          frame 1 {
            n1225 = property on="APD 2" class="ImageControl"() -> ("Displayed Image Position"=w1864:cluster{"Left":i32, "Top":i32})  [unwired: 2 in, 2 out]
            n1226 = property on="APD 1" class="ImageControl"() -> ("Displayed Image Position"=w1893:cluster{"Left":i32, "Top":i32})  [unwired: 2 in, 2 out]
            n1227 = property on="Detection Laser X" class="ImageControl"() -> ("Displayed Image Position"=w1890:cluster{"Left":i32, "Top":i32})  [unwired: 2 in, 2 out]
            n1228 = property on="Detection Laser Y" class="ImageControl"() -> ("Displayed Image Position"=w1889:cluster{"Left":i32, "Top":i32})  [unwired: 2 in, 2 out]
            n1229 = property on="APD 2" class="ImageControl"() -> ("Displayed Image Size"=w1863:cluster{"Width":u32, "Height":u32})  [unwired: 2 in, 2 out]
            n1230 = property on="APD 1" class="ImageControl"() -> ("Displayed Image Size"=w1891:cluster{"Width":u32, "Height":u32})  [unwired: 2 in, 2 out]
            n1231 = property on="Detection Laser X" class="ImageControl"() -> ("Displayed Image Size"=w1892:cluster{"Width":u32, "Height":u32})  [unwired: 2 in, 2 out]
            n1232 = property on="Detection Laser Y" class="ImageControl"() -> ("Displayed Image Size"=w1888:cluster{"Width":u32, "Height":u32})  [unwired: 2 in, 2 out]
            n1233 = Unbundle By Name(w1863) -> ("Width"=w1860:u32, "Height"=w1859:u32)
            n1234 = Unbundle By Name(w1864) -> ("Left"=w1862:i32, "Top"=w1861:i32)
            n1235 = Unbundle By Name(w1891) -> ("Width"=w1885:u32, "Height"=w1884:u32)
            n1236 = Unbundle By Name(w1892) -> ("Width"=w1881:u32, "Height"=w1880:u32)
            n1237 = Unbundle By Name(w1888) -> ("Width"=w1877:u32, "Height"=w1876:u32)
            n1238 = Unbundle By Name(w1893) -> ("Left"=w1887:i32, "Top"=w1886:i32)
            n1239 = Unbundle By Name(w1890) -> ("Left"=w1883:i32, "Top"=w1882:i32)
            n1240 = Unbundle By Name(w1889) -> ("Left"=w1879:i32, "Top"=w1878:i32)
            n1241 = Bundle("Left"=w1862, "Top"=w1861, "Width"=w1860, "Height"=w1859) -> (w1858:T32)  [unwired: 1 in]
            n1242 = Bundle("Left"=w1887, "Top"=w1886, "Width"=w1885, "Height"=w1884) -> (w1875:T32)  [unwired: 1 in]
            n1243 = Bundle("Left"=w1883, "Top"=w1882, "Width"=w1881, "Height"=w1880) -> (w1874:T32)  [unwired: 1 in]
            n1244 = Bundle("Left"=w1879, "Top"=w1878, "Width"=w1877, "Height"=w1876) -> (w1873:T32)  [unwired: 1 in]
            n1245 = Build Cluster Array(w1858, w1875, w1874, w1873) -> (w1872:T33)
            n1246 = for {
              tunnel: w1894 -> [w1905]
              tunnel: w1872 -> [w1906] mode=indexing
              shift-right: [w1903] -> w1870
              shift-left: TRUE -> [w1904]
              shift-right: [w1902] -> w1868
              shift-left: _ -> [w1898]
              shift-right: [w1901] -> w1867
              shift-left: _ -> [w1897]
              shift-right: [w1900] -> w1866
              shift-left: _ -> [w1896]
              shift-right: [w1899] -> w1865
              shift-left: _ -> [w1895]
              n1247 = case shown="True" w1904 {
                selector: w1904 -> [w1911 _]
                tunnel: w1906 -> [_ w1920]
                tunnel: w1905 -> [_ w1918]
                tunnel: [w1911 w1916] -> w1903
                tunnel: [w1910 w1915] -> w1902
                tunnel: [w1909 w1914] -> w1901
                tunnel: [w1908 w1913] -> w1900
                tunnel: [w1907 w1912] -> w1899
                tunnel: w1898 -> [w1910 _]
                tunnel: w1897 -> [w1909 _]
                tunnel: w1896 -> [w1908 _]
                tunnel: w1895 -> [w1907 _]
                frame False {
                }
                frame True {
                  n1248 = Unbundle(w1920) -> (w1919:T32)
                  n1249 = call "isclickinwindow.vi"("Image Param"=w1919, "Point32"=w1918) -> ("Y px"=w1912:i32, "Height"=w1913:i32, "X px"=w1914:i32, "Width"=w1915:i32, "In image?"=w1917:bool)  [unwired: 1 in]
                  n1250 = Not(x=w1917) -> (.not. x?=w1916:bool)
                }
              }
            }
            n1251 = Not(x=w1870) -> (.not. x?=w1869:bool)
            n1252 = case shown="True" w1869 {
              tunnel: w1867 -> [_ w1933]
              tunnel: w1865 -> [_ w1932]
              tunnel: w1868 -> [_ w1931]
              tunnel: w1866 -> [_ w1930]
              frame False {
              }
              frame True {
                w1926 = FALSE ("Get Point")
                n1253 = local read "Scan lines (y)"() -> (w1935:u64)
                n1254 = local read "Actual MCL Inc (V)"() -> (w1927:dbl)
                n1255 = local read "Scan steps (x)"() -> (w1934:u64)
                n1256 = Divide "Y Pix/step"(x=w1930, y=w1935) -> (x/y=w1942:dbl)
                n1257 = Divide "Y V/pix"(x=w1927, y=w1942) -> (x/y=w1941:dbl)
                n1258 = Divide "Y half step offset"(x=w1927, y=2.0) -> (x/y=w1943:dbl)
                n1259 = Divide "X pix/step"(x=w1931, y=w1934) -> (x/y=w1940:dbl)
                n1260 = Negate(x=w1943) -> (-x=w1944:dbl)
                n1261 = local read "Initial Y"() -> (w1950:dbl)
                n1262 = Multiply(x=w1932, y=w1941) -> (x*y=w1951:dbl)
                n1263 = Divide "X half step offset"(x=w1927, y=2.0) -> (x/y=w1937:dbl)
                n1264 = Divide "X V/pix"(x=w1927, y=w1940) -> (x/y=w1939:dbl)
                n1265 = Multiply(x=w1927, y=w1934) -> (x*y=w1946:dbl)
                n1266 = Compound Arithmetic op=ADD(w1944, w1951, w1950) -> (w1928:dbl)
                "Pointer Y (V)" <- w1928
                n1267 = Multiply(x=w1939, y=w1933) -> (x*y=w1948:dbl)
                n1268 = Negate(x=w1937) -> (-x=w1936:dbl)
                n1269 = local read "Initial X"() -> (w1949:dbl)
                n1270 = Negate(x=w1948) -> (-x=w1947:dbl)
                n1271 = Compound Arithmetic op=ADD(w1936, w1946, w1949, w1947) -> (w1929:dbl)
                "Pointer X (V)" <- w1929
                n1272 = Or(x="Set X Only", y="Set Confocal Spot (X-Y)") -> (x .or. y?=w1922:bool)
                n1273 = Or(x="Set Confocal Spot (X-Y)", y="Set Y Only") -> (x .or. y?=w1921:bool)
                n1274 = case shown="True" w1922 {
                  tunnel: w1929 -> [_ w1952]
                  frame False {
                  }
                  frame True {
                    n1275 = property on="MCL X" class="Slide (strict)"("Val(Sgnl)"=w1952) -> ()  [unwired: 2 in, 2 out]
                  }
                }
                n1276 = case shown="True" w1921 {
                  tunnel: w1928 -> [_ w1953]
                  frame False {
                  }
                  frame True {
                    n1277 = property on="MCL Y" class="Slide (strict)"("Val(Sgnl)"=w1953) -> ()  [unwired: 2 in, 2 out]
                  }
                }
                n1278 = local write "Set Confocal Spot (X-Y)"(w1926) -> ()
                n1279 = local write "Set X Only"(w1926) -> ()
                n1280 = local write "Set Y Only"(w1926) -> ()
              }
            }
          }
          frame 3 {
            n1281 = local read "BD 2 Frq 1 (MHz)"() -> (w1954:dbl)
            n1282 = local read "BD 1 Frq 1 (MHz)"() -> (w1955:dbl)
            n1283 = local write "Manipulating Trap"(TRUE ("Manipulating Trap")) -> ()
            n1284 = local write "Coords"(T8 {"Horizontal"=0, "Vertical"=0} ("Coords")) -> ()
            n1285 = while {
              tunnel: w1960 -> [w1965]
              tunnel: w1958 -> [w1964]
              tunnel: w1956 -> [w1963]
              tunnel: w1955 -> [w1962]
              tunnel: w1954 -> [w1961]
              stop <- w1966 stop-if-true
              n1286 = event shown="[0] \"Pane\": Mouse Move" {
                selector: _ -> [_ _]
                dyn-events: _ -> [_ _]
                timeout: _ -> [_ _]
                tunnel: ["Force Manip Abort" w2030] -> w1966
                tunnel: w1965 -> [w1973 _]
                tunnel: w1964 -> [w1971 _]
                tunnel: w1963 -> [w1970 _]
                tunnel: w1962 -> [w1969 _]
                tunnel: w1961 -> [w1968 _]
                event Mouse Move {
                  n1287 = event-data() -> ("Time"=w1974:u32, "Coords"=w1975:T8)  [unwired: 3 out]
                  n1288 = Less?(x=w1974, y=w1973) -> (x < y?=w1972:bool)
                  n1289 = case "Makes sure old motion events prior to mouse click aren't used" shown="False" w1972 {
                    tunnel: w1975 -> [w2017 _]
                    tunnel: w1971 -> [w2018 _]
                    tunnel: w1970 -> [w1995 _]
                    tunnel: w1969 -> [w1991 _]
                    tunnel: w1968 -> [w1990 _]
                    frame False {
                      n1290 = Subtract(x=w2017, y=w2018) -> (x-y=w2016:T8)
                      "Coords" <- w2016
                      n1291 = local read "Y RF Frequency Limits (MHz)"() -> (w1976:T16)
                      n1292 = To Double Precision Float(number=w2016) -> (double precision float=w2015:cluster{"Horizontal":dbl, "Vertical":dbl})
                      n1293 = Multiply(x=cluster{"Horizontal":dbl, "Vertical":dbl} {"Horizontal"=-1.0, "Vertical"=1.0}, y="Manipulation Scaling") -> (x*y=w2011:cluster{"Horizontal":dbl, "Vertical":dbl})
                      n1294 = local read "X RF Frequency Limits (MHz)"() -> (w1977:T16)
                      n1295 = Multiply(x=w2015, y=w2011) -> (x*y=w2013:cluster{"Horizontal":dbl, "Vertical":dbl})
                      n1296 = Unbundle By Name(w2013) -> ("Horizontal"=w2008:dbl, "Vertical"=w2012:dbl)
                      n1297 = Unbundle By Name(w1976) -> ("Maximum"=w1979:dbl, "Minimum"=w1978:dbl)
                      n1298 = Boolean To (0,1)(Boolean="Manip. X?") -> (0, 1=w2006:i16)
                      n1299 = Boolean To (0,1)(Boolean="Manip. Y?") -> (0, 1=w2003:i16)
                      n1300 = Multiply(x=w2012, y=w2003) -> (x*y=w2005:dbl)
                      n1301 = Multiply(x=w2006, y=w2008) -> (x*y=w2009:dbl)
                      n1302 = local read "BD 1 Frq 2 (MHz)"() -> (w1993:dbl)
                      n1303 = Unbundle By Name(w1977) -> ("Maximum"=w1981:dbl, "Minimum"=w1980:dbl)
                      n1304 = local read "BD 2 Frq 2 (MHz)"() -> (w1992:dbl)
                      n1305 = Add(x=w1990, y=w2005) -> (x+y=w1983:dbl)
                      n1306 = Add(x=w1991, y=w2009) -> (x+y=w1985:dbl)
                      n1307 = In Range and Coerce(upper limit=w1981, x=w1985, lower limit=w1980) -> (coerced(x)=w1984:dbl)  [unwired: 1 out]
                      n1308 = In Range and Coerce(upper limit=w1979, x=w1983, lower limit=w1978) -> (coerced(x)=w1982:dbl)  [unwired: 1 out]
                      n1309 = Subtract(x=w1984, y=w1993) -> (x-y=w2002:dbl)
                      n1310 = Subtract(x=w1982, y=w1992) -> (x-y=w2001:dbl)
                      n1311 = Square(x=w2002) -> (x^2=w2000:dbl)
                      n1312 = Square(x=w2001) -> (x^2=w1999:dbl)
                      n1313 = Add(x=w2000, y=w1999) -> (x+y=w1998:dbl)
                      n1314 = Square Root(x=w1998) -> (sqrt(x)=w1994:dbl)
                      n1315 = In Range and Coerce(upper limit="Limit Max (MHz)", x=w1994, lower limit="Limit Min (MHz)") -> (In Range?=w1987:bool)  [unwired: 1 out]
                      n1316 = Not(x="Limits Enable") -> (.not. x?=w1986:bool)
                      n1317 = Or(x=w1987, y=w1986) -> (x .or. y?=w1988:bool)
                      n1318 = case shown="True" w1988 {
                        tunnel: w1995 -> [_ w2028]
                        tunnel: w1994 -> [_ w2019]
                        tunnel: w1984 -> [_ w2026]
                        tunnel: w1993 -> [_ w2025]
                        tunnel: w1982 -> [_ w2024]
                        tunnel: w1992 -> [_ w2023]
                        tunnel: w1977 -> [_ w2021]
                        tunnel: w1976 -> [_ w2020]
                        frame False {
                        }
                        frame True {
                          n1319 = local write "Trap Delta (MHz)"(w2019) -> ()
                          n1320 = local read "BD 1 Frq 3 (MHz)"() -> (w2027:dbl)
                          n1321 = property on="Initial delta (MHz)" class="DigNum (strict)"("Val(Sgnl)"=w2019) -> ()  [unwired: 2 in, 2 out]
                          n1322 = local read "BD 2 Frq 3 (MHz)"() -> (w2022:dbl)
                          n1323 = call "set RF board frequency - interlace.vi"("Board 2 Frequency Limits"=w2020, "Board 1 Frequency Limits"=w2021, "FPGA VI Reference In"=w2028, "Board 2 Frequency 3 (MHz)"=w2022, "Board 1 Frequency 3 (MHz)"=w2027, "Board 2 Frequency 2 (MHz)"=w2023, "Board 2 Frequency 1 (MHz)"=w2024, "Board 1 Frequency 2 (MHz)"=w2025, "Board 1 Frequency 1  (MHz)"=w2026) -> ()  [unwired: 1 in, 2 out]
                          n1324 = local write "BD 2 Frq 1 (MHz)"(w2024) -> ()
                          n1325 = local write "BD 1 Frq 1 (MHz)"(w2026) -> ()
                        }
                      }
                    }
                    frame True {
                    }
                  }
                }
                event Mouse Up {
                  n1326 = event-data() -> ("Button"=w2029:u16)  [unwired: 8 out]
                  n1327 = case shown="3" w2029 {
                    tunnel: [FALSE TRUE] -> w2030
                    frame 0, Default {
                    }
                    frame 3 {
                      n1328 = local write "Manipulating Trap"(FALSE ("Manipulating Trap")) -> ()
                    }
                  }
                }
              }
            }
          }
        }
      }
      event Mouse Move {
        n1329 = event-data() -> ()  [unwired: 6 out]
      }
    }
    n1330 = local read "Stop All"() -> (w1851:bool)
    n1331 = node-c288() -> ()  [unwired: 2 out]
  }
  n1332 = node-c288(w37) -> ()  [unwired: 1 out]
  n1333 = node-c288(w80) -> ()  [unwired: 1 out]
  n1334 = node-c288(w87) -> ()  [unwired: 1 out]
  n1335 = node-c288(i64 1 ("Period"), 1 ("Processor")) -> (w169:T24)  [unwired: 2 out]
  n1336 = timed-loop "Acquire Data" {
    tunnel: w45 -> [w2276]
    tunnel: w55 -> [w2275]
    tunnel: [w2298] -> w48
    tunnel: [w2292] -> w7
    timing: w169 -> [_]
    timing-out: [_] -> w168
    tunnel: w72 -> [w2195]
    stop <- "Stop All" stop-if-true
    n1337 = node-c288() -> ()  [unwired: 2 out]
    n1338 = First Call?() -> (First Call?: T/F=w2179:bool)
    n1339 = Or(x="Reset", y=w2179) -> (x .or. y?=w2180:bool)
    n1340 = case "Reset FIFOs if asked" shown="True" w2180 {
      tunnel: w2276 -> [w2461 w2469]
      tunnel: w2275 -> [w2460 w2468]
      tunnel: [w2461 w2463] -> w2142
      tunnel: [w2460 w2462] -> w2271
      frame False {
      }
      frame True {
        w2466 = TRUE ("AI to FIFO")
        n1341 = call "reset FPGA DMA.vi"("error in"=w2468, "FPGA VI Reference In"=w2469) -> ("error out"=w2464:errorcluster, "FPGA VI Reference Out"=w2465:T20)
        n1342 = local write "Overflow (data lost)"(FALSE ("Overflow (data lost)")) -> ()
        n1343 = xnode "Read/Write Control"("FPGA VI Reference In"=w2465, "error in"=w2464, "AI to FIFO"=w2466, "APD to FIFO"=w2466) -> ("FPGA VI Reference Out"=w2463:T20, "error out"=w2462:errorcluster)
      }
    }
    n1344 = Or(x="Start AOD Scan", y="Trap Raster Scan") -> (x .or. y?=w2241:bool)
    n1345 = And(x="Save scans", y=w2241) -> (x .and. y?=w2269:bool)
    n1346 = case "Start AOM raster scan" shown="True" w2241 {
      tunnel: w2142 -> [w2634 w2645]
      tunnel: w2271 -> [w2633 w2644]
      tunnel: [w2634 w2638] -> w2141
      tunnel: [w2633 w2637] -> w2270
      frame False {
      }
      frame True {
        n1347 = case shown="True" "Restart DMA? (AOD)" {
          tunnel: [w2685 w2687] -> w2639
          tunnel: [w2684 w2686] -> w2640
          tunnel: w2645 -> [w2685 w2689]
          tunnel: w2644 -> [w2684 w2688]
          frame False {
          }
          frame True {
            n1348 = call "reset FPGA DMA.vi"("error in"=w2688, "FPGA VI Reference In"=w2689) -> ("error out"=w2686:errorcluster, "FPGA VI Reference Out"=w2687:T20)
            n1349 = local write "Overflow (data lost)"(FALSE ("Overflow (data lost)")) -> ()
          }
        }
        n1350 = local write "Trap Raster Scan"(FALSE ("Trap Raster Scan")) -> ()
        n1351 = case shown="True" "Move MCL Also?" {
          tunnel: w2640 -> [w2649 w2679]
          tunnel: w2639 -> [w2650 w2680]
          tunnel: [w2648 w2683] -> w2638
          tunnel: [w2647 w2682] -> w2637
          tunnel: "Raster to target force?" -> [w2646 w2652]
          frame False {
            w2651 = TRUE ("AI to FIFO")
            n1352 = xnode "Read/Write Control"("FPGA VI Reference In"=w2650, "error in"=w2649, "AI to FIFO"=w2651, "APD to FIFO"=w2651, "Start scan"=w2651, "Raster to target force"=w2646) -> ("FPGA VI Reference Out"=w2648:T20, "error out"=w2647:errorcluster)
          }
          frame True {
            w2676 = FALSE ("1D or 2D Scan?")
            w2681 = TRUE ("AI to FIFO")
            # "Count for MCL loop"
            # "N total cycles"
            # "N steps"
            # "V_int"
            n1353 = local read "Scan Range (nm)"() -> (w2658:dbl)
            n1354 = local read "Number of F/B Scans (AOD)"() -> (w2675:u16)
            n1355 = Sign(1:w2658) -> (0:w2657:dbl)
            n1356 = Compound Arithmetic op=MULTIPLY(w2658, "MCL Step Position Ratio", "MCL/AOM Scale Tweak") -> (w2662:dbl)
            n1357 = Negate(x=w2657) -> (-x=w2654:dbl)
            n1358 = Multiply(x=w2654, y="MCL Step Increment (V_int)") -> (x*y=w2656:dbl)
            n1359 = Divide(x=w2662, y="MCL X Cal (nm/V)") -> (x/y=w2668:dbl)
            n1360 = Multiply(x=32767.0 ("y"), y=w2668) -> (x*y=w2674:dbl)
            n1361 = local read "Total Counts (ticks)"() -> (w2659:u32)
            n1362 = local read "Cycles/step (AOD)"() -> (w2670:u64)
            n1363 = local read "Scan steps (AOD)"() -> (w2671:u64)
            n1364 = Divide(x=w2674, y=10.0) -> (x/y=w2667:dbl)
            n1365 = Divide(x=w2667, y="MCL Step Increment (V_int)") -> (x/y=w2665:dbl)
            n1366 = Absolute Value(x=w2665) -> (abs(x)=w2653:dbl)
            n1367 = Compound Arithmetic op=MULTIPLY(w2671, w2670, w2659) -> (w2666:u64)
            n1368 = local write "wait to reset values"(w2681) -> ()
            n1369 = local write "MCL Scanning"(w2681) -> ()
            n1370 = Divide(x=w2666, y=w2653) -> (x/y=w2663:dbl)
            "MCL Count" <- w2663
            n1371 = xnode "Read/Write Control"("FPGA VI Reference In"=w2680, "error in"=w2679, "Scan steps (MCL)"=w2653, "Number of scans (MCL)"=w2675, "Cycles per step (MCL)"=u64 1, "Scan freq.  increment (MCL)"=w2656, "1D or 2D Scan?"=w2676, "MCL Scan Axis"=w2676, "Cont. Scan (MCL)"=w2676, "MCL count"=w2663) -> ("FPGA VI Reference Out"=w2678:T20, "error out"=w2677:errorcluster)
            n1372 = xnode "Read/Write Control"("FPGA VI Reference In"=w2678, "error in"=w2677, "AI to FIFO"=w2681, "APD to FIFO"=w2681, "Start scan"=w2681, "Start scan (MCL)"=w2681, "Raster to target force"=w2652) -> ("FPGA VI Reference Out"=w2683:T20, "error out"=w2682:errorcluster)
          }
        }
        "Raster Scanning..." <- TRUE ("Scanning...")
      }
    }
    n1373 = Compound Arithmetic op=OR("Start MCL Scan", "Confocal Image", "Confocal Linescan") -> (w2239:bool)
    n1374 = And(x="Save Data (MCL)", y=w2239) -> (x .and. y?=w2268:bool)
    n1375 = case "Start MCL raster scan" shown="True" w2239 {
      tunnel: w2141 -> [w2548 w2562]
      tunnel: w2270 -> [w2547 w2561]
      tunnel: [w2548 w2557] -> w2093
      tunnel: [w2547 w2556] -> w2095
      tunnel: [FALSE w2555] -> w2254
      tunnel: "Start MCL Scan" -> [_ w2550]
      tunnel: "Confocal Image" -> [_ w2549]
      frame False {
      }
      frame True {
        w2555 = TRUE
        n1376 = case shown="True" "Restart DMA? (MCL)" {
          tunnel: [w2606 w2608] -> w2560
          tunnel: [w2605 w2607] -> w2559
          tunnel: w2562 -> [w2606 w2611]
          tunnel: w2561 -> [w2605 w2610]
          frame False {
          }
          frame True {
            n1377 = call "reset FPGA DMA.vi"("error in"=w2610, "FPGA VI Reference In"=w2611) -> ("error out"=w2607:errorcluster, "FPGA VI Reference Out"=w2608:T20)
            n1378 = local write "Overflow (data lost)"(FALSE ("Overflow (data lost)")) -> ()
          }
        }
        n1379 = case shown="False" w2550 {
          tunnel: w2549 -> [w2565 _]
          frame False {
            n1380 = property on="Confocal Image" class="Bool (strict)"("Value"=FALSE ("Start Confocal Map")) -> ()  [unwired: 2 in, 2 out]
            n1381 = property on="2D or 1D Scan" class="Bool (strict)"("Val(Sgnl)"=w2565) -> ()  [unwired: 2 in, 2 out]
          }
          frame True {
          }
        }
        n1382 = local write "MCL Scanning"(w2555) -> ()
        n1383 = local read "MCL X"() -> (w2551:dbl)
        n1384 = local read "MCL Y"() -> (w2552:dbl)
        n1385 = case shown="True" "Center Scan" {
          tunnel: w2560 -> [w2572 w2604]
          tunnel: w2559 -> [w2571 w2603]
          tunnel: [w2570 w2602] -> w2557
          tunnel: [w2569 w2601] -> w2556
          tunnel: [w2567 w2576] -> w2554
          tunnel: [w2566 w2573] -> w2553
          tunnel: w2552 -> [w2567 w2593]
          tunnel: w2551 -> [w2566 w2596]
          frame False {
            w2568 = TRUE ("AI to FIFO")
            n1386 = xnode "Read/Write Control"("FPGA VI Reference In"=w2572, "error in"=w2571, "AI to FIFO"=w2568, "APD to FIFO"=w2568, "Start scan (MCL)"=w2568) -> ("FPGA VI Reference Out"=w2570:T20, "error out"=w2569:errorcluster)
          }
          frame True {
            w2600 = TRUE ("AI to FIFO")
            n1387 = local read "Scan steps (x)"() -> (w2583:u64)
            n1388 = local read "Fast Scan Dir"() -> (w2590:bool)
            n1389 = local read "Scan lines (y)"() -> (w2579:u64)
            n1390 = local read "Actual MCL Inc (V)"() -> (w2580:dbl)
            n1391 = Decrement(x=w2579) -> (x-1=w2578:u64)
            n1392 = Decrement(x=w2583) -> (x-1=w2582:u64)
            n1393 = Multiply(x=w2580, y=w2578) -> (x*y=w2577:dbl)
            n1394 = Divide(x=w2577, y=2.0) -> (x/y=w2587:dbl)
            n1395 = local read "2D or 1D Scan"() -> (w2598:bool)
            n1396 = Multiply(x=w2580, y=w2582) -> (x*y=w2581:dbl)
            n1397 = Divide(x=w2581, y=2.0) -> (x/y=w2586:dbl)
            n1398 = Select(t=w2586, s=w2590, f=w2587) -> (s? t:f=w2585:dbl)
            n1399 = Select(t=w2587, s=w2590, f=w2586) -> (s? t:f=w2589:dbl)
            n1400 = Subtract(x=w2593, y=w2589) -> (x-y=w2588:dbl)
            n1401 = Subtract(x=w2596, y=w2585) -> (x-y=w2584:dbl)
            n1402 = Not(x=w2590) -> (.not. x?=w2592:bool)
            n1403 = Not(x=w2598) -> (.not. x?=w2594:bool)
            n1404 = And(x=w2590, y=w2594) -> (x .and. y?=w2595:bool)
            n1405 = And(x=w2594, y=w2592) -> (x .and. y?=w2597:bool)
            n1406 = Select(t=w2596, s=w2597, f=w2584) -> (s? t:f=w2573:dbl)
            n1407 = Select(t=w2593, s=w2595, f=w2588) -> (s? t:f=w2576:dbl)
            n1408 = call "V2int16.vi"("InV"=w2573) -> ("Out i16"=w2574:i16)  [unwired: 4 in]
            n1409 = call "V2int16.vi"("InV"=w2576) -> ("Out i16"=w2575:i16)  [unwired: 4 in]
            n1410 = xnode "Read/Write Control"("FPGA VI Reference In"=w2604, "error in"=w2603, "AI to FIFO"=w2600, "APD to FIFO"=w2600, "Start scan (MCL)"=w2600, "AO1 (Y)"=w2575, "AO2 (X)"=w2574) -> ("FPGA VI Reference Out"=w2602:T20, "error out"=w2601:errorcluster)
          }
        }
        "Initial Y" <- w2554
        "Initial X" <- w2553
        "wait to reset values" <- w2555
      }
    }
    n1411 = local read "Trap Pos Elements/DMA read"() -> (w2099:u32)
    n1412 = local read "Trap AI Elements/DMA read"() -> (w2101:u32)
    n1413 = local read "APD Elements/DMA read"() -> (w2100:u32)
    n1414 = call "ReadFIFOs.vi"("FPGA In"=w2093, "Error In"=w2095, "Trap N Read"=w2101, "APD N Read"=w2100, "TPos N Read"=w2099) -> ("FPGA Out"=w2092:T20, "Error Out"=w2091:errorcluster, "Trap Data"=w2086:i16[], "APD Data"=w2089:u32[], "TPos Data"=w2094:u64[], "Trap N Left"=w2096:u32, "APD N Left"=→"APD FIFO Elements Remaining":u32, "TPos N Left"=→"Trap Pos FIFO El Remaining":u32)  [unwired: 7 in]
    "Trap AI FIFO El. Rem." <- w2096
    n1415 = local read "Trap AI FIFO Depth"() -> (w2307:u32)
    n1416 = xnode "Read/Write Control"("FPGA VI Reference In"=w2092, "error in"=w2091) -> ("FPGA VI Reference Out"=w2138:T20, "error out"=w2090:errorcluster, "BD1 Frequency Out 1"=w2084:u64)
    n1417 = flat-sequence "To save data" {
      tunnel: [w2814] -> w2309
      tunnel: [w2815] -> w2308
      tunnel: w2269 -> [w2810]
      tunnel: w2047 -> [w2813]
      tunnel: w2088 -> [w2789]
      tunnel: [w2808] -> w2280
      tunnel: [w2805] -> w2279
      tunnel: [w2802] -> w2278
      tunnel: w2268 -> [w2804]
      tunnel: [w2794] -> w2178
      tunnel: [w2793] -> w2177
      tunnel: w2034 -> [w2787]
      tunnel: w2309 -> [w2964]
      tunnel: w2308 -> [w2963]
      tunnel: w2082 -> [w2962]
      tunnel: w2280 -> [w2960]
      tunnel: w2279 -> [w2959]
      tunnel: w2278 -> [w2958]
      tunnel: w2178 -> [w2957]
      tunnel: w2177 -> [w2956]
      tunnel: w2094 -> [w2955]
      tunnel: w2089 -> [w2954]
      tunnel: w2034 -> [w2953]
      frame #0 {
        # "Channel Pattern, N Channels, dT"
        n1418 = Or(x="Save N Sets", y="Start Saving") -> (x .or. y?=w2799:bool)
        n1419 = Build Array(w2799, "Save Calibration", w2810, w2804) -> (w2812:bool[])
        n1420 = Boolean Array To Number(Boolean array=w2812) -> (number=w2791:u32)
        n1421 = Not Equal To 0?(x=w2791) -> (x != 0?=w2790:bool)
        n1422 = feedback #1(refnum<k0> refnum) -> (w2816:refnum<file>)
        n1423 = feedback #2(0) -> (w2818:i32)
        n1424 = feedback #3(u32 0 ("Cal sets to save")) -> (w2809:u32)
        n1425 = feedback #4(refnum<k0> refnum) -> (w2806:refnum<file>)
        n1426 = feedback #5(FALSE ("Save APD Data\nwith Trap Data")) -> (w2803:bool)
        n1427 = feedback #6(refnum<k0> refnum) -> (w2797:refnum<file>)
        n1428 = feedback #7(FALSE ("Save APD Data\nwith Trap Data")) -> (w2795:bool)
        n1429 = case shown="True" w2790 {
          tunnel: [w2826 1] -> w2814
          tunnel: w2818 -> [w2827 _]
          tunnel: [w2820 w2842] -> w2815
          tunnel: w2816 -> [w2820 _]
          tunnel: w2813 -> [_ w2836]
          tunnel: w2791 -> [_ w2838]
          tunnel: [w2825 w2853] -> w2808
          tunnel: w2809 -> [w2825 _]
          tunnel: [w2824 w2852] -> w2805
          tunnel: w2806 -> [w2824 _]
          tunnel: [w2823 w2851] -> w2802
          tunnel: w2803 -> [w2823 _]
          tunnel: [w2822 w2847] -> w2793
          tunnel: w2797 -> [w2822 _]
          tunnel: [w2821 w2846] -> w2794
          tunnel: w2795 -> [w2821 _]
          tunnel: "Start Saving" -> [_ w2845]
          tunnel: w2789 -> [_ w2832]
          tunnel: w2787 -> [_ w2830]
          frame False {
            n1430 = Increment(x=w2827) -> (x+1=w2826:i32)
          }
          frame True {
            w2850 = FALSE ("Start Saving")
            w2837 = 9.0  # File Ver.
            n1431 = To Double Precision Float(number=w2832) -> (double precision float=w2831:dbl)
            n1432 = To Double Precision Float(number=w2830) -> (double precision float=w2829:dbl)
            n1433 = case "File Info Header" shown="Default" w2838 {
              tunnel: w2837 -> [w2866 w2873]
              tunnel: w2836 -> [w2865 w2868]
              tunnel: w2829 -> [w2864 w2872]
              tunnel: w2831 -> [w2863 w2871]
              tunnel: [w2862 w2870] -> w2835
              frame 2 {
                n1434 = Build Array(w2866, w2865, w2865, w2864, w2863) -> (w2862:dbl[])
              }
              frame Default {
                n1435 = local read "Save ave N"() -> (w2869:i32)
                n1436 = Multiply(x=w2868, y=w2869) -> (x*y=w2867:dbl)
                n1437 = Build Array(w2873, w2868, w2867, w2872, w2871) -> (w2870:dbl[])
              }
            }
            n1438 = case "Scan Info Header" shown="8" w2838 {
              tunnel: [w2891 "Cal sets to save" w2910 w2941] -> w2853
              tunnel: "Save APD" -> [w2885 _ w2905 w2928]
              tunnel: [w2885 w2897 w2905 w2928] -> w2851
              tunnel: [w2884 w2897 w2904 w2927] -> w2846
              tunnel: "Save TPos" -> [w2884 _ w2904 w2927]
              tunnel: w2845 -> [w2888 _ _ _]
              tunnel: [0.0 ("f") 1.0 ("t") 2.0 ("t") 3.0 ("t")] -> w2834
              tunnel: [w2882 w2894 w2900 w2923] -> w2828
              frame 1, Default {
                w2889 = 0.0 ("f")
                # "Regular Data"
                n1439 = Build Array(w2885, w2884) -> (w2886:bool[])
                n1440 = Boolean Array To Number(Boolean array=w2886) -> (number=w2883:u32)
                n1441 = To Double Precision Float(number=w2883) -> (double precision float=w2893:dbl)
                n1442 = Select(t=u32 4000000000, s=w2888, f="N sets to save") -> (s? t:f=w2891:u32)
                n1443 = Build Array(w2893, w2889, w2889, w2889, w2889) -> (w2882:dbl[])
              }
              frame 2 {
                w2895 = 0.0 ("f")
                w2897 = FALSE ("Save APD Data\nwith Trap Data")
                # "Calibration"
                n1444 = Build Array(w2895, w2895, w2895, w2895, w2895) -> (w2894:dbl[])
                "Calibrating Trap..." <- TRUE ("Calibrating...")
              }
              frame 4 {
                w2908 = 0.0 ("f")
                # "Trap Raster"
                n1445 = local read "Number of F/B Scans (AOD)"() -> (w2914:u16)
                n1446 = Build Array(w2905, w2904) -> (w2903:bool[])
                n1447 = local read "Scan Range (MHz)"() -> (w2919:dbl)
                n1448 = local read "Cycles/step (AOD)"() -> (w2916:u64)
                n1449 = local read "Scan steps (AOD)"() -> (w2918:u64)
                n1450 = Boolean Array To Number(Boolean array=w2903) -> (number=w2906:u32)
                n1451 = To Double Precision Float(number=w2906) -> (double precision float=w2909:dbl)
                n1452 = local read "Scan BD"() -> (w2922:bool)
                n1453 = local read "N sets should be saved"() -> (w2911:dbl)
                n1454 = Build Array(w2909, w2908, w2908, w2908, w2908) -> (w2902:dbl[])
                n1455 = Boolean To (0,1)(Boolean=w2922) -> (0, 1=w2921:i16)
                n1456 = To Double Precision Float(number=w2918) -> (double precision float=w2917:dbl)
                n1457 = To Double Precision Float(number=w2916) -> (double precision float=w2915:dbl)
                n1458 = To Double Precision Float(number=w2914) -> (double precision float=w2913:dbl)
                n1459 = To Double Precision Float(number=w2921) -> (double precision float=w2920:dbl)
                n1460 = Build Array(w2920, w2919, w2917, w2915, w2913) -> (w2901:dbl[])
                n1461 = Round Toward +Infinity(x=w2911) -> (ceil(x): smallest int >= x=w2912:dbl)
                n1462 = Build Array (concatenate)(w2902, w2901) -> (w2900:dbl[])
                n1463 = To Unsigned Long Integer(number=w2912) -> (unsigned 32bit integer=w2910:u32)
              }
              frame 8 {
                w2937 = 0.0 ("f")
                # "MCL raster scan"
                n1464 = local read "2D or 1D Scan"() -> (w2934:bool)
                n1465 = local read "N sets should be saved (MCL)"() -> (w2942:dbl)
                n1466 = Build Array(w2928, w2927) -> (w2929:bool[])
                n1467 = Boolean Array To Number(Boolean array=w2929) -> (number=w2926:u32)
                n1468 = To Double Precision Float(number=w2926) -> (double precision float=w2940:dbl)
                n1469 = local read "Scan Range (V)\n(of steps)"() -> (w2949:dbl)
                n1470 = local read "Number of scans (MCL)"() -> (w2932:u64)
                n1471 = Boolean To (0,1)(Boolean=w2934) -> (0, 1=w2936:i16)
                n1472 = To Double Precision Float(number=w2936) -> (double precision float=w2935:dbl)
                n1473 = local read "Cycles/step (MCL)"() -> (w2946:u64)
                n1474 = Build Array(w2940, w2935, w2937, w2937, w2937) -> (w2925:dbl[])
                n1475 = local read "Scan steps (x)"() -> (w2948:u64)
                n1476 = local read "Scan lines (y)"() -> (w2931:u64)
                n1477 = local read "Fast Scan Dir"() -> (w2952:bool)
                n1478 = local read "Initial X"() -> (w2939:dbl)
                n1479 = local read "Initial Y"() -> (w2938:dbl)
                n1480 = Round Toward +Infinity(x=w2942) -> (ceil(x): smallest int >= x=w2943:dbl)
                n1481 = To Unsigned Long Integer(number=w2943) -> (unsigned 32bit integer=w2941:u32)
                n1482 = To Double Precision Float(number=w2948) -> (double precision float=w2947:dbl)
                n1483 = To Double Precision Float(number=w2946) -> (double precision float=w2945:dbl)
                n1484 = Select(t=w2931, s=w2934, f=w2932) -> (s? t:f=w2933:u64)
                n1485 = Boolean To (0,1)(Boolean=w2952) -> (0, 1=w2951:i16)
                n1486 = To Double Precision Float(number=w2951) -> (double precision float=w2950:dbl)
                n1487 = To Double Precision Float(number=w2933) -> (double precision float=w2944:dbl)
                n1488 = Build Array(w2950, w2949, w2947, w2945, w2944, w2939, w2938) -> (w2924:dbl[])
                n1489 = Build Array (concatenate)(w2925, w2924) -> (w2923:dbl[])
              }
            }
            n1490 = local read "BD 1 Frq 1 (MHz)"() -> (w2859:dbl)
            n1491 = local read "BD 2 Frq 1 (MHz)"() -> (w2858:dbl)
            n1492 = local read "BD 1 Frq 2 (MHz)"() -> (w2857:dbl)
            n1493 = local read "BD 2 Frq 2 (MHz)"() -> (w2856:dbl)
            n1494 = local read "BD 1 Frq 3 (MHz)"() -> (w2855:dbl)
            n1495 = local read "BD 2 Frq 3 (MHz)"() -> (w2854:dbl)
            n1496 = Build Array(w2859, w2858, w2857, w2856, w2855, w2854) -> (w2839:dbl[])
            n1497 = local write "Saving..."(TRUE ("Saving...")) -> ()
            n1498 = local write "Save Calibration"(w2850) -> ()
            n1499 = local write "Start Saving"(w2850) -> ()
            n1500 = Build Array (concatenate)(w2835, w2834) -> (w2833:dbl[])
            n1501 = local read "Index"() -> (w2844:dbl)
            n1502 = call "HeaderTrap.vi"("Index In"=w2844, "File Info"=w2833, "BD Frqs"=w2839, "Scan Data"=w2828, "Comment"="Comment") -> ("Index Out"=w2843:dbl, "Trap Path"=w2841:path, "Trap File Out"=w2842:refnum<file>)  [unwired: 12 in]
            n1503 = local write "Index"(w2843) -> ()
            n1504 = local write "Save index"(w2843) -> ()
            n1505 = local write "Save file name"(w2841) -> ()
            n1506 = case "Fluorescence Header" shown="True" w2851 {
              tunnel: w2841 -> [_ w2879]
              tunnel: [refnum<k0> refnum w2878] -> w2852
              frame False {
              }
              frame True {
                n1507 = local read "APD Integration Time (s)"() -> (w2881:dbl)
                n1508 = local read "N APD Samp/step"() -> (w2880:i32)
                n1509 = call "HeaderFluorescence.vi"("N APD Samp/step"=w2880, "APD Integration Time (s)"=w2881, "Trap Path"=w2879) -> ("Flu File"=w2878:refnum<file>)  [unwired: 8 in]
              }
            }
            n1510 = case "TPos Header" shown="True" w2846 {
              tunnel: w2841 -> [_ w2876]
              tunnel: [refnum<k0> refnum w2875] -> w2847
              frame False {
              }
              frame True {
                n1511 = call "HeaderTPos.vi"("Trap Path"=w2876) -> ("TPos File"=w2875:refnum<file>)  [unwired: 10 in]
              }
            }
          }
        }
        n1512 = feedback-in #1(w2815) -> ()
        n1513 = feedback-in #2(w2814) -> ()
        n1514 = feedback-in #3(w2808) -> ()
        n1515 = feedback-in #4(w2805) -> ()
        n1516 = feedback-in #5(w2802) -> ()
        n1517 = feedback-in #6(w2793) -> ()
        n1518 = feedback-in #7(w2794) -> ()
      }
      frame #1 {
        # "N Channels"
        # "TPos, APD, Trap Data"
        n1519 = local read "Saving..."() -> (w2961:bool)
        n1520 = case shown="True" w2961 {
          tunnel: w2964 -> [_ w2968]
          tunnel: w2963 -> [_ w2987]
          tunnel: w2962 -> [_ w2983]
          tunnel: w2960 -> [_ w2967]
          tunnel: w2959 -> [_ w2979]
          tunnel: w2958 -> [_ w2978]
          tunnel: w2957 -> [_ w2976]
          tunnel: w2956 -> [_ w2975]
          tunnel: w2955 -> [_ w2974]
          tunnel: w2954 -> [_ w2973]
          tunnel: w2953 -> [_ w2972]
          frame False {
          }
          frame True {
            n1521 = local read "DMA Update Period (s)"() -> (w2971:dbl)
            n1522 = Divide(x=w2968, y=w2967) -> (x/y=w2970:dbl)
            n1523 = Multiply(x=w2968, y=w2971) -> (x*y=→"Time (s)":dbl)
            n1524 = Less Or Equal?(x=w2968, y=w2967) -> (x <= y?=w2985:bool)
            n1525 = Multiply(x=w2970, y=100.0) -> (x*y=w2966:dbl)
            n1526 = Or(x="Stop Saving", y="Abort save 2") -> (x .or. y?=w2980:bool)
            n1527 = Not(x=w2980) -> (.not. x?=w2986:bool)
            n1528 = And(x=w2985, y=w2986) -> (x .and. y?=w2984:bool)
            n1529 = case shown="True" w2984 {
              tunnel: w2987 -> [w2994 w3015]
              tunnel: w2983 -> [_ w3012]
              tunnel: w2979 -> [w2993 w3008]
              tunnel: w2978 -> [w2992 w3009]
              tunnel: w2976 -> [w2990 w3007]
              tunnel: w2975 -> [w2991 w3006]
              tunnel: w2974 -> [_ w3004]
              tunnel: w2973 -> [_ w3002]
              tunnel: w2972 -> [_ w3001]
              tunnel: w2966 -> [_ w2997]
              tunnel: [0.0 w2997] -> w2965
              frame False {
                w2989 = FALSE
                n1530 = case shown="True" w2992 {
                  tunnel: w2993 -> [_ w2996]
                  frame False {
                  }
                  frame True {
                    n1531 = Close File(refnum=w2996) -> ()  [unwired: 1 in, 2 out]
                  }
                }
                n1532 = case shown="False" w2990 {
                  tunnel: w2991 -> [_ w2995]
                  frame False {
                  }
                  frame True {
                    n1533 = Close File(refnum=w2995) -> ()  [unwired: 1 in, 2 out]
                  }
                }
                n1534 = Close File(refnum=w2994) -> ()  [unwired: 1 in, 2 out]
                n1535 = call <vilib>:"Beep.vi"() -> ()  [unwired: 3 in, 9 out]
                n1536 = property on="Raster Scanning..." class="Bool (strict)"("Val(Sgnl)"=w2989) -> ()  [unwired: 2 in, 2 out]
                n1537 = local write "Calibrating Trap..."(w2989) -> ()
                n1538 = local write "Stop Saving"(w2989) -> ()
                "Saving..." <- w2989
              }
              frame True {
                n1539 = local read "Calibrating Trap..."() -> (w3000:bool)
                n1540 = Equal?(x=1 ("y"), y="Save ave N") -> (x = y?=w3011:bool)
                n1541 = Or(x=w3000, y=w3011) -> (x .or. y?=w3005:bool)
                n1542 = case "Downsample TPos" shown="True" w3005 {
                  tunnel: w3004 -> [w3016 w3027]
                  tunnel: [w3016 w3019] -> w3003
                  tunnel: "Save ave N" -> [_ w3020]
                  frame False {
                  }
                  frame True {
                    w3017 = 2 ("dimension size")
                    n1543 = Array Size(array=w3027) -> (size(s)=w3021:i32)
                    n1544 = Divide(x=w3021, y=w3017) -> (x/y=w3025:dbl)
                    n1545 = Divide(x=w3021, y=w3020) -> (x/y=w3022:dbl)
                    n1546 = Reshape Array(w3027, w3025, w3017) -> (w3026:u64[][])
                    n1547 = Transpose 2D Array(2D array=w3026) -> (transposed array=w3024:u64[][])
                    n1548 = for {
                      tunnel: w3024 -> [w3029] mode=indexing
                      tunnel: [w3028] -> w3018 mode=indexing
                      tunnel: w3020 -> [w3030]
                      workers-P: _ -> [_]
                      n1549 = call "downsample 1D array - U64.vi"("Ave N"=w3030, "Array In"=w3029) -> ("Array Out"=w3028:u64[])  [unwired: 1 in]
                    }
                    n1550 = Transpose 2D Array(2D array=w3018) -> (transposed array=w3023:u64[][])
                    n1551 = Reshape Array(w3023, w3022) -> (w3019:u64[])
                  }
                }
                n1552 = case "Downsample Trap" shown="True" w3005 {
                  tunnel: w3012 -> [w3039 w3050]
                  tunnel: [w3039 w3042] -> w3010
                  tunnel: "Save ave N" -> [_ w3043]
                  tunnel: w3001 -> [_ w3040]
                  frame False {
                    # "Don't downsample"
                  }
                  frame True {
                    n1553 = Array Size(array=w3050) -> (size(s)=w3044:i32)
                    n1554 = Quotient & Remainder(x=w3044, y=w3040) -> (floor(x/y)=w3048:i32)  [unwired: 1 out]
                    n1555 = Quotient & Remainder(x=w3044, y=w3043) -> (floor(x/y)=w3045:i32)  [unwired: 1 out]
                    n1556 = Reshape Array(w3050, w3048, w3040) -> (w3049:i16[][])
                    n1557 = Transpose 2D Array(2D array=w3049) -> (transposed array=w3047:i16[][])
                    n1558 = for {
                      tunnel: w3047 -> [w3053] mode=indexing
                      tunnel: [w3052] -> w3041 mode=indexing
                      tunnel: w3043 -> [w3051]
                      workers-P: _ -> [_]
                      n1559 = call "downsample 1D array - I16.vi"("Ave N"=w3051, "Array In"=w3053) -> ("Array Out"=w3052:i16[])  [unwired: 1 out]
                    }
                    n1560 = Transpose 2D Array(2D array=w3041) -> (transposed array=w3046:i16[][])
                    n1561 = Reshape Array(w3046, w3045) -> (w3042:i16[])
                  }
                }
                n1562 = case "Write fluorescene" shown="True" w3009 {
                  tunnel: w3008 -> [_ w3036]
                  tunnel: w3002 -> [_ w3035]
                  frame False {
                  }
                  frame True {
                    n1563 = Write to Binary File(file (use dialog)=w3036, data=w3035, 5:FALSE ("prepend array or string size? (T)"), 9:T28."big-endian, network order" ("byte order (0:big-endian, network order)")) -> ()  [unwired: 1 in, 4 out]
                  }
                }
                n1564 = case "Save TPos Data" shown="True" w3007 {
                  tunnel: w3006 -> [_ w3032]
                  tunnel: w3003 -> [_ w3031]
                  frame False {
                  }
                  frame True {
                    n1565 = Write to Binary File(file (use dialog)=w3032, data=w3031, 5:FALSE ("prepend array or string size? (T)"), 9:T28."big-endian, network order" ("byte order (0:big-endian, network order)")) -> ()  [unwired: 1 in, 4 out]
                  }
                }
                n1566 = Write to Binary File "Save Trap Data"(file (use dialog)=w3015, data=w3010, 5:FALSE ("prepend array or string size? (T)"), 9:T28."big-endian, network order" ("byte order (0:big-endian, network order)")) -> ()  [unwired: 1 in, 4 out]
              }
            }
            "Progress" <- w2965
            "Progress 2" <- w2965
          }
        }
      }
    }
    n1567 = local read "BD 1 Frq 2 (MHz)"() -> (w2148:dbl)
    n1568 = local read "MCL Tracking"() -> (w2143:bool)
    n1569 = Subtract(x=w2307, y=w2101) -> (x-y=w2306:u32)
    n1570 = Divide(x=w2096, y=w2306) -> (x/y=w2305:dbl)
    "Buffer Status" <- w2305
    n1571 = call "AODuint642MHz.vi"("In u64"=w2084) -> ("Out MHz"=w2083:dbl)  [unwired: 4 in]
    n1572 = Equal?(x=w2305, y=1.0) -> (x = y?=w2303:bool)
    n1573 = Subtract ("TD")(x=w2148, y=w2083) -> (x-y=w2139:dbl)
    "Current Trap Delta" <- w2139
    n1574 = case shown="True" w2143 {
      tunnel: w2083 -> [_ w2438]
      tunnel: w2141 -> [_ w2428]
      frame False {
      }
      frame True {
        n1575 = local read "Zero T1 position"() -> (w2437:dbl)
        n1576 = local read "AOM X Cal (nm/MHz)"() -> (w2435:dbl)
        n1577 = local read "MCL X Cal (nm/V)"() -> (w2431:dbl)
        n1578 = Subtract(x=w2438, y=w2437) -> (x-y=w2436:dbl)
        n1579 = local read "Zero MCL x position"() -> (w2430:dbl)
        n1580 = Multiply(x=w2436, y=w2435) -> (x*y=w2434:dbl)
        n1581 = Multiply(x=w2434, y="Tracking factor") -> (x*y=w2432:dbl)
        n1582 = Divide(x=w2432, y=w2431) -> (x/y=w2429:dbl)
        n1583 = Add(x=w2430, y=w2429) -> (x+y=w2427:dbl)
        "Current MCL (V)" <- w2427
        n1584 = call "V2int16.vi"("InV"=w2427) -> ("Out i16"=w2426:i16)  [unwired: 4 in]
        n1585 = xnode "Read/Write Control"("FPGA VI Reference In"=w2428, "AO2 (X)"=w2426) -> ()  [unwired: 1 in, 2 out]
      }
    }
    n1586 = call "IR AOM word to freq - vec.vi"("Frequency Word In (double vec)"=w2094) -> ("Frequency Out"=w2193:dbl[])
    n1587 = case "Alert buffer overflow" shown="True" w2303 {
      frame False {
      }
      frame True {
        n1588 = call <vilib>:"Beep.vi"() -> ()  [unwired: 3 in, 9 out]
        "Overflow (data lost)" <- TRUE ("Overflow (data lost)")
      }
    }
    n1589 = Decimate 1D Array(w2193) -> (w2192:dbl[], w2191:dbl[])
    n1590 = Build Array(w2192, w2191) -> (w2062:dbl[][])
    n1591 = Array Size(array=w2086) -> (size(s)=→"Waveform Chart":i32)
    n1592 = local read "Dynamic Force FB"() -> (w2147:bool)
    n1593 = local read "Trap Pos. FB ON"() -> (w2146:bool)
    n1594 = local read "Trap Sets"() -> (w2087:u32)
    n1595 = call "Trapu16toDbl.vi"("Detector Type"="Detector Type", "Trap Sets"=w2087, "Raw Trap Data In"=w2086) -> ("Channel pattern"=w2088:i32, "Channel Names"=w2035:string[], "Trap Data"=w2076:dbl[][], "Trap Data Out"=w2082:i16[])  [unwired: 5 in]
    "AI labels" <- w2035
    n1596 = Compound Arithmetic op=AND(w2147, w2146, "Real time offset \ncorrection for setpoint") -> (w2144:bool)
    n1597 = local read "Trap X AI1 (DMA)"() -> (w2187:T13)
    n1598 = case "Apply Offset to Force Feedback" shown="True" w2144 {
      tunnel: w2139 -> [_ w2441]
      tunnel: w2138 -> [_ w2440]
      frame False {
      }
      frame True {
        n1599 = local read "Setpoint offset\nCorrection values"() -> (w2456:dbl[])
        n1600 = local read "Offset file step size"() -> (w2459:dbl)
        n1601 = local read "Negate offset difference"() -> (w2451:bool)
        n1602 = local read "T1 kappa_x (pN/nm)"() -> (w2449:dbl)
        n1603 = local read "T1 alpha_x (nm/V)"() -> (w2450:dbl)
        n1604 = Divide(x=w2441, y=w2459) -> (x/y=w2458:dbl)
        n1605 = Multiply(x="Target Force (pN)", y=2.0) -> (x*y=w2447:dbl)
        n1606 = Multiply(x=w2450, y=w2449) -> (x*y=w2446:dbl)
        n1607 = To Long Integer(number=w2458) -> (32bit integer=w2457:i32)
        n1608 = Divide(x=w2447, y=w2446) -> (x/y=w2445:dbl)
        n1609 = Select(t=-1, s=w2451, f=1) -> (s? t:f=w2452:i32)
        n1610 = Index Array(array=w2456, index=w2457) -> (element=w2455:dbl)
        n1611 = Multiply(x=w2452, y=w2455) -> (x*y=w2444:dbl)
        n1612 = Add(x=w2445, y=w2444) -> (x+y=w2443:dbl)
        n1613 = To Fixed-Point(number=w2443) -> (fixed-point=w2439:fxp<+/-,16,1>)  [unwired: 1 in]
        "Actual setpoint" <- w2439
        n1614 = xnode "Read/Write Control"("FPGA VI Reference In"=w2440, "Trap Pos. FB SP"=w2439) -> ()  [unwired: 1 in, 2 out]
      }
    }
    n1615 = Array Size(array=w2035) -> (size(s)=w2034:i32)
    n1616 = call "Trapi162FXP.vi"("N El. to Ave."="N El. to Ave.", "Trap Data"=w2082) -> ("Trap 2"=w2079:fxp<+/-,16,1>, "Trap 1"=w2080:fxp<+/-,16,1>)  [unwired: 8 in]
    n1617 = Bundle By Name(cluster=w2187, "Set 1"=w2080, "Set 2"=w2079) -> (→"Trap X AI1 (DMA)":T13)
    n1618 = case shown="True" "Use Full Offset?" {
      tunnel: [w2412 w2418] -> w2050
      tunnel: [w2411 w2417] -> w2053
      tunnel: w2139 -> [_ w2424]
      frame False {
        n1619 = Divide(x="T1 offset_x (mV)", y=1000.0) -> (x/y=w2412:dbl)
        n1620 = Divide(x="T2 offset_x (mV)", y=1000.0) -> (x/y=w2411:dbl)
      }
      frame True {
        n1621 = local read "Offset file step size"() -> (w2423:dbl)
        n1622 = local read "Offset Values"() -> (w2425:T14)
        n1623 = Unbundle By Name(w2425) -> ("Trap 1X offset"=w2420:dbl[], "Trap 2X offset"=w2419:dbl[])
        n1624 = Divide(x=w2424, y=w2423) -> (x/y=w2422:dbl)
        n1625 = To Long Integer(number=w2422) -> (32bit integer=w2421:i32)
        n1626 = Index Array(array=w2420, index=w2421) -> (element=w2418:dbl)
        n1627 = Index Array(array=w2419, index=w2421) -> (element=w2417:dbl)
      }
    }
    n1628 = Decimate 1D Array(w2089) -> (w2219:u32[], w2197:u32[])
    n1629 = local read "DMA Update Period (s)"() -> (w2224:dbl)
    n1630 = local read "Data Period (s)"() -> (w2047:dbl)
    n1631 = Build Array(w2219, w2197) -> (w2253:u32[][])
    n1632 = local read "APD Integration Time (s)"() -> (w2074:dbl)
    n1633 = To Double Precision Float(number=w2253) -> (double precision float=w2075:dbl[][])
    n1634 = feedback #8(0.0) -> (w2190:dbl)
    n1635 = Add(x=w2224, y=w2190) -> (x+y=w2282:dbl)
    n1636 = feedback-in #8(w2282) -> ()
    n1637 = To Time Stamp(1:w2190) -> (0:w2061:timestamp)
    n1638 = Multiply(x=w2047, y="Trap Disp. Downsample") -> (x*y=w2059:dbl)
    "Display Period (s)" <- w2059
    n1639 = local read "BD 1 Frq 1 (MHz)"() -> (w2066:dbl)
    n1640 = local read "BD 1 Frq 2 (MHz)"() -> (w2065:dbl)
    n1641 = Reciprocal(x=w2059) -> (1/x=→"Trap Disp. Freq. (Hz)":dbl)
    n1642 = Build Array(w2066, w2065) -> (w2064:dbl[])
    n1643 = Multiply(x=w2074, y="APD Disp. dSamp") -> (x*y=w2072:dbl)
    "APD Display Period (s)" <- w2072
    n1644 = local read "Data points/scans (MCL)"() -> (w2263:dbl)
    n1645 = local read "AOM X Cal (nm/MHz)"() -> (w2067:dbl)
    n1646 = call "TPosDSamp.vi"("TPos Data"=w2062, "Data Period (s)"=w2047, "TPos Disp. Dsamp"="Trap Disp. Downsample", "Time Stamp"=w2061, "Trap Pos"=w2064) -> ("TPos dSampd"=w2063:waveform(dbl)[])  [unwired: 14 in]
    n1647 = call "TrapDSamp.vi"("Trap Data"=w2076, "Data Period (s)"=w2047, "Trap Disp. dSamp"="Trap Disp. Downsample", "Time Stamp"=w2061, "Channel Names"=w2035) -> ("Trap dSampd"=w2078:waveform(dbl)[], "Trap Raw"=w2077:waveform(dbl)[])  [unwired: 13 in]
    n1648 = local read "MCL Scanning"() -> (w2257:bool)
    n1649 = local read "Display Period (s)"() -> (w2212:dbl)
    n1650 = Reciprocal(x=w2072) -> (1/x=→"APD Display Freq. (Hz)":dbl)
    n1651 = call "APDDSamp.vi"("APD Data"=w2075, "Data Period (s)"=w2074, "APD Disp. dSamp"="APD Disp. dSamp", "Time Stamp"=w2061) -> ("APD dSampd"=w2071:waveform(dbl)[])  [unwired: 15 in]
    n1652 = Multiply(x=w2063, y=w2067) -> (x*y=w2068:waveform(dbl)[])
    "Trap Positions" <- w2068
    n1653 = Increment(x=w2263) -> (x+1=w2264:dbl)
    n1654 = feedback #9(w2264) -> (w2267:dbl)
    n1655 = Select(t=0, s=w2254, f=w2267) -> (s? t:f=w2260:dbl)
    n1656 = Index Array(array=w2068, index=0) -> (element=w2173:waveform(dbl))
    n1657 = To Double Precision Float(number=w2219) -> (double precision float=w2218:dbl[])
    n1658 = Array Size(array=w2218) -> (size(s)=w2266:i32)
    n1659 = Add(x=w2266, y=w2260) -> (x+y=w2261:dbl)
    n1660 = Greater?(x=w2261, y=w2263) -> (0:w2262:bool)
    n1661 = Select(t=w2260, s=w2262, f=w2261) -> (s? t:f=w2259:dbl)
    n1662 = Not(x=w2262) -> (.not. x?=w2256:bool)
    n1663 = feedback-in #9(w2259) -> ()
    n1664 = And(x=w2256, y=w2257) -> (x .and. y?=w2258:bool)
    n1665 = Divide(x="Bead Sep. Int. Time (s)", y=w2212) -> (x/y=w2169:dbl)
    n1666 = Unbundle By Name(w2173) -> ("Y"=w2171:dbl[])
    n1667 = Or(x=w2258, y=w2254) -> (x .or. y?=w2255:bool)
    n1668 = feedback #10(w2171) -> (w2172:dbl[])
    n1669 = Build Array (concatenate)(w2171, w2172) -> (w2170:dbl[])
    n1670 = Multiply(x=w2071, y="APD Disp. Scale") -> (x*y=w2070:waveform(dbl)[])
    n1671 = local read "APD Integration Time (s)"() -> (w2210:dbl)
    n1672 = Build Array (concatenate)(w2070, w2078) -> (w2208:waveform(dbl)[])
    "All Signals" <- w2208
    n1673 = Split 1D Array(array=w2170, index=w2169) -> (first subarray=w2163:dbl[])  [unwired: 1 out]
    n1674 = feedback-in #10(w2163) -> ()
    n1675 = local read "Tab Control Display"() -> (w2046:T3)
    n1676 = To Double Precision Float(number=w2197) -> (double precision float=w2196:dbl[])
    n1677 = call-poly <vilib>:"Mean.vi"("X"=w2163) -> ("mean"=w2162:dbl)  [unwired: 1 out]
    "Mean T1 Position (nm)" <- w2162
    n1678 = Subtract(x=w2163, y=w2162) -> (x-y=w2168:dbl[])
    n1679 = Square(x=w2168) -> (x^2=w2167:dbl[])
    n1680 = call-poly <vilib>:"Mean.vi"("X"=w2167) -> ("mean"=w2166:dbl)  [unwired: 1 out]
    n1681 = Square Root(x=w2166) -> (sqrt(x)=w2165:dbl)
    n1682 = Equal?(x="Tab Control Display", y=T3."High Res Display") -> (x = y?=w2222:bool)
    n1683 = Equal?(x=w2046, y=T3."FFT") -> (x = y?=w2044:bool)
    n1684 = Multiply(x="APD Disp. dSamp", y=w2210) -> (x*y=w2209:dbl)
    n1685 = Multiply(x=10.0, y=w2165) -> (x*y=→"Trap 1 Position RMS (A)":dbl)
    n1686 = Divide(x=w2071, y=w2209) -> (x/y=w2194:waveform(dbl)[])
    n1687 = Index Array(array=w2194, index=1) -> (element=w2202:waveform(dbl))
    n1688 = Index Array(array=w2194, index=0) -> (element=w2204:waveform(dbl))
    n1689 = case "For computing FFTs for display" shown="True" w2044 {
      tunnel: w2077 -> [_ w2718]
      frame False {
      }
      frame True {
        n1690 = Build Array("FFT 1 Choice 1", "FFT 1 Choice 2", "FFT 2 Choice 1", "FFT 2 Choice 2") -> (w2711:u16[])
        n1691 = Array Size(array=w2718) -> (size(s)=w2717:i32)
        n1692 = feedback-in #11(w2711) -> ()
        n1693 = feedback #11(u16[] [100, 100, 100, 100]) -> (w2712:u16[])
        n1694 = feedback-in #12("# Spectra to Ave.") -> ()
        n1695 = feedback #12("# Spectra to Ave.") -> (w2709:dbl)
        n1696 = Not Equal?(x="# Spectra to Ave.", y=w2709) -> (x != y?=w2708:bool)
        n1697 = Not Equal?(x=w2711, y=w2712) -> (x != y?=w2710:bool)
        n1698 = feedback #13(1.0) -> (w2695:dbl)
        n1699 = Compound Arithmetic op=OR("Reset FFT", w2710, w2708) -> (w2693:bool)
        n1700 = Select(t=1.0, s=w2693, f=w2695) -> (s? t:f=w2697:dbl)
        n1701 = Greater?(x=w2697, y="# Spectra to Ave.") -> (0:w2716:bool)
        n1702 = Increment(x=w2697) -> (x+1=w2696:dbl)
        n1703 = feedback-in #13(w2696) -> ()
        n1704 = local read "DMA Update Period (s)"() -> (w2691:dbl)
        n1705 = Multiply(x="# Spectra to Ave.", y=w2691) -> (x*y=→"Ave. Time (s)":dbl)
        n1706 = Build Array(cluster{"f0":dbl, "df":dbl, "magnitude":dbl[]} {"f0"=0.0, "df"=0.0, "magnitude"=[]} ("PSD")) -> (w2700:cluster{"f0":dbl, "df":dbl, "magnitude":dbl[]}[])
        n1707 = Build Array(w2700, w2700, w2700, w2700) -> (w2702:T36)
        n1708 = feedback #14(w2702) -> (w2707:T36)
        n1709 = for {
          N: 4 -> [_]
          tunnel: w2711 -> [w2740] mode=indexing
          tunnel: w2718 -> [w2741]
          tunnel: w2717 -> [w2743]
          tunnel: w2693 -> [w2736]
          tunnel: w2716 -> [w2735]
          tunnel: "# Spectra to Ave." -> [w2734]
          tunnel: [w2733] -> w2706 mode=indexing
          tunnel: w2707 -> [w2738] mode=indexing
          tunnel: [w2737] -> w2694 mode=indexing
          tunnel: w2697 -> [w2732]
          n1710 = Less?(x=w2740, y=w2743) -> (x < y?=w2742:bool)
          n1711 = Index Array(array=w2741, index=w2740) -> (element=w2739:waveform(dbl))
          n1712 = case shown="True" w2742 {
            tunnel: w2739 -> [_ w2760]
            tunnel: w2738 -> [w2745 w2758]
            tunnel: [w2745 w2746] -> w2737
            tunnel: w2736 -> [_ w2757]
            tunnel: w2735 -> [_ w2750]
            tunnel: w2734 -> [_ w2749]
            tunnel: [cluster{"f0":dbl, "df":dbl, "magnitude":dbl[]} {"f0"=0.0, "df"=0.0, "magnitude"=[]} ("PSD") w2751] -> w2733
            tunnel: w2732 -> [_ w2748]
            frame False {
            }
            frame True {
              n1713 = call <vilib>:"Std Deviation and Variance.vi"("X"=w2760) -> ("mean"=w2761:dbl)  [unwired: 1 in, 2 out]
              n1714 = Subtract(x=w2760, y=w2761) -> (x-y=w2759:waveform(dbl))
              n1715 = xnode "Spectral Measurements"("Signals"=w2759) -> ("PSD"=w2753:cluster{"f0":dbl, "df":dbl, "magnitude":dbl[]})  [unwired: 1 in, 1 out]
              n1716 = case shown="False" w2757 {
                tunnel: w2758 -> [w2770 _]
                tunnel: [w2766 w2775] -> w2746
                tunnel: w2753 -> [w2769 w2776]
                tunnel: w2750 -> [w2768 _]
                frame False {
                  n1717 = Build Array (concatenate)(w2770, w2769) -> (w2767:cluster{"f0":dbl, "df":dbl, "magnitude":dbl[]}[])
                  n1718 = case shown="True" w2768 {
                    tunnel: w2767 -> [w2771 w2774]
                    tunnel: [w2771 w2772] -> w2766
                    frame False {
                    }
                    frame True {
                      n1719 = Delete From Array(array=w2774, index=0) -> (array with subset deleted=w2772:cluster{"f0":dbl, "df":dbl, "magnitude":dbl[]}[])  [unwired: 1 in, 1 out]
                    }
                  }
                }
                frame True {
                  n1720 = Build Array(w2776) -> (w2775:cluster{"f0":dbl, "df":dbl, "magnitude":dbl[]}[])
                }
              }
              n1721 = for {
                tunnel: w2746 -> [w2765] mode=indexing
                tunnel: [w2764] -> w2756 mode=indexing
                workers-P: _ -> [_]
                n1722 = Unbundle By Name(w2765) -> ("magnitude"=w2764:dbl[])
              }
              n1723 = Transpose 2D Array(2D array=w2756) -> (transposed array=w2755:dbl[][])
              n1724 = for {
                tunnel: w2755 -> [w2763] mode=indexing
                tunnel: [w2762] -> w2754 mode=indexing
                workers-P: _ -> [_]
                n1725 = Add Array Elements(numeric array=w2763) -> (sum=w2762:dbl)
              }
              n1726 = Select(t=w2749, s=w2750, f=w2748) -> (s? t:f=w2747:dbl)
              n1727 = Divide(x=w2754, y=w2747) -> (x/y=w2752:dbl[])
              n1728 = Bundle By Name(cluster=w2753, "magnitude"=w2752) -> (w2751:cluster{"f0":dbl, "df":dbl, "magnitude":dbl[]})
            }
          }
        }
        n1729 = case shown="True" w2693 {
          tunnel: w2694 -> [w2725 w2731]
          tunnel: [w2725 w2726] -> w2692
          frame False {
          }
          frame True {
            n1730 = Array Subset(array=w2731, index (row)=0 ("index"), length (row)=4 ("length"), index (col)=0 ("index"), length (col)=1 ("length")) -> (w2726:T36)
          }
        }
        n1731 = feedback-in #14(w2692) -> ()
        n1732 = Split 1D Array(array=w2706, index=2) -> (first subarray=→"FFT 1":cluster{"f0":dbl, "df":dbl, "magnitude":dbl[]}[], second subarray=→"FFT 2":cluster{"f0":dbl, "df":dbl, "magnitude":dbl[]}[])
      }
    }
    n1733 = case "For displaying the high frequency display (no downsampling)" shown="True" w2222 {
      tunnel: w2077 -> [_ w2470]
      frame False {
      }
      frame True {
        n1734 = Index Array(array=w2470, index="High Res. Display") -> (element=w2471:waveform(dbl))
        n1735 = call <vilib>:"Std Deviation and Variance.vi"("X"=w2471) -> ("mean"=w2478:dbl, "standard deviation"=w2483:dbl)  [unwired: 1 in, 1 out]
        "Mean Intensity" <- w2478
        "Sigma" <- w2483
        n1736 = Subtract(x=w2471, y=w2478) -> (x-y=w2477:waveform(dbl))
        n1737 = Select(t=w2477, s="Subtract mean", f=w2471) -> (s? t:f=→"1 Channel":waveform(dbl))
        n1738 = Divide(x=w2483, y=w2478) -> (x/y=→"Sigma/Mean":dbl)
        n1739 = feedback #15(1) -> (w2472:i32)
        n1740 = Greater Or Equal?(x=w2472, y="Slow mean N ave.") -> (x >= y?=w2485:bool)
        n1741 = Increment(x=w2472) -> (x+1=w2487:i32)
        n1742 = Select(t=1, s=w2485, f=w2487) -> (s? t:f=w2474:i32)
        n1743 = feedback-in #15(w2474) -> ()
        n1744 = feedback #16() -> (w2475:waveform(dbl))  [unwired: 1 out]
        n1745 = case shown="Default" w2472 {
          tunnel: [w2490 w2493] -> w2476
          tunnel: w2475 -> [w2492 _]
          tunnel: w2471 -> [w2491 w2493]
          frame Default {
            n1746 = call-poly <vilib>:"Append Waveforms.vi"("waveform B"=w2491, "waveform A"=w2492) -> ("waveform out"=w2490:waveform(dbl))  [unwired: 1 in, 8 out]
          }
          frame 1 {
          }
        }
        n1747 = feedback-in #16(w2476) -> ()
        n1748 = case shown="True" w2485 {
          tunnel: w2476 -> [_ w2489]
          frame False {
          }
          frame True {
            n1749 = call-poly <vilib>:"Mean.vi"("X"=w2489) -> ("mean"=→"Slow mean":dbl)  [unwired: 1 out]
          }
        }
      }
    }
    n1750 = case "Update MCL Scan Images" shown="True" w2255 {
      tunnel: w2254 -> [_ w2523]
      tunnel: w2218 -> [_ w2539]
      tunnel: w2263 -> [_ _]
      tunnel: w2077 -> [_ w2541]
      tunnel: w2196 -> [_ w2535]
      tunnel: w2195 -> [_ w2540]
      frame False {
      }
      frame True {
        n1751 = local read "Cycles/step (MCL)"() -> (w2524:u64)
        n1752 = local read "N APD Samp/step"() -> (w2536:i32)
        n1753 = local read "Scan steps (x)"() -> (w2526:u64)
        n1754 = Index Array(array=w2541, index=10) -> (element=w2544:waveform(dbl))
        n1755 = Index Array(array=w2541, index=11) -> (element=w2542:waveform(dbl))
        n1756 = local read "Scan lines (y)"() -> (w2525:u64)
        n1757 = Unbundle By Name(w2544) -> ("Y"=w2527:dbl[])
        n1758 = Unbundle By Name(w2542) -> ("Y"=w2528:dbl[])
        n1759 = Unbundle(w2540) -> ("New Image"=w2538:T4, "New Image"=w2534:T4, "New Image"=w2532:T4, "New Image"=w2529:T4)
        n1760 = call "MCLScanAPD.vi"("Image In"=w2538, "APD Cts"=w2539, "Scan steps (MCL)"=w2526, "Scan lines (y)"=w2525, "N APD Samp/step"=w2536, "NewScan?"=w2523) -> ("Image Out"=→"APD 1":T4)  [unwired: 13 in]
        n1761 = call "MCLScanAPD.vi"("Image In"=w2534, "APD Cts"=w2535, "Scan steps (MCL)"=w2526, "Scan lines (y)"=w2525, "N APD Samp/step"=w2536, "NewScan?"=w2523) -> ("Image Out"=→"APD 2":T4)  [unwired: 13 in]
        n1762 = call "MCLScanPSD.vi"("In Image"=w2529, "Trap Detector"=w2527, "Scan steps (x)"=w2526, "Scan lines (y)"=w2525, "Cycles/step (MCL)"=w2524, "NewScan?"=w2523) -> ("Out Image"=→"Detection Laser Y":T4)  [unwired: 13 in]
        n1763 = call "MCLScanPSD.vi"("In Image"=w2532, "Trap Detector"=w2528, "Scan steps (x)"=w2526, "Scan lines (y)"=w2525, "Cycles/step (MCL)"=w2524, "NewScan?"=w2523) -> ("Out Image"=→"Detection Laser X":T4)  [unwired: 13 in]
      }
    }
    n1764 = Subtract(x=w2202, y="APD 2 Offset") -> (x-y=w2199:waveform(dbl))
    n1765 = Subtract(x=w2204, y="APD 1 Offset") -> (x-y=w2200:waveform(dbl))
    n1766 = Index Array(array=w2208, index=3) -> (element=w2043:waveform(dbl))
    n1767 = Index Array(array=w2208, index=6) -> (element=w2058:waveform(dbl))
    n1768 = Build Array(w2200, w2199) -> (→"APD Chart":waveform(dbl)[])
    n1769 = feedback-in #17("Calibration") -> ()
    n1770 = feedback #17(u16 1 ("Calibration")) -> (w2238:u16)
    n1771 = local read "AOM X Cal (nm/MHz)"() -> (w2150:dbl)
    n1772 = local read "Trap 2 Bead Size (nm)"() -> (w2153:dbl)
    n1773 = local read "Trap 1 Bead Size (nm)"() -> (w2152:dbl)
    n1774 = local read "Trap Delta (MHz)"() -> (w2149:dbl)
    n1775 = call "CalcForce.vi"("Trap 1X V"=w2043, "T1 alphaX (nm/V)"="T1 alpha_x (nm/V)", "T1 kappaX (pN/nm)"="T1 kappa_x (pN/nm)", "T1 offset X"=w2050, "Trap 2X V"=w2058, "Calibration"="Calibration", "T2 alphaX (nm/V)"="T2 alpha_x (nm/V)", "T2 kappaX (pN/nm)"="T2 kappa_x (pN/nm)", "T2 offsetX"=w2053) -> ("Force 1X"=w2056:waveform(dbl), "Force X"=w2038:waveform(dbl), "Force 2X"=w2057:waveform(dbl), "BeadDeflection"=w2040:waveform(dbl), "Out Names"=w2048:T37)  [unwired: 2 in]
    n1776 = Not Equal?(x=w2238, y="Calibration") -> (x != y?=w2220:bool)
    n1777 = Unbundle By Name(w2038) -> ("Y"=w2037:dbl[])
    n1778 = Unbundle By Name(w2040) -> ("Y"=w2039:dbl[])
    n1779 = case shown="True" w2220 {
      tunnel: w2048 -> [_ w2522]
      frame False {
      }
      frame True {
        n1780 = Unbundle(w2522) -> ("Label.Text"=w2517:string, "Label.Text"=w2521:string, "Label.Text"=w2520:string, "Label.Text"=w2519:string, "Label.Text"=w2518:string)
        n1781 = property on="T1 X" class="DigNum (strict)"("Caption.Text"=w2517) -> ()  [unwired: 2 in, 2 out]
        n1782 = property on="T2 X" class="DigNum (strict)"("Caption.Text"=w2521) -> ()  [unwired: 2 in, 2 out]
        n1783 = property on="Force" class="WFChart (strict)"("YScale.NameLbl.Text"=w2520) -> ()  [unwired: 2 in, 2 out]
        n1784 = property on="Difference" class="DigNum (strict)"("Caption.Text"=w2519) -> ()  [unwired: 2 in, 2 out]
        n1785 = property on="Mean" class="DigNum (strict)"("Caption.Text"=w2518) -> ()  [unwired: 2 in, 2 out]
      }
    }
    n1786 = Subtract(x=w2037, y=w2039) -> (x-y=w2041:dbl[])
    n1787 = Multiply(x=w2150, y=w2149) -> (x*y=w2154:dbl)
    n1788 = Bundle By Name(cluster=w2038, "Y"=w2041) -> (w2042:waveform(dbl))
    n1789 = call-poly <vilib>:"Mean.vi"("X"=w2042) -> ("mean"=w2155:dbl)  [unwired: 1 out]
    n1790 = Add(x=w2154, y=w2155) -> (x+y=w2158:dbl)
    n1791 = Subtract(x=w2042, y="Offset (nm)") -> (x-y=w2214:waveform(dbl))
    n1792 = Unbundle By Name(w2056) -> ("Y"=w2133:dbl[])
    n1793 = Unbundle By Name(w2057) -> ("Y"=w2132:dbl[])
    n1794 = Add(x=w2153, y=w2152) -> (x+y=w2156:dbl)
    n1795 = case shown="False" "Negate trap 2 force" {
      tunnel: [-1.0 1.0] -> w2229
      frame False {
      }
      frame True {
      }
    }
    n1796 = Divide(x=w2156, y=2.0) -> (x/y=w2151:dbl)
    n1797 = Subtract(x=w2158, y=w2151) -> (x-y=→"Tether Extension (nm, calculated)":dbl)
    n1798 = Subtract(x=w2133, y=w2132) -> (x-y=w2130:dbl[])
    n1799 = Divide(x=w2130, y=2.0) -> (x/y=w2129:dbl[])
    n1800 = Multiply(x=w2057, y=w2229) -> (x*y=w2230:waveform(dbl))
    n1801 = Bundle By Name(cluster=w2056, "Y"=w2129) -> (w2128:waveform(dbl))
    n1802 = case shown="True" "Read Lateness and Rel Phase" {
      tunnel: w2138 -> [w2495 w2516]
      tunnel: [w2495 w2515] -> w2227
      tunnel: [w2494 w2514] -> w2226
      tunnel: w2090 -> [w2494 w2496]
      frame False {
      }
      frame True {
        n1803 = xnode "Read/Write Control"("FPGA VI Reference In"=w2516, "error in"=w2496) -> ("FPGA VI Reference Out"=w2515:T20, "error out"=w2514:errorcluster, "GI Relative phase"=→"GI relative phase":i16, "Relative phase"=→"Relative phase (AI1)":i16, "AI Late Counter"=→"Late Counter (AI1)":u8, "GI Late Counter"=→"GI Late Counter":u8, "MCL Late Counter"=→"MCL Late Counter":u8, "MCL Relative Phase"=→"Relative Phase (MCL)":i16, "APD Acq Relative Phase"=→"APD Acq Relative Phase":i16, "APD 1 Gate Relative Phase"=→"APD 1 Gate Relative Phase":i16, "APD 2 Gate Relative Phase"=→"APD 2 Gate Relative Phase":i16, "APD Acq Late Counter"=→"APD Acq Late Counter":u16, "APD 1 Gate Late Counter"=→"APD 1 Gate Late Counter":u8, "APD 2 Gate Late Counter"=→"APD 2 Gate Late Counter":u8, "Green FB Relative Phase"=→"Relative phase (Green FB)":i16, "GI Relative phase"=→"GI relative phase 2":i16, "GI Late Counter 2"=→"GI Late Counter 2":u16, "Trap Pos FIFO Timeout"=→"Trap Pos FIFO Timeout":u16, "Trap AI FIFO Timeout"=→"Trap AI FIFO Timeout":u16)
      }
    }
    n1804 = Unbundle By Name(w2057) -> ("Y"=w2126:dbl[])
    n1805 = Unbundle By Name(w2056) -> ("Y"=w2127:dbl[])
    n1806 = Build Array(w2056, w2230, w2128) -> (→"Force":waveform(dbl)[])
    n1807 = call-poly <vilib>:"Mean.vi"("X"=w2126) -> ("mean"=w2124:dbl)  [unwired: 1 out]
    "T2 X" <- w2124
    n1808 = call-poly <vilib>:"Mean.vi"("X"=w2127) -> ("mean"=w2125:dbl)  [unwired: 1 out]
    "T1 X" <- w2125
    n1809 = Subtract(x=w2127, y=w2126) -> (x-y=w2216:dbl[])
    n1810 = Bundle By Name("Y"=w2214) -> (→"Bead Separation":waveform(dbl))  [unwired: 1 out]
    n1811 = Divide(x=w2216, y=2.0) -> (x/y=→"Vec Mean of T1 T2":dbl[])
    n1812 = Subtract(x=w2125, y=w2124) -> (x-y=w2237:dbl)
    n1813 = Add(x=w2125, y=w2124) -> (x+y=→"Difference":dbl)
    n1814 = Divide(x=w2237, y=2.0) -> (x/y=w2104:dbl)
    "Mean" <- w2104
    n1815 = case shown="True" "Semi Passive ON" {
      tunnel: "Semi Passive mode" -> [_ w2370]
      tunnel: "Jump Force (pN)" -> [_ w2369]
      tunnel: w2104 -> [_ w2368]
      frame False {
      }
      frame True {
        n1816 = case shown="\"Sharp Jump\"" w2370 {
          tunnel: w2369 -> [_ w2373 w2389]
          tunnel: w2368 -> [_ w2372 w2388]
          frame "None" {
          }
          frame "Use Feedback" {
            n1817 = local read "Target Force (pN)"() -> (w2375:dbl)
            n1818 = Less?(x=w2373, y=w2375) -> (x < y?=w2374:bool)
            n1819 = case shown="True" w2374 {
              tunnel: w2373 -> [w2382 w2385]
              tunnel: w2372 -> [w2381 w2384]
              tunnel: [w2380 w2383] -> w2371
              frame False {
                n1820 = Less?(x=w2382, y=w2381) -> (x < y?=w2380:bool)
              }
              frame True {
                n1821 = Greater?(x=w2385, y=w2384) -> (0:w2383:bool)
              }
            }
            n1822 = case shown="True" w2371 {
              frame False {
                n1823 = local read "Trap Pos. FB ON"() -> (w2376:bool)
                n1824 = case shown="True" w2376 {
                  frame False {
                  }
                  frame True {
                    n1825 = property on="Trap Pos. FB ON" class="Bool (strict)"("Val(Sgnl)"=FALSE) -> ()  [unwired: 2 in, 2 out]
                  }
                }
              }
              frame True {
                n1826 = local read "Trap Pos. FB ON"() -> (w2378:bool)
                n1827 = case shown="False" w2378 {
                  frame False {
                    n1828 = property on="Trap Pos. FB ON" class="Bool (strict)"("Val(Sgnl)"=TRUE) -> ()  [unwired: 2 in, 2 out]
                  }
                  frame True {
                  }
                }
              }
            }
          }
          frame "Sharp Jump" {
            n1829 = local read "Target Force (pN)"() -> (w2391:dbl)
            n1830 = Greater?(x=w2389, y=w2391) -> (0:w2390:bool)
            n1831 = case shown="False" w2390 {
              tunnel: w2389 -> [w2406 w2410]
              tunnel: w2388 -> [w2407 w2409]
              tunnel: [w2405 w2408] -> w2387
              frame False {
                n1832 = Greater?(x=w2407, y=w2406) -> (0:w2405:bool)
              }
              frame True {
                n1833 = Less?(x=w2410, y=w2409) -> (x < y?=w2408:bool)
              }
            }
            n1834 = Subtract(x=w2389, y=w2391) -> (x-y=w2386:dbl)
            n1835 = case shown="True" w2387 {
              tunnel: w2386 -> [_ w2397]
              frame False {
              }
              frame True {
                n1836 = local read "T1 kappa_x (pN/nm)"() -> (w2402:dbl)
                n1837 = local read "T2 kappa_x (pN/nm)"() -> (w2403:dbl)
                n1838 = Reciprocal(x="DNA stiffness (pN / nm)") -> (1/x=w2399:dbl)
                n1839 = Reciprocal(x=w2402) -> (1/x=w2401:dbl)
                n1840 = Reciprocal(x=w2403) -> (1/x=w2400:dbl)
                n1841 = Compound Arithmetic op=ADD(w2401, w2400, w2399) -> (w2398:dbl)
                n1842 = local read "AOM X Cal (nm/MHz)"() -> (w2396:dbl)
                n1843 = Multiply(x=w2398, y=w2397) -> (x*y=w2395:dbl)
                n1844 = local read "Trap Delta (MHz)"() -> (w2393:dbl)
                n1845 = Divide(x=w2395, y=w2396) -> (x/y=w2394:dbl)
                n1846 = Subtract(x=w2393, y=w2394) -> (x-y=w2392:dbl)
                n1847 = property on="Trap Delta (MHz)" class="DigNum (strict)"("Val(Sgnl)"=w2392) -> ()  [unwired: 2 in, 2 out]
              }
            }
          }
        }
      }
    }
    n1848 = xnode "Read/Write Control"("FPGA VI Reference In"=w2227, "error in"=w2226) -> ("FPGA VI Reference Out"=w2299:T20, "error out"=w2293:errorcluster, "AI2 Y Sum Set 1"=w2289:i16, "AI2 Y Sum Set 2"=w2288:i16, "AI1 X Set 1"=w2185:fxp<+/-,16,1>, "AI1 X Set 2"=w2184:fxp<+/-,16,1>, "Trap Pos FB Int Signal"=→"Trap Pos FB Int Signal":fxp<+/-,24,9>, "Trap Pos FB Int-Norm Signal"=→"Trap Pos FB Int-Norm Signal":fxp<+/-,16,1>, "Trap Pos FB Action"=w2182:i64, "Scanning"=→"AOD Scanning":bool, "Scan I"=→"AOD Scan I":u64, "Scanning MCL"=w2291:bool, "Scan I (MCL)"=→"MCL Scan I":u64, "Green FB Signals"=w2248:T38, "BD1 amplitude 1 out"=w2123:u16, "BD1 amplitude 2 out"=w2108:u16)  [unwired: 1 out]
    "MCL Scanning" <- w2291
    "Trap Pos FB Action" <- w2182
    n1849 = local read "Fish Status"() -> (w2103:u16)
    n1850 = local read "AI2 (V)"() -> (w2290:cluster{"Set 1":dbl, "Set 2":dbl})
    n1851 = case shown="False" "Toggle AFish" {
      tunnel: w2104 -> [w2311 _]
      tunnel: w2103 -> [w2310 w2354]
      frame False {
        n1852 = case "Autofishing - Alex" shown="3" w2310 {
          tunnel: w2311 -> [_ _ _ w2340 _]
          frame 0, Default {
            # "Off"
          }
          frame 1 {
            # "Approach"
            n1853 = local read "Trap Delta (MHz)"() -> (w2314:dbl)
            n1854 = Add(x=w2314, y="Approach dTD") -> (x+y=w2313:dbl)
            n1855 = In Range and Coerce(upper limit=inf, x=w2313, lower limit="Min TD") -> (coerced(x)=w2315:dbl, In Range?=w2316:bool)
            n1856 = case shown="False" w2316 {
              frame False {
                w2320 = u16 2 items=["Off", "Approach", "Wiggle", "Extend", "Tether Found"] ("Fish Status")
                n1857 = Tick Count (ms)() -> (millisecond timer value=→"AF Time":u32)
                n1858 = local write "Fish Status"(w2320) -> ()
              }
              frame True {
              }
            }
            n1859 = property on="Trap Delta (MHz)" class="DigNum (strict)"("Val(Sgnl)"=w2315) -> ()  [unwired: 2 in, 2 out]
          }
          frame 2 {
            # "Wiggle"
            n1860 = Random Number (0-1)() -> (number: 0 to 1=w2326:dbl)
            n1861 = local read "Min TD"() -> (w2323:dbl)
            n1862 = local read "AF Time"() -> (w2331:u32)
            n1863 = Multiply(x=w2326, y="Wiggle TD") -> (x*y=w2324:dbl)
            n1864 = Tick Count (ms)() -> (millisecond timer value=w2332:u32)
            n1865 = Add(x=w2324, y=w2323) -> (x+y=w2321:dbl)
            n1866 = Subtract(x=w2332, y=w2331) -> (x-y=w2330:u32)
            n1867 = property on="Trap Delta (MHz)" class="DigNum (strict)"("Val(Sgnl)"=w2321) -> ()  [unwired: 2 in, 2 out]
            n1868 = Divide(x=w2330, y=u32 1000) -> (x/y=w2328:dbl)
            n1869 = Greater?(x=w2328, y="Wiggle time") -> (0:w2322:bool)
            n1870 = case shown="True" w2322 {
              frame False {
              }
              frame True {
                w2333 = u16 3 items=["Off", "Approach", "Wiggle", "Extend", "Tether Found"] ("Fish Status")
                n1871 = local write "Fish Status"(w2333) -> ()
              }
            }
          }
          frame 3 {
            # "Force"
            # "Extend"
            n1872 = local read "Trap Delta (MHz)"() -> (w2346:dbl)
            n1873 = Greater?(x=w2340, y="Extend Min F") -> (0:w2339:bool)
            n1874 = Add(x=w2346, y="Extend dTD") -> (x+y=w2344:dbl)
            n1875 = In Range and Coerce(upper limit="Max TD", x=w2344, lower limit=0.0) -> (coerced(x)=w2335:dbl, In Range?=w2334:bool)
            n1876 = Greater?(x=w2335, y="Extend Min TD") -> (0:w2338:bool)
            n1877 = And(x=w2338, y=w2339) -> (x .and. y?=w2337:bool)
            n1878 = case shown="False" w2337 {
              tunnel: w2334 -> [w2347 _]
              frame False {
                n1879 = case shown="True" w2347 {
                  frame False {
                    w2348 = u16 1 items=["Off", "Approach", "Wiggle", "Extend", "Tether Found"] ("Fish Status")
                    n1880 = local write "Fish Status"(w2348) -> ()
                  }
                  frame True {
                  }
                }
              }
              frame True {
                w2349 = u16 4 items=["Off", "Approach", "Wiggle", "Extend", "Tether Found"] ("Fish Status")
                n1881 = local write "Fish Status"(w2349) -> ()
              }
            }
            n1882 = property on="Trap Delta (MHz)" class="DigNum (strict)"("Val(Sgnl)"=w2335) -> ()  [unwired: 2 in, 2 out]
          }
          frame 4 {
            w2350 = u16 0 items=["Off", "Approach", "Wiggle", "Extend", "Tether Found"] ("Fish Status")
            n1883 = call <vilib>:"Beep.vi"("use system alert? (T)"=FALSE, "duration (msec)"=u32 100, "frequency (Hz)"=u32 466) -> ()  [unwired: 9 in]
            n1884 = local write "Fish Status"(w2350) -> ()
          }
        }
      }
      frame True {
        n1885 = case shown="Default" w2354 {
          frame 0 {
            w2356 = u16 1 items=["Off", "Approach", "Wiggle", "Extend", "Tether Found"] ("Fish Status")
            n1886 = local write "Fish Status"(w2356) -> ()
          }
          frame Default {
            w2357 = u16 0 items=["Off", "Approach", "Wiggle", "Extend", "Tether Found"] ("Fish Status")
            n1887 = local write "Fish Status"(w2357) -> ()
          }
        }
        n1888 = local write "Toggle AFish"(FALSE ("Toggle AFish")) -> ()
      }
    }
    n1889 = Bundle By Name(cluster=w2290, "Set 1"=w2289, "Set 2"=w2288) -> (w2286:cluster{"Set 1":dbl, "Set 2":dbl})
    n1890 = Divide(x=w2182, y=327.67) -> (x/y=→"Action (%)":dbl)
    n1891 = local read "Trap X (AI1)"() -> (w2189:T1)
    n1892 = Divide(x=w2286, y=3276.7) -> (x/y=w2285:cluster{"Set 1":dbl, "Set 2":dbl})
    n1893 = local write "AI2 (V)"(w2285) -> ()
    n1894 = Bundle(cluster=w2189, "Trap 1"=w2185, "Trap 2"=w2184) -> (→"Trap X (AI1)":T1)
    n1895 = Scale By Power Of 2(n=i16 12, x=ext 1.0) -> (x*2^n=w2119:ext)
    n1896 = Subtract(x=w2119, y=ext 1.0) -> (x-y=w2116:ext)
    n1897 = Divide(x=w2248, y=3276.7) -> (x/y=w2244:T39)
    n1898 = Multiply(x=w2123, y=ext 100.0) -> (x*y=w2117:ext)
    n1899 = Unbundle By Name(w2244) -> ("Green FB Ch 0"=w2247:dbl, "Green FB Ch 1"=w2246:dbl, "Green FB Ch 2"=w2245:dbl)
    n1900 = local read "All FB On/Off"() -> (w2107:bool)
    n1901 = Divide(x=w2117, y=w2116) -> (x/y=w2106:ext)
    "Trap 1 amplitude" <- w2106
    n1902 = Scale By Power Of 2(n=i16 12, x=ext 1.0) -> (x*2^n=w2112:ext)
    n1903 = Subtract(x=w2112, y=ext 1.0) -> (x-y=w2115:ext)
    n1904 = Multiply(x=w2108, y=ext 100.0) -> (x*y=w2114:ext)
    n1905 = Divide(x=w2247, y=w2245) -> (x/y=w2243:dbl)
    n1906 = Divide(x=w2246, y=w2245) -> (x/y=w2242:dbl)
    n1907 = Divide(x=w2114, y=w2115) -> (x/y=w2105:ext)
    "Trap 2 amplitude" <- w2105
    n1908 = Bundle By Name(cluster=w2244, "Green FB Ch 0"=w2243, "Green FB Ch 1"=w2242) -> (w2235:T39)
    "Green FB Signals (V)" <- w2235
    n1909 = case shown="True" w2107 {
      tunnel: w2106 -> [_ w2362]
      tunnel: w2105 -> [_ w2361]
      frame False {
      }
      frame True {
        w2363 = 50.0
        n1910 = Greater?(x=w2361, y=w2363) -> (0:w2359:bool)
        n1911 = Greater?(x=w2362, y=w2363) -> (0:w2360:bool)
        n1912 = Or(x=w2360, y=w2359) -> (x .or. y?=w2358:bool)
        n1913 = case shown="True" w2358 {
          frame False {
          }
          frame True {
            n1914 = property on="All FB On/Off" class="Bool (strict)"("Val(Sgnl)"=FALSE) -> ()  [unwired: 2 in, 2 out]
            "Feedback overload" <- TRUE
          }
        }
      }
    }
    n1915 = Unbundle By Name(w2235) -> ("Green FB Ch 2"=→"Green FB Plot":dbl)
    n1916 = local read "wait to reset values"() -> (w2294:bool)
    n1917 = Not(x=w2291) -> (.not. x?=w2295:bool)
    n1918 = And(x=w2295, y=w2294) -> (x .and. y?=w2296:bool)
    n1919 = case "Part of MCL raster scanning: returns to initial positions after scan done" shown="True" w2296 {
      tunnel: w2299 -> [w2615 w2622]
      tunnel: [w2615 w2621] -> w2298
      tunnel: w2293 -> [w2614 w2620]
      tunnel: [w2614 w2619] -> w2292
      frame False {
      }
      frame True {
        w2630 = 10.0 ("y")
        w2629 = 32767.0 ("y")
        # "to return scan values\nafter a synchronous \nAOM scan"
        n1920 = local read "MCL X"() -> (w2623:dbl)
        n1921 = local read "MCL Y"() -> (w2624:dbl)
        n1922 = local write "wait to reset values"(FALSE ("wait to reset values")) -> ()
        n1923 = Multiply(x=w2624, y=w2629) -> (x*y=w2626:dbl)
        n1924 = Multiply(x=w2623, y=w2629) -> (x*y=w2628:dbl)
        n1925 = Divide(x=w2626, y=w2630) -> (x/y=w2625:dbl)
        n1926 = Divide(x=w2628, y=w2630) -> (x/y=w2627:dbl)
        n1927 = To Word Integer(number=w2625) -> (16bit integer=w2631:i16)
        n1928 = To Word Integer(number=w2627) -> (16bit integer=w2632:i16)
        n1929 = local read "Total Counts (ticks)"() -> (w2616:u32)
        n1930 = xnode "Read/Write Control"("FPGA VI Reference In"=w2622, "error in"=w2620, "AO1 (Y)"=w2631, "AO2 (X)"=w2632, "MCL count"=w2616) -> ("FPGA VI Reference Out"=w2621:T20, "error out"=w2619:errorcluster)
        n1931 = local read "Scan Range (V)\n(of steps)"() -> (w2617:dbl)
        n1932 = property on="Scan Range (V)\n(of steps)" class="DigNum (strict)"("Val(Sgnl)"=w2617) -> ()  [unwired: 2 in, 2 out]
      }
    }
    n1933 = node-c288() -> ()  [unwired: 2 out]
  }
  n1934 = node-c288(3 ("Processor")) -> (w86:T24)  [unwired: 3 out]
  n1935 = timed-loop "Oscillate AOD (debugging)" {
    tunnel: w45 -> [w3055]
    tunnel: [w3054] -> w51
    timing: w86 -> [_]
    timing-out: [_] -> w85
    stop <- w3054 stop-if-true
    n1936 = node-c288() -> ()  [unwired: 2 out]
    n1937 = event shown="[1] \"Fl. Triggered...\": Value Change" {
      selector: _ -> [_ _ _]
      dyn-events: _ -> [_ _ _]
      timeout: _ -> [_ _ _]
      tunnel: w3055 -> [w3062 _ _]
      tunnel: [FALSE ("Stop All") _ w3328] -> w3054
      event "Oscillate Set 2", "Fish for Tether": Value Change {
        n1938 = event-data() -> ()  [unwired: 6 out]
        n1939 = local read "Oscillate Set 2"() -> (w3061:bool)
        n1940 = Or(x=w3061, y="Fish for Tether") -> (x .or. y?=w3059:bool)
        n1941 = case shown="True" w3059 {
          tunnel: w3062 -> [_ w3065]
          tunnel: "Fish for Tether" -> [_ w3064]
          frame False {
          }
          frame True {
            n1942 = case shown="True" w3064 {
              frame False {
              }
              frame True {
                n1943 = local write "Scan axis 2"(TRUE) -> ()
                n1944 = local write "Tether"(FALSE ("Tether")) -> ()
              }
            }
            n1945 = node-c288("Period") -> (w3067:T24)  [unwired: 3 out]
            n1946 = timed-loop "Oscillate AOD" {
              timing: w3067 -> [_]
              timing-out: [_] -> w3066
              tunnel: w3065 -> [w3077]
              tunnel: w3064 -> [w3076]
              i -> [w3079]
              stop <- w3075 stop-if-true
              n1947 = node-c288() -> (w3078:i64)  [unwired: 1 out]
              n1948 = flat-sequence {
                tunnel: w3079 -> [w3105]
                tunnel: w3078 -> [w3104]
                tunnel: w3077 -> [w3088]
                tunnel: w3076 -> [w3090]
                tunnel: [w3090] -> w3074
                tunnel: [w3089] -> w3073
                tunnel: [w3087] -> w3072
                tunnel: [w3084] -> w3070
                tunnel: w3074 -> [w3141]
                tunnel: w3073 -> [w3139]
                tunnel: w3072 -> [w3138]
                tunnel: [w3137] -> w3071
                tunnel: w3070 -> [w3136]
                tunnel: [w3205] -> w3075
                tunnel: w3071 -> [w3203]
                frame #0 {
                  n1949 = Divide(x=w3104, y=i64 1000) -> (x/y=w3099:dbl)
                  n1950 = Multiply(x=w3099, y=w3105) -> (x*y=w3101:dbl)
                  n1951 = Multiply(x="Osc. freq. (Hz)", y=6.283185307179586) -> (x*y=w3102:dbl)
                  n1952 = Multiply(x=w3102, y=w3101) -> (x*y=w3086:dbl)
                  n1953 = local read "BD 1 Frq 2 (MHz)"() -> (w3083:dbl)
                  n1954 = local read "BD 1 Frq 1 (MHz)"() -> (w3080:dbl)
                  n1955 = case shown="True" w3090 {
                    tunnel: w3086 -> [w3111 w3118]
                    tunnel: w3083 -> [_ w3128]
                    tunnel: [w3108 w3112] -> w3091
                    tunnel: [FALSE w3121] -> w3087
                    tunnel: [0.0 w3114] -> w3084
                    tunnel: w3080 -> [_ w3113]
                    frame False {
                      n1956 = Sine(x=w3111) -> (sin(x)=w3109:dbl)
                      n1957 = Multiply(x=w3109, y="Osc. amp. (MHz)") -> (x*y=w3108:dbl)
                    }
                    frame True {
                      n1958 = Cosine(x=w3118) -> (cos(x)=w3131:dbl)
                      n1959 = Subtract(x=w3128, y=w3113) -> (x-y=w3127:dbl)
                      n1960 = Decrement(x=w3131) -> (x-1=w3130:dbl)
                      n1961 = Subtract(x=w3127, y="Closest Delta (MHz)") -> (x-y=w3124:dbl)
                      n1962 = Divide(x=w3130, y=2.0) -> (x/y=w3125:dbl)
                      n1963 = Multiply(x=w3125, y=w3124) -> (x*y=w3112:dbl)
                      n1964 = local read "Vec Mean of T1 T2"() -> (w3120:dbl[])
                      n1965 = Greater?(x=w3120, y="Stop F (pN)") -> (0:w3122:bool[])
                      n1966 = Or Array Elements(Boolean array=w3122) -> (logical OR=w3121:bool)
                      n1967 = Divide(x=w3118, y=6.283185307179586) -> (x/y=w3117:dbl)
                      n1968 = Round Toward +Infinity(x=w3117) -> (ceil(x): smallest int >= x=w3114:dbl)
                      "Attempts" <- w3114
                      n1969 = Greater?(x=w3114, y="Attempt Limit") -> (0:w3116:bool)
                      n1970 = case shown="True" w3116 {
                        frame False {
                        }
                        frame True {
                          n1971 = local write "Fish for Tether"(FALSE ("Fish for Tether")) -> ()
                          n1972 = call <vilib>:"Beep.vi"() -> ()  [unwired: 3 in, 9 out]
                          n1973 = local read "Messages"() -> (w3133:string)
                          n1974 = call "Update messages.vi"("Message to add"="Tether fishing timeout." ("Messages"), "Old message string"=w3133) -> ("New message string"=→"Messages":string)
                        }
                      }
                    }
                  }
                  n1975 = local read "Y RF Frequency Limits (MHz)"() -> (w3092:T16)
                  n1976 = local read "X RF Frequency Limits (MHz)"() -> (w3093:T16)
                  n1977 = local read "BD 1 Frq 3 (MHz)"() -> (w3098:dbl)
                  n1978 = local read "BD 2 Frq 2 (MHz)"() -> (w3082:dbl)
                  n1979 = Select(t=w3083, s="Scan axis 2", f=w3082) -> (s? t:f=w3094:dbl)
                  n1980 = Add(x=w3091, y=w3094) -> (x+y=w3089:dbl)
                  n1981 = Select(t=w3089, s="Scan axis 2", f=w3083) -> (s? t:f=w3081:dbl)
                  n1982 = Select(t=w3082, s="Scan axis 2", f=w3089) -> (s? t:f=w3096:dbl)
                  n1983 = local read "BD 2 Frq 3 (MHz)"() -> (w3097:dbl)
                  n1984 = call "set RF board frequency - interlace.vi"("Board 2 Frequency Limits"=w3092, "Board 1 Frequency Limits"=w3093, "FPGA VI Reference In"=w3088, "Board 2 Frequency 3 (MHz)"=w3097, "Board 1 Frequency 3 (MHz)"=w3098, "Board 2 Frequency 2 (MHz)"=w3082, "Board 2 Frequency 1 (MHz)"=w3096, "Board 1 Frequency 2 (MHz)"=w3081, "Board 1 Frequency 1  (MHz)"=w3080) -> ()  [unwired: 1 in, 2 out]
                }
                frame #1 {
                  n1985 = And(x=w3141, y=w3138) -> (x .and. y?=w3140:bool)
                  n1986 = case "Only if were fishing and now formed tether" shown="True" w3140 {
                    tunnel: w3139 -> [w3143 w3155]
                    tunnel: [w3142 w3154] -> w3137
                    tunnel: w3136 -> [_ w3150]
                    frame False {
                      n1987 = local read "Fish for Tether"() -> (w3142:bool)
                      n1988 = case shown="True" w3142 {
                        tunnel: w3143 -> [_ _]
                        frame False {
                        }
                        frame True {
                        }
                      }
                    }
                    frame True {
                      w3154 = FALSE ("Fish for Tether")
                      n1989 = call <vilib>:"Beep.vi"() -> ()  [unwired: 3 in, 9 out]
                      n1990 = Number To Decimal String(number=w3150, width (-)=i16 1) -> (decimal integer string=w3148:string)
                      n1991 = case shown="\"2\", \"3\", \"4\", \"5\", \"6\"" "Then..." {
                        selector: "Then..." -> [_ w3158]
                        tunnel: w3155 -> [w3157 _]
                        frame "1", Default {
                          # "do nothing"
                          n1992 = property on="BD 1 Frq 1 (MHz)" class="DigNum (strict)"("Val(Sgnl)"=w3157) -> ()  [unwired: 2 in, 2 out]
                        }
                        frame "2", "3", "4", "5", "6" {
                          n1993 = flat-sequence {
                            tunnel: w3158 -> [w3160]
                            frame #0 {
                              n1994 = property on="Trap Delta (MHz)" class="DigNum (strict)"("Val(Sgnl)"="Move to Delta 1 (MHz)") -> ()  [unwired: 2 in, 2 out]
                            }
                            frame #1 {
                              n1995 = case shown="\"5\", \"6\"" w3160 {
                                selector: w3160 -> [w3163 w3173 _]
                                frame "3", "4" {
                                n1996 = flat-sequence {
                                tunnel: w3163 -> [w3164]
                                tunnel: [w3164] -> w3161
                                tunnel: [w3166] -> w3162
                                tunnel: w3161 -> [w3166]
                                tunnel: w3162 -> [w3170]
                                frame #0 {
                                n1997 = property on="Green Laser ON/Interlacing" class="Bool (strict)"("Val(Sgnl)"=TRUE ("Value (Signaling)")) -> ()  [unwired: 2 in, 2 out]
                                }
                                frame #1 {
                                n1998 = Multiply(x="Wait Before Save (s)", y=u32 1000 ("x")) -> (x*y=w3168:u32)
                                n1999 = Wait (ms)(milliseconds to wait=w3168) -> ()  [unwired: 1 out]
                                }
                                frame #2 {
                                n2000 = property on="Start Saving" class="Bool (strict)"("Value"=TRUE ("Start Saving")) -> ()  [unwired: 2 in, 2 out]
                                n2001 = case shown="Default" w3170 {
                                frame Default {
                                }
                                frame "4" {
                                n2002 = property on="Fl. Triggered..." class="Bool (strict)"("Val(Sgnl)"=TRUE ("Value (Signaling)")) -> ()  [unwired: 2 in, 2 out]
                                }
                                }
                                }
                                }
                                }
                                frame "5", "6" {
                                n2003 = stacked-sequence {
                                tunnel: w3173 -> [_ _ _ _ _ _ _ _ w3190 _ _]
                                frame #0 {
                                n2004 = Replace Array Subset(array=u32[] [0] ("Index Values"), new element="Raster Set Upon Tether", index=0) -> (w3174:u32[])
                                n2005 = property on="Saved AOD Raster Scan Parameter Sets" class="Arr (strict)"("Index Values"=w3174) -> ()  [unwired: 2 in, 2 out]
                                }
                                frame #1 {
                                n2006 = Wait (ms)(milliseconds to wait=u32 500) -> ()  [unwired: 1 out]
                                }
                                frame #2 {
                                n2007 = property on="Load parameters" class="Bool (strict)"("Val(Sgnl)"=TRUE ("Value (Signaling)")) -> ()  [unwired: 2 in, 2 out]
                                }
                                frame #3 {
                                n2008 = Wait (ms)(milliseconds to wait=u32 500) -> ()  [unwired: 1 out]
                                }
                                frame #4 {
                                n2009 = property on="Trap Raster Scan" class="Bool (strict)"("Val(Sgnl)"=TRUE ("Value (Signaling)")) -> ()  [unwired: 2 in, 2 out]
                                }
                                frame #5 {
                                n2010 = Wait (ms)(milliseconds to wait=u32 2000) -> ()  [unwired: 1 out]
                                }
                                frame #6 {
                                n2011 = while {
                                stop <- w3185 stop-if-true
                                n2012 = local read "Raster Scanning..."() -> (w3184:bool)
                                n2013 = local read "Saving..."() -> (w3187:bool)
                                n2014 = Wait (ms)(milliseconds to wait=u32 100) -> ()  [unwired: 1 out]
                                n2015 = Not(x=w3187) -> (.not. x?=w3186:bool)
                                n2016 = Not(x=w3184) -> (.not. x?=w3183:bool)
                                n2017 = And(x=w3186, y=w3183) -> (x .and. y?=w3185:bool)
                                }
                                }
                                frame #7 {
                                n2018 = property on="Trap Delta (MHz)" class="DigNum (strict)"("Val(Sgnl)"="Move to Delta 2 (MHz)") -> ()  [unwired: 2 in, 2 out]
                                }
                                frame #8 {
                                n2019 = local read "Tether"() -> (w3191:bool)
                                n2020 = case shown="True" w3191 {
                                tunnel: w3190 -> [_ w3192]
                                frame False {
                                }
                                frame True {
                                n2021 = flat-sequence {
                                tunnel: w3192 -> [w3194]
                                frame #0 {
                                n2022 = Wait (ms)(milliseconds to wait=u32 500) -> ()  [unwired: 1 out]
                                }
                                frame #1 {
                                n2023 = case shown="\"6\"" w3194 {
                                frame Default {
                                }
                                frame "6" {
                                n2024 = property on="Green Laser ON/Interlacing" class="Bool (strict)"("Val(Sgnl)"=TRUE ("Green Laser ON/Interlacing")) -> ()  [unwired: 2 in, 2 out]
                                }
                                }
                                }
                                frame #2 {
                                n2025 = Wait (ms)(milliseconds to wait=u32 500) -> ()  [unwired: 1 out]
                                }
                                frame #3 {
                                n2026 = local write "Start Saving"("Save at end (5, 6)") -> ()
                                }
                                }
                                }
                                }
                                }
                                frame #9 {
                                n2027 = local read "Bead Sep. Int. Time (s)"() -> (w3200:dbl)
                                n2028 = Multiply(x=w3200, y=1000.0) -> (x*y=w3199:dbl)
                                n2029 = Wait (ms)(milliseconds to wait=w3199) -> ()  [unwired: 1 out]
                                }
                                frame #10 {
                                n2030 = property on="Rescale on Mean" class="Bool (strict)"("Val(Sgnl)"=TRUE ("Value (Signaling)")) -> ()  [unwired: 2 in, 2 out]
                                }
                                }
                                }
                                frame "2", Default {
                                }
                              }
                            }
                          }
                        }
                      }
                      n2031 = Concatenate Strings("Formed tether in ", w3148, " attempt(s)." ("string")) -> (w3145:string)
                      n2032 = local read "Messages"() -> (w3152:string)
                      n2033 = local write "Fish for Tether"(w3154) -> ()
                      n2034 = call "Update messages.vi"("Message to add"=w3145, "Old message string"=w3152) -> ("New message string"=w3151:string)
                      n2035 = local write "Messages"(w3151) -> ()
                      n2036 = Get Date/Time In Seconds() -> (seconds since 1Jan1904=→"Time tether formed":timestamp)
                      "Tether" <- "Tether Alarm?"
                    }
                  }
                }
                frame #2 {
                  n2037 = local read "Oscillate Set 2"() -> (w3204:bool)
                  n2038 = local read "Stop All"() -> (w3206:bool)
                  n2039 = Not Or(1:w3203, 2:w3204) -> (0:w3202:bool)
                  n2040 = Compound Arithmetic op=OR(w3206, w3202) -> (w3205:bool)
                }
              }
              n2041 = node-c288() -> ()  [unwired: 2 out]
            }
            n2042 = node-c288(w3066) -> ()  [unwired: 1 out]
          }
        }
      }
      event "Fl. Triggered...": Value Change {
        n2043 = event-data() -> ()  [unwired: 7 out]
        n2044 = case shown="True" "Fl. Triggered..." {
          frame False {
          }
          frame True {
            n2045 = node-c288() -> (w3218:T24)  [unwired: 4 out]
            n2046 = timed-loop {
              timing: w3218 -> [_]
              timing-out: [_] -> w3217
              tunnel: "Action" -> [w3222]
              shift-right: [w3219] -> _
              shift-left: u8 255 -> [w3221]
              stop <- w3223 stop-if-true
              n2047 = node-c288() -> ()  [unwired: 2 out]
              n2048 = flat-sequence {
                tunnel: w3222 -> [w3234]
                tunnel: w3221 -> [w3231]
                tunnel: [w3230] -> w3220
                tunnel: [w3319] -> w3223
                tunnel: w3220 -> [w3318]
                tunnel: [w3318] -> w3219
                frame #0 {
                  w3224 = 1.0 ("t")
                  n2049 = Select(t=w3224, s="APD to Watch", f=w3224) -> (s? t:f=w3226:dbl)
                  n2050 = Multiply(x="Fl. Delta Thresh. (kHz)", y=1000.0) -> (x*y=w3233:dbl)
                  n2051 = Greater?(x=w3226, y=w3233) -> (0:w3228:bool)
                  n2052 = Or(x="Force Yank", y=w3228) -> (x .or. y?=w3229:bool)
                  n2053 = case shown="True" w3229 {
                    tunnel: w3234 -> [_ w3244]
                    tunnel: w3231 -> [w3236 w3240]
                    tunnel: [w3236 w3237] -> w3230
                    frame False {
                    }
                    frame True {
                      # "THIS IS NOW NOT WORKING BC I DELETED SOME THINGS - ALEX"
                      n2054 = flat-sequence {
                        tunnel: w3241 -> [w3250]
                        tunnel: [w3250] -> w3245
                        tunnel: w3244 -> [w3249]
                        tunnel: [w3249] -> w3243
                        tunnel: [w3248] -> w3242
                        tunnel: w3240 -> [w3247]
                        tunnel: [w3246] -> w3239
                        tunnel: w3245 -> [w3275]
                        tunnel: w3243 -> [w3274]
                        tunnel: w3242 -> [w3273]
                        tunnel: w3239 -> [w3272]
                        tunnel: [w3272] -> w3238
                        tunnel: w3238 -> [w3316]
                        tunnel: [w3316] -> w3237
                        frame #0 {
                          n2055 = call <vilib>:"Beep.vi"() -> ()  [unwired: 3 in, 9 out]
                          n2056 = local write "Waiting"(FALSE ("Waiting")) -> ()
                          n2057 = Increment(x=w3247) -> (x+1=w3246:u8)
                          n2058 = case shown="\"Yank\"" w3249 {
                            tunnel: w3246 -> [_ _ w3256]
                            frame "Image" {
                              n2059 = property on="Confocal Image" class="Bool (strict)"("Val(Sgnl)"=TRUE ("Value (Signaling)")) -> ()  [unwired: 2 in, 2 out]
                            }
                            frame "Alarm", Default {
                            }
                            frame "Yank" {
                              n2060 = flat-sequence {
                                tunnel: w3256 -> [w3259]
                                tunnel: [w3258] -> w3255
                                tunnel: ["N Array El"] -> w3254
                                tunnel: w3255 -> [w3269]
                                tunnel: w3254 -> [w3265]
                                frame #0 {
                                n2061 = Multiply(x="Yank Delay (s)", y=1000.0) -> (x*y=w3262:dbl)
                                n2062 = Quotient & Remainder(x=w3259, y="N Array El") -> (x-y*floor(x/y)=w3258:u8)  [unwired: 1 out]
                                n2063 = Wait (ms)(milliseconds to wait=w3262) -> ()  [unwired: 1 out]
                                }
                                frame #1 {
                                n2064 = Random Number (0-1)() -> (number: 0 to 1=w3266:dbl)
                                n2065 = Multiply(x=w3265, y=w3266) -> (x*y=w3264:dbl)
                                n2066 = Round Toward -Infinity(1:w3264) -> (0:w3263:dbl)
                                n2067 = Select(t=w3263, s="Random Choice", f=w3269) -> (s? t:f=w3267:dbl)
                                n2068 = Index Array(array="Yank to Delta Array (MHz)", index=w3267) -> (element=w3270:dbl)
                                n2069 = property on="Trap Delta (MHz)" class="DigNum (strict)"("Val(Sgnl)"=w3270) -> ()  [unwired: 2 in, 2 out]
                                }
                              }
                            }
                          }
                          n2070 = local read "Time (s)"() -> (w3248:dbl)
                          "Fl. High" <- TRUE ("Yanking")
                        }
                        frame #1 {
                          n2071 = node-c288() -> (w3277:T24)  [unwired: 4 out]
                          n2072 = timed-loop {
                            timing: w3277 -> [_]
                            timing-out: [_] -> w3276
                            tunnel: w3275 -> [w3292]
                            tunnel: w3274 -> [w3290]
                            tunnel: w3273 -> [w3289]
                            stop <- w3291 stop-if-true
                            w3278 = 1.0 ("t")
                            n2073 = node-c288() -> ()  [unwired: 2 out]
                            n2074 = local read "Fl. Delta Thresh. (kHz)"() -> (w3284:dbl)
                            n2075 = local read "Fl. Triggered..."() -> (w3293:bool)
                            n2076 = local read "Stop All"() -> (w3287:bool)
                            n2077 = local read "APD to Watch"() -> (w3280:bool)
                            n2078 = Select(t=w3278, s=w3280, f=w3278) -> (s? t:f=w3279:dbl)
                            n2079 = Not(x=w3293) -> (.not. x?=w3288:bool)
                            n2080 = Multiply(x=w3284, y=1000.0) -> (x*y=w3283:dbl)
                            n2081 = Negate(x=w3283) -> (-x=w3282:dbl)
                            n2082 = Less?(x=w3279, y=w3282) -> (x < y?=w3286:bool)
                            n2083 = Compound Arithmetic op=OR(w3286, w3287, w3288, "Force Reset") -> (w3291:bool)
                            n2084 = case shown="True" w3291 {
                              tunnel: w3292 -> [_ w3304]
                              tunnel: w3290 -> [_ w3303]
                              tunnel: w3289 -> [_ w3301]
                              frame False {
                              }
                              frame True {
                                n2085 = case shown="\"Yank\"" w3303 {
                                tunnel: w3304 -> [_ w3305]
                                frame "Image", Default {
                                }
                                frame "Yank" {
                                n2086 = flat-sequence {
                                tunnel: [w3310] -> w3306
                                tunnel: w3305 -> [w3310]
                                tunnel: w3306 -> [w3311]
                                frame #0 {
                                n2087 = local read "Yank Delay (s)"() -> (w3309:dbl)
                                n2088 = Multiply(x=w3309, y=1000.0) -> (x*y=w3307:dbl)
                                n2089 = Wait (ms)(milliseconds to wait=w3307) -> ()  [unwired: 1 out]
                                }
                                frame #1 {
                                n2090 = property on="Trap Delta (MHz)" class="DigNum (strict)"("Val(Sgnl)"=w3311) -> ()  [unwired: 2 in, 2 out]
                                }
                                }
                                }
                                }
                                n2091 = local read "Time (s)"() -> (w3302:dbl)
                                n2092 = Subtract(x=w3302, y=w3301) -> (x-y=w3298:dbl)
                                "Duration (s)" <- w3298
                                n2093 = Number To Decimal String(number=w3298, width (-)=i16 0) -> (decimal integer string=w3296:string)
                                n2094 = Concatenate Strings(w3296, " s fluorescence event." ("string")) -> (w3294:string)
                                n2095 = local read "Messages"() -> (w3300:string)
                                n2096 = call "Update messages.vi"("Message to add"=w3294, "Old message string"=w3300) -> ("New message string"=w3299:string)
                                n2097 = call <vilib>:"Beep.vi"() -> ()  [unwired: 3 in, 9 out]
                                n2098 = local write "Messages"(w3299) -> ()
                              }
                            }
                            n2099 = node-c288() -> ()  [unwired: 2 out]
                          }
                          n2100 = node-c288(w3276) -> ()  [unwired: 1 out]
                        }
                        frame #2 {
                          n2101 = local write "Fl. High"(FALSE ("Yanking")) -> ()
                        }
                      }
                      n2102 = local read "Trap Delta (MHz)"() -> (w3241:dbl)
                    }
                  }
                }
                frame #1 {
                  n2103 = local read "Stop All"() -> (w3322:bool)
                  n2104 = local read "Fl. Triggered..."() -> (w3320:bool)
                  n2105 = Not(x=w3320) -> (.not. x?=w3321:bool)
                  n2106 = Or(x=w3321, y=w3322) -> (x .or. y?=w3319:bool)
                  n2107 = Not(x=w3319) -> (.not. x?=→"Waiting":bool)
                }
              }
              n2108 = node-c288() -> ()  [unwired: 2 out]
            }
            n2109 = node-c288(w3217) -> ()  [unwired: 1 out]
          }
        }
      }
      event "Stop All": Value Change {
        n2110 = event-data() -> ()  [unwired: 7 out]
        n2111 = local read "Stop All"() -> (w3328:bool)
      }
    }
    n2112 = node-c288() -> ()  [unwired: 2 out]
  }
  n2113 = node-c288(w85) -> ()  [unwired: 1 out]
  n2114 = node-c288(w168) -> ()  [unwired: 1 out]
  n2115 = flat-sequence "@Alex - Set stage to 0,0,0 on exit" {
    tunnel: w7 -> [w3330]
    tunnel: [w3329] -> w6
    frame #0 {
      n2116 = local read "ESP Port"() -> (w3334:refnum<visa-resource-name>)
      n2117 = Concatenate Strings("1PA0;\n2PA0;\n3PA0" ("write buffer"), "\r") -> (w3331:string)
      n2118 = VISA Write(VISA resource name=w3334, write buffer=w3331, error in (no error)=w3330) -> (error out=w3329:errorcluster)  [unwired: 2 out]
    }
  }
  n2119 = flat-sequence {
    tunnel: w48 -> [w3339]
    tunnel: [w3338] -> w54
    tunnel: [w3335] -> w53
    tunnel: w52 -> [_]
    tunnel: w51 -> [_]
    tunnel: w50 -> [_]
    tunnel: w49 -> [_]
    tunnel: w6 -> [w3336]
    tunnel: w54 -> [w3342]
    tunnel: w53 -> [w3341]
    frame #0 {
      w3337 = FALSE ("APD to FIFO")
      n2120 = xnode "Read/Write Control"("FPGA VI Reference In"=w3339, "error in"=w3336, "APD to FIFO"=w3337, "AI to FIFO"=w3337) -> ("FPGA VI Reference Out"=w3338:T20, "error out"=w3335:errorcluster)
    }
    frame #1 {
      n2121 = xnode "Invoke Method"("FPGA VI Reference In"=w3342, "error in"=w3341) -> ("FPGA VI Reference Out"=w3340:T20)  [unwired: 1 out]
      n2122 = xnode "Close FPGA VI Reference"("FPGA VI Reference In"=w3340) -> ()  [unwired: 1 in, 1 out]
    }
  }
  "Fish Status" <- w5
